vi "Main.vi"() -> ()   [LabVIEW 2015]
uses:
  Typedef/Queue1 Data.ctl
  Typedef/Data.ctl
  <vilib>/vision/Image Controls.llb/IMAQ Image.ctl
  Typedef/Last Mouse Position.ctl
  Typedef/Report Data.ctl
  Typedef/Data2.ctl
  Typedef/State.ctl
  Typedef/Inst. Data.ctl
  Typedef/Inst. Queue.ctl
  <vilib>/Utility/xml.llb/Read From XML File(string).vi
  <vilib>/Utility/xml.llb/Write to XML File(string).vi
  <vilib>/Utility/file.llb/Read From Spreadsheet File (DBL).vi
  Debug 2/Test_ARTS_1.dll
  zauxdll-2014/zauxdll.lvlib
panel:
  out "load?":bool
  out "dist":dbl[](array[numeric])
  in  "SPEED":dbl[][](array[numeric])
  in  "report dist 2":bool
  out "last time":dbl
  out "DYNAMIC 2":T1(array[cluster])
  out "time":dbl[](array[numeric])
  out "autoRs2finish?":bool
  out "autoRSfinish?":bool
  out "autoSliderfinish?":bool
  out "DYNAMIC":T1(array[cluster])
  out "big abgle":string
  out "auto step finish?":bool
  out "y angle array":i32[][](array[numeric])
  out "x angle array":i32[][](array[numeric])
  out "y angle":dbl[](array[numeric])
  out "x angle":dbl[](array[numeric])
  out "Report Data.Degree":dbl[][](array[numeric])
  out "Array":T2(array[cluster])
  out "x^y":dbl
  out "x*y":dbl
  out "Radar Settings":T3={"Car 1"=[], "Times 1"=0, "Car 2"=[], "Times 2"=0, "ORG"={"X"=0.0, "Y"=0.0}, "ORG?"=FALSE, "User1 Velocity"=[], "User2 Velocity"=[], "Lane Distance(X,Y)"={"X"=15.0, "Y"=15.0}, "Lines Para"=[], "Line to Line"=[]}
  in  "Tab Control":T4(tab)
  in  "early time(ms)":dbl
  in  "loop":bool
  in  "Open Button":bool
  in  "Save Button":bool
  in  "clearMSG":bool
  in  "B dist. comp":dbl
  in  "A dist. comp":dbl
  in  "RCS B":dbl
  in  "Path?":bool
  in  "Mode":bool
  in  "dynamic setting":T5
  in  "s/d setting":bool=TRUE
  in  "Rotate":bool
  in  "lock RCS":bool
  out "Path B":u16(slide) scale=0.0..5.0
  in  "TCP?":bool=TRUE
  out "Path A":u16(slide) scale=0.0..5.0
  in  "RUN":bool
  in  "Cluster":cluster{"tester  A":bool, " tester B":bool}={"tester  A"=TRUE, " tester B"=TRUE}
  in  "Clear All":bool
  in  "Velocity":dbl
  in  "User":enum16{"Car A", "Car B"}(ring)
  out "Image":T6(plugin-control)
  in  "Mode":T7(ring)
  in  "Lane Distance(X,Y)":cluster{"X":dbl, "Y":dbl}={"X"=4.0, "Y"=25.0}
  in  "Exit":bool
  in  "RCS A":dbl
  in  "TARGET":enum32{"CarA", "CarB", "Dy path"}(tab)
  out "Target 1":string
  out "Target 2":string
  in  "dy Path":T8(array[cluster])
  in  "set":bool
  in  "AS mode":enum16{"manual", "ratio"}(ring)
  in  "report dist":bool
  out "MSG":string
  in  "AutoExit":bool
  in  "Server":bool
  in  "gap":i32=5
  in  "Path No.":u16(ring) items=["1", "2", "3", "4", "5"]
  in  "Coordinates(X,Y)":cluster{"X":dbl, "Y":dbl}
  in  "Modify (X,Y)":bool
  out "RCS":dbl
  in  "RCSAUTO":bool
  in  "Gain":dbl=3.0
  in  "Range":dbl=3.0
  in  "Dist to RUT":dbl=3.0
  in  "GRX (dB)":dbl=10.0
  in  "GTX (dB)":dbl=10.0
  in  "Load":bool
  out "Output £m File":string
  in  "Path":path
  out "Input RCS File":string
  in  "Boolean":bool
  in  "RCS1":bool
  out "String":string
  out "Inst. Status":bool
  in  "Reset":bool
  in  "Stop":bool
  in  "RF ON/OFF":bool
  in  "T/R Converters":bool
  out "Status?":bool
  in  "Run/Stop":bool
  in  "Custom File":bool
  in  "status":bool
  in  "Trigger":bool
  in  "Dynamic1":T9={"Target 1"={"Boolean"=TRUE, "Start Speed (km/h)"=100.0, "Stop Speed (km/h)"=100.0, "Start Range(m)"=0.0, "Stop Range(m)"=100.0, "Start Gain(dB)"=0.0}, "Target 2"={"Boolean"=FALSE, "Start Speed (km/h)"=0.0, "Stop Speed (km/h)"=0.0, "Start Range(m)"=0.0, "Stop Range(m)"=0.0, "Start Gain(dB)"=0.0}, "Target 3"={"Boolean"=FALSE, "Start Speed (km/h)"=0.0, "Stop Speed (km/h)"=0.0, "Start Range(m)"=0.0, "Stop Range(m)"=0.0, "Start Gain(dB)"=0.0}, "Target 4"={"Boolean"=FALSE, "Start Speed (km/h)"=0.0, "Stop Speed (km/h)"=0.0, "Start Range(m)"=0.0, "Stop Range(m)"=0.0, "Start Gain(dB)"=0.0}}
  in  "Direct program":T10={"Target 1"={"Boolean"=TRUE, "Speed"=100.0, "Range"=50.0, "Gain"=10.0}, "Target 2"={"Boolean"=FALSE, "Speed"=0.0, "Range"=0.0, "Gain"=0.0}, "Target 3"={"Boolean"=FALSE, "Speed"=0.0, "Range"=0.0, "Gain"=0.0}, "Target 4"={"Boolean"=FALSE, "Speed"=0.0, "Range"=0.0, "Gain"=0.0}}
  in  "Mapping":cluster{"4:4":bool, "4:2":bool, "4:1":bool}
  in  "Rx Attenuation (dB)":dbl=3.0
  in  "Distance to RUT":dbl=3.0
  in  "Range Trim (m)":dbl=2.0
  in  "Gain Trim (dB)":dbl=-3.0
  in  "Freq. (GHz)":dbl=76.5
  in  "Inst. Connect":bool
  in  "Inst. Connect IP":string="192.168.0.19"
  in  "GRX (dB)":dbl=10.0
  in  "GTX (dB)":dbl=10.0
  in  "R^4 Comp":bool
  out "generateWF ok?":i32
  out "RCS":dbl=-58.2
  out "RCS def":dbl=-58.2
  in  "wait":u32=1500
  in  "Boolean 2":bool
  in  "RCS2":bool
  out "generateWF ok? 2":i32
  out "String":string
  out "Inst. Status":bool
  in  "Reset":bool
  in  "Stop":bool
  in  "RF ON/OFF":bool
  in  "T/R Converters":bool
  out "Status?":bool
  in  "Run/Stop":bool
  in  "Custom File":bool
  in  "status":bool
  in  "Trigger":bool
  in  "Dynamic2":T9
  in  "Direct program2":T10={"Target 1"={"Boolean"=TRUE, "Speed"=100.0, "Range"=50.0, "Gain"=10.0}, "Target 2"={"Boolean"=FALSE, "Speed"=0.0, "Range"=0.0, "Gain"=0.0}, "Target 3"={"Boolean"=FALSE, "Speed"=0.0, "Range"=0.0, "Gain"=0.0}, "Target 4"={"Boolean"=FALSE, "Speed"=0.0, "Range"=0.0, "Gain"=0.0}}
  in  "Mapping":cluster{"4:4":bool, "4:2":bool, "4:1":bool}
  in  "Rx Attenuation (dB)":dbl=3.0
  in  "Distance to RUT":dbl=3.0
  in  "Range Trim (m)":dbl=2.0
  in  "Gain Trim (dB)":dbl=5.0
  in  "Freq. (GHz)":dbl=76.5
  in  "Inst. Connect":bool
  in  "Inst. Connect IP":string="192.168.0.20"
  in  "GRX (dB)":dbl=10.0
  in  "GTX (dB)":dbl=10.0
  in  "R^4 Comp":bool
  out "RCS 2":dbl=-58.2
  out "RCS def 2":dbl=-58.2
  in  "wait 2":u32=1500
  in  "Y_Vert_Dist(mm)":dbl=24500.0
  in  "X_Vert_Dist(mm)":dbl=24500.0
  in  "Y_MID":dbl=72100.0
  in  "X_MID":dbl=72700.0
  in  "reset ant":bool
  out "Y Position (cm)":dbl(slide)
  out "X Position (cm)":dbl(slide) scale=0.0..150.0
  out "Run Time (sec)":dbl
  in  "Tab Control 2":enum32{"Move"}(tab)
  in  "Move Method":enum16{"Continue", "Inching"}(ring)
  in  "Distance":dbl
  in  "Move Mode":enum16{"Relative", "Absolute"}(ring)
  in  "Direct of movement":enum16{"Forward", "Backward"}(ring)
  in  "Normal Open / Close":enum16{"Open", "Close"}(ring)=enum."Close"
  in  "Move Button":bool
  in  "S ramp":dbl=30.0
  in  "Acceleration":dbl=100000.0
  in  "Initial Speed":dbl=10.0
  in  "Deceleration":dbl=100000.0
  in  "Creep":dbl=30.0
  in  "Stop Button":bool
  in  "Return to Zero Button":bool
  in  "Axis":enum16{"X", "Y", "X+Y"}[](array[ring])=[enum."X"]
  in  "Speed":dbl=10000.0
  in  "Angle":T11(ring)
  in  "Rotate Button":bool
  in  "Return to Origin Button":bool
  in  "Move & Rotate":bool
  in  "Return to Middle Button":bool
  out "Y Axis":T12
  out "X Axis":T12
  out "Connect":bool
  out "APP State":string
  in  "Connect DUT Button":bool
  in  "IP Addr":string="192.168.0.11"
  in  "Cluster 2":cluster{"reset y":bool, "reset x ":bool}
  in  "Save Button 2":bool
  in  "Speed":dbl=1.0 format="%#_13g"
  in  "Initial to Y Step":bool
  in  "Step1":bool
  in  "Step2":bool
  in  "Step3":bool
  in  "Remove Button":bool
  in  "Add Button":bool
  in  "Connect":bool
  in  "angle":T13(ring)
  out "Meter":dbl(knob) scale=-180.0..180.0
  in  "VISA GPIB Resource":refnum<visa-resource-name>="EM-2000"
  out "read buffer":string
  in  "origin":dbl=90.0 format="%#_13g"
  # "dB"
  # "dB"
  # "CarA"
  # "CarB"
  # "RCS Calc"
  # "Dynamic Target"
  # "Setting"
  # "Simulation Setup"
  # "Direct Program"
  # "Dynamic Target"
  # "Setting"
  # "Simulation Setup"
  # "Direct Program"
  # "Move"
  # "Rotate"
  # "Return to Zero"
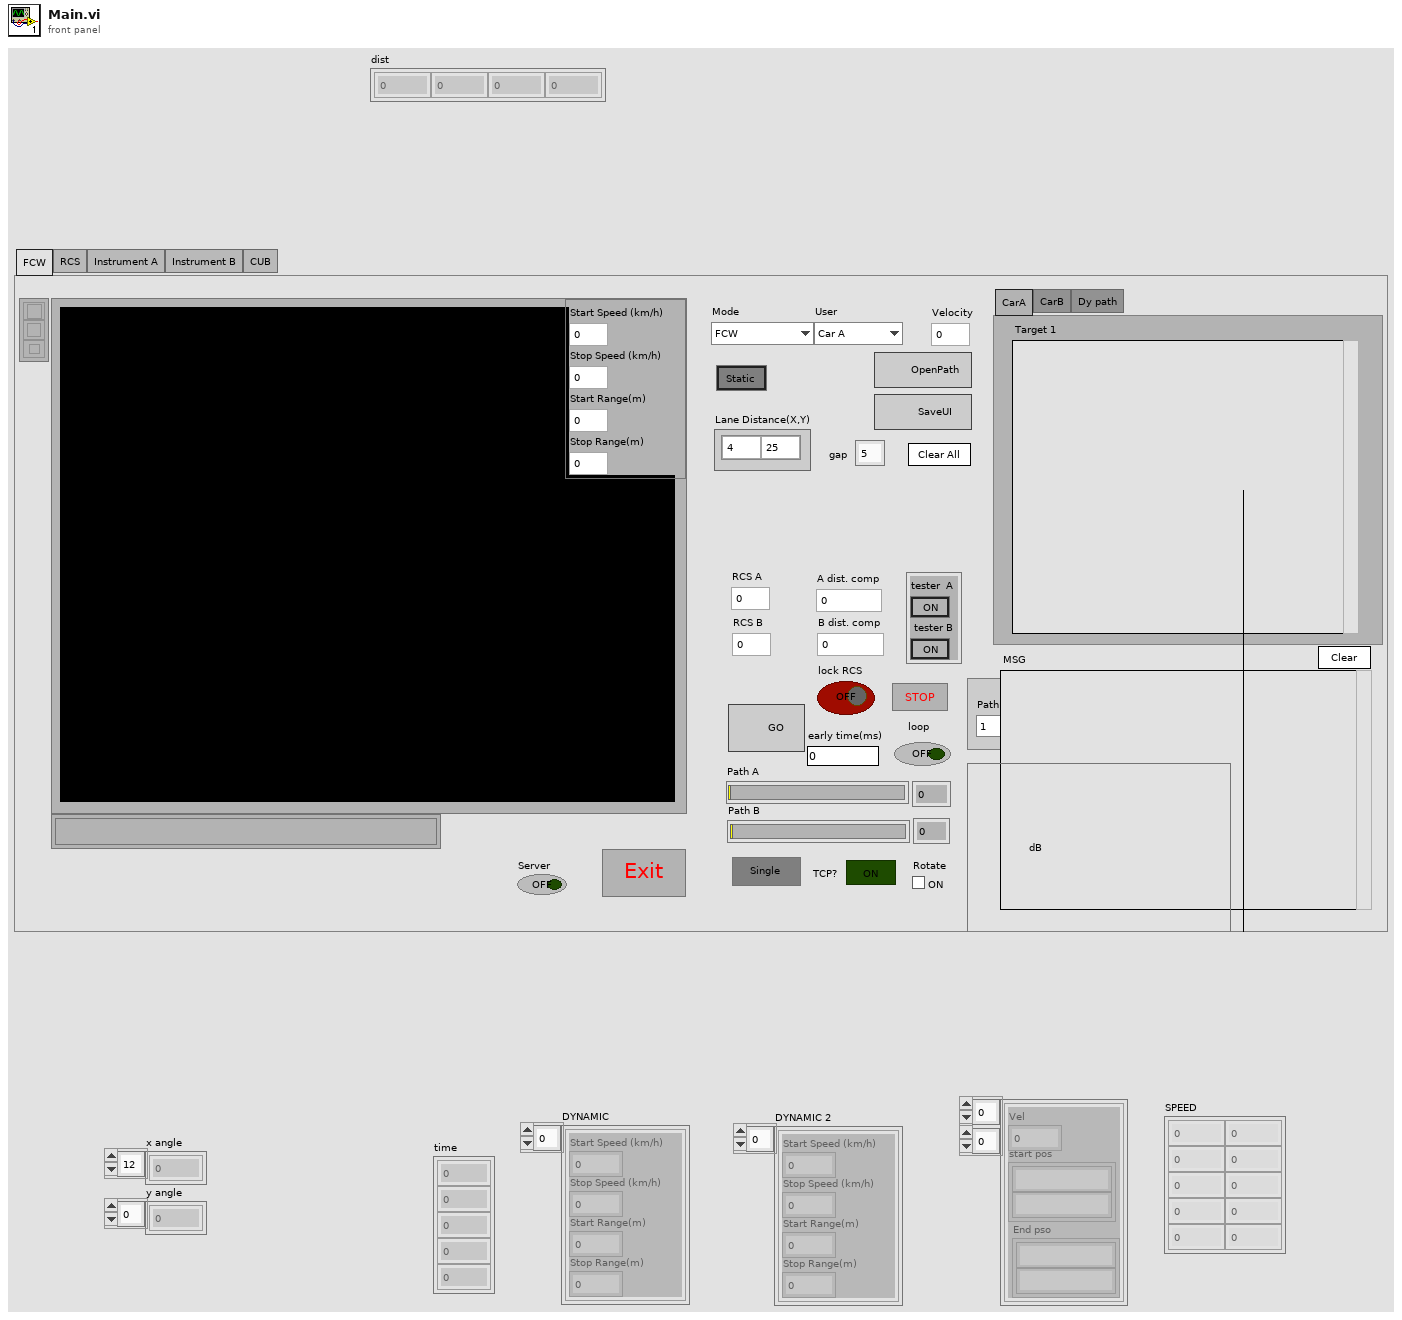
[diagram p1: front panel]
types:
  T1 = cluster{"Start Speed (km/h)":dbl, "Stop Speed (km/h) ":dbl, "Start Range(m)":dbl, "Stop Range(m)":dbl}[]
  T2 = cluster{"Vel":dbl, "start pos":cluster{string, string}, "End pso":cluster{string, string}}[][]
  T3 = cluster{"Car 1":cluster{"X":dbl, "Y":dbl}[], "Times 1":i32, "Car 2":cluster{"X":dbl, "Y":dbl}[], "Times 2":i32, "ORG":cluster{"X":dbl, "Y":dbl}, "ORG?":bool, "User1 Velocity":dbl[], "User2 Velocity":dbl[], "Lane Distance(X,Y)":cluster{"X":dbl, "Y":dbl}, "Lines Para":dbl[][], "Line to Line":dbl[]}
  T4 = enum32{"FCW", "RCS", "Instrument A", "Instrument B", "CUB", "GPIB"}
  T5 = cluster{"Start Speed (km/h)":dbl, "Stop Speed (km/h) ":dbl, "Start Range(m)":dbl, "Stop Range(m)":dbl}
  T6 = typedef "IMAQ Image.ctl" = refnum<image>
  T7 = enum16{"FCW", "BSD(Right)", "BSD(Left)", "RCTA(Right)", "RCTA(Left)", "DOW(Right)", "DOW(Left)"}
  T8 = cluster{"end":dbl, "start":dbl, "Axis Speed":dbl, "movement":dbl}[][]
  T9 = cluster{"Target 1":cluster{"Boolean":bool, "Start Speed (km/h)":dbl, "Stop Speed (km/h)":dbl, "Start Range(m)":dbl, "Stop Range(m)":dbl, "Start Gain(dB)":dbl}, "Target 2":cluster{"Boolean":bool, "Start Speed (km/h)":dbl, "Stop Speed (km/h)":dbl, "Start Range(m)":dbl, "Stop Range(m)":dbl, "Start Gain(dB)":dbl}, "Target 3":cluster{"Boolean":bool, "Start Speed (km/h)":dbl, "Stop Speed (km/h)":dbl, "Start Range(m)":dbl, "Stop Range(m)":dbl, "Start Gain(dB)":dbl}, "Target 4":cluster{"Boolean":bool, "Start Speed (km/h)":dbl, "Stop Speed (km/h)":dbl, "Start Range(m)":dbl, "Stop Range(m)":dbl, "Start Gain(dB)":dbl}}
  T10 = cluster{"Target 1":cluster{"Boolean":bool, "Speed":dbl, "Range":dbl, "Gain":dbl}, "Target 2":cluster{"Boolean":bool, "Speed":dbl, "Range":dbl, "Gain":dbl}, "Target 3":cluster{"Boolean":bool, "Speed":dbl, "Range":dbl, "Gain":dbl}, "Target 4":cluster{"Boolean":bool, "Speed":dbl, "Range":dbl, "Gain":dbl}}
  T11 = enum32{"0", "1", "10", "30", "34", "60", "90", "180", "-1", "-10"}
  T12 = cluster{"Operating State":string, "Current Position":dbl, "Current Speed":dbl, "Axis State":i32, "Angle":dbl}
  T13 = enum16{"0", "1", "5", "10", "30", "60", "90", "180"}
  T14 = cluster{"Global Rectangle":i32[], "Contours":cluster{"Contour Type":u32, "ROI Type":u32, "Points":i32[]}[]}
  T15 = typedef "Inst. Data.ctl" = cluster{"£m Data":dbl[][], "Inst. Status":bool, "GTX (dB)":dbl, "GRX (dB)":dbl, "Freq. (GHz)":dbl, "Gain Trim (dB)":dbl, "Range Trim (m)":dbl, "Distance to RUT":dbl, "Rx Attenuation (dB)":dbl, "Mapping":cluster{"4:4":bool, "4:2":bool, "4:1":bool}, "Direct program":cluster{"Target 1":cluster{"Boolean":bool, "Speed":dbl, "Range":dbl, "Gain":dbl}, "Target 2":cluster{"Boolean":bool, "Speed":dbl, "Range":dbl, "Gain":dbl}, "Target 3":cluster{"Boolean":bool, "Speed":dbl, "Range":dbl, "Gain":dbl}, "Target 4":cluster{"Boolean":bool, "Speed":dbl, "Range":dbl, "Gain":dbl}}, "Dynamic":cluster{"Target 1":cluster{"Boolean":bool, "Start Speed (km/h)":dbl, "Stop Speed (km/h)":dbl, "Start Range(m)":dbl, "Stop Range(m)":dbl, "Start Gain(dB)":dbl}, "Target 2":cluster{"Boolean":bool, "Start Speed (km/h)":dbl, "Stop Speed (km/h)":dbl, "Start Range(m)":dbl, "Stop Range(m)":dbl, "Start Gain(dB)":dbl}, "Target 3":cluster{"Boolean":bool, "Start Speed (km/h)":dbl, "Stop Speed (km/h)":dbl, "Start Range(m)":dbl, "Stop Range(m)":dbl, "Start Gain(dB)":dbl}, "Target 4":cluster{"Boolean":bool, "Start Speed (km/h)":dbl, "Stop Speed (km/h)":dbl, "Start Range(m)":dbl, "Stop Range(m)":dbl, "Start Gain(dB)":dbl}}, "String":string, "auto test":bool}
  T16 = enum16{"INIT", "READ", "WRITE", "Query", "CLOSE"}
  T17 = typedef "State.ctl" = enum16{"Idle", "Initial", "Update", "get angle", "Axis", "Connect", "Creep", "Speed", "Distance", "Move Method", "Move Mode", "Direct of Movement", "Initail Speed", "Sramp", "Normal Open", "Acceleration", "Deceleration", "Angle", "Move&Rotate", "Rotate", "Rotate_2", "Return to Origin", "Move", "Inching", "Return to Zero", "Return to Middle", "Go to Step1", "Go to Step2", "Go to Step3", "Initial to Y Step", "Select Speed", "auto mode", "Stop", "reset xy", "reset ant", "set speed", "Exit"}
  T18 = typedef "Queue1 Data.ctl" = cluster{"State":enum16{"Idle", "Initial", "Update", "User", "Mode", "Lane Distance", "ORG", "Lines Para", "Velocity", "Coordinate", "Path No.", "Modify", "Load", "Loadpath", "Clear All", "Overlay_Circle Para", "Overlay", "Report Dist", "Report", "RCS Report", "dynamic", "save", "dypath", "Exit"}, "variant":variant}
  T19 = typedef "Inst. Queue.ctl" = cluster{enum16{"auto mode", "Idle", "Inst. Connect", "£m Data", "Inst. Update", "Freq. (GHz)", "rx att", "GTX (dB)", "GRX (dB)", "Range Trim(m)", "Gain Trim (dB)", "Distance to RUT", "Mapping", "Convert", "RF ON/OFF", "Run", "Direct Program", "Stop", "Dynamic", "dyset", "Exit"}, "variant":variant}
  T20 = enum16{"0", "1", "10", "30", "34", "60", "90", "180"}
  T21 = cluster{"Enum":enum16{"INIT", "READ", "DEC", "ADD", "WRITE", "CLOSE", "IDLE"}, "Variable":variant}
  T22 = cluster{dbl, cluster{string, string}, cluster{string, string}}[]
  T23 = cluster{dbl, cluster{string, string}, cluster{string, string}}
  T24 = typedef "Data2.ctl" = cluster{"App State":string, "Connect ":bool, "phandle out":u32, "Axis":enum16{"X", "Y", "X+Y"}[], "S ramp":dbl, "Acceleration":dbl, "Initial Speed":dbl, "Normal Open / Close":enum16{"Open", "Close"}, "Deceleration":dbl, "Creep":dbl, "Speed":dbl, "X Axis":cluster{"Operating State":string, "Current Position":dbl, "Current Speed":dbl, "Axis State":i32, "Angle":dbl}, "Y Axis":cluster{"Operating State":string, "Current Position":dbl, "Current Speed":dbl, "Axis State":i32, "Angle":dbl}, "Distance":dbl, "Direct of movement":enum16{"Forward", "Backward"}, "Move Method":enum16{"Continue", "Inching"}, "Move Mode":enum16{"Relative", "Absolute"}, "Angle":enum32{"0", "1", "10", "30", "34", "60", "90", "180", "-1", "-10"}, "Times":i32, "Start Time":dbl, "Step Flag":bool, "x  dist":dbl[], "y dist":dbl[], "x angle array":i32[][], "y angle array":i32[][], "index":dbl, "big motion angle":dbl, "big angle":dbl[], "xy dy speed table":dbl[][], "x dy speed table":dbl[], "y dy speed table":dbl[], "x dy time":dbl[], "y dy time":dbl[], "xy dy time":dbl[][], "dy Path  ":cluster{"end":dbl, "start":dbl, "Axis Speed":dbl, "movement":dbl}[][]}
  T25 = typedef "Data.ctl" = cluster{"Image":T6, "User":enum16{"Car 1", "Car 2"}, "Last Mouse Position":T26, "Mode":enum16{"FCW", "BSD(Right)", "BSD(Left)", "RCTA(Right)", "RCTA(Left)", "DOW(Right)", "DOW(Left)"}, "Report Data":T27, "Target 1":string, "Target 2":string, "Velocity":dbl, "Coordinates(X,Y)":cluster{"X":dbl, "Y":dbl}, "Path No.":u16, "Input RCS File":string, "Input RCS Data":dbl[][], "Output £m File":string, "DYNAMIC":cluster{"Start Speed (km/h)":dbl, "Stop Speed (km/h) ":dbl, "Start Range(m)":dbl, "Stop Range(m)":dbl}[], "DYNAMIC 2":cluster{"Start Speed (km/h)":dbl, "Stop Speed (km/h) ":dbl, "Start Range(m)":dbl, "Stop Range(m)":dbl}[], "dy Path  ":cluster{"end":dbl, "start":dbl, "Axis Speed":dbl, "movement":dbl}[][]}
  T26 = typedef "Last Mouse Position.ctl" = cluster{"User1":cluster{"X":dbl, "Y":dbl}[], "Times 1":i32, "User2":cluster{"X":dbl, "Y":dbl}[], "Times 2":i32, "ORG":cluster{"X":dbl, "Y":dbl}, "ORG?":bool, "User1 Velocity":dbl[], "User2 Velocity":dbl[], "Lane Distance(X,Y)":cluster{"X":dbl, "Y":dbl}, "Lines Para":dbl[][], "Line to Line":dbl[]}[]
  T27 = typedef "Report Data.ctl" = cluster{"Coordinate":cluster{string, string}[][], "Distance":dbl[][], "Degree":dbl[][], "Velocity":dbl[][], "Times":i32[]}
  T28 = cluster{"Operating State":string, "Current Position":dbl, "Current Speed":dbl, "Axis State":i32, "Angle":i32}
  T29 = cluster{"end":dbl, "start":dbl, "Axis Speed":dbl, "movement":dbl}[]
  T30 = enum16{"auto mode", "Idle", "Inst. Connect", "£m Data", "Inst. Update", "Freq. (GHz)", "rx att", "GTX (dB)", "GRX (dB)", "Range Trim(m)", "Gain Trim (dB)", "Distance to RUT", "Mapping", "Convert", "RF ON/OFF", "Run", "Direct Program", "Stop", "Dynamic", "dyset", "Exit"}
  T31 = cluster{"Boolean":bool, "Speed":dbl, "Range":dbl, "Gain":dbl}
  T32 = enum16{"INIT", "READ", "DEC", "ADD", "WRITE", "CLOSE", "IDLE"}
  T33 = cluster{"Value":cluster{"Target 1":cluster{"Boolean":bool, "Start Speed (km/h)":dbl, "Stop Speed (km/h)":dbl, "Start Range(m)":dbl, "Stop Range(m)":dbl, "Start Gain(dB)":dbl}, "Target 2":cluster{"Boolean":bool, "Start Speed (km/h)":dbl, "Stop Speed (km/h)":dbl, "Start Range(m)":dbl, "Stop Range(m)":dbl, "Start Gain(dB)":dbl}, "Target 3":cluster{"Boolean":bool, "Start Speed (km/h)":dbl, "Stop Speed (km/h)":dbl, "Start Range(m)":dbl, "Stop Range(m)":dbl, "Start Gain(dB)":dbl}, "Target 4":cluster{"Boolean":bool, "Start Speed (km/h)":dbl, "Stop Speed (km/h)":dbl, "Start Range(m)":dbl, "Stop Range(m)":dbl, "Start Gain(dB)":dbl}}, "Value":cluster{"Target 1":cluster{"Boolean":bool, "Start Speed (km/h)":dbl, "Stop Speed (km/h)":dbl, "Start Range(m)":dbl, "Stop Range(m)":dbl, "Start Gain(dB)":dbl}, "Target 2":cluster{"Boolean":bool, "Start Speed (km/h)":dbl, "Stop Speed (km/h)":dbl, "Start Range(m)":dbl, "Stop Range(m)":dbl, "Start Gain(dB)":dbl}, "Target 3":cluster{"Boolean":bool, "Start Speed (km/h)":dbl, "Stop Speed (km/h)":dbl, "Start Range(m)":dbl, "Stop Range(m)":dbl, "Start Gain(dB)":dbl}, "Target 4":cluster{"Boolean":bool, "Start Speed (km/h)":dbl, "Stop Speed (km/h)":dbl, "Start Range(m)":dbl, "Stop Range(m)":dbl, "Start Gain(dB)":dbl}}}
  T34 = cluster{"Value":cluster{"Target 1":cluster{"Boolean":bool, "Speed":dbl, "Range":dbl, "Gain":dbl}, "Target 2":cluster{"Boolean":bool, "Speed":dbl, "Range":dbl, "Gain":dbl}, "Target 3":cluster{"Boolean":bool, "Speed":dbl, "Range":dbl, "Gain":dbl}, "Target 4":cluster{"Boolean":bool, "Speed":dbl, "Range":dbl, "Gain":dbl}}, "Value":cluster{"Target 1":cluster{"Boolean":bool, "Speed":dbl, "Range":dbl, "Gain":dbl}, "Target 2":cluster{"Boolean":bool, "Speed":dbl, "Range":dbl, "Gain":dbl}, "Target 3":cluster{"Boolean":bool, "Speed":dbl, "Range":dbl, "Gain":dbl}, "Target 4":cluster{"Boolean":bool, "Speed":dbl, "Range":dbl, "Gain":dbl}}}
  T35 = cluster{"Target 1":cluster{"Boolean":bool, "Start Speed (km/h)":dbl, "Stop Speed (km/h)":dbl, "Start Range(m)":dbl, "Stop Range(m)":dbl, "Start Gain(dB)":dbl}, "Target 2":cluster{"Boolean":bool, "Start Speed (km/h)":dbl, "Stop Speed (km/h)":dbl, "Start Range(m)":dbl, "Stop Range(m)":dbl, "Start Gain(dB)":dbl}, "Target 3":cluster{"Boolean":bool, "Start Speed (km/h)":dbl, "Stop Speed (km/h)":dbl, "Start Range(m)":dbl, "Stop Range(m)":dbl, "Start Gain(dB)":dbl}, "Target 4":cluster{"Boolean":bool, "Start Speed (km/h)":dbl, "Stop Speed (km/h)":dbl, "Start Range(m)":dbl, "Stop Range(m)":dbl, "Start Gain(dB)":dbl}}[][]
  T36 = cluster{cluster{"Target 1":cluster{"Boolean":bool, "Speed":dbl, "Range":dbl, "Gain":dbl}, "Target 2":cluster{"Boolean":bool, "Speed":dbl, "Range":dbl, "Gain":dbl}, "Target 3":cluster{"Boolean":bool, "Speed":dbl, "Range":dbl, "Gain":dbl}, "Target 4":cluster{"Boolean":bool, "Speed":dbl, "Range":dbl, "Gain":dbl}}[], cluster{"Target 1":cluster{"Boolean":bool, "Speed":dbl, "Range":dbl, "Gain":dbl}, "Target 2":cluster{"Boolean":bool, "Speed":dbl, "Range":dbl, "Gain":dbl}, "Target 3":cluster{"Boolean":bool, "Speed":dbl, "Range":dbl, "Gain":dbl}, "Target 4":cluster{"Boolean":bool, "Speed":dbl, "Range":dbl, "Gain":dbl}}[]}
  T37 = cluster{"Target 1":cluster{"Boolean":bool, "Start Speed (km/h)":dbl, "Stop Speed (km/h)":dbl, "Start Range(m)":dbl, "Stop Range(m)":dbl, "Start Gain(dB)":dbl}, "Target 2":cluster{"Boolean":bool, "Start Speed (km/h)":dbl, "Stop Speed (km/h)":dbl, "Start Range(m)":dbl, "Stop Range(m)":dbl, "Start Gain(dB)":dbl}, "Target 3":cluster{"Boolean":bool, "Start Speed (km/h)":dbl, "Stop Speed (km/h)":dbl, "Start Range(m)":dbl, "Stop Range(m)":dbl, "Start Gain(dB)":dbl}, "Target 4":cluster{"Boolean":bool, "Start Speed (km/h)":dbl, "Stop Speed (km/h)":dbl, "Start Range(m)":dbl, "Stop Range(m)":dbl, "Start Gain(dB)":dbl}}[]
  T38 = cluster{"queue out":refnum<queue>, "queue out":refnum<queue>, "queue out":refnum<queue>}
  T39 = cluster{"auto step finish?":refnum<vi>, "Run/Stop":refnum<vi>, "Run/Stop":refnum<vi>, "AutoExit":refnum<vi>, "RUN":refnum<vi>}
  T40 = enum16{"Idle", "Initial", "Update", "User", "Mode", "Lane Distance", "ORG", "Lines Para", "Velocity", "Coordinate", "Path No.", "Modify", "Load", "Loadpath", "Clear All", "Overlay_Circle Para", "Overlay", "Report Dist", "Report", "RCS Report", "dynamic", "save", "dypath", "Exit"}
  T41 = cluster{cluster{"X":dbl, "Y":dbl}[], i32, cluster{"X":dbl, "Y":dbl}[], i32, cluster{"X":dbl, "Y":dbl}, bool, dbl[], dbl[], "Value":cluster{"X":dbl, "Y":dbl}, "Lines Para":dbl[][], "Line to Line":dbl[]}
  T42 = cluster{cluster{"X":dbl, "Y":dbl}[], i32, cluster{"X":dbl, "Y":dbl}[], i32, cluster{"X":dbl, "Y":dbl}, bool, dbl[], dbl[], "Value":cluster{"X":dbl, "Y":dbl}, "Lines Para":dbl[][], "Line to Line":dbl[]}[]
  T43 = cluster{"Start Speed (km/h)":dbl, "Stop Speed (km/h) ":dbl, "Start Range(m)":dbl, "Stop Range(m)":dbl}[][]
  T44 = cluster{"User1":cluster{"X":dbl, "Y":dbl}[], "Times 1":i32, "User2":cluster{"X":dbl, "Y":dbl}[], "Times 2":i32, "ORG":cluster{"X":dbl, "Y":dbl}, "ORG?":bool, "User1 Velocity":dbl[], "User2 Velocity":dbl[], "Lane Distance(X,Y)":cluster{"X":dbl, "Y":dbl}, "Lines Para":dbl[][], "Line to Line":dbl[]}
  T45 = cluster{"Start Speed (km/h)":dbl, "Stop Speed (km/h) ":dbl, "Stop Range(m)":dbl, "Start Range(m)":dbl}[]
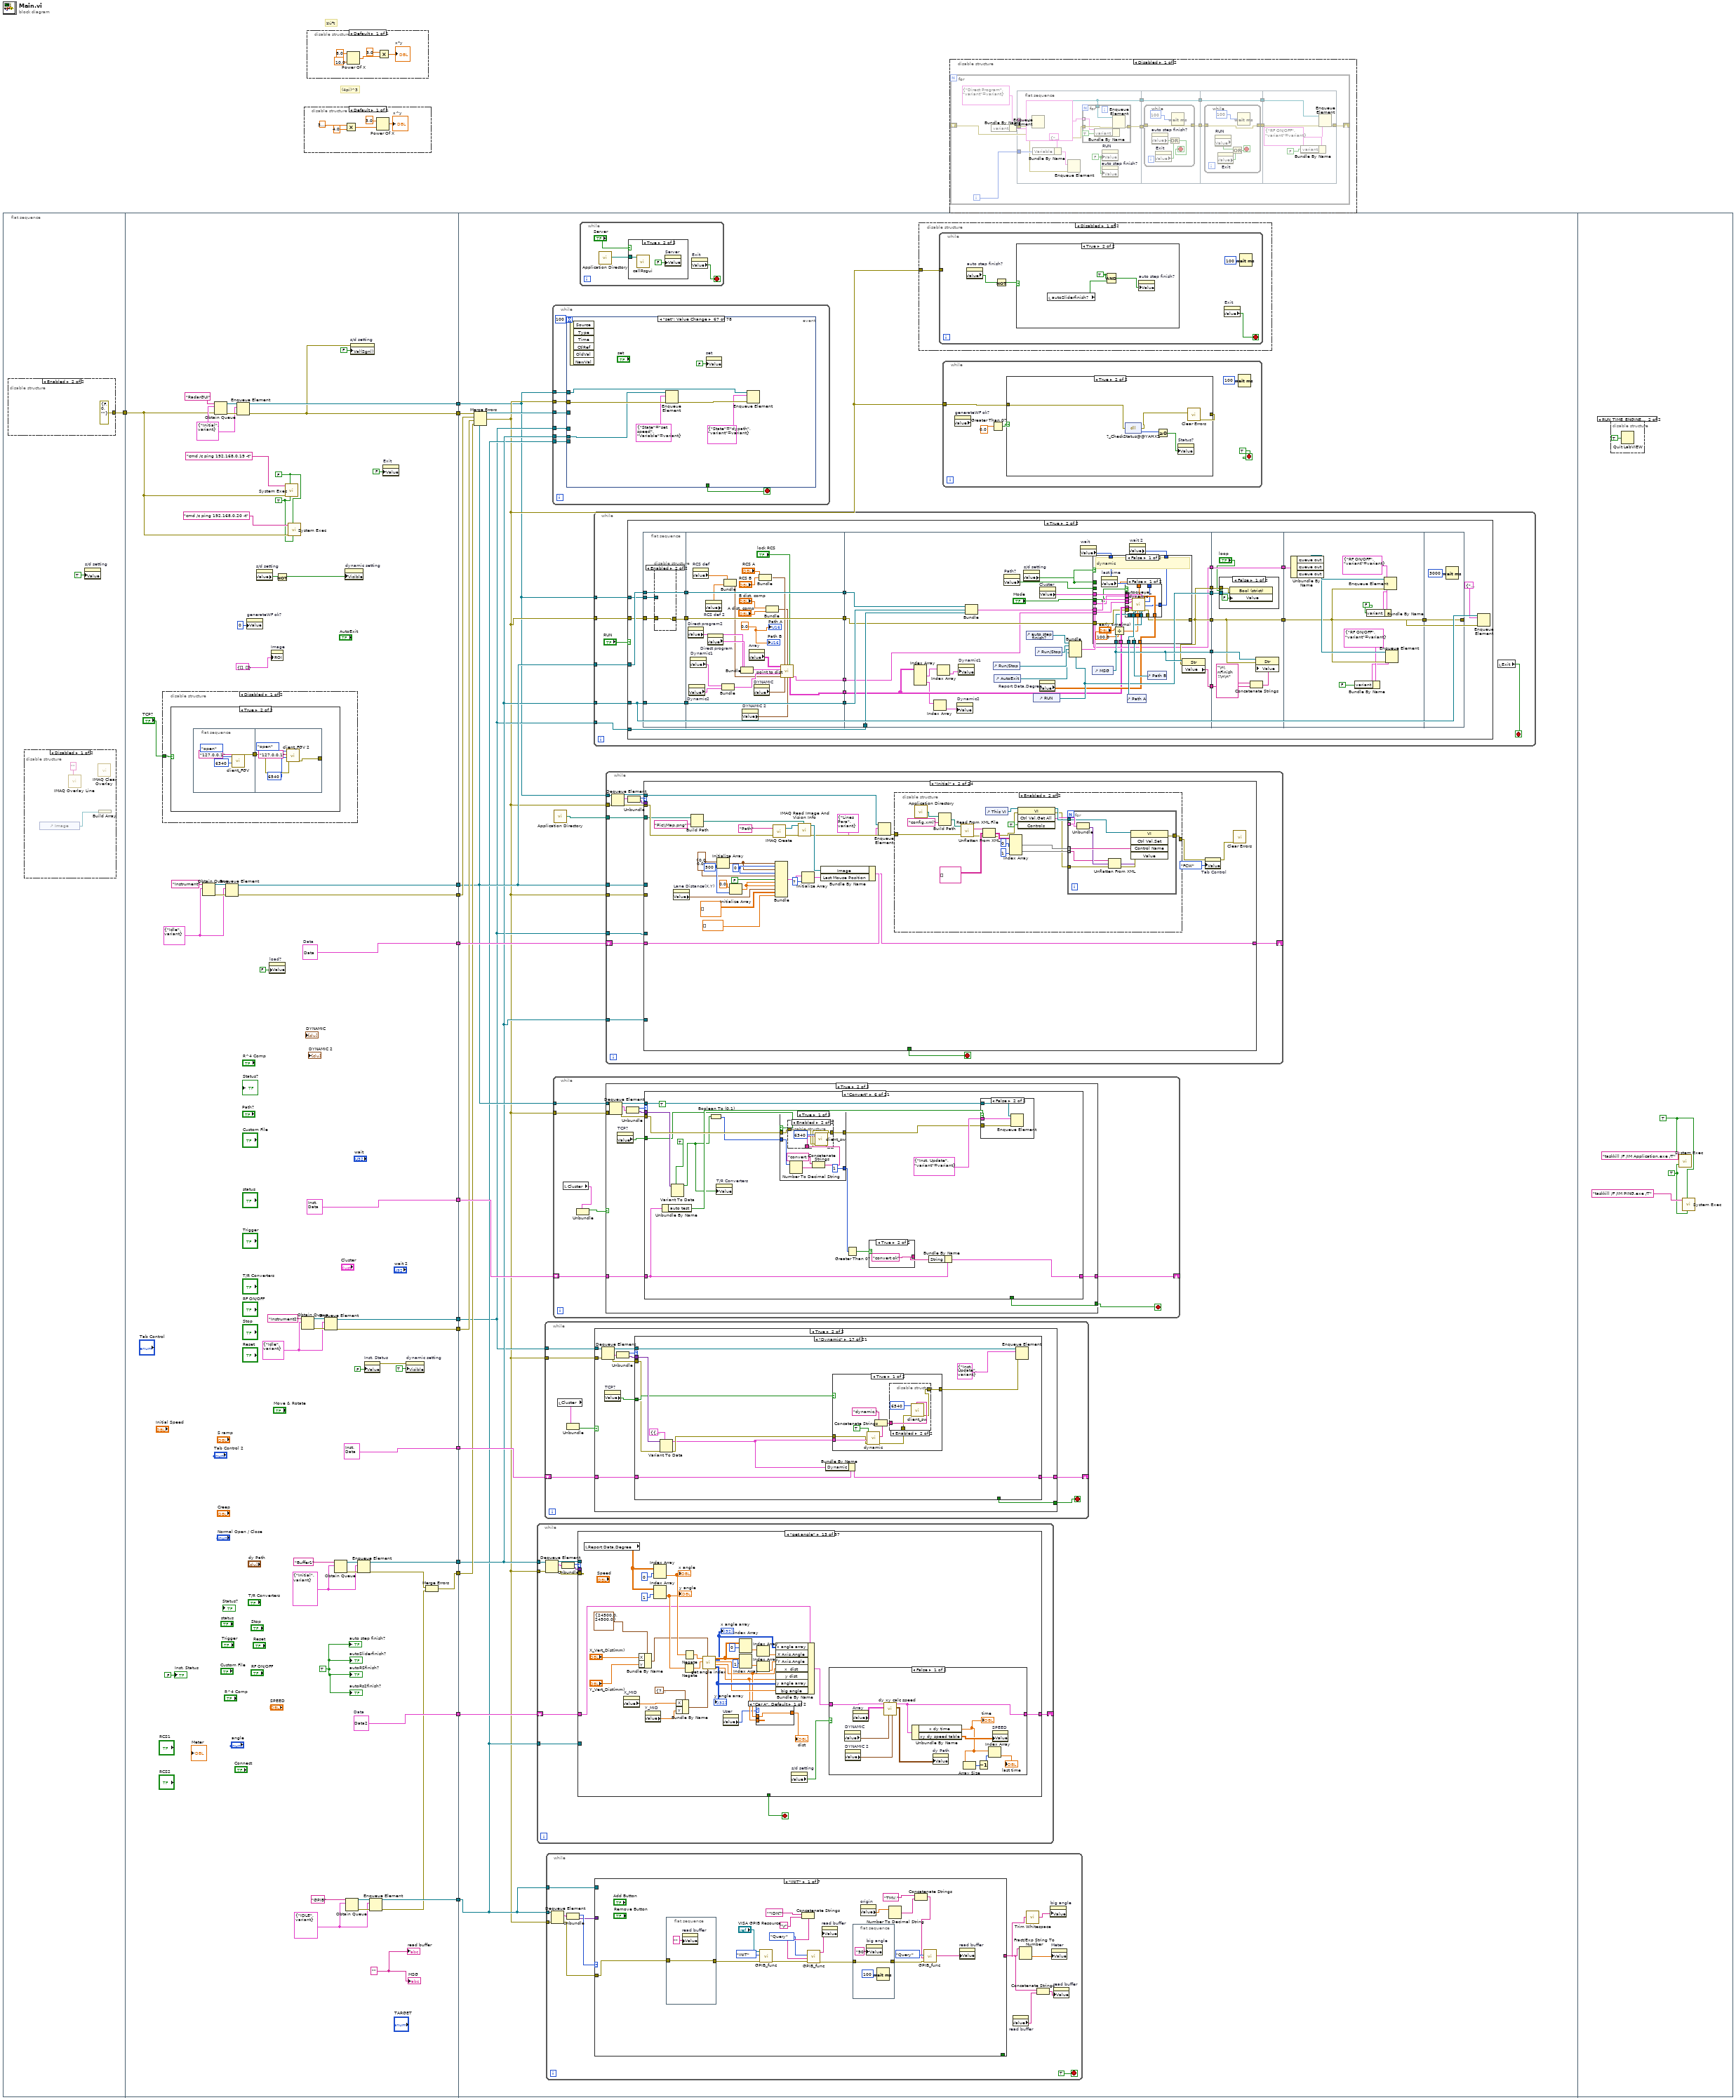
[diagram p0: block diagram]
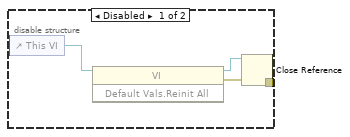
[diagram p3: hidden frame]
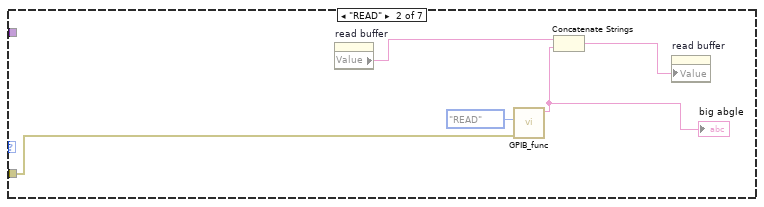
[diagram p11: hidden frame]
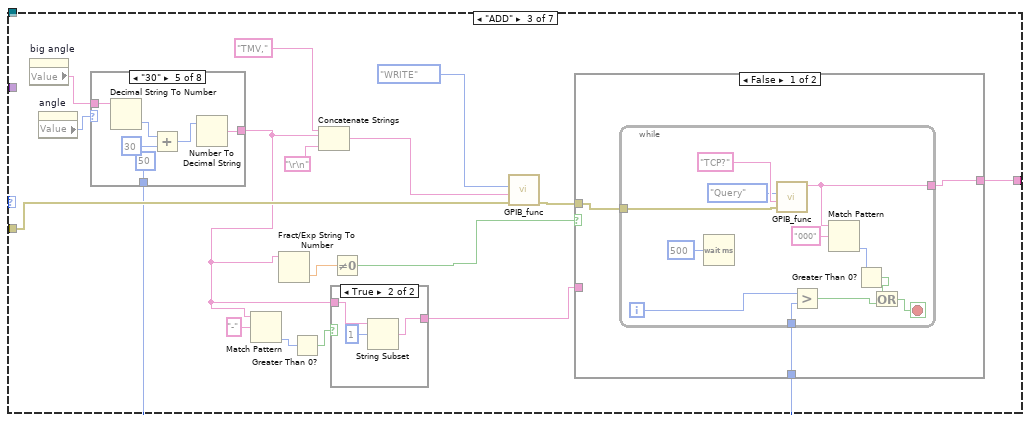
[diagram p12: hidden frame]
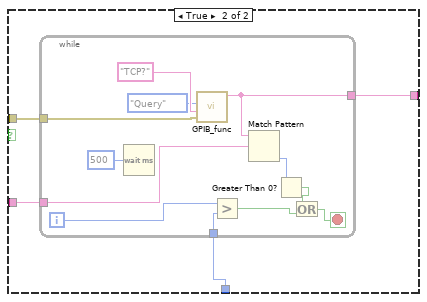
[diagram p13: hidden frame]
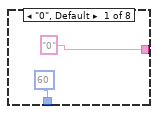
[diagram p15: hidden frame]
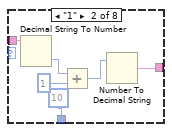
[diagram p16: hidden frame]
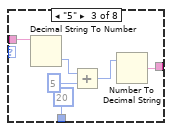
[diagram p17: hidden frame]
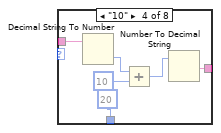
[diagram p18: hidden frame]
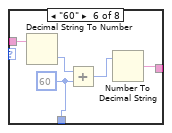
[diagram p19: hidden frame]
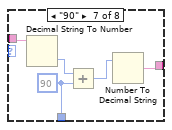
[diagram p20: hidden frame]
diagram:
  # "(4pi)^3"
  # "¥ú³t"
  n1 = flat-sequence {
    tunnel: [w16] -> w12
    tunnel: [w28] -> w14
    tunnel: [w73] -> w13
    tunnel: w12 -> [w36]
    tunnel: [w72] -> w11
    tunnel: [w68] -> w10
    tunnel: [w67] -> w9
    tunnel: [T15 {"£m Data"=[], "Inst. Status"=FALSE, "GTX (dB)"=0.0, "GRX (dB)"=0.0, "Freq. (GHz)"=76.5, "Gain Trim (dB)"=5.0, "Range Trim (m)"=2.5, "Distance to RUT"=3.0, "Rx Attenuation (dB)"=10.0, "Mapping"={"4:4"=FALSE, "4:2"=FALSE, "4:1"=FALSE}, "Direct program"={"Target 1"={"Boolean"=FALSE, "Speed"=0.0, "Range"=0.0, "Gain"=0.0}, "Target 2"={"Boolean"=FALSE, "Speed"=0.0, "Range"=0.0, "Gain"=0.0}, "Target 3"={"Boolean"=FALSE, "Speed"=0.0, "Range"=0.0, "Gain"=0.0}, "Target 4"={"Boolean"=FALSE, "Speed"=0.0, "Range"=0.0, "Gain"=0.0}}, "Dynamic"={"Target 1"={"Boolean"=FALSE, "Start Speed (km/h)"=0.0, "Stop Speed (km/h)"=0.0, "Start Range(m)"=0.0, "Stop Range(m)"=0.0, "Start Gain(dB)"=0.0}, "Target 2"={"Boolean"=FALSE, "Start Speed (km/h)"=0.0, "Stop Speed (km/h)"=0.0, "Start Range(m)"=0.0, "Stop Range(m)"=0.0, "Start Gain(dB)"=0.0}, "Target 3"={"Boolean"=FALSE, "Start Speed (km/h)"=0.0, "Stop Speed (km/h)"=0.0, "Start Range(m)"=0.0, "Stop Range(m)"=0.0, "Start Gain(dB)"=0.0}, "Target 4"={"Boolean"=FALSE, "Start Speed (km/h)"=0.0, "Stop Speed (km/h)"=0.0, "Start Range(m)"=0.0, "Stop Range(m)"=0.0, "Start Gain(dB)"=0.0}}, "String"="", "auto test"=FALSE}] -> w8
    tunnel: [w64] -> w7
    tunnel: [w46] -> w6
    tunnel: [w59] -> w5
    tunnel: [T15 {"£m Data"=[], "Inst. Status"=FALSE, "GTX (dB)"=0.0, "GRX (dB)"=0.0, "Freq. (GHz)"=76.5, "Gain Trim (dB)"=5.0, "Range Trim (m)"=2.5, "Distance to RUT"=3.0, "Rx Attenuation (dB)"=10.0, "Mapping"={"4:4"=FALSE, "4:2"=FALSE, "4:1"=FALSE}, "Direct program"={"Target 1"={"Boolean"=FALSE, "Speed"=0.0, "Range"=0.0, "Gain"=0.0}, "Target 2"={"Boolean"=FALSE, "Speed"=0.0, "Range"=0.0, "Gain"=0.0}, "Target 3"={"Boolean"=FALSE, "Speed"=0.0, "Range"=0.0, "Gain"=0.0}, "Target 4"={"Boolean"=FALSE, "Speed"=0.0, "Range"=0.0, "Gain"=0.0}}, "Dynamic"={"Target 1"={"Boolean"=FALSE, "Start Speed (km/h)"=0.0, "Stop Speed (km/h)"=0.0, "Start Range(m)"=0.0, "Stop Range(m)"=0.0, "Start Gain(dB)"=0.0}, "Target 2"={"Boolean"=FALSE, "Start Speed (km/h)"=0.0, "Stop Speed (km/h)"=0.0, "Start Range(m)"=0.0, "Stop Range(m)"=0.0, "Start Gain(dB)"=0.0}, "Target 3"={"Boolean"=FALSE, "Start Speed (km/h)"=0.0, "Stop Speed (km/h)"=0.0, "Start Range(m)"=0.0, "Stop Range(m)"=0.0, "Start Gain(dB)"=0.0}, "Target 4"={"Boolean"=FALSE, "Start Speed (km/h)"=0.0, "Stop Speed (km/h)"=0.0, "Start Range(m)"=0.0, "Stop Range(m)"=0.0, "Start Gain(dB)"=0.0}}, "String"="", "auto test"=FALSE}] -> w4
    tunnel: [w53] -> w3
    tunnel: [w52] -> w2
    tunnel: [w47] -> w1
    tunnel: w14 -> [w98]
    tunnel: w13 -> [w89]
    tunnel: w11 -> [w103]
    tunnel: w10 -> [w94]
    tunnel: w9 -> [w97]
    tunnel: w8 -> [w101]
    tunnel: w7 -> [w100]
    tunnel: w6 -> [w95]
    tunnel: w5 -> [w93]
    tunnel: w4 -> [w99]
    tunnel: w3 -> [w91]
    tunnel: w2 -> [w96]
    tunnel: w1 -> [w92]
    frame #0 {
      n2 = disable-structure shown="Enabled" {
        disable-tunnel: [w17 errorcluster {"status"=FALSE, "code"=0, "source"=""} ("error out")] -> w16
        frame Disabled {
          n3 = control-ref of="This VI"() -> (w20:refnum<vi>)
          n4 = invoke class="VI" method="Default Vals.Reinit All"(reference=w20) -> (reference out=w18:refnum<vi>, error out=w19:errorcluster)  [unwired: 2 in, 1 out]
          n5 = Close Reference(reference=w18, error in (no error)=w19) -> (error out=w17:errorcluster)
        }
        frame Enabled {
        }
      }
      n6 = disable-structure shown="Disabled" {
        frame Disabled {
          n7 = control-ref of="Image"() -> (w22:refnum<vi>)
          n8 = call "IMAQ Overlay Line"("Group"="") -> ()  [unwired: 9 in, 2 out]
          n9 = call "IMAQ Clear Overlay"() -> ()  [unwired: 10 in, 2 out]
          n10 = Build Array(w22) -> ()  [unwired: 1 out]
        }
        frame Enabled {
        }
      }
      n11 = property on="s/d setting" class="Bool (strict)"("Value"=TRUE ("s/d setting")) -> ()  [unwired: 2 in, 2 out]
    }
    frame #1 {
      w31 = TRUE ("run minimized? (F)")
      w33 = FALSE ("wait until completion? (T)")
      w37 = TRUE
      w41 = ""
      w48 = T21 {"Enum"=enum."IDLE", "Variable"=variant}
      w54 = T19 {enum."Idle", "variant"=variant}
      w60 = cluster{"State":T17, "Variable":variant} {"State"=enum."Initial", "Variable"=variant}
      w64 = T24 {"App State"="", "Connect "=FALSE, "phandle out"=0, "Axis"=[], "S ramp"=30.0, "Acceleration"=100000.0, "Initial Speed"=10.0, "Normal Open / Close"=enum."Close", "Deceleration"=100000.0, "Creep"=30.0, "Speed"=1000.0, "X Axis"={"Operating State"="", "Current Position"=0.0, "Current Speed"=0.0, "Axis State"=0, "Angle"=0.0}, "Y Axis"={"Operating State"="", "Current Position"=0.0, "Current Speed"=0.0, "Axis State"=0, "Angle"=0.0}, "Distance"=0.0, "Direct of movement"=enum."Forward", "Move Method"=enum."Continue", "Move Mode"=enum."Relative", "Angle"=enum."0", "Times"=0, "Start Time"=0.0, "Step Flag"=FALSE, "x  dist"=[], "y dist"=[], "x angle array"=[], "y angle array"=[], "index"=0.0, "big motion angle"=0.0, "big angle"=[], "xy dy speed table"=[], "x dy speed table"=[], "y dy speed table"=[], "x dy time"=[], "y dy time"=[], "xy dy time"=[], "dy Path  "=[]}  # Data
      w66 = T19 {enum."Idle", "variant"=variant}
      w72 = T25 {"Image"=refnum, "User"=enum."Car 1", "Last Mouse Position"=[], "Mode"=enum."FCW", "Report Data"={"Coordinate"=[], "Distance"=[], "Degree"=[], "Velocity"=[], "Times"=[]}, "Target 1"="", "Target 2"="", "Velocity"=0.0, "Coordinates(X,Y)"={"X"=0.0, "Y"=0.0}, "Path No."=0, "Input RCS File"="", "Input RCS Data"=[], "Output £m File"="", "DYNAMIC"=[], "DYNAMIC 2"=[], "dy Path  "=[]}  # Data
      w74 = T18 {"State"=enum."Initial", "variant"=variant}
      n12 = disable-structure shown="Disabled" {
        disable-tunnel: "TCP?" -> [w78 _]
        frame Disabled {
          n13 = case shown="True" w78 {
            frame False {
            }
            frame True {
              n14 = flat-sequence {
                tunnel: [w83] -> w79
                tunnel: w79 -> [w88]
                tunnel: [w84] -> _
                frame #0 {
                  n15 = call "client_FGV.vi"("port"=u16 6340, "address"="127.0.0.1", "Enum"=enum16{"open", "idle", "write", "read", "close"}."open") -> ("error constant 2"=w83:errorcluster)  [unwired: 7 in, 1 out]
                }
                frame #1 {
                  n16 = call "client_FGV 2.vi"("error constant"=w88, "port"=u16 6540, "address"="127.0.0.1", "Enum"=enum16{"open", "idle", "write", "read", "close"}."open") -> ("error constant 2"=w84:errorcluster)  [unwired: 6 in, 1 out]
                }
              }
            }
          }
        }
        frame Enabled {
        }
      }
      n17 = Obtain Queue(name (unnamed)="Instrument", element data type=w66) -> (queue out=w71:refnum<queue>, error out=w70:errorcluster)  [unwired: 3 in, 1 out]
      n18 = Obtain Queue(name (unnamed)="RadarGUI", element data type=w74, error in (no error)=w36) -> (queue out=w75:refnum<queue>, error out=w76:errorcluster)  [unwired: 2 in, 1 out]
      n19 = Enqueue Element(queue=w71, element=w66, error in (no error)=w70) -> (queue out=w68:refnum<queue>, error out=w67:errorcluster)  [unwired: 1 in, 1 out]
      n20 = Enqueue Element(queue=w75, element=w74, error in (no error)=w76) -> (queue out=w73:refnum<queue>, error out=w28:errorcluster)  [unwired: 1 in, 1 out]
      n21 = property on="generateWF ok?" class="DigNum (strict)"("Value"=0 ("generateWF ok?")) -> ()  [unwired: 2 in, 2 out]
      n22 = property on="s/d setting" class="Bool (strict)"() -> ("Value"=w40:bool)  [unwired: 2 in, 2 out]
      n23 = property on="load?" class="Bool (strict)"("Value"=FALSE ("load?")) -> ()  [unwired: 2 in, 2 out]
      n24 = property on="Image" class="ImageControl"("ROI"=T14 {"Global Rectangle"=[], "Contours"=[]}) -> ()  [unwired: 2 in, 2 out]
      n25 = Not(x=w40) -> (.not. x?=w39:bool)
      n26 = call <vilib>:"System Exec.vi"("run minimized? (F)"=w31, "wait until completion? (T)"=w33, "error in (no error)"=w36, "command line"="cmd /c ping 192.168.0.19 -t") -> ()  [unwired: 4 in, 4 out]
      n27 = call <vilib>:"System Exec.vi"("run minimized? (F)"=w31, "wait until completion? (T)"=w33, "error in (no error)"=w36, "command line"="cmd /c ping 192.168.0.20 -t") -> ()  [unwired: 4 in, 4 out]
      n28 = Obtain Queue(name (unnamed)="Instrument2", element data type=w54) -> (queue out=w57:refnum<queue>, error out=w56:errorcluster)  [unwired: 3 in, 1 out]
      n29 = Enqueue Element(queue=w57, element=w54, error in (no error)=w56) -> (queue out=w53:refnum<queue>, error out=w52:errorcluster)  [unwired: 1 in, 1 out]
      n30 = Obtain Queue(name (unnamed)="Buffer1", element data type=w60) -> (queue out=w61:refnum<queue>, error out=w62:errorcluster)  [unwired: 3 in, 1 out]
      n31 = property on="dynamic setting" class="Clust (strict)"("Visible"=w39) -> ()  [unwired: 2 in, 2 out]
      n32 = Obtain Queue(name (unnamed)="GPIB", element data type=w48) -> (queue out=w49:refnum<queue>, error out=w50:errorcluster)  [unwired: 3 in, 1 out]
      n33 = property on="s/d setting" class="Bool (strict)"(error in=w28, "Val(Sgnl)"=FALSE ("Value (Signaling)")) -> ()  [unwired: 1 in, 2 out]
      n34 = Enqueue Element(queue=w61, element=w60, error in (no error)=w62) -> (queue out=w59:refnum<queue>, error out=w45:errorcluster)  [unwired: 1 in, 1 out]
      n35 = property on="Inst. Status" class="Bool (strict)"("Value"=FALSE ("Inst. Status")) -> (error out=w26:errorcluster)  [unwired: 2 in, 1 out]
      n36 = Enqueue Element(queue=w49, element=w48, error in (no error)=w50) -> (queue out=w47:refnum<queue>, error out=w44:errorcluster)  [unwired: 1 in, 1 out]
      n37 = property on="Exit" class="Bool (strict)"("Value"=FALSE ("Exit")) -> ()  [unwired: 2 in, 2 out]
      n38 = property on="dynamic setting" class="Clust (strict)"(error in=w26, "Visible"=TRUE) -> ()  [unwired: 1 in, 2 out]
      n39 = Merge Errors(w45, w44) -> (w46:errorcluster)
      "Inst. Status" <- FALSE ("Inst. Status")
      "auto step finish?" <- w37
      "read buffer" <- w41
      "MSG" <- w41
      "autoSliderfinish?" <- w37
      "autoRSfinish?" <- w37
      "autoRs2finish?" <- w37
    }
    frame #2 {
      n40 = Merge Errors(w98, w97, w96, w95) -> (w90:errorcluster)
      n41 = while {
        tunnel: w93 -> [w1117]
        tunnel: w90 -> [w1118]
        shift-right: [w1109] -> _
        shift-left: w100 -> [w1110]
        tunnel: w92 -> [w1108]
        stop <- w1112 stop-if-true
        n42 = Dequeue Element(queue=w1117, error in (no error)=w1118) -> (queue out=w1114:refnum<queue>, element=w1116:cluster{"State":T17, "Variable":variant}, error out=w1113:errorcluster)  [unwired: 1 in, 1 out]
        n43 = Unbundle(w1116) -> ("State"=w1115:T17, "Variable"=w1111:variant)
        n44 = case shown="\"get angle\"" w1115 {
          tunnel: w1114 -> [w1130 w1187 _ _ _ _ _ _ _ _ _ _ _ _ _ _ _ _ _ _ w1446 w1455 _ _ _ _ w1885 w2005 w2314 w2617 w2857 _ _ _ _ w3343 w3371]
          tunnel: w1113 -> [w1119 w1188 _ w1223 w1227 w1242 w1304 w1310 w1316 w1322 w1328 w1334 _ _ w1406 w1412 w1418 w1424 w1430 w1436 w1451 w1454 w1463 w1591 w1706 w1767 w1886 w2007 w2316 w2619 w2858 w2870 w2877 w3047 w3138 w3342 w3372]
          tunnel: [_ _ w1208 _ _ _ _ _ _ _ _ _ _ _ _ _ _ _ _ _ _ _ _ _ _ _ _ _ _ _ _ _ _ _ _ _ TRUE] -> w1112
          tunnel: w1111 -> [_ _ _ w1222 w1228 _ w1303 w1309 w1315 w1321 w1327 w1333 _ _ w1405 w1411 w1417 w1423 w1429 w1435 w1450 _ _ _ _ _ _ _ _ _ _ w2869 _ w3060 _ _ _]
          tunnel: [w1128 w1189 w1196 w1219 w1225 w1244 w1301 w1307 w1313 w1319 w1325 w1331 w1335 w1383 w1403 w1409 w1415 w1421 w1427 w1433 w1444 w1453 w1461 w1589 w1704 w1764 w1896 w2003 w2311 w2614 w2854 w2865 w2878 w3050 w3139 w3339 w3378] -> w1109
          tunnel: w1110 -> [w1129 w1169 w1196 w1220 w1226 w1245 w1302 w1308 w1314 w1320 w1326 w1332 w1342 w1384 w1404 w1410 w1416 w1422 w1428 w1434 w1445 w1453 w1462 w1590 w1705 w1765 w1896 w2004 w2312 w2615 w2855 w2866 w2879 w3033 w3140 w3339 w3374]
          tunnel: w1108 -> [_ _ _ _ _ _ _ _ _ _ _ _ _ _ _ _ _ _ _ _ _ _ _ _ _ _ _ _ _ _ _ _ _ w3055 _ _ _]
          frame "Idle", Default {
            n45 = Unbundle By Name(w1129) -> ("Connect"=w1132:bool, "phandle out"=w1131:u32)
            n46 = case shown="True" w1132 {
              tunnel: w1131 -> [_ w1151]
              tunnel: w1130 -> [_ w1149]
              tunnel: [_ w1147] -> w1127
              tunnel: [_ w1146] -> w1126
              tunnel: [_ w1144] -> w1125
              tunnel: [_ w1143] -> w1124
              tunnel: [_ w1141] -> w1123
              tunnel: [_ w1140] -> w1122
              tunnel: [_ w1138] -> w1121
              tunnel: [_ w1137] -> w1120
              tunnel: w1119 -> [w1133 w1135]
              tunnel: [w1133 w1134] -> _
              frame False {
              }
              frame True {
                n47 = Enqueue Element(queue=w1149, element=cluster{"State":T17, "Variable":variant} {"State"=enum."Update", "Variable"=variant}, error in (no error)=w1135) -> (error out=w1134:errorcluster)  [unwired: 1 in, 2 out]
                n48 = for {
                  tunnel: w1151 -> [w1162]
                  tunnel: [w1161] -> w1145 mode=indexing
                  tunnel: [w1160] -> w1142 mode=indexing
                  tunnel: [w1159] -> w1139 mode=indexing
                  tunnel: i32[] [0, 1] -> [w1158] mode=indexing
                  tunnel: [w1152] -> w1148 mode=indexing
                  n49 = call "Idle.vi"("iaxis"=w1158, "handle"=w1162) -> ("Axis"=w1159:i32, "Speed"=w1160:sgl, "Dpos"=w1161:sgl, "State"=w1156:i32)  [unwired: 5 in, 1 out]
                  n50 = Equal?(x=w1156, y=0) -> (x = y?=w1155:bool)
                  n51 = Select(t="Running", s=w1155, f="Stop") -> (s? t:f=w1152:string)
                }
                n52 = Index Array(array=w1148) -> (element #1=w1147:string, element #2=w1146:string)  [unwired: 2 in]
                n53 = Index Array(array=w1145) -> (element #1=w1144:sgl, element #2=w1143:sgl)  [unwired: 2 in]
                n54 = Index Array(array=w1142) -> (element #1=w1141:sgl, element #2=w1140:sgl)  [unwired: 2 in]
                n55 = Index Array(array=w1139) -> (element #1=w1138:i32, element #2=w1137:i32)  [unwired: 2 in]
              }
            }
            n56 = Bundle By Name(cluster=w1129, "X Axis.Operating State"=w1127, "Y Axis.Operating State"=w1126, "X Axis.Current Position"=w1125, "Y Axis.Current Position"=w1124, "X Axis.Current Speed"=w1123, "Y Axis.Current Speed"=w1122, "X Axis.Axis State"=w1121, "Y Axis.Axis State"=w1120) -> (w1128:T24)
          }
          frame "Initial" {
            w1166 = T28 {"Operating State"="", "Current Position"=0.0, "Current Speed"=0.0, "Axis State"=0, "Angle"=0} ("X Axis")
            w1182 = enum16{"X", "Y", "X+Y"}[] [enum."X"] items=["X", "Y", "X+Y"] ("Axis")
            n57 = Enqueue Element(queue=w1187, element=cluster{"State":T17, "Variable":variant} {"State"=enum."Update", "Variable"=variant}, error in (no error)=w1188) -> (error out=w1163:errorcluster)  [unwired: 1 in, 2 out]
            n58 = Bundle By Name(cluster=w1169, "Step Flag"=FALSE, "X Axis.Angle"=T20."0" ("Angle"), "Distance"=0.0, "Direct of movement"=enum16{"Forward", "Backward"}."Forward", "Move Method"=enum16{"Continue", "Inching"}."Continue" ("Move Mode"), "X Axis"=w1166, "Y Axis"=w1166, "Start Time"=0.0) -> (w1168:T24)
            n59 = property on="Run Time (sec)" class="DigNum (strict)"(error in=w1163, "Value"=0.0 ("Run Time (ms)")) -> ()  [unwired: 1 in, 2 out]
            n60 = Bundle By Name(cluster=w1168, "Speed"=10000.0, "Creep"=30.0, "S ramp"=30.0, "Acceleration"=100000.0, "Deceleration"=100000.0, "Initial Speed"=10.0, "Normal Open / Close"=enum16{"Open", "Close"}."Close", "Axis"=w1182, "phandle out"=u32 0, "Connect"=FALSE, "App State"="Initial Done", "Times"=0) -> (w1189:T24)
          }
          frame "Update" {
            w1202 = "Running"
            n61 = Unbundle By Name(w1196) -> ("Axis"=w1207:enum16{"X", "Y", "X+Y"}[], "X Axis"=w1195:T12, "Y Axis"=w1194:T12, "Connect"=→"Connect":bool, "App State"=w1193:string)
            "X Axis" <- w1195
            "Y Axis" <- w1194
            "APP State" <- w1193
            n62 = Unbundle By Name(w1194) -> ("Operating State"=w1201:string, "Current Position"=w1206:dbl)
            n63 = Unbundle By Name(w1195) -> ("Current Position"=w1203:dbl, "Operating State"=w1200:string)
            n64 = property on="Axis" class="Arr (strict)"("Value"=w1207) -> ()  [unwired: 2 in, 2 out]
            n65 = Equal?(x=w1193, y="Exit") -> (x = y?=w1208:bool)
            n66 = Divide(x=w1203, y=1000.0) -> (x/y=→"X Position (cm)":dbl)
            n67 = Divide(x=w1206, y=1000.0) -> (x/y=→"Y Position (cm)":dbl)
            n68 = Equal?(x=w1200, y=w1202) -> (x = y?=w1198:bool)
            n69 = Equal?(x=w1202, y=w1201) -> (x = y?=w1199:bool)
            n70 = Or(x=w1198, y=w1199) -> (x .or. y?=w1197:bool)
            n71 = case shown="False" w1197 {
              tunnel: w1196 -> [_ w1217]
              frame False {
                n72 = property on="auto step finish?" class="Bool (strict)"() -> ("Value"=w1211:bool)  [unwired: 2 in, 2 out]
                n73 = Not(x=w1211) -> (.not. x?=w1210:bool)
                n74 = case shown="True" w1210 {
                  frame False {
                  }
                  frame True {
                    w1212 = TRUE ("auto step")
                    n75 = property on="autoSliderfinish?" class="Bool (strict)"("Value"=w1212) -> ()  [unwired: 2 in, 2 out]
                    n76 = property on="auto step finish?" class="Bool (strict)"("Value"=w1212) -> ()  [unwired: 2 in, 2 out]
                  }
                }
              }
              frame True {
                n77 = Unbundle By Name(w1217) -> ("Start Time"=w1216:dbl)
                n78 = Get Date/Time In Seconds() -> (seconds since 1Jan1904=w1215:timestamp)
                n79 = To Double Precision Float(number=w1215) -> (double precision float=w1214:dbl)
                n80 = Subtract(x=w1214, y=w1216) -> (x-y=→"Run Time (sec)":dbl)
              }
            }
          }
          frame "Axis" {
            w1221 = enum16{"X", "Y", "X+Y"}[] [] items=["X", "Y", "X+Y"] ("Axis")
            n81 = Variant To Data(error in=w1223, type=w1221, Variant=w1222) -> (data=w1218:enum16{"X", "Y", "X+Y"}[])  [unwired: 1 out]
            n82 = Bundle By Name(cluster=w1220, "Axis"=w1218) -> (w1219:T24)
          }
          frame "reset xy" {
            n83 = Unbundle By Name(w1226) -> ("phandle out"=w1239:u32)
            n84 = Variant To Data(error in=w1227, type=cluster{"reset y":bool, "reset x ":bool} {"reset y"=FALSE, "reset x "=FALSE} ("Cluster 2"), Variant=w1228) -> (data=w1231:cluster{"reset y":bool, "reset x ":bool}, error out=w1238:errorcluster)
            n85 = Unbundle By Name(w1231) -> ("reset x"=w1229:bool, "reset y"=w1230:bool)
            n86 = Build Array(w1230, w1229) -> (w1232:bool[])
            n87 = Boolean Array To Number(Boolean array=w1232) -> (number=w1237:u32)
            n88 = Build Array(w1237) -> (w1236:u32[])
            n89 = Byte Array To String(unsigned byte array=w1236) -> (string=w1235:string)
            n90 = call "Z Aux Modbus Set0x.vi"("pdata"=w1235, "error in (no error)"=w1238, "inum"=u16 2, "start"=u16 20010, "handle"=w1239) -> ("handle out"=w1224:u32)  [unwired: 3 in, 3 out]
            n91 = Bundle By Name(cluster=w1226, "phandle out"=w1224) -> (w1225:T24)
          }
          frame "reset ant" {
            w1241 = 0.0 ("X Axis.Angle")
            n92 = Unbundle By Name(w1245) -> ("phandle out"=w1246:u32)
            n93 = stacked-sequence {
              tunnel: w1246 -> [w1256 w1258 w1279 w1295]
              tunnel: [_ _ _ w1286] -> _
              tunnel: [_ _ _ w1285] -> w1243
              tunnel: w1242 -> [w1249 w1260 w1278 w1294]
              frame #0 {
                w1248 = TRUE
                n94 = Build Array(w1248, w1248) -> (w1250:bool[])
                n95 = Boolean Array To Number(Boolean array=w1250) -> (number=w1255:u32)
                n96 = Build Array(w1255) -> (w1254:u32[])
                n97 = Byte Array To String(unsigned byte array=w1254) -> (string=w1253:string)
                n98 = call "Z Aux Modbus Set0x.vi"("pdata"=w1253, "error in (no error)"=w1249, "inum"=u16 2, "start"=u16 20010, "handle"=w1256) -> ("error out"=w1247:errorcluster)  [unwired: 3 in, 3 out]
                n99 = flat-sequence {
                  tunnel: w1247 -> [_]
                  frame #0 {
                    n100 = Wait (ms)(milliseconds to wait=u32 100) -> ()  [unwired: 1 out]
                  }
                }
              }
              frame #1 {
                w1259 = FALSE
                n101 = Build Array(w1259, w1259) -> (w1261:bool[])
                n102 = Boolean Array To Number(Boolean array=w1261) -> (number=w1266:u32)
                n103 = Build Array(w1266) -> (w1265:u32[])
                n104 = Byte Array To String(unsigned byte array=w1265) -> (string=w1264:string)
                n105 = call "Z Aux Modbus Set0x.vi"("pdata"=w1264, "error in (no error)"=w1260, "inum"=u16 2, "start"=u16 20010, "handle"=w1258) -> ()  [unwired: 3 in, 4 out]
                n106 = flat-sequence {
                  frame #0 {
                    n107 = Wait (ms)(milliseconds to wait=u32 100) -> ()  [unwired: 1 out]
                  }
                }
              }
              frame #2 {
                w1273 = u16 1 ("inum")
                n108 = Build Array(TRUE) -> (w1276:bool[])
                n109 = Boolean Array To Number(Boolean array=w1276) -> (number=w1282:u32)
                n110 = Build Array(w1282) -> (w1281:u32[])
                n111 = Byte Array To String(unsigned byte array=w1281) -> (string=w1275:string)
                n112 = call "Z Aux Modbus Set0x.vi"("pdata"=w1275, "error in (no error)"=w1278, "inum"=w1273, "start"=u16 20038, "handle"=w1279) -> ("error out"=w1272:errorcluster, "handle out"=w1271:u32)  [unwired: 3 in, 2 out]
                n113 = call "Z Aux Modbus Set0x.vi"("pdata"=w1275, "error in (no error)"=w1272, "inum"=w1273, "start"=u16 20046, "handle"=w1271) -> ("error out"=w1270:errorcluster)  [unwired: 3 in, 3 out]
                n114 = flat-sequence {
                  tunnel: w1270 -> [w1283]
                  tunnel: [w1283] -> w1269
                  frame #0 {
                    n115 = Wait (ms)(milliseconds to wait=u32 5000) -> ()  [unwired: 1 out]
                  }
                }
                n116 = property on="reset ant" class="Bool (strict)"(error in=w1269, "Value"=FALSE ("reset ant")) -> ()  [unwired: 1 in, 2 out]
              }
              frame #3 {
                w1289 = u16 1 ("inum")
                n117 = Build Array(FALSE) -> (w1292:bool[])
                n118 = Boolean Array To Number(Boolean array=w1292) -> (number=w1298:u32)
                n119 = Build Array(w1298) -> (w1297:u32[])
                n120 = Byte Array To String(unsigned byte array=w1297) -> (string=w1291:string)
                n121 = call "Z Aux Modbus Set0x.vi"("pdata"=w1291, "error in (no error)"=w1294, "inum"=w1289, "start"=u16 20038, "handle"=w1295) -> ("error out"=w1288:errorcluster, "handle out"=w1287:u32)  [unwired: 3 in, 2 out]
                n122 = call "Z Aux Modbus Set0x.vi"("pdata"=w1291, "error in (no error)"=w1288, "inum"=w1289, "start"=u16 20046, "handle"=w1287) -> ("error out"=w1286:errorcluster, "handle out"=w1285:u32)  [unwired: 3 in, 2 out]
              }
            }
            n123 = Bundle By Name(cluster=w1245, "phandle out"=w1243, "X Axis.Angle"=w1241, "Y Axis.Angle"=w1241) -> (w1244:T24)
          }
          frame "Creep" {
            n124 = Variant To Data(error in=w1304, type=0.0, Variant=w1303) -> (data=w1300:dbl)  [unwired: 1 out]
            n125 = Bundle By Name(cluster=w1302, "Creep"=w1300) -> (w1301:T24)
          }
          frame "Acceleration" {
            n126 = Variant To Data(error in=w1310, type=0.0, Variant=w1309) -> (data=w1306:dbl)  [unwired: 1 out]
            n127 = Bundle By Name(cluster=w1308, "Acceleration"=w1306) -> (w1307:T24)
          }
          frame "Deceleration" {
            n128 = Variant To Data(error in=w1316, type=0.0, Variant=w1315) -> (data=w1312:dbl)  [unwired: 1 out]
            n129 = Bundle By Name(cluster=w1314, "Deceleration"=w1312) -> (w1313:T24)
          }
          frame "Sramp" {
            n130 = Variant To Data(error in=w1322, type=0.0, Variant=w1321) -> (data=w1318:dbl)  [unwired: 1 out]
            n131 = Bundle By Name(cluster=w1320, "S ramp"=w1318) -> (w1319:T24)
          }
          frame "Initail Speed" {
            n132 = Variant To Data(error in=w1328, type=0.0, Variant=w1327) -> (data=w1324:dbl)  [unwired: 1 out]
            n133 = Bundle By Name(cluster=w1326, "Initial Speed"=w1324) -> (w1325:T24)
          }
          frame "Speed" {
            n134 = Variant To Data(error in=w1334, type=0.0, Variant=w1333) -> (data=w1330:dbl)  [unwired: 1 out]
            n135 = Bundle By Name(cluster=w1332, "Speed"=w1330) -> (w1331:T24)
          }
          frame "get angle" {
            n136 = local read "Report Data.Degree"() -> (w1367:dbl[][])
            n137 = property on="X_MID" class="DigNum (strict)"() -> ("Value"=w1349:dbl)  [unwired: 2 in, 2 out]
            n138 = Bundle By Name(cluster=cluster{"X":dbl, "Y":dbl} {"X"=24500.0, "Y"=24500.0} ("Center Post Pulse"), "X"="X_Vert_Dist(mm)", "Y"="Y_Vert_Dist(mm)") -> (w1344:cluster{"X":dbl, "Y":dbl})
            n139 = property on="Y_MID" class="DigNum (strict)"() -> ("Value"=w1348:dbl)  [unwired: 2 in, 2 out]
            n140 = Index Array(array=w1367, index (row)=0 ("disabled index (col)")) -> (element=w1354:dbl[])  [unwired: 1 in]
            "x angle" <- w1354
            n141 = Index Array(array=w1367, index (row)=1 ("index (col)")) -> (element=w1352:dbl[])  [unwired: 1 in]
            "y angle" <- w1352
            n142 = Bundle By Name(cluster=cluster{"X":dbl, "Y":dbl} {"X"=72700.0, "Y"=72100.0} ("Center Post Pulse"), "X"=w1349, "Y"=w1348) -> (w1350:cluster{"X":dbl, "Y":dbl})
            n143 = Negate(x=w1352) -> (-x=w1351:dbl[])
            n144 = Negate(x=w1354) -> (-x=w1353:dbl[])
            n145 = call "get angle index.vi"("Center Post Pulse"=w1350, "Vert_Dist"=w1344, "y angle"=w1351, "x angle"=w1353) -> ("y dist"=w1339:dbl[], "x  dist"=w1341:dbl[], "angle"=w1355:dbl[], "appended array"=w1364:dbl[][], "y"=w1357:i32[][], "x"=w1356:i32[][])  [unwired: 2 in]
            "x angle array" <- w1356
            "y angle array" <- w1357
            n146 = property on="User" class="Enum (strict)"() -> ("Value"=w1338:enum16{"Car A", "Car B"})  [unwired: 2 in, 2 out]
            n147 = Index Array(array=w1364, index (row)=0) -> (element=w1363:dbl[])  [unwired: 1 in]
            n148 = Index Array(array=w1364, index (row)=1) -> (element=w1361:dbl[])  [unwired: 1 in]
            n149 = case shown="\"Car A\", Default" w1338 {
              tunnel: w1341 -> [w1380 _]
              tunnel: [w1380 w1381] -> w1340
              tunnel: w1339 -> [_ w1381]
              frame "Car A", Default {
              }
              frame "Car B" {
              }
            }
            "dist" <- w1340
            n150 = Index Array(array=w1363) -> (element=w1362:dbl)  [unwired: 1 in]
            n151 = Index Array(array=w1361) -> (element=w1360:dbl)  [unwired: 1 in]
            n152 = Bundle By Name(cluster=w1342, "x angle array"=w1356, "X Axis.Angle"=w1362, "Y Axis.Angle"=w1360, "x  dist"=w1341, "y dist"=w1339, "y angle array"=w1357, "big angle"=w1355) -> (w1337:T24)
            n153 = property on="s/d setting" class="Bool (strict)"() -> ("Value"=w1336:bool)  [unwired: 2 in, 2 out]
            n154 = case shown="False" w1336 {
              tunnel: w1337 -> [w1375 w1379]
              tunnel: [w1374 w1379] -> w1335
              frame False {
                n155 = property on="DYNAMIC" class="Arr (strict)"() -> ("Value"=w1378:T1)  [unwired: 2 in, 2 out]
                n156 = property on="DYNAMIC 2" class="Arr (strict)"() -> ("Value"=w1377:T1)  [unwired: 2 in, 2 out]
                n157 = property on="Array" class="Arr (strict)"() -> ("Value"=w1376:T2)  [unwired: 2 in, 2 out]
                n158 = call "dy xy calc speed .vi"("DYNAMIC 2"=w1377, "DYNAMIC"=w1378, "Array 2"=w1376, "Data IN"=w1375) -> ("dy Path"=w1368:T8, "Data out"=w1374:T24)  [unwired: 6 in]
                n159 = Unbundle By Name(w1374) -> ("x dy time"=w1369:dbl[], "xy dy speed table"=w1373:dbl[][])
                "time" <- w1369
                n160 = property on="dy Path" class="Arr (strict)"("Value"=w1368) -> ()  [unwired: 2 in, 2 out]
                n161 = Array Size(array=w1369) -> (size(s)=w1372:i32)
                n162 = Decrement(x=w1372) -> (x-1=w1371:i32)
                n163 = Index Array(array=w1369, index=w1371) -> (element=→"last time":dbl)
                n164 = property on="SPEED" class="Arr (strict)"("Value"=w1373) -> ()  [unwired: 2 in, 2 out]
              }
              frame True {
              }
            }
          }
          frame "set speed" {
            n165 = case shown="\"manual\", Default" "AS mode" {
              tunnel: w1384 -> [w1396]
              tunnel: [w1395] -> w1383
              frame "manual", Default {
                w1390 = 10000.0
                n166 = property on="dy Path" class="Arr (strict)"() -> ("Value"=w1394:T8)  [unwired: 2 in, 2 out]
                n167 = Index Array(array=w1394) -> (element #1=w1393:T29, element #2=w1392:T29)  [unwired: 4 in]
                n168 = for {
                  tunnel: w1393 -> [w1400] mode=indexing
                  tunnel: [w1399] -> w1391 mode=indexing
                  n169 = Unbundle(w1400) -> ("Axis Speed"=w1399:dbl)  [unwired: 3 out]
                }
                n170 = for {
                  tunnel: w1392 -> [w1398] mode=indexing
                  tunnel: [w1397] -> w1389 mode=indexing
                  n171 = Unbundle(w1398) -> ("Axis Speed"=w1397:dbl)  [unwired: 3 out]
                }
                n172 = Build Array (concatenate)(w1390, w1389) -> (w1387:dbl[])
                n173 = Build Array (concatenate)(w1390, w1391) -> (w1388:dbl[])
                n174 = Build Array(w1388, w1387) -> (w1386:dbl[][])
                n175 = Transpose 2D Array(2D array=w1386) -> (transposed array=w1385:dbl[][])
                n176 = Bundle By Name(cluster=w1396, "x dy speed table"=w1388, "y dy speed table"=w1387, "xy dy speed table"=w1385, "dy Path"=w1394) -> (w1395:T24)
              }
            }
          }
          frame "Distance" {
            n177 = Variant To Data(error in=w1406, type=0.0, Variant=w1405) -> (data=w1402:dbl)  [unwired: 1 out]
            n178 = Bundle By Name(cluster=w1404, "Distance"=w1402) -> (w1403:T24)
          }
          frame "Move Mode" {
            n179 = Variant To Data(error in=w1412, type=enum16{"Relative", "Absolute"}."Relative" ("Move Mode"), Variant=w1411) -> (data=w1408:enum16{"Relative", "Absolute"})  [unwired: 1 out]
            n180 = Bundle By Name(cluster=w1410, "Move Mode"=w1408) -> (w1409:T24)
          }
          frame "Move Method" {
            n181 = Variant To Data(error in=w1418, type=enum16{"Continue", "Inching"}."Inching" ("Move Mode"), Variant=w1417) -> (data=w1414:enum16{"Continue", "Inching"})  [unwired: 1 out]
            n182 = Bundle By Name(cluster=w1416, "Move Method"=w1414) -> (w1415:T24)
          }
          frame "Direct of Movement" {
            n183 = Variant To Data(error in=w1424, type=enum16{"Forward", "Backward"}."Forward" ("Direct of movement"), Variant=w1423) -> (data=w1420:enum16{"Forward", "Backward"})  [unwired: 1 out]
            n184 = Bundle By Name(cluster=w1422, "Direct of movement"=w1420) -> (w1421:T24)
          }
          frame "Normal Open" {
            n185 = Variant To Data(error in=w1430, type=enum16{"Open", "Close"}."Close" ("Normal Open / Close"), Variant=w1429) -> (data=w1426:enum16{"Open", "Close"})  [unwired: 1 out]
            n186 = Bundle By Name(cluster=w1428, "Normal Open / Close"=w1426) -> (w1427:T24)
          }
          frame "Angle" {
            n187 = Variant To Data(error in=w1436, type=T11."0" ("Rotate"), Variant=w1435) -> (data=w1432:T11)  [unwired: 1 out]
            n188 = Bundle By Name(cluster=w1434, "Angle"=w1432) -> (w1433:T24)
          }
          frame "Connect" {
            n189 = Variant To Data(error in=w1451, type="", Variant=w1450) -> (data=w1448:string, error out=w1447:errorcluster)
            n190 = call "Z Aux Open Eth.vi"("error in (no error)"=w1447, "ipaddr"=w1448) -> ("error out"=w1437:errorcluster, "phandle out"=w1439:u32)  [unwired: 6 in, 2 out]
            n191 = Not Equal To 0?(x=w1439) -> (x != 0?=w1438:bool)
            n192 = Select(t="Connect done.", s=w1438, f="Connect Fail" ("t")) -> (s? t:f=w1443:string)
            n193 = Bundle By Name(cluster=w1445, "phandle out"=w1439, "Connect"=w1438, "App State"=w1443) -> (w1444:T24)
            n194 = Enqueue Element(queue=w1446, element=cluster{"State":T17, "Variable":variant} {"State"=enum."Update", "Variable"=variant}, error in (no error)=w1437) -> ()  [unwired: 1 in, 3 out]
          }
          frame "Move&Rotate" {
            n195 = for {
              tunnel: w1455 -> [w1459]
              shift-right: [w1458] -> _
              shift-left: w1454 -> [w1457]
              tunnel: cluster{"State":T17, "Variable":variant}[] [{"State"=enum."Inching", "Variable"=variant}, {"State"=enum."Rotate_2", "Variable"=variant}] -> [w1456] mode=indexing
              n196 = Enqueue Element(queue=w1459, element=w1456, error in (no error)=w1457) -> (error out=w1458:errorcluster)  [unwired: 1 in, 2 out]
            }
          }
          frame "Rotate" {
            n197 = Unbundle By Name(w1462) -> ("Angle"=w1460:T11, "phandle out"=w1465:u32, "Axis"=w1464:enum16{"X", "Y", "X+Y"}[])
            n198 = for {
              tunnel: w1465 -> [w1480]
              tunnel: w1464 -> [w1479] mode=indexing
              tunnel: w1460 -> [w1466]
              shift-right: [w1471] -> _
              shift-left: w1463 -> [w1472]
              shift-right: [w1469] -> w1461
              shift-left: w1462 -> [w1470]
              n199 = To Unsigned Long Integer(number=w1466) -> (unsigned 32bit integer=w1468:u32)
              n200 = disable-structure shown="Enabled" {
                disable-tunnel: u32 128 -> [w1493 _]
                disable-tunnel: [w1492 u32 1] -> w1477
                disable-tunnel: w1468 -> [w1491 _]
                frame Disabled {
                  n201 = Add(x=w1493, y=w1491) -> (x+y=w1492:u32)
                }
                frame Enabled {
                }
              }
              n202 = case shown="\"34\"" w1466 {
                tunnel: [0.0 1.0 10.0 30.0 34.0 60.0 90.0 180.0 -1.0 -10.0] -> w1467
                frame "0", Default {
                }
                frame "1" {
                }
                frame "10" {
                }
                frame "30" {
                }
                frame "34" {
                }
                frame "60" {
                }
                frame "90" {
                }
                frame "180" {
                }
                frame "-1" {
                }
                frame "-10" {
                }
              }
              n203 = Build Array(w1477) -> (w1476:u32[])
              n204 = Build Array(w1468) -> (w1474:u32[])
              n205 = Byte Array To String(unsigned byte array=w1476) -> (string=w1475:string)
              n206 = Byte Array To String(unsigned byte array=w1474) -> (string=w1473:string)
              n207 = case shown="\"X+Y\"" w1479 {
                tunnel: w1480 -> [w1510 w1537 w1564]
                tunnel: w1475 -> [w1511 w1538 w1565]
                tunnel: w1473 -> [w1509 w1536 w1563]
                tunnel: w1472 -> [w1504 w1531 w1560]
                tunnel: [w1499 w1526 w1556] -> w1471
                tunnel: w1470 -> [w1498 w1525 w1553]
                tunnel: [w1497 w1524 w1552] -> w1469
                tunnel: w1467 -> [w1496 w1523 w1549]
                tunnel: w1466 -> [w1495 w1522 _]
                frame "Y" {
                  w1505 = u16 20047 ("start")
                  n208 = case shown="\"0\"" w1495 {
                    tunnel: w1498 -> [w1516 w1521]
                    tunnel: [w1515 w1520] -> w1497
                    tunnel: w1496 -> [w1514 w1517]
                    frame "0" {
                      n209 = Bundle By Name(cluster=w1516, "Y Axis.Angle"=w1514) -> (w1515:T24)
                    }
                    frame Default {
                      n210 = Unbundle By Name(w1521) -> ("Y Axis.Angle"=w1518:dbl)
                      n211 = Add(x=w1517, y=w1518) -> (x+y=w1519:dbl)
                      n212 = Bundle By Name(cluster=w1521, "Y Axis.Angle"=w1519) -> (w1520:T24)
                    }
                  }
                  n213 = call "Z Aux Modbus Set0x.vi"("pdata"=w1509, "error in (no error)"=w1504, "inum"=u16 8, "start"=u16 20040, "handle"=w1510) -> ("error out"=w1502:errorcluster, "handle out"=w1503:u32)  [unwired: 3 in, 2 out]
                  n214 = call "Delay Time.vi"("error in (no error)"=w1502, "Delay(ms)"=u32 30) -> ("error out"=w1500:errorcluster)  [unwired: 9 in]
                  n215 = call "Z Aux Modbus Set0x.vi"("pdata"=w1511, "error in (no error)"=w1500, "inum"=u16 1, "start"=w1505, "handle"=w1503) -> ("error out"=w1513:errorcluster, "handle out"=w1512:u32)  [unwired: 3 in, 2 out]
                  n216 = call "Check Rotate Done.vi"("error in (no error)"=w1513, "start"=w1505, "phandle in"=w1512) -> ("error out"=w1499:errorcluster)  [unwired: 8 in]
                }
                frame "X" {
                  w1532 = u16 20039 ("start")
                  n217 = case shown="\"0\"" w1522 {
                    tunnel: w1525 -> [w1543 w1548]
                    tunnel: [w1542 w1547] -> w1524
                    tunnel: w1523 -> [w1541 w1544]
                    frame "0" {
                      n218 = Bundle By Name(cluster=w1543, "X Axis.Angle"=w1541) -> (w1542:T24)
                    }
                    frame Default {
                      n219 = Unbundle By Name(w1548) -> ("X Axis.Angle"=w1546:dbl)
                      n220 = Add(x=w1544, y=w1546) -> (x+y=w1545:dbl)
                      n221 = Bundle By Name(cluster=w1548, "X Axis.Angle"=w1545) -> (w1547:T24)
                    }
                  }
                  n222 = call "Z Aux Modbus Set0x.vi"("pdata"=w1536, "error in (no error)"=w1531, "inum"=u16 8, "start"=u16 20032, "handle"=w1537) -> ("error out"=w1529:errorcluster, "handle out"=w1530:u32)  [unwired: 3 in, 2 out]
                  n223 = call "Delay Time.vi"("error in (no error)"=w1529, "Delay(ms)"=u32 30) -> ("error out"=w1527:errorcluster)  [unwired: 9 in]
                  n224 = call "Z Aux Modbus Set0x.vi"("pdata"=w1538, "error in (no error)"=w1527, "inum"=u16 1, "start"=w1532, "handle"=w1530) -> ("error out"=w1540:errorcluster, "handle out"=w1539:u32)  [unwired: 3 in, 2 out]
                  n225 = call "Check Rotate Done.vi"("error in (no error)"=w1540, "start"=w1532, "phandle in"=w1539) -> ("error out"=w1526:errorcluster)  [unwired: 8 in]
                }
                frame "X+Y" {
                  n226 = Unbundle By Name(w1553) -> ("X Axis.Angle"=w1555:dbl, "Y Axis.Angle"=w1554:dbl)
                  n227 = for {
                    tunnel: w1563 -> [w1579]
                    shift-right: [w1578] -> w1558
                    shift-left: w1564 -> [w1580]
                    tunnel: i32[] [20032, 20040] -> [w1576] mode=indexing
                    tunnel: w1560 -> [w1575]
                    tunnel: [w1574] -> w1559
                    n228 = call "Z Aux Modbus Set0x.vi"("pdata"=w1579, "error in (no error)"=w1575, "inum"=u16 8, "start"=w1576, "handle"=w1580) -> ("error out"=w1574:errorcluster, "handle out"=w1578:u32)  [unwired: 3 in, 2 out]
                  }
                  n229 = call "Delay Time.vi"("error in (no error)"=w1559) -> ("error out"=w1557:errorcluster)  [unwired: 10 in]
                  n230 = Add(x=w1549, y=w1555) -> (x+y=w1551:dbl)
                  n231 = Add(x=w1554, y=w1549) -> (x+y=w1550:dbl)
                  n232 = for {
                    tunnel: w1565 -> [w1571]
                    tunnel: w1558 -> [w1570]
                    tunnel: i32[] [20039, 20047] -> [w1568] mode=indexing
                    tunnel: w1557 -> [w1567]
                    tunnel: [w1566] -> w1556
                    n233 = call "Z Aux Modbus Set0x.vi"("pdata"=w1571, "error in (no error)"=w1567, "inum"=u16 1, "start"=w1568, "handle"=w1570) -> ("error out"=w1573:errorcluster, "handle out"=w1572:u32)  [unwired: 3 in, 2 out]
                    n234 = call "Check Rotate Done.vi"("error in (no error)"=w1573, "start"=w1568, "phandle in"=w1572) -> ("error out"=w1566:errorcluster)  [unwired: 8 in]
                  }
                  n235 = Bundle By Name(cluster=w1553, "X Axis.Angle"=w1551, "Y Axis.Angle"=w1550) -> (w1552:T24)
                }
              }
            }
          }
          frame "Rotate_2" {
            n236 = Unbundle By Name(w1590) -> ("Distance"=w1581:dbl, "phandle out"=w1593:u32, "Axis"=w1592:enum16{"X", "Y", "X+Y"}[])
            n237 = Absolute Value(x=w1581) -> (abs(x)=w1582:dbl)
            n238 = Divide(x=w1582, y=1000.0) -> (x/y=w1587:dbl)
            n239 = Build Array(u32 1) -> (w1585:u32[])
            n240 = Absolute Value(x=w1587) -> (abs(x)=w1583:dbl)
            n241 = Byte Array To String(unsigned byte array=w1585) -> (string=w1584:string)
            n242 = for {
              tunnel: w1593 -> [w1602]
              tunnel: w1592 -> [w1601] mode=indexing
              shift-right: [w1599] -> _
              shift-left: w1591 -> [w1600]
              shift-right: [w1597] -> w1589
              shift-left: w1590 -> [w1598]
              tunnel: w1584 -> [w1596]
              tunnel: w1583 -> [w1595]
              tunnel: w1581 -> [w1594]
              n243 = for {
                N: w1595 -> [_]
                tunnel: w1602 -> [w1610]
                tunnel: w1601 -> [w1609]
                tunnel: w1596 -> [w1604]
                shift-right: [w1607] -> w1599
                shift-left: w1600 -> [w1608]
                shift-right: [w1605] -> w1597
                shift-left: w1598 -> [w1606]
                tunnel: w1594 -> [w1603]
                n244 = case shown="\"X\"" w1609 {
                  tunnel: w1610 -> [w1635 w1666 w1671]
                  tunnel: w1604 -> [w1636 w1648 w1672]
                  tunnel: w1608 -> [w1630 w1665 w1670]
                  tunnel: [w1625 w1664 w1669] -> w1607
                  tunnel: w1606 -> [w1624 w1663 w1668]
                  tunnel: [w1623 w1662 w1667] -> w1605
                  tunnel: w1603 -> [w1611 w1640 _]
                  frame "Y" {
                    w1631 = u16 20047 ("start")
                    n245 = Greater Than 0?(x=w1611) -> (x > 0?=w1613:bool)
                    n246 = Select(t=u32 55 ("number"), s=w1613, f=u32 54 ("number")) -> (s? t:f=w1617:u32)
                    n247 = Build Array(w1617) -> (w1618:u32[])
                    n248 = Byte Array To String(unsigned byte array=w1618) -> (string=w1616:string)
                    n249 = call "Z Aux Modbus Set0x.vi"("pdata"=w1616, "error in (no error)"=w1630, "inum"=u16 8, "start"=u16 20040, "handle"=w1635) -> ("error out"=w1628:errorcluster, "handle out"=w1629:u32)  [unwired: 3 in, 2 out]
                    n250 = Select(t=0.21 ("x"), s=w1613, f=-0.21 ("x")) -> (s? t:f=w1612:dbl)
                    n251 = Unbundle By Name(w1624) -> ("X Axis.Angle"=w1621:dbl)
                    n252 = call "Delay Time.vi"("error in (no error)"=w1628, "Delay(ms)"=u32 30) -> ("error out"=w1626:errorcluster)  [unwired: 9 in]
                    n253 = Add(x=w1612, y=w1621) -> (x+y=w1622:dbl)
                    n254 = call "Z Aux Modbus Set0x.vi"("pdata"=w1636, "error in (no error)"=w1626, "inum"=u16 1, "start"=w1631, "handle"=w1629) -> ("error out"=w1638:errorcluster, "handle out"=w1637:u32)  [unwired: 3 in, 2 out]
                    n255 = Bundle By Name(cluster=w1624, "X Axis.Angle"=w1622) -> (w1623:T24)
                    n256 = call "Check Rotate Done.vi"("error in (no error)"=w1638, "start"=w1631, "phandle in"=w1637) -> ("error out"=w1625:errorcluster)  [unwired: 8 in]
                  }
                  frame "X" {
                    w1656 = u16 20039 ("start")
                    n257 = Greater Than 0?(x=w1640) -> (x > 0?=w1639:bool)
                    n258 = Select(t=u32 54 ("number"), s=w1639, f=u32 55 ("number")) -> (s? t:f=w1646:u32)
                    n259 = Build Array(w1646) -> (w1649:u32[])
                    n260 = Select(t=0.21 ("x"), s=w1639, f=-0.21 ("x")) -> (s? t:f=w1641:dbl)
                    n261 = Byte Array To String(unsigned byte array=w1649) -> (string=w1647:string)
                    n262 = call "Z Aux Modbus Set0x.vi"("pdata"=w1647, "error in (no error)"=w1665, "inum"=u16 8, "start"=u16 20032, "handle"=w1666) -> ("error out"=w1654:errorcluster, "handle out"=w1655:u32)  [unwired: 3 in, 2 out]
                    n263 = Unbundle By Name(w1663) -> ("X Axis.Angle"=w1651:dbl)
                    n264 = call "Delay Time.vi"("error in (no error)"=w1654, "Delay(ms)"=u32 30) -> ("error out"=w1652:errorcluster)  [unwired: 9 in]
                    n265 = Add(x=w1641, y=w1651) -> (x+y=w1650:dbl)
                    n266 = Bundle By Name(cluster=w1663, "X Axis.Angle"=w1650) -> (w1662:T24)
                    n267 = call "Z Aux Modbus Set0x.vi"("pdata"=w1648, "error in (no error)"=w1652, "inum"=u16 1, "start"=w1656, "handle"=w1655) -> ("error out"=w1661:errorcluster, "handle out"=w1660:u32)  [unwired: 3 in, 2 out]
                    n268 = call "Check Rotate Done.vi"("error in (no error)"=w1661, "start"=w1656, "phandle in"=w1660) -> ("error out"=w1664:errorcluster)  [unwired: 8 in]
                  }
                  frame "X+Y" {
                    n269 = disable-structure shown="Enabled" {
                      disable-tunnel: w1672 -> [w1688 _]
                      disable-tunnel: w1671 -> [w1687 _]
                      disable-tunnel: w1670 -> [w1684 _]
                      disable-tunnel: [w1680 _] -> w1669
                      disable-tunnel: w1668 -> [w1677 _]
                      disable-tunnel: [w1676 _] -> w1667
                      frame Disabled {
                        n270 = Unbundle By Name(w1677) -> ("X Axis.Angle"=w1679:dbl, "X Axis.Angle"=w1678:dbl)
                        n271 = for {
                          tunnel: _ -> [w1702]
                          shift-right: [w1701] -> w1682
                          shift-left: w1687 -> [w1703]
                          tunnel: i32[] [20032, 20040] -> [w1699] mode=indexing
                          tunnel: w1684 -> [w1698]
                          tunnel: [w1697] -> w1683
                          n272 = call "Z Aux Modbus Set0x.vi"("pdata"=w1702, "error in (no error)"=w1698, "inum"=u16 8, "start"=w1699, "handle"=w1703) -> ("error out"=w1697:errorcluster, "handle out"=w1701:u32)  [unwired: 3 in, 2 out]
                        }
                        n273 = call "Delay Time.vi"("error in (no error)"=w1683) -> ("error out"=w1681:errorcluster)  [unwired: 10 in]
                        n274 = Add(x=w1678) -> (y=w1673:dbl, x+y=w1674:dbl)
                        n275 = Add(x=w1673, y=w1679) -> (x+y=w1675:dbl)
                        n276 = for {
                          tunnel: w1688 -> [w1694]
                          tunnel: w1682 -> [w1693]
                          tunnel: i32[] [20039, 20047] -> [w1691] mode=indexing
                          tunnel: w1681 -> [w1690]
                          tunnel: [w1689] -> w1680
                          n277 = call "Z Aux Modbus Set0x.vi"("pdata"=w1694, "error in (no error)"=w1690, "inum"=u16 1, "start"=w1691, "handle"=w1693) -> ("error out"=w1696:errorcluster, "handle out"=w1695:u32)  [unwired: 3 in, 2 out]
                          n278 = call "Check Rotate Done.vi"("error in (no error)"=w1696, "start"=w1691, "phandle in"=w1695) -> ("error out"=w1689:errorcluster)  [unwired: 8 in]
                        }
                        n279 = Bundle By Name(cluster=w1677, "X Axis.Angle"=w1675, "X Axis.Angle"=w1674) -> (w1676:T24)
                      }
                      frame Enabled {
                      }
                    }
                  }
                }
              }
            }
          }
          frame "Return to Origin" {
            n280 = Unbundle By Name(w1705) -> ("phandle out"=w1708:u32, "Axis"=w1707:enum16{"X", "Y", "X+Y"}[])
            n281 = for {
              tunnel: w1708 -> [w1717]
              tunnel: w1707 -> [w1716] mode=indexing
              shift-right: [w1711] -> _
              shift-left: w1706 -> [w1712]
              shift-right: [w1709] -> w1704
              shift-left: w1705 -> [w1710]
              n282 = Build Array(u32 64) -> (w1714:u32[])
              n283 = Byte Array To String(unsigned byte array=w1714) -> (string=w1713:string)
              n284 = case shown="\"X+Y\"" w1716 {
                tunnel: w1717 -> [w1726 w1741 w1752]
                tunnel: w1713 -> [w1725 w1740 w1751]
                tunnel: w1712 -> [w1722 w1734 w1747]
                tunnel: [w1721 w1733 w1745] -> w1711
                tunnel: w1710 -> [w1720 w1732 w1744]
                tunnel: [w1719 w1731 w1743] -> w1709
                frame "X", Default {
                  n285 = call "Z Aux Modbus Set0x.vi"("pdata"=w1725, "error in (no error)"=w1722, "inum"=u16 8, "start"=u16 20032, "handle"=w1726) -> ("error out"=w1728:errorcluster, "handle out"=w1727:u32)  [unwired: 3 in, 2 out]
                  n286 = call "Check Rotate Done.vi"("error in (no error)"=w1728, "start"=u16 20038, "phandle in"=w1727) -> ("error out"=w1721:errorcluster)  [unwired: 8 in]
                  n287 = Bundle By Name(cluster=w1720, "X Axis.Angle"=0.0) -> (w1719:T24)
                }
                frame "Y" {
                  n288 = call "Z Aux Modbus Set0x.vi"("pdata"=w1740, "error in (no error)"=w1734, "inum"=u16 8, "start"=u16 20040, "handle"=w1741) -> ("error out"=w1738:errorcluster, "handle out"=w1737:u32)  [unwired: 3 in, 2 out]
                  n289 = call "Check Rotate Done.vi"("error in (no error)"=w1738, "start"=u16 20046, "phandle in"=w1737) -> ("error out"=w1733:errorcluster)  [unwired: 8 in]
                  n290 = Bundle By Name(cluster=w1732, "X Axis.Angle"=0.0 ("Y Axis.Angle")) -> (w1731:T24)
                }
                frame "X+Y" {
                  w1742 = 0.0 ("X Axis.Angle")
                  n291 = for {
                    tunnel: w1752 -> [w1763]
                    tunnel: i32[] [20032, 20040] -> [w1760] mode=indexing
                    tunnel: w1751 -> [w1762]
                    tunnel: [w1759] -> w1750
                    tunnel: w1747 -> [w1758]
                    tunnel: [w1757] -> w1746
                    n292 = call "Z Aux Modbus Set0x.vi"("pdata"=w1762, "error in (no error)"=w1758, "inum"=u16 8, "start"=w1760, "handle"=w1763) -> ("error out"=w1757:errorcluster, "handle out"=w1759:u32)  [unwired: 3 in, 2 out]
                  }
                  n293 = Bundle By Name(cluster=w1744, "X Axis.Angle"=w1742, "X Axis.Angle"=w1742) -> (w1743:T24)
                  n294 = for {
                    tunnel: w1750 -> [w1756]
                    tunnel: i32[] [20038, 20046] -> [w1755] mode=indexing
                    tunnel: w1746 -> [w1754]
                    tunnel: [w1753] -> w1745
                    n295 = call "Check Rotate Done.vi"("error in (no error)"=w1754, "start"=w1755, "phandle in"=w1756) -> ("error out"=w1753:errorcluster)  [unwired: 8 in]
                  }
                }
              }
            }
          }
          frame "Return to Zero" {
            n296 = Unbundle By Name(w1765) -> ("Normal Open / Close"=w1772:enum16{"Open", "Close"}, "Deceleration"=w1771:dbl, "Creep"=w1773:dbl, "phandle out"=w1777:u32, "Axis"=w1770:enum16{"X", "Y", "X+Y"}[], "S ramp"=w1776:dbl, "Acceleration"=w1775:dbl, "Initial Speed"=w1774:dbl, "Speed"=w1766:dbl, "X Axis.Operating State"=w1769:string, "X Axis.Operating State"=w1768:string)
            n297 = for {
              tunnel: w1777 -> [w1794]
              tunnel: w1776 -> [w1793]
              tunnel: w1775 -> [w1792]
              tunnel: w1774 -> [w1791]
              tunnel: w1773 -> [w1790]
              tunnel: w1772 -> [w1789]
              tunnel: w1771 -> [w1788]
              tunnel: w1770 -> [w1787] mode=indexing
              tunnel: w1769 -> [w1786]
              tunnel: w1768 -> [w1785]
              tunnel: w1766 -> [w1782]
              shift-right: [w1783] -> _
              shift-left: w1767 -> [w1784]
              tunnel: w1765 -> [w1778]
              tunnel: [w1778] -> w1764
              n298 = In Range and Coerce(upper limit=5000.0, x=w1782, lower limit=0.0) -> (coerced(x)=w1779:dbl)  [unwired: 1 out]
              n299 = case shown="\"X\", Default" w1787 {
                selector: w1787 -> [w1798 w1822 _]
                tunnel: w1794 -> [w1806 w1830 w1858]
                tunnel: w1793 -> [w1805 w1829 w1857]
                tunnel: w1792 -> [w1804 w1828 w1856]
                tunnel: w1791 -> [w1803 w1827 w1855]
                tunnel: w1779 -> [w1802 w1826 w1854]
                tunnel: w1790 -> [w1801 w1825 w1853]
                tunnel: w1789 -> [w1800 w1824 w1852]
                tunnel: w1788 -> [w1799 w1823 w1851]
                tunnel: w1786 -> [w1797 _ w1850]
                tunnel: w1785 -> [_ w1821 w1849]
                tunnel: w1784 -> [w1796 w1820 w1844]
                tunnel: [w1795 w1819 w1843] -> w1783
                frame "X", Default {
                  n300 = case shown="\"Stop\"" w1797 {
                    tunnel: w1806 -> [_ w1818]
                    tunnel: w1805 -> [_ w1817]
                    tunnel: w1804 -> [_ w1816]
                    tunnel: w1803 -> [_ w1815]
                    tunnel: w1802 -> [_ w1814]
                    tunnel: w1801 -> [_ w1813]
                    tunnel: w1800 -> [_ w1812]
                    tunnel: w1799 -> [_ w1811]
                    tunnel: w1798 -> [_ w1810]
                    tunnel: w1796 -> [w1807 w1809]
                    tunnel: [w1807 w1808] -> w1795
                    frame "False", Default {
                    }
                    frame "Stop" {
                      n301 = call "Return to Zero.vi"("handle"=w1818, "Creep"=w1813, "Decel"=w1811, "ionum"=w1812, "Axis"=w1810, "Sramp"=w1817, "Accel"=w1816, "error in (no error)"=w1809, "Lspeed"=w1815, "Speed"=w1814) -> ("error out"=w1808:errorcluster)  [unwired: 5 in]
                    }
                  }
                }
                frame "Y" {
                  n302 = case shown="\"Stop\"" w1821 {
                    tunnel: w1830 -> [_ w1842]
                    tunnel: w1829 -> [_ w1841]
                    tunnel: w1828 -> [_ w1840]
                    tunnel: w1827 -> [_ w1839]
                    tunnel: w1826 -> [_ w1838]
                    tunnel: w1825 -> [_ w1837]
                    tunnel: w1824 -> [_ w1836]
                    tunnel: w1823 -> [_ w1835]
                    tunnel: w1822 -> [_ w1834]
                    tunnel: w1820 -> [w1831 w1833]
                    tunnel: [w1831 w1832] -> w1819
                    frame "False", Default {
                    }
                    frame "Stop" {
                      n303 = call "Return to Zero.vi"("handle"=w1842, "Creep"=w1837, "Decel"=w1835, "ionum"=w1836, "Axis"=w1834, "Sramp"=w1841, "Accel"=w1840, "error in (no error)"=w1833, "Lspeed"=w1839, "Speed"=w1838) -> ("error out"=w1832:errorcluster)  [unwired: 5 in]
                    }
                  }
                }
                frame "X+Y" {
                  w1848 = "Stop" ("y")
                  n304 = Equal?(x=w1850, y=w1848) -> (x = y?=w1847:bool)
                  n305 = Equal?(x=w1848, y=w1849) -> (x = y?=w1846:bool)
                  n306 = And(x=w1847, y=w1846) -> (x .and. y?=w1845:bool)
                  n307 = case shown="True" w1845 {
                    tunnel: w1858 -> [_ w1870]
                    tunnel: w1857 -> [_ w1869]
                    tunnel: w1856 -> [_ w1868]
                    tunnel: w1855 -> [_ w1867]
                    tunnel: w1854 -> [_ w1866]
                    tunnel: w1853 -> [_ w1865]
                    tunnel: w1852 -> [_ w1864]
                    tunnel: w1851 -> [_ w1863]
                    tunnel: w1844 -> [w1859 w1861]
                    tunnel: [w1859 w1860] -> w1843
                    frame False {
                    }
                    frame True {
                      n308 = for {
                        tunnel: w1870 -> [w1881]
                        tunnel: w1869 -> [w1880]
                        tunnel: w1868 -> [w1879]
                        tunnel: w1867 -> [w1878]
                        tunnel: w1866 -> [w1877]
                        tunnel: w1865 -> [w1876]
                        tunnel: w1864 -> [w1875]
                        tunnel: w1863 -> [w1874]
                        tunnel: i32[] [0, 1] -> [w1873] mode=indexing
                        tunnel: w1861 -> [w1872]
                        tunnel: [w1871] -> w1860
                        n309 = call "Return to Zero.vi"("handle"=w1881, "Creep"=w1876, "Decel"=w1874, "ionum"=w1875, "Axis"=w1873, "Sramp"=w1880, "Accel"=w1879, "error in (no error)"=w1872, "Lspeed"=w1878, "Speed"=w1877) -> ("error out"=w1871:errorcluster)  [unwired: 5 in]
                      }
                    }
                  }
                }
              }
            }
          }
          frame "Return to Middle" {
            n310 = Unbundle By Name(w1896) -> ("Deceleration"=w1890:dbl, "phandle out"=w1895:u32, "Axis"=w1889:enum16{"X", "Y", "X+Y"}[], "S ramp"=w1894:dbl, "Acceleration"=w1893:dbl, "Initial Speed"=w1892:dbl, "Speed"=w1891:dbl, "X Axis.Operating State"=w1888:string, "X Axis.Operating State"=w1887:string)
            n311 = Build Array("X_MID", "Y_MID") -> (w1884:dbl[])
            n312 = for {
              tunnel: w1895 -> [w1911]
              tunnel: w1894 -> [w1910]
              tunnel: w1893 -> [w1909]
              tunnel: w1892 -> [w1908]
              tunnel: w1891 -> [w1907]
              tunnel: w1890 -> [w1906]
              tunnel: w1889 -> [w1905] mode=indexing
              tunnel: w1888 -> [w1904]
              tunnel: w1887 -> [w1903]
              shift-right: [w1901] -> _
              shift-left: w1886 -> [w1902]
              tunnel: w1885 -> [w1900]
              tunnel: w1884 -> [w1899]
              tunnel: "X_MID" -> [w1898]
              tunnel: "Y_MID" -> [w1897]
              n313 = case shown="\"Y\"" w1905 {
                selector: w1905 -> [w1919 w1944 _]
                tunnel: w1911 -> [w1925 w1950 w1976]
                tunnel: w1910 -> [w1924 w1949 w1975]
                tunnel: w1909 -> [w1923 w1948 w1974]
                tunnel: w1908 -> [w1922 w1947 w1973]
                tunnel: w1907 -> [w1921 w1946 w1972]
                tunnel: w1906 -> [w1920 w1945 w1971]
                tunnel: w1904 -> [w1918 _ w1970]
                tunnel: w1903 -> [_ w1943 w1969]
                tunnel: w1902 -> [w1917 w1942 w1964]
                tunnel: [w1914 w1940 w1963] -> w1901
                tunnel: w1900 -> [w1915 w1939 _]
                tunnel: w1899 -> [_ _ w1962]
                tunnel: w1898 -> [w1912 _ _]
                tunnel: w1897 -> [_ w1937 _]
                frame "X", Default {
                  (unwired) 72700.0 ("Creep")
                  n314 = case shown="\"Stop\"" w1918 {
                    tunnel: w1925 -> [_ w1936]
                    tunnel: w1924 -> [_ w1935]
                    tunnel: w1923 -> [_ w1934]
                    tunnel: w1922 -> [_ w1933]
                    tunnel: w1921 -> [_ w1932]
                    tunnel: w1912 -> [_ w1931]
                    tunnel: w1920 -> [_ w1930]
                    tunnel: w1919 -> [_ w1929]
                    tunnel: w1917 -> [w1926 w1928]
                    tunnel: [w1926 w1927] -> w1916
                    frame "False", Default {
                    }
                    frame "Stop" {
                      n315 = call "Return to Middle.vi"("handle"=w1936, "Distance"=w1931, "Decel"=w1930, "Axis"=w1929, "Sramp"=w1935, "Accel"=w1934, "error in (no error)"=w1928, "Lspeed"=w1933, "Speed"=w1932) -> ("error out"=w1927:errorcluster)  [unwired: 5 in, 1 out]
                    }
                  }
                  n316 = Enqueue Element(queue=w1915, element=cluster{"State":T17, "Variable":variant} {"State"=enum."Return to Origin", "Variable"=variant}, error in (no error)=w1916) -> (error out=w1914:errorcluster)  [unwired: 1 in, 2 out]
                }
                frame "Y" {
                  (unwired) 71700.0 ("Creep")
                  n317 = case shown="\"Stop\"" w1943 {
                    tunnel: w1950 -> [_ w1961]
                    tunnel: w1949 -> [_ w1960]
                    tunnel: w1948 -> [_ w1959]
                    tunnel: w1947 -> [_ w1958]
                    tunnel: w1946 -> [_ w1957]
                    tunnel: w1937 -> [_ w1956]
                    tunnel: w1945 -> [_ w1955]
                    tunnel: w1944 -> [_ w1954]
                    tunnel: w1942 -> [w1951 w1953]
                    tunnel: [w1951 w1952] -> w1941
                    frame "False", Default {
                    }
                    frame "Stop" {
                      n318 = call "Return to Middle.vi"("handle"=w1961, "Distance"=w1956, "Decel"=w1955, "Axis"=w1954, "Sramp"=w1960, "Accel"=w1959, "error in (no error)"=w1953, "Lspeed"=w1958, "Speed"=w1957) -> ("error out"=w1952:errorcluster)  [unwired: 5 in, 1 out]
                    }
                  }
                  n319 = Enqueue Element(queue=w1939, element=cluster{"State":T17, "Variable":variant} {"State"=enum."Return to Origin", "Variable"=variant}, error in (no error)=w1941) -> (error out=w1940:errorcluster)  [unwired: 1 in, 2 out]
                }
                frame "X+Y" {
                  w1968 = "Stop" ("y")
                  n320 = Equal?(x=w1970, y=w1968) -> (x = y?=w1967:bool)
                  n321 = Equal?(x=w1968, y=w1969) -> (x = y?=w1966:bool)
                  n322 = And(x=w1967, y=w1966) -> (x .and. y?=w1965:bool)
                  n323 = case shown="True" w1965 {
                    tunnel: w1976 -> [_ w1987]
                    tunnel: w1975 -> [_ w1986]
                    tunnel: w1974 -> [_ w1985]
                    tunnel: w1973 -> [_ w1984]
                    tunnel: w1972 -> [_ w1983]
                    tunnel: w1962 -> [_ w1982]
                    tunnel: w1971 -> [_ w1981]
                    tunnel: w1964 -> [w1977 w1979]
                    tunnel: [w1977 w1978] -> w1963
                    frame False {
                    }
                    frame True {
                      n324 = for {
                        tunnel: w1987 -> [w1997]
                        tunnel: w1986 -> [w1996]
                        tunnel: w1985 -> [w1995]
                        tunnel: w1984 -> [w1994]
                        tunnel: w1983 -> [w1993]
                        tunnel: w1982 -> [w1992] mode=indexing
                        tunnel: w1981 -> [w1991]
                        tunnel: i32[] [0, 1] -> [w1990] mode=indexing
                        tunnel: w1979 -> [w1989]
                        tunnel: [w1988] -> w1978
                        n325 = call "Return to Middle.vi"("handle"=w1997, "Distance"=w1992, "Decel"=w1991, "Axis"=w1990, "Sramp"=w1996, "Accel"=w1995, "error in (no error)"=w1989, "Lspeed"=w1994, "Speed"=w1993) -> ("error out"=w1988:errorcluster)  [unwired: 5 in, 1 out]
                      }
                    }
                  }
                }
              }
            }
          }
          frame "Go to Step1" {
            n326 = Unbundle By Name(w2004) -> ("Deceleration"=w2009:dbl, "phandle out"=w2014:u32, "Axis"=w2001:enum16{"X", "Y", "X+Y"}[], "S ramp"=w2013:dbl, "Acceleration"=w2012:dbl, "Initial Speed"=w2011:dbl, "Speed"=w2010:dbl, "X Axis.Operating State"=w2008:string, "X Axis.Operating State"=w2000:string, "X Axis.Current Position"=w2006:dbl, "X Axis.Current Position"=w1999:dbl, "X Axis.Angle"=w2002:dbl, "X Axis.Angle"=w1998:dbl)
            n327 = for {
              tunnel: w2014 -> [w2032]
              tunnel: w2013 -> [w2031]
              tunnel: w2012 -> [w2030]
              tunnel: w2011 -> [w2029]
              tunnel: w2010 -> [w2028]
              tunnel: w2009 -> [w2027]
              tunnel: w2008 -> [w2026]
              tunnel: w2006 -> [w2023]
              tunnel: w2005 -> [w2022]
              tunnel: w2002 -> [w2019]
              tunnel: w2001 -> [w2018] mode=indexing
              tunnel: w2000 -> [w2017]
              tunnel: w1999 -> [w2016]
              tunnel: w1998 -> [w2015]
              shift-right: [w2024] -> _
              shift-left: w2007 -> [w2025]
              shift-right: [w2020] -> w2003
              shift-left: w2004 -> [w2021]
              n328 = case shown="\"X\"" w2018 {
                selector: w2018 -> [w2033 w2173]
                tunnel: w2032 -> [w2047 w2184]
                tunnel: w2031 -> [w2046 w2183]
                tunnel: w2030 -> [w2045 w2182]
                tunnel: w2029 -> [w2044 w2181]
                tunnel: w2028 -> [w2043 w2180]
                tunnel: w2027 -> [w2042 w2179]
                tunnel: w2026 -> [w2041 _]
                tunnel: w2025 -> [w2040 w2178]
                tunnel: [w2039 w2177] -> w2024
                tunnel: w2023 -> [w2038 _]
                tunnel: w2022 -> [w2037 w2176]
                tunnel: w2021 -> [w2036 w2175]
                tunnel: [w2035 w2174] -> w2020
                tunnel: w2019 -> [w2034 _]
                tunnel: w2017 -> [_ w2172]
                tunnel: w2016 -> [_ w2171]
                tunnel: w2015 -> [_ w2170]
                frame "Y", Default {
                  n329 = case shown="Default" w2038 {
                    tunnel: w2047 -> [_ w2063 w2112 _]
                    tunnel: w2046 -> [_ w2062 w2111 _]
                    tunnel: w2045 -> [_ w2061 w2110 _]
                    tunnel: w2044 -> [_ w2060 w2109 _]
                    tunnel: w2043 -> [_ w2059 w2108 _]
                    tunnel: w2042 -> [_ w2058 w2107 _]
                    tunnel: w2033 -> [_ w2057 w2106 _]
                    tunnel: w2041 -> [_ w2056 w2105 w2155]
                    tunnel: w2040 -> [w2049 w2055 w2104 w2157]
                    tunnel: [w2049 w2054 w2103 w2149] -> w2039
                    tunnel: w2037 -> [_ _ _ w2156]
                    tunnel: w2036 -> [w2048 w2052 w2101 w2151]
                    tunnel: [w2048 w2051 w2100 w2151] -> w2035
                    tunnel: w2034 -> [_ w2050 w2099 _]
                    frame Default {
                    }
                    frame 0..5999 {
                      n330 = case shown="\"Stop\"" w2056 {
                        tunnel: w2063 -> [_ w2098]
                        tunnel: w2062 -> [_ w2097]
                        tunnel: w2061 -> [_ w2096]
                        tunnel: w2060 -> [_ w2095]
                        tunnel: w2059 -> [_ w2094]
                        tunnel: 6000.0 ("Creep") -> [_ w2093]
                        tunnel: w2058 -> [_ w2092]
                        tunnel: w2057 -> [_ w2091]
                        tunnel: w2055 -> [w2065 w2090]
                        tunnel: [w2065 w2074] -> w2054
                        tunnel: w2052 -> [w2064 w2070]
                        tunnel: [w2064 w2069] -> w2051
                        tunnel: w2050 -> [_ w2067]
                        frame "False", Default {
                        }
                        frame "Stop" {
                          w2071 = u16 20047 ("start")
                          n331 = call "Return to Middle.vi"("handle"=w2098, "Distance"=w2093, "Decel"=w2092, "Axis"=w2091, "Sramp"=w2097, "Accel"=w2096, "error in (no error)"=w2090, "Lspeed"=w2095, "Speed"=w2094) -> ("handle out"=w2079:u32, "error out"=w2080:errorcluster)  [unwired: 5 in]
                          n332 = Build Array(u32 61 ("element")) -> (w2077:u32[])
                          n333 = Byte Array To String(unsigned byte array=w2077) -> (string=w2078:string)
                          n334 = call "Z Aux Modbus Set0x.vi"("pdata"=w2078, "error in (no error)"=w2080, "inum"=u16 8, "start"=u16 20040, "handle"=w2079) -> ("error out"=w2083:errorcluster, "handle out"=w2084:u32)  [unwired: 3 in, 2 out]
                          n335 = Add(x=-14.43, y=w2067) -> (x+y=w2068:dbl)
                          n336 = Build Array(u32 1 ("element")) -> (w2073:u32[])
                          n337 = call "Delay Time.vi"("error in (no error)"=w2083, "Delay(ms)"=u32 30) -> ("error out"=w2081:errorcluster)  [unwired: 9 in]
                          n338 = Bundle By Name(cluster=w2070, "X Axis.Angle"=w2068) -> (w2069:T24)
                          n339 = Byte Array To String(unsigned byte array=w2073) -> (string=w2075:string)
                          n340 = call "Z Aux Modbus Set0x.vi"("pdata"=w2075, "error in (no error)"=w2081, "inum"=u16 1, "start"=w2071, "handle"=w2084) -> ("error out"=w2089:errorcluster, "handle out"=w2088:u32)  [unwired: 3 in, 2 out]
                          n341 = call "Check Rotate Done.vi"("error in (no error)"=w2089, "start"=w2071, "phandle in"=w2088) -> ("error out"=w2074:errorcluster)  [unwired: 8 in]
                        }
                      }
                    }
                    frame 6001..71700 {
                      n342 = case shown="\"Stop\"" w2105 {
                        tunnel: w2112 -> [_ w2147]
                        tunnel: w2111 -> [_ w2146]
                        tunnel: w2110 -> [_ w2145]
                        tunnel: w2109 -> [_ w2144]
                        tunnel: w2108 -> [_ w2143]
                        tunnel: 6000.0 ("Creep") -> [_ w2142]
                        tunnel: w2107 -> [_ w2141]
                        tunnel: w2106 -> [_ w2140]
                        tunnel: w2104 -> [w2114 w2139]
                        tunnel: [w2114 w2123] -> w2103
                        tunnel: w2101 -> [w2113 w2119]
                        tunnel: [w2113 w2118] -> w2100
                        tunnel: w2099 -> [_ w2117]
                        frame "False", Default {
                        }
                        frame "Stop" {
                          w2120 = u16 20047 ("start")
                          n343 = call "Return to Middle.vi"("handle"=w2147, "Distance"=w2142, "Decel"=w2141, "Axis"=w2140, "Sramp"=w2146, "Accel"=w2145, "error in (no error)"=w2139, "Lspeed"=w2144, "Speed"=w2143) -> ("handle out"=w2128:u32, "error out"=w2129:errorcluster)  [unwired: 5 in]
                          n344 = Add(x=-14.43, y=w2117) -> (x+y=w2115:dbl)
                          n345 = Build Array(u32 61 ("element")) -> (w2126:u32[])
                          n346 = Byte Array To String(unsigned byte array=w2126) -> (string=w2127:string)
                          n347 = call "Z Aux Modbus Set0x.vi"("pdata"=w2127, "error in (no error)"=w2129, "inum"=u16 8, "start"=u16 20040, "handle"=w2128) -> ("error out"=w2132:errorcluster, "handle out"=w2133:u32)  [unwired: 3 in, 2 out]
                          n348 = Build Array(u32 1 ("element")) -> (w2122:u32[])
                          n349 = call "Delay Time.vi"("error in (no error)"=w2132, "Delay(ms)"=u32 30) -> ("error out"=w2130:errorcluster)  [unwired: 9 in]
                          n350 = Bundle By Name(cluster=w2119, "X Axis.Angle"=w2115) -> (w2118:T24)
                          n351 = Byte Array To String(unsigned byte array=w2122) -> (string=w2124:string)
                          n352 = call "Z Aux Modbus Set0x.vi"("pdata"=w2124, "error in (no error)"=w2130, "inum"=u16 1, "start"=w2120, "handle"=w2133) -> ("error out"=w2138:errorcluster, "handle out"=w2137:u32)  [unwired: 3 in, 2 out]
                          n353 = call "Check Rotate Done.vi"("error in (no error)"=w2138, "start"=w2120, "phandle in"=w2137) -> ("error out"=w2123:errorcluster)  [unwired: 8 in]
                        }
                      }
                    }
                    frame 71701..135000 {
                      n354 = case shown="\"Stop\"" w2155 {
                        tunnel: w2157 -> [w2164 w2169]
                        tunnel: w2156 -> [w2163 w2168]
                        tunnel: [w2164 w2166] -> w2154
                        tunnel: [w2163 w2165] -> w2153
                        frame Default {
                        }
                        frame "Stop" {
                          n355 = Enqueue Element(queue=w2168, element=cluster{"State":T17, "Variable":variant} {"State"=enum."Go to Step2", "Variable"=variant}, error in (no error)=w2169) -> (queue out=w2165:refnum<queue>, error out=w2166:errorcluster)  [unwired: 1 in, 1 out]
                        }
                      }
                      n356 = for {
                        tunnel: w2154 -> [w2162]
                        tunnel: w2153 -> [w2161]
                        tunnel: cluster{"State":T17, "Variable":variant}[] [{"State"=enum."Idle", "Variable"=variant}, {"State"=enum."Update", "Variable"=variant}, {"State"=enum."Go to Step1", "Variable"=variant}] -> [w2160] mode=indexing
                        tunnel: [w2159] -> w2150
                        n357 = Enqueue Element(queue=w2161, element=w2160, error in (no error)=w2162) -> (error out=w2159:errorcluster)  [unwired: 1 in, 2 out]
                        n358 = call "Delay Time.vi"("Delay(ms)"=u32 30) -> ()  [unwired: 10 in, 1 out]
                      }
                      n359 = call "Delay Time.vi"("error in (no error)"=w2150, "Delay(ms)"=u32 30) -> ("error out"=w2149:errorcluster)  [unwired: 9 in]
                    }
                  }
                }
                frame "X" {
                  n360 = case shown="0..12199" w2171 {
                    tunnel: w2184 -> [_ w2200 w2249 _]
                    tunnel: w2183 -> [_ w2199 w2248 _]
                    tunnel: w2182 -> [_ w2198 w2247 _]
                    tunnel: w2181 -> [_ w2197 w2246 _]
                    tunnel: w2180 -> [_ w2196 w2245 _]
                    tunnel: w2179 -> [_ w2195 w2244 _]
                    tunnel: w2173 -> [_ w2194 w2243 _]
                    tunnel: w2178 -> [w2186 w2193 w2242 w2294]
                    tunnel: [w2186 w2192 w2241 w2287] -> w2177
                    tunnel: w2176 -> [_ _ _ w2293]
                    tunnel: w2175 -> [w2185 w2190 w2239 w2289]
                    tunnel: [w2185 w2189 w2238 w2289] -> w2174
                    tunnel: w2170 -> [_ w2188 w2237 _]
                    tunnel: w2172 -> [_ w2187 w2236 w2285]
                    frame Default {
                    }
                    frame 0..12199 {
                      n361 = case shown="\"Stop\"" w2187 {
                        tunnel: w2200 -> [_ w2235]
                        tunnel: w2199 -> [_ w2234]
                        tunnel: w2198 -> [_ w2233]
                        tunnel: w2197 -> [_ w2232]
                        tunnel: w2196 -> [_ w2231]
                        tunnel: 12200.0 ("Creep") -> [_ w2230]
                        tunnel: w2195 -> [_ w2229]
                        tunnel: w2194 -> [_ w2228]
                        tunnel: w2193 -> [w2202 w2227]
                        tunnel: [w2202 w2211] -> w2192
                        tunnel: w2190 -> [w2201 w2207]
                        tunnel: [w2201 w2206] -> w2189
                        tunnel: w2188 -> [_ w2204]
                        frame "False", Default {
                        }
                        frame "Stop" {
                          w2208 = u16 20039 ("start")
                          n362 = call "Return to Middle.vi"("handle"=w2235, "Distance"=w2230, "Decel"=w2229, "Axis"=w2228, "Sramp"=w2234, "Accel"=w2233, "error in (no error)"=w2227, "Lspeed"=w2232, "Speed"=w2231) -> ("handle out"=w2216:u32, "error out"=w2217:errorcluster)  [unwired: 5 in]
                          n363 = Build Array(u32 56 ("element")) -> (w2214:u32[])
                          n364 = Byte Array To String(unsigned byte array=w2214) -> (string=w2215:string)
                          n365 = call "Z Aux Modbus Set0x.vi"("pdata"=w2215, "error in (no error)"=w2217, "inum"=u16 8, "start"=u16 20032, "handle"=w2216) -> ("error out"=w2220:errorcluster, "handle out"=w2221:u32)  [unwired: 3 in, 2 out]
                          n366 = Add(x=13.2, y=w2204) -> (x+y=w2205:dbl)
                          n367 = Build Array(u32 1 ("element")) -> (w2210:u32[])
                          n368 = call "Delay Time.vi"("error in (no error)"=w2220, "Delay(ms)"=u32 30) -> ("error out"=w2218:errorcluster)  [unwired: 9 in]
                          n369 = Bundle By Name(cluster=w2207, "X Axis.Angle"=w2205) -> (w2206:T24)
                          n370 = Byte Array To String(unsigned byte array=w2210) -> (string=w2212:string)
                          n371 = call "Z Aux Modbus Set0x.vi"("pdata"=w2212, "error in (no error)"=w2218, "inum"=u16 1, "start"=w2208, "handle"=w2221) -> ("error out"=w2226:errorcluster, "handle out"=w2225:u32)  [unwired: 3 in, 2 out]
                          n372 = call "Check Rotate Done.vi"("error in (no error)"=w2226, "start"=w2208, "phandle in"=w2225) -> ("error out"=w2211:errorcluster)  [unwired: 8 in]
                        }
                      }
                    }
                    frame 12200..72700 {
                      n373 = case shown="\"Stop\"" w2236 {
                        tunnel: w2249 -> [_ w2284]
                        tunnel: w2248 -> [_ w2283]
                        tunnel: w2247 -> [_ w2282]
                        tunnel: w2246 -> [_ w2281]
                        tunnel: w2245 -> [_ w2280]
                        tunnel: 12200.0 ("Creep") -> [_ w2279]
                        tunnel: w2244 -> [_ w2278]
                        tunnel: w2243 -> [_ w2277]
                        tunnel: w2242 -> [w2251 w2276]
                        tunnel: [w2251 w2260] -> w2241
                        tunnel: w2239 -> [w2250 w2256]
                        tunnel: [w2250 w2255] -> w2238
                        tunnel: w2237 -> [_ w2254]
                        frame "False", Default {
                        }
                        frame "Stop" {
                          w2257 = u16 20039 ("start")
                          n374 = call "Return to Middle.vi"("handle"=w2284, "Distance"=w2279, "Decel"=w2278, "Axis"=w2277, "Sramp"=w2283, "Accel"=w2282, "error in (no error)"=w2276, "Lspeed"=w2281, "Speed"=w2280) -> ("handle out"=w2265:u32, "error out"=w2266:errorcluster)  [unwired: 5 in]
                          n375 = Add(x=13.2, y=w2254) -> (x+y=w2252:dbl)
                          n376 = Build Array(u32 56 ("element")) -> (w2263:u32[])
                          n377 = Byte Array To String(unsigned byte array=w2263) -> (string=w2264:string)
                          n378 = call "Z Aux Modbus Set0x.vi"("pdata"=w2264, "error in (no error)"=w2266, "inum"=u16 8, "start"=u16 20032, "handle"=w2265) -> ("error out"=w2269:errorcluster, "handle out"=w2270:u32)  [unwired: 3 in, 2 out]
                          n379 = Build Array(u32 1 ("element")) -> (w2259:u32[])
                          n380 = call "Delay Time.vi"("error in (no error)"=w2269, "Delay(ms)"=u32 30) -> ("error out"=w2267:errorcluster)  [unwired: 9 in]
                          n381 = Bundle By Name(cluster=w2256, "X Axis.Angle"=w2252) -> (w2255:T24)
                          n382 = Byte Array To String(unsigned byte array=w2259) -> (string=w2261:string)
                          n383 = call "Z Aux Modbus Set0x.vi"("pdata"=w2261, "error in (no error)"=w2267, "inum"=u16 1, "start"=w2257, "handle"=w2270) -> ("error out"=w2275:errorcluster, "handle out"=w2274:u32)  [unwired: 3 in, 2 out]
                          n384 = call "Check Rotate Done.vi"("error in (no error)"=w2275, "start"=w2257, "phandle in"=w2274) -> ("error out"=w2260:errorcluster)  [unwired: 8 in]
                        }
                      }
                    }
                    frame 72701..141500 {
                      n385 = case shown="Default" w2285 {
                        tunnel: w2294 -> [w2301 w2306]
                        tunnel: w2293 -> [w2300 w2305]
                        tunnel: [w2301 w2303] -> w2292
                        tunnel: [w2300 w2302] -> w2291
                        frame Default {
                        }
                        frame "Stop" {
                          n386 = Enqueue Element(queue=w2305, element=cluster{"State":T17, "Variable":variant} {"State"=enum."Go to Step2", "Variable"=variant}, error in (no error)=w2306) -> (queue out=w2302:refnum<queue>, error out=w2303:errorcluster)  [unwired: 1 in, 1 out]
                        }
                      }
                      n387 = for {
                        tunnel: w2292 -> [w2299]
                        tunnel: w2291 -> [w2298]
                        tunnel: cluster{"State":T17, "Variable":variant}[] [{"State"=enum."Idle", "Variable"=variant}, {"State"=enum."Update", "Variable"=variant}, {"State"=enum."Go to Step1", "Variable"=variant}] -> [w2297] mode=indexing
                        tunnel: [w2296] -> w2288
                        n388 = Enqueue Element(queue=w2298, element=w2297, error in (no error)=w2299) -> (error out=w2296:errorcluster)  [unwired: 1 in, 2 out]
                        n389 = call "Delay Time.vi"("Delay(ms)"=u32 30) -> ()  [unwired: 10 in, 1 out]
                      }
                      n390 = call "Delay Time.vi"("error in (no error)"=w2288, "Delay(ms)"=u32 30) -> ("error out"=w2287:errorcluster)  [unwired: 9 in]
                    }
                  }
                }
              }
            }
          }
          frame "Go to Step2" {
            n391 = Unbundle By Name(w2312) -> ("Deceleration"=w2318:dbl, "phandle out"=w2323:u32, "Axis"=w2310:enum16{"X", "Y", "X+Y"}[], "S ramp"=w2322:dbl, "Acceleration"=w2321:dbl, "Initial Speed"=w2320:dbl, "Speed"=w2319:dbl, "X Axis.Operating State"=w2317:string, "X Axis.Operating State"=w2309:string, "X Axis.Current Position"=w2315:dbl, "X Axis.Current Position"=w2308:dbl, "X Axis.Angle"=w2313:dbl, "X Axis.Angle"=w2307:dbl)
            n392 = for {
              tunnel: w2323 -> [w2341]
              tunnel: w2322 -> [w2340]
              tunnel: w2321 -> [w2339]
              tunnel: w2320 -> [w2338]
              tunnel: w2319 -> [w2337]
              tunnel: w2318 -> [w2336]
              tunnel: w2317 -> [w2335]
              tunnel: w2315 -> [w2332]
              tunnel: w2314 -> [w2331]
              tunnel: w2313 -> [w2330]
              tunnel: w2310 -> [w2327] mode=indexing
              tunnel: w2309 -> [w2326]
              tunnel: w2308 -> [w2325]
              tunnel: w2307 -> [w2324]
              shift-right: [w2333] -> _
              shift-left: w2316 -> [w2334]
              shift-right: [w2328] -> w2311
              shift-left: w2312 -> [w2329]
              n393 = case shown="\"X\"" w2327 {
                selector: w2327 -> [w2342 w2479]
                tunnel: w2341 -> [w2356 w2490]
                tunnel: w2340 -> [w2355 w2489]
                tunnel: w2339 -> [w2354 w2488]
                tunnel: w2338 -> [w2353 w2487]
                tunnel: w2337 -> [w2352 w2486]
                tunnel: w2336 -> [w2351 w2485]
                tunnel: w2335 -> [w2350 _]
                tunnel: w2334 -> [w2349 w2484]
                tunnel: [w2348 w2483] -> w2333
                tunnel: w2332 -> [w2347 _]
                tunnel: w2331 -> [w2346 w2482]
                tunnel: w2330 -> [w2345 _]
                tunnel: w2329 -> [w2344 w2481]
                tunnel: [w2343 w2480] -> w2328
                tunnel: w2326 -> [_ w2478]
                tunnel: w2325 -> [_ w2477]
                tunnel: w2324 -> [_ w2476]
                frame "Y", Default {
                  n394 = case shown="0..5999" w2347 {
                    tunnel: w2356 -> [_ _ w2391 w2440]
                    tunnel: w2355 -> [_ _ w2390 w2439]
                    tunnel: w2354 -> [_ _ w2389 w2438]
                    tunnel: w2353 -> [_ _ w2388 w2437]
                    tunnel: w2352 -> [_ _ w2387 w2436]
                    tunnel: w2351 -> [_ _ w2386 w2435]
                    tunnel: w2342 -> [_ _ w2385 w2434]
                    tunnel: w2350 -> [_ w2363 w2384 w2433]
                    tunnel: w2349 -> [w2358 w2366 w2383 w2432]
                    tunnel: [w2358 w2360 w2382 w2431] -> w2348
                    tunnel: w2346 -> [_ w2365 _ _]
                    tunnel: w2345 -> [_ _ w2378 w2429]
                    tunnel: w2344 -> [w2357 w2359 w2380 w2428]
                    tunnel: [w2357 w2359 w2379 w2427] -> w2343
                    frame Default {
                    }
                    frame 0..5999 {
                      n395 = case shown="\"Stop\"" w2363 {
                        tunnel: w2366 -> [w2367 w2373]
                        tunnel: w2365 -> [w2368 w2372]
                        tunnel: [w2367 w2370] -> w2362
                        tunnel: [w2368 w2369] -> w2361
                        frame Default {
                        }
                        frame "Stop" {
                          n396 = Enqueue Element(queue=w2372, element=cluster{"State":T17, "Variable":variant} {"State"=enum."Go to Step1", "Variable"=variant}, error in (no error)=w2373) -> (queue out=w2369:refnum<queue>, error out=w2370:errorcluster)  [unwired: 1 in, 1 out]
                        }
                      }
                      n397 = for {
                        tunnel: w2362 -> [w2377]
                        tunnel: w2361 -> [w2376]
                        tunnel: cluster{"State":T17, "Variable":variant}[] [{"State"=enum."Idle", "Variable"=variant}, {"State"=enum."Update", "Variable"=variant}, {"State"=enum."Go to Step2", "Variable"=variant}] -> [w2375] mode=indexing
                        tunnel: [w2374] -> w2360
                        n398 = Enqueue Element(queue=w2376, element=w2375, error in (no error)=w2377) -> (error out=w2374:errorcluster)  [unwired: 1 in, 2 out]
                      }
                    }
                    frame 6000..71699 {
                      n399 = case shown="\"Stop\"" w2384 {
                        tunnel: w2391 -> [_ w2426]
                        tunnel: w2390 -> [_ w2425]
                        tunnel: w2389 -> [_ w2424]
                        tunnel: w2388 -> [_ w2423]
                        tunnel: w2387 -> [_ w2422]
                        tunnel: 71700.0 ("Creep") -> [_ w2421]
                        tunnel: w2386 -> [_ w2420]
                        tunnel: w2385 -> [_ w2419]
                        tunnel: w2383 -> [w2393 w2418]
                        tunnel: [w2393 w2402] -> w2382
                        tunnel: w2380 -> [w2392 w2398]
                        tunnel: [w2392 w2397] -> w2379
                        tunnel: w2378 -> [_ w2395]
                        frame "False", Default {
                        }
                        frame "Stop" {
                          w2399 = u16 20047 ("start")
                          n400 = call "Return to Middle.vi"("handle"=w2426, "Distance"=w2421, "Decel"=w2420, "Axis"=w2419, "Sramp"=w2425, "Accel"=w2424, "error in (no error)"=w2418, "Lspeed"=w2423, "Speed"=w2422) -> ("handle out"=w2407:u32, "error out"=w2408:errorcluster)  [unwired: 5 in]
                          n401 = Build Array(u32 60 ("element")) -> (w2405:u32[])
                          n402 = Add(x=14.43, y=w2395) -> (x+y=w2396:dbl)
                          n403 = Byte Array To String(unsigned byte array=w2405) -> (string=w2406:string)
                          n404 = call "Z Aux Modbus Set0x.vi"("pdata"=w2406, "error in (no error)"=w2408, "inum"=u16 8, "start"=u16 20040, "handle"=w2407) -> ("error out"=w2411:errorcluster, "handle out"=w2412:u32)  [unwired: 3 in, 2 out]
                          n405 = Bundle By Name(cluster=w2398, "X Axis.Angle"=w2396) -> (w2397:T24)
                          n406 = Build Array(u32 1 ("element")) -> (w2401:u32[])
                          n407 = call "Delay Time.vi"("error in (no error)"=w2411, "Delay(ms)"=u32 30) -> ("error out"=w2409:errorcluster)  [unwired: 9 in]
                          n408 = Byte Array To String(unsigned byte array=w2401) -> (string=w2403:string)
                          n409 = call "Z Aux Modbus Set0x.vi"("pdata"=w2403, "error in (no error)"=w2409, "inum"=u16 1, "start"=w2399, "handle"=w2412) -> ("error out"=w2417:errorcluster, "handle out"=w2416:u32)  [unwired: 3 in, 2 out]
                          n410 = call "Check Rotate Done.vi"("error in (no error)"=w2417, "start"=w2399, "phandle in"=w2416) -> ("error out"=w2402:errorcluster)  [unwired: 8 in]
                        }
                      }
                    }
                    frame 71701..135000 {
                      n411 = case shown="\"Stop\"" w2433 {
                        tunnel: w2440 -> [_ w2475]
                        tunnel: w2439 -> [_ w2474]
                        tunnel: w2438 -> [_ w2473]
                        tunnel: w2437 -> [_ w2472]
                        tunnel: w2436 -> [_ w2471]
                        tunnel: 71700.0 ("Creep") -> [_ w2470]
                        tunnel: w2435 -> [_ w2469]
                        tunnel: w2434 -> [_ w2468]
                        tunnel: w2432 -> [w2442 w2467]
                        tunnel: [w2442 w2451] -> w2431
                        tunnel: w2429 -> [_ w2445]
                        tunnel: w2428 -> [w2441 w2447]
                        tunnel: [w2441 w2446] -> w2427
                        frame "False", Default {
                        }
                        frame "Stop" {
                          w2448 = u16 20047 ("start")
                          n412 = call "Return to Middle.vi"("handle"=w2475, "Distance"=w2470, "Decel"=w2469, "Axis"=w2468, "Sramp"=w2474, "Accel"=w2473, "error in (no error)"=w2467, "Lspeed"=w2472, "Speed"=w2471) -> ("handle out"=w2456:u32, "error out"=w2457:errorcluster)  [unwired: 5 in]
                          n413 = Build Array(u32 62 ("element")) -> (w2454:u32[])
                          n414 = Add(x=-12.92, y=w2445) -> (x+y=w2444:dbl)
                          n415 = Byte Array To String(unsigned byte array=w2454) -> (string=w2455:string)
                          n416 = call "Z Aux Modbus Set0x.vi"("pdata"=w2455, "error in (no error)"=w2457, "inum"=u16 8, "start"=u16 20040, "handle"=w2456) -> ("error out"=w2460:errorcluster, "handle out"=w2461:u32)  [unwired: 3 in, 2 out]
                          n417 = Bundle By Name(cluster=w2447, "X Axis.Angle"=w2444) -> (w2446:T24)
                          n418 = Build Array(u32 1 ("element")) -> (w2450:u32[])
                          n419 = call "Delay Time.vi"("error in (no error)"=w2460, "Delay(ms)"=u32 30) -> ("error out"=w2458:errorcluster)  [unwired: 9 in]
                          n420 = Byte Array To String(unsigned byte array=w2450) -> (string=w2452:string)
                          n421 = call "Z Aux Modbus Set0x.vi"("pdata"=w2452, "error in (no error)"=w2458, "inum"=u16 1, "start"=w2448, "handle"=w2461) -> ("error out"=w2466:errorcluster, "handle out"=w2465:u32)  [unwired: 3 in, 2 out]
                          n422 = call "Check Rotate Done.vi"("error in (no error)"=w2466, "start"=w2448, "phandle in"=w2465) -> ("error out"=w2451:errorcluster)  [unwired: 8 in]
                        }
                      }
                    }
                  }
                }
                frame "X" {
                  n423 = case shown="Default" w2477 {
                    tunnel: w2490 -> [_ _ w2525 w2574]
                    tunnel: w2489 -> [_ _ w2524 w2573]
                    tunnel: w2488 -> [_ _ w2523 w2572]
                    tunnel: w2487 -> [_ _ w2522 w2571]
                    tunnel: w2486 -> [_ _ w2521 w2570]
                    tunnel: w2485 -> [_ _ w2520 w2569]
                    tunnel: w2479 -> [_ _ w2519 w2568]
                    tunnel: w2478 -> [_ w2497 w2518 w2561]
                    tunnel: w2484 -> [w2492 w2500 w2517 w2567]
                    tunnel: [w2492 w2494 w2516 w2566] -> w2483
                    tunnel: w2482 -> [_ w2499 _ _]
                    tunnel: w2476 -> [_ _ w2512 w2564]
                    tunnel: w2481 -> [w2491 w2493 w2514 w2563]
                    tunnel: [w2491 w2493 w2513 w2562] -> w2480
                    frame Default {
                    }
                    frame 0..12199 {
                      n424 = case shown="\"Stop\"" w2497 {
                        tunnel: w2500 -> [w2501 w2507]
                        tunnel: w2499 -> [w2502 w2506]
                        tunnel: [w2501 w2504] -> w2496
                        tunnel: [w2502 w2503] -> w2495
                        frame Default {
                        }
                        frame "Stop" {
                          n425 = Enqueue Element(queue=w2506, element=cluster{"State":T17, "Variable":variant} {"State"=enum."Go to Step1", "Variable"=variant}, error in (no error)=w2507) -> (queue out=w2503:refnum<queue>, error out=w2504:errorcluster)  [unwired: 1 in, 1 out]
                        }
                      }
                      n426 = for {
                        tunnel: w2496 -> [w2511]
                        tunnel: w2495 -> [w2510]
                        tunnel: cluster{"State":T17, "Variable":variant}[] [{"State"=enum."Idle", "Variable"=variant}, {"State"=enum."Update", "Variable"=variant}, {"State"=enum."Go to Step2", "Variable"=variant}] -> [w2509] mode=indexing
                        tunnel: [w2508] -> w2494
                        n427 = Enqueue Element(queue=w2510, element=w2509, error in (no error)=w2511) -> (error out=w2508:errorcluster)  [unwired: 1 in, 2 out]
                      }
                    }
                    frame 12200..72699 {
                      n428 = case shown="\"Stop\"" w2518 {
                        tunnel: w2525 -> [_ w2560]
                        tunnel: w2524 -> [_ w2559]
                        tunnel: w2523 -> [_ w2558]
                        tunnel: w2522 -> [_ w2557]
                        tunnel: w2521 -> [_ w2556]
                        tunnel: 72700.0 ("Creep") -> [_ w2555]
                        tunnel: w2520 -> [_ w2554]
                        tunnel: w2519 -> [_ w2553]
                        tunnel: w2517 -> [w2527 w2552]
                        tunnel: [w2527 w2536] -> w2516
                        tunnel: w2514 -> [w2526 w2532]
                        tunnel: [w2526 w2531] -> w2513
                        tunnel: w2512 -> [_ w2529]
                        frame "False", Default {
                        }
                        frame "Stop" {
                          w2533 = u16 20039 ("start")
                          n429 = call "Return to Middle.vi"("handle"=w2560, "Distance"=w2555, "Decel"=w2554, "Axis"=w2553, "Sramp"=w2559, "Accel"=w2558, "error in (no error)"=w2552, "Lspeed"=w2557, "Speed"=w2556) -> ("handle out"=w2541:u32, "error out"=w2542:errorcluster)  [unwired: 5 in]
                          n430 = Build Array(u32 57 ("element")) -> (w2539:u32[])
                          n431 = Add(x=-13.2, y=w2529) -> (x+y=w2530:dbl)
                          n432 = Byte Array To String(unsigned byte array=w2539) -> (string=w2540:string)
                          n433 = call "Z Aux Modbus Set0x.vi"("pdata"=w2540, "error in (no error)"=w2542, "inum"=u16 8, "start"=u16 20032, "handle"=w2541) -> ("error out"=w2545:errorcluster, "handle out"=w2546:u32)  [unwired: 3 in, 2 out]
                          n434 = Bundle By Name(cluster=w2532, "X Axis.Angle"=w2530) -> (w2531:T24)
                          n435 = Build Array(u32 1 ("element")) -> (w2535:u32[])
                          n436 = call "Delay Time.vi"("error in (no error)"=w2545, "Delay(ms)"=u32 30) -> ("error out"=w2543:errorcluster)  [unwired: 9 in]
                          n437 = Byte Array To String(unsigned byte array=w2535) -> (string=w2537:string)
                          n438 = call "Z Aux Modbus Set0x.vi"("pdata"=w2537, "error in (no error)"=w2543, "inum"=u16 1, "start"=w2533, "handle"=w2546) -> ("error out"=w2551:errorcluster, "handle out"=w2550:u32)  [unwired: 3 in, 2 out]
                          n439 = call "Check Rotate Done.vi"("error in (no error)"=w2551, "start"=w2533, "phandle in"=w2550) -> ("error out"=w2536:errorcluster)  [unwired: 8 in]
                        }
                      }
                    }
                    frame 72701..141500 {
                      n440 = case shown="\"Stop\"" w2561 {
                        tunnel: w2574 -> [_ w2609]
                        tunnel: w2573 -> [_ w2608]
                        tunnel: w2572 -> [_ w2607]
                        tunnel: w2571 -> [_ w2606]
                        tunnel: w2570 -> [_ w2605]
                        tunnel: 72700.0 ("Creep") -> [_ w2604]
                        tunnel: w2569 -> [_ w2603]
                        tunnel: w2568 -> [_ w2602]
                        tunnel: w2567 -> [w2576 w2601]
                        tunnel: [w2576 w2585] -> w2566
                        tunnel: w2564 -> [_ w2579]
                        tunnel: w2563 -> [w2575 w2581]
                        tunnel: [w2575 w2580] -> w2562
                        frame "False", Default {
                        }
                        frame "Stop" {
                          w2582 = u16 20039 ("start")
                          n441 = call "Return to Middle.vi"("handle"=w2609, "Distance"=w2604, "Decel"=w2603, "Axis"=w2602, "Sramp"=w2608, "Accel"=w2607, "error in (no error)"=w2601, "Lspeed"=w2606, "Speed"=w2605) -> ("handle out"=w2590:u32, "error out"=w2591:errorcluster)  [unwired: 5 in]
                          n442 = Build Array(u32 59 ("element")) -> (w2588:u32[])
                          n443 = Add(x=14.7, y=w2579) -> (x+y=w2578:dbl)
                          n444 = Byte Array To String(unsigned byte array=w2588) -> (string=w2589:string)
                          n445 = call "Z Aux Modbus Set0x.vi"("pdata"=w2589, "error in (no error)"=w2591, "inum"=u16 8, "start"=u16 20032, "handle"=w2590) -> ("error out"=w2594:errorcluster, "handle out"=w2595:u32)  [unwired: 3 in, 2 out]
                          n446 = Bundle By Name(cluster=w2581, "X Axis.Angle"=w2578) -> (w2580:T24)
                          n447 = Build Array(u32 1 ("element")) -> (w2584:u32[])
                          n448 = call "Delay Time.vi"("error in (no error)"=w2594, "Delay(ms)"=u32 30) -> ("error out"=w2592:errorcluster)  [unwired: 9 in]
                          n449 = Byte Array To String(unsigned byte array=w2584) -> (string=w2586:string)
                          n450 = call "Z Aux Modbus Set0x.vi"("pdata"=w2586, "error in (no error)"=w2592, "inum"=u16 1, "start"=w2582, "handle"=w2595) -> ("error out"=w2600:errorcluster, "handle out"=w2599:u32)  [unwired: 3 in, 2 out]
                          n451 = call "Check Rotate Done.vi"("error in (no error)"=w2600, "start"=w2582, "phandle in"=w2599) -> ("error out"=w2585:errorcluster)  [unwired: 8 in]
                        }
                      }
                    }
                  }
                }
              }
            }
          }
          frame "Go to Step3" {
            n452 = Unbundle By Name(w2615) -> ("Deceleration"=w2621:dbl, "phandle out"=w2626:u32, "Axis"=w2613:enum16{"X", "Y", "X+Y"}[], "S ramp"=w2625:dbl, "Acceleration"=w2624:dbl, "Initial Speed"=w2623:dbl, "Speed"=w2622:dbl, "X Axis.Operating State"=w2620:string, "X Axis.Operating State"=w2612:string, "X Axis.Current Position"=w2618:dbl, "X Axis.Current Position"=w2611:dbl, "X Axis.Angle"=w2616:dbl, "X Axis.Angle"=w2610:dbl)
            n453 = for {
              tunnel: w2626 -> [w2644]
              tunnel: w2625 -> [w2643]
              tunnel: w2624 -> [w2642]
              tunnel: w2623 -> [w2641]
              tunnel: w2622 -> [w2640]
              tunnel: w2621 -> [w2639]
              tunnel: w2620 -> [w2638]
              tunnel: w2618 -> [w2635]
              tunnel: w2617 -> [w2634]
              tunnel: w2616 -> [w2633]
              tunnel: w2613 -> [w2630] mode=indexing
              tunnel: w2612 -> [w2629]
              tunnel: w2611 -> [w2628]
              tunnel: w2610 -> [w2627]
              shift-right: [w2636] -> _
              shift-left: w2619 -> [w2637]
              shift-right: [w2631] -> w2614
              shift-left: w2615 -> [w2632]
              n454 = case shown="\"Y\", Default" w2630 {
                selector: w2630 -> [w2645 w2752]
                tunnel: w2644 -> [w2659 w2763]
                tunnel: w2643 -> [w2658 w2762]
                tunnel: w2642 -> [w2657 w2761]
                tunnel: w2641 -> [w2656 w2760]
                tunnel: w2640 -> [w2655 w2759]
                tunnel: w2639 -> [w2654 w2758]
                tunnel: w2638 -> [w2653 _]
                tunnel: w2637 -> [w2652 w2757]
                tunnel: [w2651 w2756] -> w2636
                tunnel: w2635 -> [w2650 _]
                tunnel: w2634 -> [w2649 w2755]
                tunnel: w2633 -> [w2648 _]
                tunnel: w2632 -> [w2647 w2754]
                tunnel: [w2646 w2753] -> w2631
                tunnel: w2629 -> [_ w2751]
                tunnel: w2628 -> [_ w2750]
                tunnel: w2627 -> [_ w2749]
                frame "Y", Default {
                  n455 = case shown="71700..135000" w2650 {
                    tunnel: w2659 -> [_ _ _ w2713]
                    tunnel: w2658 -> [_ _ _ w2712]
                    tunnel: w2657 -> [_ _ _ w2711]
                    tunnel: w2656 -> [_ _ _ w2710]
                    tunnel: w2655 -> [_ _ _ w2709]
                    tunnel: w2654 -> [_ _ _ w2708]
                    tunnel: w2645 -> [_ _ _ w2707]
                    tunnel: w2653 -> [_ w2667 w2686 w2706]
                    tunnel: w2652 -> [w2661 w2669 w2688 w2705]
                    tunnel: [w2661 w2663 w2682 w2704] -> w2651
                    tunnel: w2649 -> [_ w2668 w2687 _]
                    tunnel: w2648 -> [_ _ _ w2700]
                    tunnel: w2647 -> [w2660 w2662 w2681 w2702]
                    tunnel: [w2660 w2662 w2681 w2701] -> w2646
                    frame Default {
                    }
                    frame 0..5999 {
                      n456 = case shown="\"Stop\"" w2667 {
                        tunnel: w2669 -> [w2675 w2680]
                        tunnel: w2668 -> [w2674 w2679]
                        tunnel: [w2675 w2677] -> w2665
                        tunnel: [w2674 w2676] -> w2664
                        frame Default {
                        }
                        frame "Stop" {
                          n457 = Enqueue Element(queue=w2679, element=cluster{"State":T17, "Variable":variant} {"State"=enum."Go to Step1", "Variable"=variant}, error in (no error)=w2680) -> (queue out=w2676:refnum<queue>, error out=w2677:errorcluster)  [unwired: 1 in, 1 out]
                        }
                      }
                      n458 = for {
                        tunnel: w2665 -> [w2673]
                        tunnel: w2664 -> [w2672]
                        tunnel: cluster{"State":T17, "Variable":variant}[] [{"State"=enum."Idle", "Variable"=variant}, {"State"=enum."Update", "Variable"=variant}, {"State"=enum."Go to Step3", "Variable"=variant}] -> [w2671] mode=indexing
                        tunnel: [w2670] -> w2663
                        n459 = Enqueue Element(queue=w2672, element=w2671, error in (no error)=w2673) -> (error out=w2670:errorcluster)  [unwired: 1 in, 2 out]
                      }
                    }
                    frame 6000..71699 {
                      n460 = case shown="\"Stop\"" w2686 {
                        tunnel: w2688 -> [w2694 w2699]
                        tunnel: w2687 -> [w2693 w2698]
                        tunnel: [w2694 w2696] -> w2684
                        tunnel: [w2693 w2695] -> w2683
                        frame Default {
                        }
                        frame "Stop" {
                          n461 = Enqueue Element(queue=w2698, element=cluster{"State":T17, "Variable":variant} {"State"=enum."Go to Step2", "Variable"=variant}, error in (no error)=w2699) -> (queue out=w2695:refnum<queue>, error out=w2696:errorcluster)  [unwired: 1 in, 1 out]
                        }
                      }
                      n462 = for {
                        tunnel: w2684 -> [w2692]
                        tunnel: w2683 -> [w2691]
                        tunnel: cluster{"State":T17, "Variable":variant}[] [{"State"=enum."Idle", "Variable"=variant}, {"State"=enum."Update", "Variable"=variant}, {"State"=enum."Go to Step3", "Variable"=variant}] -> [w2690] mode=indexing
                        tunnel: [w2689] -> w2682
                        n463 = Enqueue Element(queue=w2691, element=w2690, error in (no error)=w2692) -> (error out=w2689:errorcluster)  [unwired: 1 in, 2 out]
                      }
                    }
                    frame 71700..135000 {
                      n464 = case shown="\"Stop\"" w2706 {
                        tunnel: w2713 -> [_ w2748]
                        tunnel: w2712 -> [_ w2747]
                        tunnel: w2711 -> [_ w2746]
                        tunnel: w2710 -> [_ w2745]
                        tunnel: w2709 -> [_ w2744]
                        tunnel: 135000.0 ("Creep") -> [_ w2743]
                        tunnel: w2708 -> [_ w2742]
                        tunnel: w2707 -> [_ w2741]
                        tunnel: w2705 -> [w2715 w2740]
                        tunnel: [w2715 w2724] -> w2704
                        tunnel: w2702 -> [w2714 w2720]
                        tunnel: [w2714 w2719] -> w2701
                        tunnel: w2700 -> [_ w2717]
                        frame "False", Default {
                        }
                        frame "Stop" {
                          w2721 = u16 20047 ("start")
                          n465 = call "Return to Middle.vi"("handle"=w2748, "Distance"=w2743, "Decel"=w2742, "Axis"=w2741, "Sramp"=w2747, "Accel"=w2746, "error in (no error)"=w2740, "Lspeed"=w2745, "Speed"=w2744) -> ("handle out"=w2729:u32, "error out"=w2730:errorcluster)  [unwired: 5 in]
                          n466 = Build Array(u32 63 ("element")) -> (w2727:u32[])
                          n467 = Byte Array To String(unsigned byte array=w2727) -> (string=w2728:string)
                          n468 = call "Z Aux Modbus Set0x.vi"("pdata"=w2728, "error in (no error)"=w2730, "inum"=u16 8, "start"=u16 20040, "handle"=w2729) -> ("error out"=w2733:errorcluster, "handle out"=w2734:u32)  [unwired: 3 in, 2 out]
                          n469 = Add(x=12.92, y=w2717) -> (x+y=w2718:dbl)
                          n470 = Bundle By Name(cluster=w2720, "X Axis.Angle"=w2718) -> (w2719:T24)
                          n471 = Build Array(u32 1 ("element")) -> (w2723:u32[])
                          n472 = call "Delay Time.vi"("error in (no error)"=w2733, "Delay(ms)"=u32 30) -> ("error out"=w2731:errorcluster)  [unwired: 9 in]
                          n473 = Byte Array To String(unsigned byte array=w2723) -> (string=w2725:string)
                          n474 = call "Z Aux Modbus Set0x.vi"("pdata"=w2725, "error in (no error)"=w2731, "inum"=u16 1, "start"=w2721, "handle"=w2734) -> ("error out"=w2739:errorcluster, "handle out"=w2738:u32)  [unwired: 3 in, 2 out]
                          n475 = call "Check Rotate Done.vi"("error in (no error)"=w2739, "start"=w2721, "phandle in"=w2738) -> ("error out"=w2724:errorcluster)  [unwired: 8 in]
                        }
                      }
                    }
                  }
                }
                frame "X" {
                  n476 = case shown="Default" w2750 {
                    tunnel: w2763 -> [_ _ _ w2817]
                    tunnel: w2762 -> [_ _ _ w2816]
                    tunnel: w2761 -> [_ _ _ w2815]
                    tunnel: w2760 -> [_ _ _ w2814]
                    tunnel: w2759 -> [_ _ _ w2813]
                    tunnel: w2758 -> [_ _ _ w2812]
                    tunnel: w2752 -> [_ _ _ w2811]
                    tunnel: w2751 -> [_ w2771 w2790 w2810]
                    tunnel: w2757 -> [w2765 w2773 w2792 w2809]
                    tunnel: [w2765 w2767 w2786 w2808] -> w2756
                    tunnel: w2755 -> [_ w2772 w2791 _]
                    tunnel: w2749 -> [_ _ _ w2804]
                    tunnel: w2754 -> [w2764 w2766 w2785 w2806]
                    tunnel: [w2764 w2766 w2785 w2805] -> w2753
                    frame Default {
                    }
                    frame 0..12199 {
                      n477 = case shown="Default" w2771 {
                        tunnel: w2773 -> [w2779 w2784]
                        tunnel: w2772 -> [w2778 w2783]
                        tunnel: [w2779 w2781] -> w2769
                        tunnel: [w2778 w2780] -> w2768
                        frame Default {
                        }
                        frame "Stop" {
                          n478 = Enqueue Element(queue=w2783, element=cluster{"State":T17, "Variable":variant} {"State"=enum."Go to Step1", "Variable"=variant}, error in (no error)=w2784) -> (queue out=w2780:refnum<queue>, error out=w2781:errorcluster)  [unwired: 1 in, 1 out]
                        }
                      }
                      n479 = for {
                        tunnel: w2769 -> [w2777]
                        tunnel: w2768 -> [w2776]
                        tunnel: cluster{"State":T17, "Variable":variant}[] [{"State"=enum."Idle", "Variable"=variant}, {"State"=enum."Update", "Variable"=variant}, {"State"=enum."Go to Step3", "Variable"=variant}] -> [w2775] mode=indexing
                        tunnel: [w2774] -> w2767
                        n480 = Enqueue Element(queue=w2776, element=w2775, error in (no error)=w2777) -> (error out=w2774:errorcluster)  [unwired: 1 in, 2 out]
                      }
                    }
                    frame 12200..72699 {
                      n481 = case shown="\"Stop\"" w2790 {
                        tunnel: w2792 -> [w2798 w2803]
                        tunnel: w2791 -> [w2797 w2802]
                        tunnel: [w2798 w2800] -> w2788
                        tunnel: [w2797 w2799] -> w2787
                        frame Default {
                        }
                        frame "Stop" {
                          n482 = Enqueue Element(queue=w2802, element=cluster{"State":T17, "Variable":variant} {"State"=enum."Go to Step2", "Variable"=variant}, error in (no error)=w2803) -> (queue out=w2799:refnum<queue>, error out=w2800:errorcluster)  [unwired: 1 in, 1 out]
                        }
                      }
                      n483 = for {
                        tunnel: w2788 -> [w2796]
                        tunnel: w2787 -> [w2795]
                        tunnel: cluster{"State":T17, "Variable":variant}[] [{"State"=enum."Idle", "Variable"=variant}, {"State"=enum."Update", "Variable"=variant}, {"State"=enum."Go to Step3", "Variable"=variant}] -> [w2794] mode=indexing
                        tunnel: [w2793] -> w2786
                        n484 = Enqueue Element(queue=w2795, element=w2794, error in (no error)=w2796) -> (error out=w2793:errorcluster)  [unwired: 1 in, 2 out]
                      }
                    }
                    frame 72700..141500 {
                      n485 = case shown="\"Stop\"" w2810 {
                        tunnel: w2817 -> [_ w2852]
                        tunnel: w2816 -> [_ w2851]
                        tunnel: w2815 -> [_ w2850]
                        tunnel: w2814 -> [_ w2849]
                        tunnel: w2813 -> [_ w2848]
                        tunnel: 141500.0 ("Creep") -> [_ w2847]
                        tunnel: w2812 -> [_ w2846]
                        tunnel: w2811 -> [_ w2845]
                        tunnel: w2809 -> [w2819 w2844]
                        tunnel: [w2819 w2828] -> w2808
                        tunnel: w2806 -> [w2818 w2824]
                        tunnel: [w2818 w2823] -> w2805
                        tunnel: w2804 -> [_ w2821]
                        frame "False", Default {
                        }
                        frame "Stop" {
                          w2825 = u16 20039 ("start")
                          n486 = call "Return to Middle.vi"("handle"=w2852, "Distance"=w2847, "Decel"=w2846, "Axis"=w2845, "Sramp"=w2851, "Accel"=w2850, "error in (no error)"=w2844, "Lspeed"=w2849, "Speed"=w2848) -> ("handle out"=w2833:u32, "error out"=w2834:errorcluster)  [unwired: 5 in]
                          n487 = Build Array(u32 58 ("element")) -> (w2831:u32[])
                          n488 = Byte Array To String(unsigned byte array=w2831) -> (string=w2832:string)
                          n489 = call "Z Aux Modbus Set0x.vi"("pdata"=w2832, "error in (no error)"=w2834, "inum"=u16 8, "start"=u16 20032, "handle"=w2833) -> ("error out"=w2837:errorcluster, "handle out"=w2838:u32)  [unwired: 3 in, 2 out]
                          n490 = Add(x=-14.7, y=w2821) -> (x+y=w2822:dbl)
                          n491 = Bundle By Name(cluster=w2824, "X Axis.Angle"=w2822) -> (w2823:T24)
                          n492 = Build Array(u32 1 ("element")) -> (w2827:u32[])
                          n493 = call "Delay Time.vi"("error in (no error)"=w2837, "Delay(ms)"=u32 30) -> ("error out"=w2835:errorcluster)  [unwired: 9 in]
                          n494 = Byte Array To String(unsigned byte array=w2827) -> (string=w2829:string)
                          n495 = call "Z Aux Modbus Set0x.vi"("pdata"=w2829, "error in (no error)"=w2835, "inum"=u16 1, "start"=w2825, "handle"=w2838) -> ("error out"=w2843:errorcluster, "handle out"=w2842:u32)  [unwired: 3 in, 2 out]
                          n496 = call "Check Rotate Done.vi"("error in (no error)"=w2843, "start"=w2825, "phandle in"=w2842) -> ("error out"=w2828:errorcluster)  [unwired: 8 in]
                        }
                      }
                    }
                  }
                }
              }
            }
          }
          frame "Initial to Y Step" {
            w2853 = enum16{"X", "Y", "X+Y"}[] [enum."X", enum."Y"] items=["X", "Y", "X+Y"] ("Axis")
            n497 = for {
              tunnel: w2858 -> [w2862]
              tunnel: w2857 -> [w2861]
              tunnel: cluster{"State":T17, "Variable":variant}[] [{"State"=enum."Return to Zero", "Variable"=variant}, {"State"=enum."Return to Origin", "Variable"=variant}] -> [w2860] mode=indexing
              tunnel: [w2859] -> _
              n498 = Enqueue Element(queue=w2861, element=w2860, error in (no error)=w2862) -> (error out=w2859:errorcluster)  [unwired: 1 in, 2 out]
            }
            n499 = Bundle By Name(cluster=w2855, "Axis"=w2853) -> (w2854:T24)
          }
          frame "Select Speed" {
            n500 = Variant To Data(error in=w2870, type=enum32{"30", "50000"}."50000" ("Select Speed"), Variant=w2869) -> (data=w2867:enum32{"30", "50000"}, error out=w2868:errorcluster)
            n501 = case shown="\"30\"" w2867 {
              tunnel: w2868 -> [w2873 w2875]
              tunnel: [w2872 w2876] -> _
              tunnel: [w2871 w2874] -> w2864
              frame "50000", Default {
                w2871 = 50000.0 ("Speed")
                n502 = property on="Speed" class="DigNum (strict)"(error in=w2873, "Value"=w2871) -> (error out=w2872:errorcluster)  [unwired: 1 in, 1 out]
              }
              frame "30" {
                w2874 = 30.0 ("Speed")
                n503 = property on="Speed" class="DigNum (strict)"(error in=w2875, "Value"=w2874) -> (error out=w2876:errorcluster)  [unwired: 1 in, 1 out]
              }
            }
            n504 = Bundle By Name(cluster=w2866, "Speed"=w2864) -> (w2865:T24)
          }
          frame "Move" {
            n505 = Unbundle By Name(w2879) -> ("Direct of movement"=w2883:enum16{"Forward", "Backward"}, "Move Method"=w2887:enum16{"Continue", "Inching"}, "Deceleration"=w2886:dbl, "Distance"=w2884:dbl, "phandle out"=w2892:u32, "Axis"=w2885:enum16{"X", "Y", "X+Y"}[], "S ramp"=w2891:dbl, "Acceleration"=w2890:dbl, "Initial Speed"=w2889:dbl, "Speed"=w2888:dbl, "Move Mode"=w2882:enum16{"Relative", "Absolute"}, "X Axis.Operating State"=w2881:string, "X Axis.Operating State"=w2880:string)
            n506 = for {
              tunnel: w2892 -> [w2909]
              tunnel: w2891 -> [w2908]
              tunnel: w2890 -> [w2907]
              tunnel: w2889 -> [w2906]
              tunnel: w2888 -> [w2905]
              tunnel: w2887 -> [w2904]
              tunnel: w2886 -> [w2903]
              tunnel: w2885 -> [w2902] mode=indexing
              tunnel: w2884 -> [w2901]
              tunnel: w2883 -> [w2900]
              tunnel: w2882 -> [w2899]
              tunnel: w2881 -> [w2898]
              tunnel: w2880 -> [w2897]
              shift-right: [w2895] -> w2878
              shift-left: w2879 -> [w2896]
              shift-right: [w2893] -> _
              shift-left: w2877 -> [w2894]
              n507 = case shown="\"X\", Default" w2902 {
                selector: w2902 -> [w2918 w2953 _]
                tunnel: w2909 -> [w2925 w2960 w2999]
                tunnel: w2908 -> [w2924 w2959 w2998]
                tunnel: w2907 -> [w2923 w2958 w2997]
                tunnel: w2906 -> [w2922 w2957 w2996]
                tunnel: w2905 -> [w2921 w2956 w2995]
                tunnel: w2904 -> [w2920 w2955 w2994]
                tunnel: w2903 -> [w2919 w2954 w2993]
                tunnel: w2901 -> [w2916 w2951 w2992]
                tunnel: w2900 -> [w2917 w2952 w2991]
                tunnel: w2899 -> [w2915 w2950 w2990]
                tunnel: w2898 -> [w2914 _ w2989]
                tunnel: w2897 -> [_ w2949 w2987]
                tunnel: w2896 -> [w2913 w2948 w2983]
                tunnel: [w2912 w2947 w2982] -> w2895
                tunnel: w2894 -> [w2911 w2946 w2981]
                tunnel: [w2910 w2945 w2980] -> w2893
                frame "X", Default {
                  n508 = case shown="\"Stop\"" w2914 {
                    tunnel: w2925 -> [_ w2944]
                    tunnel: w2924 -> [_ w2943]
                    tunnel: w2923 -> [_ w2942]
                    tunnel: w2922 -> [_ w2941]
                    tunnel: w2921 -> [_ w2940]
                    tunnel: w2920 -> [_ w2939]
                    tunnel: w2919 -> [_ w2938]
                    tunnel: w2918 -> [_ w2937]
                    tunnel: w2917 -> [_ w2936]
                    tunnel: w2916 -> [_ w2935]
                    tunnel: w2915 -> [_ w2934]
                    tunnel: w2913 -> [w2927 w2933]
                    tunnel: [w2927 w2932] -> w2912
                    tunnel: w2911 -> [w2926 w2929]
                    tunnel: [w2926 w2928] -> w2910
                    frame "False", Default {
                    }
                    frame "Stop" {
                      n509 = Get Date/Time In Seconds() -> (seconds since 1Jan1904=w2931:timestamp)
                      n510 = call "Move.vi"("handle"=w2944, "Distance"=w2935, "Decel"=w2938, "Move Method"=w2939, "Direct of movement"=w2936, "Axis"=w2937, "Sramp"=w2943, "Accel"=w2942, "error in (no error)"=w2929, "Lspeed"=w2941, "Speed"=w2940, "Move Mode"=w2934) -> ("error out"=w2928:errorcluster)  [unwired: 3 in]
                      n511 = To Double Precision Float(number=w2931) -> (double precision float=w2930:dbl)
                      n512 = Bundle By Name(cluster=w2933, "Start Time"=w2930) -> (w2932:T24)
                    }
                  }
                }
                frame "Y" {
                  n513 = case shown="\"Stop\"" w2949 {
                    tunnel: w2960 -> [_ w2979]
                    tunnel: w2959 -> [_ w2978]
                    tunnel: w2958 -> [_ w2977]
                    tunnel: w2957 -> [_ w2976]
                    tunnel: w2956 -> [_ w2975]
                    tunnel: w2955 -> [_ w2974]
                    tunnel: w2954 -> [_ w2973]
                    tunnel: w2953 -> [_ w2972]
                    tunnel: w2952 -> [_ w2971]
                    tunnel: w2951 -> [_ w2970]
                    tunnel: w2950 -> [_ w2969]
                    tunnel: w2948 -> [w2962 w2966]
                    tunnel: [w2962 w2965] -> w2947
                    tunnel: w2946 -> [w2961 w2964]
                    tunnel: [w2961 w2963] -> w2945
                    frame "False", Default {
                    }
                    frame "Stop" {
                      n514 = Get Date/Time In Seconds() -> (seconds since 1Jan1904=w2968:timestamp)
                      n515 = To Double Precision Float(number=w2968) -> (double precision float=w2967:dbl)
                      n516 = call "Move.vi"("handle"=w2979, "Distance"=w2970, "Decel"=w2973, "Move Method"=w2974, "Direct of movement"=w2971, "Axis"=w2972, "Sramp"=w2978, "Accel"=w2977, "error in (no error)"=w2964, "Lspeed"=w2976, "Speed"=w2975, "Move Mode"=w2969) -> ("error out"=w2963:errorcluster)  [unwired: 3 in]
                      n517 = Bundle By Name(cluster=w2966, "Start Time"=w2967) -> (w2965:T24)
                    }
                  }
                }
                frame "X+Y" {
                  w2988 = "Stop" ("y")
                  n518 = Equal?(x=w2989, y=w2988) -> (x = y?=w2986:bool)
                  n519 = Equal?(x=w2988, y=w2987) -> (x = y?=w2984:bool)
                  n520 = And(x=w2986, y=w2984) -> (x .and. y?=w2985:bool)
                  n521 = case shown="False" w2985 {
                    tunnel: w2999 -> [_ w3018]
                    tunnel: w2998 -> [_ w3017]
                    tunnel: w2997 -> [_ w3016]
                    tunnel: w2996 -> [_ w3015]
                    tunnel: w2995 -> [_ w3014]
                    tunnel: w2994 -> [_ w3013]
                    tunnel: w2993 -> [_ w3012]
                    tunnel: w2992 -> [_ w3010]
                    tunnel: w2991 -> [_ w3009]
                    tunnel: w2990 -> [_ w3008]
                    tunnel: w2983 -> [w3001 w3007]
                    tunnel: [w3001 w3006] -> w2982
                    tunnel: w2981 -> [w3000 w3003]
                    tunnel: [w3000 w3002] -> w2980
                    frame False {
                    }
                    frame True {
                      n522 = Get Date/Time In Seconds() -> (seconds since 1Jan1904=w3005:timestamp)
                      n523 = To Double Precision Float(number=w3005) -> (double precision float=w3004:dbl)
                      n524 = for {
                        tunnel: w3018 -> [w3031]
                        tunnel: w3017 -> [w3030]
                        tunnel: w3016 -> [w3029]
                        tunnel: w3015 -> [w3028]
                        tunnel: w3014 -> [w3027]
                        tunnel: w3013 -> [w3026]
                        tunnel: w3012 -> [w3025]
                        tunnel: i32[] [0, 1] -> [w3024] mode=indexing
                        tunnel: w3010 -> [w3023]
                        tunnel: w3009 -> [w3022]
                        tunnel: w3008 -> [w3021]
                        tunnel: w3003 -> [w3020]
                        tunnel: [w3019] -> w3002
                        n525 = call "Move.vi"("handle"=w3031, "Distance"=w3023, "Decel"=w3025, "Move Method"=w3026, "Direct of movement"=w3022, "Axis"=w3024, "Sramp"=w3030, "Accel"=w3029, "error in (no error)"=w3020, "Lspeed"=w3028, "Speed"=w3027, "Move Mode"=w3021) -> ("error out"=w3019:errorcluster)  [unwired: 3 in]
                      }
                      n526 = Bundle By Name(cluster=w3007, "Start Time"=w3004) -> (w3006:T24)
                    }
                  }
                }
              }
            }
          }
          frame "auto mode" {
            # "move and rotate"
            n527 = Unbundle By Name(w3033) -> ("dy Path"=w3032:T8)
            n528 = Variant To Data(error in=w3047, type=i32[] [], Variant=w3060) -> (data=w3045:i32[], error out=w3035:errorcluster)
            n529 = Index Array(array=w3045) -> (element #1=w3043:i32, element #2=w3044:i32)  [unwired: 2 in]
            n530 = Bundle By Name(cluster=w3033, "index"=w3044) -> (w3052:T24)
            n531 = property on="auto step finish?" class="Bool (strict)"(error in=w3035, "Value"=FALSE ("auto step finish?")) -> ()  [unwired: 1 in, 2 out]
            n532 = property on="dy Path" class="Arr (strict)"("Value"=w3032) -> ()  [unwired: 2 in, 2 out]
            n533 = property on="autoSliderfinish?" class="Bool (strict)"(error in=w3035, "Value"=FALSE ("autoSlider")) -> (error out=w3039:errorcluster)  [unwired: 1 in, 1 out]
            n534 = case shown="0, Default" w3043 {
              tunnel: [enum16{"X", "Y", "X+Y"}."X" ("Axis") enum16{"X", "Y", "X+Y"}."Y" ("Axis") enum16{"X", "Y", "X+Y"}."X+Y" ("Axis")] -> w3042
              frame 0, Default {
              }
              frame 1 {
              }
              frame 2 {
              }
            }
            n535 = flat-sequence {
              tunnel: w3052 -> [w3067]
              tunnel: w3039 -> [w3072]
              tunnel: [w3071] -> w3059
              tunnel: [w3070] -> w3057
              tunnel: w3055 -> [w3069]
              tunnel: [w3068] -> w3053
              tunnel: "Rotate" -> [w3066]
              tunnel: w3042 -> [w3065]
              tunnel: [w3064] -> w3040
              tunnel: w3059 -> [w3097]
              tunnel: [w3097] -> w3058
              tunnel: w3057 -> [w3096]
              tunnel: [w3096] -> w3056
              tunnel: [w3094] -> w3054
              tunnel: w3053 -> [w3094]
              tunnel: [w3093] -> w3041
              tunnel: w3040 -> [w3093]
              tunnel: [w3106] -> w3051
              tunnel: [w3109] -> _
              tunnel: w3058 -> [w3108]
              tunnel: w3056 -> [w3107]
              tunnel: w3054 -> [w3112]
              tunnel: [w3111] -> w3049
              tunnel: "Rotate" -> [w3105]
              tunnel: "Rotate" -> [w3110]
              tunnel: w3042 -> [w3104]
              tunnel: w3041 -> [w3103]
              tunnel: w3037 -> [w3101]
              tunnel: w3036 -> [w3100]
              frame #0 {
                # "angle return\n to zero"
                n536 = disable-structure shown="Enabled" {
                  disable-tunnel: w3069 -> [w3091 w3092]
                  disable-tunnel: [w3090 w3092] -> w3068
                  disable-tunnel: ["origin" _] -> w3064
                  frame Disabled {
                    n537 = Bundle By Name(cluster=T21 {"Enum"=enum."WRITE", "Variable"=variant}, "Variable"="origin") -> (w3089:T21)
                    n538 = Enqueue Element(queue=w3091, element=w3089) -> (queue out=w3090:refnum<queue>)  [unwired: 2 in, 2 out]
                  }
                  frame Enabled {
                  }
                }
                n539 = case shown="False" w3066 {
                  tunnel: w3072 -> [w3073 w3078]
                  tunnel: [w3073 w3077] -> w3071
                  tunnel: [w3074 w3076] -> w3070
                  tunnel: w3067 -> [w3074 w3079]
                  tunnel: w3065 -> [_ w3075]
                  frame False {
                  }
                  frame True {
                    n540 = disable-structure shown="Enabled" {
                      disable-tunnel: w3079 -> [w3084 w3085]
                      disable-tunnel: w3078 -> [w3083 w3086]
                      disable-tunnel: [w3082 w3086] -> w3077
                      disable-tunnel: [w3081 w3085] -> w3076
                      disable-tunnel: w3075 -> [w3080 _]
                      frame Disabled {
                        n541 = call "return zero.vi"("Axis"=w3080, "error IN"=w3083, "Data IN"=w3084) -> ("error out"=w3082:errorcluster, "Data out"=w3081:T24)  [unwired: 7 in]
                      }
                      frame Enabled {
                      }
                    }
                  }
                }
              }
              frame #1 {
                n542 = Wait (ms)(milliseconds to wait=u32 0) -> ()  [unwired: 1 out]
              }
              frame #2 {
                n543 = disable-structure shown="Enabled" {
                  disable-tunnel: w3112 -> [w3119 _]
                  disable-tunnel: [w3117 0.0 ("tan(x)")] -> w3111
                  disable-tunnel: w3110 -> [w3116 _]
                  disable-tunnel: w3107 -> [w3114 _]
                  disable-tunnel: w3103 -> [w3113 _]
                  disable-tunnel: [_ w3134] -> w3098
                  disable-tunnel: [_ w3133] -> w3099
                  frame Disabled {
                    n544 = Unbundle By Name(w3114) -> ("big angle"=w3118:dbl[], "index"=w3115:dbl)
                    n545 = Index Array(array=w3118, index=w3115) -> (element=w3117:dbl)
                    n546 = case shown="False" w3116 {
                      tunnel: w3119 -> [w3123 w3132]
                      tunnel: w3117 -> [w3122 _]
                      tunnel: w3115 -> [_ w3128]
                      tunnel: w3113 -> [_ w3124]
                      frame True {
                        n547 = Bundle By Name(cluster=T21 {"Enum"=enum."WRITE", "Variable"=variant}, "Variable"=w3122) -> (w3121:T21)
                        n548 = Enqueue Element(queue=w3123, element=w3121) -> ()  [unwired: 2 in, 3 out]
                      }
                      frame False {
                        n549 = property on="x angle" class="Arr (strict)"() -> ("Value"=w3129:dbl[])  [unwired: 2 in, 2 out]
                        n550 = Index Array(array=w3129, index=w3128) -> (element=w3127:dbl)
                        n551 = Round To Nearest(number=w3127) -> (nearest integer value=w3125:dbl)
                        n552 = Add(x=w3125, y=w3124) -> (x+y=w3126:dbl)
                        n553 = Bundle By Name(cluster=T21 {"Enum"=enum."WRITE", "Variable"=variant}, "Variable"=w3126) -> (w3131:T21)
                        n554 = Enqueue Element(queue=w3132, element=w3131) -> ()  [unwired: 2 in, 3 out]
                      }
                    }
                  }
                  frame Enabled {
                    n555 = property on="Speed" class="DigNum (strict)"() -> ("Value"=w3134:dbl)  [unwired: 2 in, 2 out]
                    n556 = property on="DYNAMIC 2" class="Arr (strict)"() -> ("Value"=w3133:T1)  [unwired: 2 in, 2 out]
                  }
                }
                n557 = property on="s/d setting" class="Bool (strict)"() -> ("Value"=w3102:bool)  [unwired: 2 in, 2 out]
                n558 = call "Untitled 2.vi"("Data IN"=w3107, "Axis"=w3104, "Rotate"=w3105, "dynamic"=w3102, "Array 2"=w3101, "error IN"=w3108, "DYNAMIC"=w3100, "DYNAMIC 2"=w3099, "Speed"=w3098) -> ("Data OUT"=w3106:T24, "error out"=w3109:errorcluster)  [unwired: 5 in]
              }
            }
            n559 = property on="Array" class="Arr (strict)"() -> ("Value"=w3037:T2)  [unwired: 2 in, 2 out]
            n560 = property on="DYNAMIC" class="Arr (strict)"() -> ("Value"=w3036:T1)  [unwired: 2 in, 2 out]
            n561 = Bundle By Name(cluster=w3051, "big motion angle"=w3049) -> (w3050:T24)
          }
          frame "Inching" {
            n562 = Unbundle By Name(w3140) -> ("Direct of movement"=w3143:enum16{"Forward", "Backward"}, "Deceleration"=w3146:dbl, "Distance"=w3144:dbl, "phandle out"=w3151:u32, "Axis"=w3145:enum16{"X", "Y", "X+Y"}[], "S ramp"=w3150:dbl, "Acceleration"=w3149:dbl, "Initial Speed"=w3148:dbl, "Speed"=w3147:dbl, "X Axis.Operating State"=w3142:string, "X Axis.Operating State"=w3141:string, "X Axis.Current Position"=w3137:dbl, "X Axis.Current Position"=w3136:dbl)  [unwired: 2 out]
            n563 = for {
              tunnel: w3151 -> [w3170]
              tunnel: w3150 -> [w3169]
              tunnel: w3149 -> [w3168]
              tunnel: w3148 -> [w3167]
              tunnel: w3147 -> [w3166]
              tunnel: w3146 -> [w3165]
              tunnel: w3145 -> [w3164] mode=indexing
              tunnel: w3144 -> [w3163]
              tunnel: w3143 -> [w3162]
              tunnel: w3142 -> [w3161]
              tunnel: w3141 -> [w3160]
              shift-right: [w3158] -> w3139
              shift-left: w3140 -> [w3159]
              shift-right: [w3156] -> _
              shift-left: w3138 -> [w3157]
              tunnel: w3137 -> [w3153]
              tunnel: w3136 -> [w3152]
              n564 = case shown="\"Y\"" w3164 {
                selector: w3164 -> [w3184 w3242 _]
                tunnel: w3170 -> [w3191 w3249 w3306]
                tunnel: w3169 -> [w3190 w3248 w3305]
                tunnel: w3168 -> [w3189 w3247 w3304]
                tunnel: w3167 -> [w3188 w3246 w3303]
                tunnel: w3166 -> [w3187 w3245 w3302]
                tunnel: enum16{"Continue", "Inching"}."Inching" ("Move Method") -> [w3186 w3244 w3301]
                tunnel: w3165 -> [w3185 w3243 w3300]
                tunnel: w3163 -> [w3175 w3233 w3299]
                tunnel: w3162 -> [w3183 w3241 w3298]
                tunnel: enum16{"Relative", "Absolute"}."Relative" ("Move Mode") -> [w3182 w3240 w3297]
                tunnel: w3161 -> [w3181 _ w3296]
                tunnel: w3160 -> [_ w3239 w3294]
                tunnel: w3159 -> [w3180 w3238 w3290]
                tunnel: [w3179 w3237 w3289] -> w3158
                tunnel: w3157 -> [w3178 w3236 w3288]
                tunnel: [w3177 w3235 w3287] -> w3156
                tunnel: w3153 -> [w3176 _ _]
                tunnel: w3152 -> [_ w3234 _]
                frame "X", Default {
                  n565 = Add(x=w3175, y=w3176) -> (x+y=w3174:dbl)
                  n566 = In Range and Coerce(upper limit=141500.0, x=w3174, lower limit=12200.0) -> (In Range?=w3173:bool)  [unwired: 1 out]
                  n567 = case shown="False" w3173 {
                    tunnel: w3191 -> [_ w3209]
                    tunnel: w3190 -> [_ w3208]
                    tunnel: w3189 -> [_ w3207]
                    tunnel: w3188 -> [_ w3206]
                    tunnel: w3187 -> [_ w3205]
                    tunnel: w3186 -> [_ w3204]
                    tunnel: w3185 -> [_ w3203]
                    tunnel: w3184 -> [_ w3202]
                    tunnel: w3183 -> [_ w3201]
                    tunnel: w3175 -> [_ w3200]
                    tunnel: w3182 -> [_ w3199]
                    tunnel: w3181 -> [_ w3198]
                    tunnel: w3180 -> [w3192 w3197]
                    tunnel: [w3192 w3196] -> w3179
                    tunnel: w3178 -> [w3193 w3195]
                    tunnel: [w3193 w3194] -> w3177
                    frame False {
                    }
                    frame True {
                      n568 = case shown="\"Stop\"" w3198 {
                        tunnel: w3209 -> [_ w3228]
                        tunnel: w3208 -> [_ w3227]
                        tunnel: w3207 -> [_ w3226]
                        tunnel: w3206 -> [_ w3225]
                        tunnel: w3205 -> [_ w3224]
                        tunnel: w3204 -> [_ w3223]
                        tunnel: w3203 -> [_ w3222]
                        tunnel: w3202 -> [_ w3221]
                        tunnel: w3201 -> [_ w3220]
                        tunnel: w3200 -> [_ w3219]
                        tunnel: w3199 -> [_ w3218]
                        tunnel: w3197 -> [w3211 w3217]
                        tunnel: [w3211 w3216] -> w3196
                        tunnel: w3195 -> [w3210 w3213]
                        tunnel: [w3210 w3212] -> w3194
                        frame "False", Default {
                        }
                        frame "Stop" {
                          n569 = Get Date/Time In Seconds() -> (seconds since 1Jan1904=w3215:timestamp)
                          n570 = call "Move.vi"("handle"=w3228, "Distance"=w3219, "Decel"=w3222, "Move Method"=w3223, "Direct of movement"=w3220, "Axis"=w3221, "Sramp"=w3227, "Accel"=w3226, "error in (no error)"=w3213, "Lspeed"=w3225, "Speed"=w3224, "Move Mode"=w3218) -> ("error out"=w3212:errorcluster)  [unwired: 3 in]
                          n571 = To Double Precision Float(number=w3215) -> (double precision float=w3214:dbl)
                          n572 = Bundle By Name(cluster=w3217, "Start Time"=w3214) -> (w3216:T24)
                        }
                      }
                    }
                  }
                }
                frame "Y" {
                  n573 = Add(x=w3233, y=w3234) -> (x+y=w3232:dbl)
                  n574 = In Range and Coerce(upper limit=135000.0, x=w3232, lower limit=6000.0) -> (In Range?=w3229:bool)  [unwired: 1 out]
                  n575 = case shown="False" w3229 {
                    tunnel: w3249 -> [_ w3267]
                    tunnel: w3248 -> [_ w3266]
                    tunnel: w3247 -> [_ w3265]
                    tunnel: w3246 -> [_ w3264]
                    tunnel: w3245 -> [_ w3263]
                    tunnel: w3244 -> [_ w3262]
                    tunnel: w3243 -> [_ w3261]
                    tunnel: w3242 -> [_ w3260]
                    tunnel: w3241 -> [_ w3259]
                    tunnel: w3240 -> [_ w3258]
                    tunnel: w3239 -> [_ w3257]
                    tunnel: w3238 -> [w3250 w3256]
                    tunnel: [w3250 w3255] -> w3237
                    tunnel: w3236 -> [w3251 w3254]
                    tunnel: [w3251 w3253] -> w3235
                    tunnel: w3233 -> [_ w3252]
                    frame False {
                    }
                    frame True {
                      n576 = case shown="\"Stop\"" w3257 {
                        tunnel: w3267 -> [_ w3286]
                        tunnel: w3266 -> [_ w3285]
                        tunnel: w3265 -> [_ w3284]
                        tunnel: w3264 -> [_ w3283]
                        tunnel: w3263 -> [_ w3282]
                        tunnel: w3262 -> [_ w3281]
                        tunnel: w3261 -> [_ w3280]
                        tunnel: w3260 -> [_ w3279]
                        tunnel: w3259 -> [_ w3278]
                        tunnel: w3252 -> [_ w3277]
                        tunnel: w3258 -> [_ w3276]
                        tunnel: w3256 -> [w3269 w3273]
                        tunnel: [w3269 w3272] -> w3255
                        tunnel: w3254 -> [w3268 w3271]
                        tunnel: [w3268 w3270] -> w3253
                        frame "False", Default {
                        }
                        frame "Stop" {
                          n577 = Get Date/Time In Seconds() -> (seconds since 1Jan1904=w3275:timestamp)
                          n578 = To Double Precision Float(number=w3275) -> (double precision float=w3274:dbl)
                          n579 = call "Move.vi"("handle"=w3286, "Distance"=w3277, "Decel"=w3280, "Move Method"=w3281, "Direct of movement"=w3278, "Axis"=w3279, "Sramp"=w3285, "Accel"=w3284, "error in (no error)"=w3271, "Lspeed"=w3283, "Speed"=w3282, "Move Mode"=w3276) -> ("error out"=w3270:errorcluster)  [unwired: 3 in]
                          n580 = Bundle By Name(cluster=w3273, "Start Time"=w3274) -> (w3272:T24)
                        }
                      }
                    }
                  }
                }
                frame "X+Y" {
                  w3295 = "Stop" ("y")
                  n581 = Equal?(x=w3296, y=w3295) -> (x = y?=w3293:bool)
                  n582 = Equal?(x=w3295, y=w3294) -> (x = y?=w3291:bool)
                  n583 = And(x=w3293, y=w3291) -> (x .and. y?=w3292:bool)
                  n584 = case shown="True" w3292 {
                    tunnel: w3306 -> [_ w3325]
                    tunnel: w3305 -> [_ w3324]
                    tunnel: w3304 -> [_ w3323]
                    tunnel: w3303 -> [_ w3322]
                    tunnel: w3302 -> [_ w3321]
                    tunnel: w3301 -> [_ w3320]
                    tunnel: w3300 -> [_ w3319]
                    tunnel: w3299 -> [_ w3317]
                    tunnel: w3298 -> [_ w3316]
                    tunnel: w3297 -> [_ w3315]
                    tunnel: w3290 -> [w3308 w3314]
                    tunnel: [w3308 w3313] -> w3289
                    tunnel: w3288 -> [w3307 w3310]
                    tunnel: [w3307 w3309] -> w3287
                    frame False {
                    }
                    frame True {
                      n585 = Get Date/Time In Seconds() -> (seconds since 1Jan1904=w3312:timestamp)
                      n586 = To Double Precision Float(number=w3312) -> (double precision float=w3311:dbl)
                      n587 = for {
                        tunnel: w3325 -> [w3338]
                        tunnel: w3324 -> [w3337]
                        tunnel: w3323 -> [w3336]
                        tunnel: w3322 -> [w3335]
                        tunnel: w3321 -> [w3334]
                        tunnel: w3320 -> [w3333]
                        tunnel: w3319 -> [w3332]
                        tunnel: i32[] [0, 1] -> [w3331] mode=indexing
                        tunnel: w3317 -> [w3330]
                        tunnel: w3316 -> [w3329]
                        tunnel: w3315 -> [w3328]
                        tunnel: w3310 -> [w3327]
                        tunnel: [w3326] -> w3309
                        n588 = call "Move.vi"("handle"=w3338, "Distance"=w3330, "Decel"=w3332, "Move Method"=w3333, "Direct of movement"=w3329, "Axis"=w3331, "Sramp"=w3337, "Accel"=w3336, "error in (no error)"=w3327, "Lspeed"=w3335, "Speed"=w3334, "Move Mode"=w3328) -> ("error out"=w3326:errorcluster)  [unwired: 3 in]
                      }
                      n589 = Bundle By Name(cluster=w3314, "Start Time"=w3311) -> (w3313:T24)
                    }
                  }
                }
              }
            }
          }
          frame "Stop" {
            n590 = Flush Queue(queue=w3343, error in (no error)=w3342) -> (queue out=w3340:refnum<queue>, error out=w3341:errorcluster)  [unwired: 1 out]
            n591 = Enqueue Element At Opposite End(queue=w3340, element=cluster{"State":T17, "Variable":variant} {"State"=enum."Idle", "Variable"=variant}, error in (no error)=w3341) -> (error out=w3345:errorcluster)  [unwired: 1 in, 2 out]
            n592 = Unbundle By Name(w3339) -> ("phandle out"=w3347:u32, "Axis"=w3346:enum16{"X", "Y", "X+Y"}[])
            n593 = for {
              tunnel: w3347 -> [w3351]
              tunnel: w3346 -> [w3350] mode=indexing
              shift-right: [w3348] -> _
              shift-left: w3345 -> [w3349]
              n594 = case shown="\"X+Y\"" w3350 {
                selector: w3350 -> [_ w3363]
                tunnel: w3349 -> [w3355 w3366]
                tunnel: w3351 -> [w3354 w3365]
                tunnel: [w3352 w3362] -> w3348
                frame "X+Y" {
                  n595 = for {
                    tunnel: w3355 -> [w3359]
                    tunnel: w3354 -> [w3358]
                    tunnel: i32[] [0, 1] -> [w3357] mode=indexing
                    tunnel: [w3356] -> w3352
                    n596 = To Long Integer(number=w3357) -> (32bit integer=w3360:i32)
                    n597 = call "Z Aux Direct Singl Cancel.vi"("error in (no error)"=w3359, "imode"=2, "iaxis"=w3360, "handle"=w3358) -> ("error out"=w3356:errorcluster)  [unwired: 5 in, 2 out]
                  }
                }
                frame "X", "Y", Default {
                  n598 = To Long Integer(number=w3363) -> (32bit integer=w3364:i32)
                  n599 = call "Z Aux Direct Singl Cancel.vi"("error in (no error)"=w3366, "imode"=2, "iaxis"=w3364, "handle"=w3365) -> ("error out"=w3362:errorcluster)  [unwired: 5 in, 2 out]
                }
              }
            }
          }
          frame "Exit" {
            n600 = Flush Queue(queue=w3371, error in (no error)=w3372) -> (queue out=w3369:refnum<queue>, error out=w3370:errorcluster)  [unwired: 1 out]
            n601 = Unbundle By Name(w3374) -> ("phandle out"=w3373:u32)
            n602 = call "Z Aux Close.vi"("error in (no error)"=w3370, "handle"=w3373) -> ("error out"=w3375:errorcluster)  [unwired: 7 in, 2 out]
            n603 = Bundle By Name(cluster=w3374, "App State"="Exit") -> (w3378:T24)
            n604 = Enqueue Element(queue=w3369, element=cluster{"State":T17, "Variable":variant} {"State"=enum."Update", "Variable"=variant}, error in (no error)=w3375) -> ()  [unwired: 1 in, 3 out]
          }
        }
      }
      n605 = while {
        tunnel: w91 -> [w613]
        tunnel: w90 -> [w614]
        shift-right: [w611] -> _
        shift-left: w99 -> [w612]
        stop <- w608 stop-if-true
        n606 = local read "Cluster"() -> (w610:cluster{"tester  A":bool, " tester B":bool})
        n607 = Unbundle(w610) -> ("tester B"=w609:bool)  [unwired: 1 out]
        n608 = case shown="True" w609 {
          tunnel: w614 -> [_ w626]
          tunnel: w613 -> [_ w625]
          tunnel: w612 -> [w615 w619]
          tunnel: [w615 w618] -> w611
          tunnel: [_ w616] -> w608
          frame False {
          }
          frame True {
            n609 = Dequeue Element(queue=w625, error in (no error)=w626) -> (queue out=w622:refnum<queue>, element=w624:T19, error out=w621:errorcluster)  [unwired: 1 in, 1 out]
            n610 = property on="TCP?" class="Bool (strict)"() -> ("Value"=w617:bool)  [unwired: 2 in, 2 out]
            n611 = Unbundle(w624) -> (w623:T30, "variant"=w620:variant)
            n612 = case shown="\"Dynamic\"" w623 {
              tunnel: w622 -> [_ _ w635 _ w663 w747 w794 w834 _ w879 w888 w897 w906 w915 w924 w968 w1020 _ _ _ w1086]
              tunnel: w621 -> [_ _ w634 _ w664 w737 w783 w827 w860 w887 w896 w905 w914 w923 w932 w933 w1013 w1043 w1053 w1057 w1085]
              tunnel: w620 -> [_ _ w633 _ _ w735 w782 w825 w861 w886 w895 w904 w913 w922 w931 w971 w1023 w1048 w1054 _ _]
              tunnel: [_ _ _ _ _ _ _ _ _ _ _ _ _ _ _ _ _ _ _ TRUE _] -> w616
              tunnel: w619 -> [w627 w628 w631 w653 w660 w740 w786 w830 w865 w884 w893 w902 w911 w920 w930 w938 w1015 w1044 w1051 w1058 w1088]
              tunnel: [w627 w628 w630 w653 w662 w744 w791 w835 w865 w883 w892 w901 w910 w919 w929 w970 w1022 w1047 w1050 w1058 w1089] -> w618
              tunnel: w617 -> [_ _ _ _ w659 w738 w784 w823 w859 _ _ _ _ _ _ w935 w1014 _ _ w1056 w1083]
              frame "Idle", Default {
              }
              frame "Run" {
              }
              frame "auto mode" {
                n613 = Unbundle By Name(w631) -> ("auto test"=w632:bool)
                n614 = Not(x=w632) -> (.not. x?=w629:bool)
                n615 = case shown="True" w629 {
                  tunnel: w635 -> [_ w639]
                  tunnel: w634 -> [_ w638]
                  tunnel: w633 -> [_ w637]
                  frame False {
                  }
                  frame True {
                    n616 = Variant To Data(error in=w638, type=T10 {"Target 1"={"Boolean"=FALSE, "Speed"=0.0, "Range"=0.0, "Gain"=0.0}, "Target 2"={"Boolean"=FALSE, "Speed"=0.0, "Range"=0.0, "Gain"=0.0}, "Target 3"={"Boolean"=FALSE, "Speed"=0.0, "Range"=0.0, "Gain"=0.0}, "Target 4"={"Boolean"=FALSE, "Speed"=0.0, "Range"=0.0, "Gain"=0.0}} ("Direct program"), Variant=w637) -> (data=w643:T10, error out=w644:errorcluster)
                    n617 = Bundle By Name(cluster=T19 {enum."Direct Program", "variant"=variant}, "variant"=w643) -> (w642:T19)
                    n618 = Build Array (concatenate)(T19[] [{enum."Idle", "variant"=variant}, {enum."Freq. (GHz)", "variant"=variant}], w642, T19[] [{enum."Convert", "variant"=variant}, {enum."RF ON/OFF", "variant"=variant}]) -> (w640:T19[])
                    n619 = for {
                      tunnel: w639 -> [w649]
                      tunnel: w644 -> [w648]
                      tunnel: w640 -> [w647] mode=indexing
                      n620 = Enqueue Element(queue=w649, element=w647, error in (no error)=w648) -> ()  [unwired: 1 in, 3 out]
                    }
                  }
                }
                n621 = Bundle By Name(cluster=w631, "auto test"=w629) -> (w630:T15)
              }
              frame "Inst. Update" {
                n622 = Unbundle By Name(w653) -> ("Dynamic"=w654:T9, "Mapping"=w655:cluster{"4:4":bool, "4:2":bool, "4:1":bool}, "GRX (dB)"=w656:dbl, "GTX (dB)"=w658:dbl, "Freq. (GHz)"=w657:dbl, "Inst. Status"=w651:bool, "String"=→"String":string)
                n623 = property on="Freq. (GHz)" class="DigNum (strict)"("Value"=w657) -> ()  [unwired: 2 in, 2 out]
                n624 = property on="GTX (dB)" class="DigNum (strict)"("Value"=w658) -> ()  [unwired: 2 in, 2 out]
                n625 = property on="GRX (dB)" class="DigNum (strict)"("Value"=w656) -> ()  [unwired: 2 in, 2 out]
                n626 = property on="Mapping" class="Clust (strict)"("Value"=w655) -> ()  [unwired: 2 in, 2 out]
                n627 = property on="Dynamic2" class="Clust (strict)"("Value"=w654) -> ()  [unwired: 2 in, 2 out]
                n628 = local write "Inst. Status"(w651) -> ()
                n629 = Unbundle By Name(w653) -> ("Direct program"=w652:T10)
                n630 = property on="Direct program2" class="Clust (strict)"("Value"=w652) -> ()  [unwired: 2 in, 2 out]
              }
              frame "Inst. Connect" {
                n631 = Unbundle By Name(w660) -> ("Inst. Status"=w661:bool)
                n632 = case shown="False" w661 {
                  tunnel: w664 -> [_ w673]
                  tunnel: w663 -> [_ w666]
                  tunnel: w660 -> [w665 w670]
                  tunnel: [w665 w669] -> w662
                  tunnel: w659 -> [_ w667]
                  frame True {
                  }
                  frame False {
                    n633 = Empty String/Path?(string/path="Inst. Connect IP") -> (empty?=w674:bool)
                    n634 = case shown="False" w674 {
                      tunnel: "Inst. Connect IP" -> [w686 _]
                      tunnel: w673 -> [w677 w729]
                      tunnel: [w676 w729] -> w672
                      tunnel: w670 -> [w685 w728]
                      tunnel: [w684 w727] -> w669
                      tunnel: w667 -> [w678 _]
                      tunnel: w666 -> [w675 _]
                      frame False {
                        n635 = case shown="True" w678 {
                          tunnel: w686 -> [w691 w725]
                          tunnel: w677 -> [w692 w724]
                          tunnel: [w689 w718] -> w676
                          tunnel: [w688 w723] -> w683
                          tunnel: w675 -> [_ w720]
                          frame True {
                            n636 = Concatenate Strings("connect," ("string"), w691) -> (w690:string)
                            n637 = disable-structure shown="Enabled" {
                              disable-tunnel: w692 -> [w698 w716]
                              disable-tunnel: w690 -> [w697 w715]
                              disable-tunnel: [w695 w713] -> w689
                              disable-tunnel: [w694 w714] -> w687
                              frame Disabled {
                                (unwired) 1 ("return type")
                                n638 = call "client_FGV 2.vi"("data in"=w697, "error constant"=w698, "Enum"=enum16{"open", "idle", "write", "read", "close"}."write") -> ("error constant 2"=w696:errorcluster)  [unwired: 7 in, 1 out]
                                n639 = while {
                                tunnel: w696 -> [w703]
                                tunnel: [w701] -> w695
                                tunnel: [w700] -> w694
                                i -> [w705]
                                stop <- w707 stop-if-true
                                n640 = call "client_FGV 2.vi"("error constant"=w703, "Enum"=enum16{"open", "idle", "write", "read", "close"}."read") -> ("error constant 2"=w701:errorcluster, "data out"=w700:string)  [unwired: 8 in]
                                n641 = String Length(string=w700) -> (length=w709:i32)
                                n642 = Greater Than 0?(x=w709) -> (x > 0?=w708:bool)
                                n643 = Greater?(x=w705, y=600) -> (0:w706:bool)
                                n644 = Or(x=w706, y=w708) -> (x .or. y?=w707:bool)
                                n645 = Wait (ms)(milliseconds to wait=u32 100) -> ()  [unwired: 1 out]
                                }
                              }
                              frame Enabled {
                                n646 = call "client_sw.vi"("receive?"=TRUE, "data in"=w715, "error constant"=w716, "port"=u16 6540) -> ("error constant 2"=w713:errorcluster, "data out"=w714:string)  [unwired: 6 in]
                              }
                            }
                            n647 = Decimal String To Number(string=w687) -> (number=w688:i32)  [unwired: 2 in, 1 out]
                          }
                          frame False, Default {
                            n648 = dll-call lib="D:/0717/0717/Radar - 2015 32bit_autoqueue_angle_0319/Debug 2/Test_ARTS_1.dll" fn="?_connect@@YAHPAD@Z"(error in=w724, "serverIPaddr"=w725) -> (error out=w719:errorcluster, "return type"=w723:i32)  [unwired: 3 in, 1 out]
                            n649 = property on="Freq. (GHz)" class="DigNum (strict)"() -> ("Value"=w717:dbl)  [unwired: 2 in, 2 out]
                            n650 = Bundle By Name(cluster=T19 {enum."Freq. (GHz)", "variant"=variant}, "variant"=w717) -> (w721:T19)
                            n651 = Enqueue Element(queue=w720, element=w721, error in (no error)=w719) -> (error out=w718:errorcluster)  [unwired: 1 in, 2 out]
                          }
                        }
                        n652 = Greater Than 0?(x=w683) -> (x > 0?=w682:bool)
                        n653 = Select(t="connected" ("String"), s=w682, f="connect fail" ("String")) -> (s? t:f=w679:string)
                        n654 = Bundle By Name(cluster=w685, "Inst. Status"=w682, "String"=w679) -> (w684:T15)
                      }
                      frame True {
                        n655 = Bundle By Name(cluster=w728, "String"="connect fail") -> (w727:T15)
                      }
                    }
                    n656 = Enqueue Element(queue=w666, element=T19 {enum."Inst. Update", "variant"=variant}, error in (no error)=w672) -> ()  [unwired: 1 in, 3 out]
                  }
                }
              }
              frame "RF ON/OFF" {
                n657 = Variant To Data(error in=w737, type=TRUE, Variant=w735) -> (data=w733:bool, error out=w736:errorcluster)
                n658 = Unbundle By Name(w740) -> ("auto test"=w739:bool)
                n659 = Boolean To (0,1)(Boolean=w733) -> (0, 1=w741:i16)
                n660 = property on="RF ON/OFF" class="Bool (strict)"("Value"=w733) -> ()  [unwired: 2 in, 2 out]
                n661 = case shown="True" w738 {
                  tunnel: w736 -> [w754 w770]
                  tunnel: [w751 w769] -> w745
                  tunnel: [1 w768] -> w732
                  tunnel: w741 -> [w753 w767]
                  frame True {
                    n662 = Number To Decimal String(number=w753) -> (decimal integer string=w755:string)  [unwired: 1 in]
                    n663 = Concatenate Strings("rfon,", w755) -> (w752:string)
                    n664 = disable-structure shown="Enabled" {
                      disable-tunnel: w754 -> [w759 w765]
                      disable-tunnel: [w758 w762] -> w751
                      disable-tunnel: w752 -> [w757 w763]
                      disable-tunnel: [_ w761] -> _
                      frame Disabled {
                        n665 = call "client_FGV 2.vi"("data in"=w757, "error constant"=w759, "Enum"=enum16{"open", "idle", "write", "read", "close"}."write") -> ("error constant 2"=w758:errorcluster)  [unwired: 7 in, 1 out]
                      }
                      frame Enabled {
                        n666 = call "client_sw.vi"("receive?"=FALSE, "data in"=w763, "error constant"=w765, "port"=u16 6540) -> ("error constant 2"=w762:errorcluster, "data out"=w761:string)  [unwired: 6 in]
                      }
                    }
                  }
                  frame False, Default {
                    n667 = dll-call lib="D:/0717/0717/Radar - 2015 32bit_autoqueue_angle_0319/Debug 2/Test_ARTS_1.dll" fn="?_SetSynthRFOutput@@YAHH@Z"(error in=w770, "irfoutput"=w767) -> (error out=w769:errorcluster, "return type"=w768:i32)  [unwired: 3 in, 1 out]
                  }
                }
                n668 = Greater Than 0?(x=w732) -> (x > 0?=w743:bool)
                n669 = case shown="False" w743 {
                  tunnel: ["run fail" ("String") "run ok" ("String")] -> w742
                  frame False {
                  }
                  frame True {
                  }
                }
                n670 = property on="auto step finish?" class="Bool (strict)"() -> ("Value"=w730:bool)  [unwired: 2 in, 2 out]
                n671 = Bundle By Name(cluster=w740, "String"=w742) -> (w744:T15)
                n672 = Not(x=w730) -> (.not. x?=w731:bool)
                n673 = case shown="False" w739 {
                  tunnel: w747 -> [w773 w776]
                  tunnel: T19 {enum."Inst. Update", "variant"=variant} -> [w771 w775]
                  tunnel: w745 -> [w772 w774]
                  frame True {
                    n674 = Enqueue Element At Opposite End(queue=w773, element=w771, error in (no error)=w772) -> ()  [unwired: 1 in, 3 out]
                  }
                  frame False {
                    n675 = Enqueue Element(queue=w776, element=w775, error in (no error)=w774) -> ()  [unwired: 1 in, 3 out]
                  }
                }
                n676 = case shown="True" w731 {
                  tunnel: w732 -> [_ w748]
                  frame False {
                  }
                  frame True {
                    n677 = Greater Than 0?(x=w748) -> (x > 0?=w749:bool)
                    n678 = property on="autoRs2finish?" class="Bool (strict)"("Value"=w749) -> ()  [unwired: 2 in, 2 out]
                  }
                }
              }
              frame "Convert" {
                n679 = Variant To Data(error in=w783, type=TRUE, Variant=w782) -> (data=w779:bool, error out=w780:errorcluster)
                n680 = Unbundle By Name(w786) -> ("auto test"=w785:bool)
                n681 = Boolean To (0,1)(Boolean=w779) -> (0, 1=w787:i16)
                n682 = property on="T/R Converters" class="Bool (strict)"("Value"=w779) -> ()  [unwired: 2 in, 2 out]
                n683 = case shown="True" w784 {
                  tunnel: w780 -> [w797 w813]
                  tunnel: [w798 w812] -> w792
                  tunnel: [1 ("return type") w811] -> w789
                  tunnel: w787 -> [w796 w810]
                  frame True {
                    n684 = Number To Decimal String(number=w796) -> (decimal integer string=w801:string)  [unwired: 1 in]
                    n685 = Concatenate Strings("convert,", w801) -> (w795:string)
                    n686 = disable-structure shown="Enabled" {
                      disable-tunnel: [w804 w807] -> w798
                      disable-tunnel: w797 -> [w803 w808]
                      disable-tunnel: w795 -> [w802 w806]
                      frame Disabled {
                        n687 = call "client_FGV 2.vi"("data in"=w802, "error constant"=w803, "Enum"=enum16{"open", "idle", "write", "read", "close"}."write") -> ("error constant 2"=w804:errorcluster)  [unwired: 7 in, 1 out]
                      }
                      frame Enabled {
                        n688 = call "client_sw.vi"("data in"=w806, "error constant"=w808, "port"=u16 6540) -> ("error constant 2"=w807:errorcluster)  [unwired: 7 in, 1 out]
                      }
                    }
                  }
                  frame False, Default {
                    n689 = dll-call lib="D:/0717/0717/Radar - 2015 32bit_autoqueue_angle_0319/Debug 2/Test_ARTS_1.dll" fn="?_SetTrEn@@YAHH@Z"(error in=w813, "ienable"=w810) -> (error out=w812:errorcluster, "return type"=w811:i32)  [unwired: 3 in, 1 out]
                  }
                }
                n690 = Greater Than 0?(x=w789) -> (x > 0?=w790:bool)
                n691 = case shown="True" w790 {
                  tunnel: ["run fail" ("String") "convert ok" ("String")] -> w788
                  frame False {
                  }
                  frame True {
                  }
                }
                n692 = Bundle By Name(cluster=w786, "String"=w788) -> (w791:T15)
                n693 = case shown="False" w785 {
                  tunnel: w794 -> [w816 w819]
                  tunnel: T19 {enum."Inst. Update", "variant"=variant} -> [w814 w818]
                  tunnel: w792 -> [w815 w817]
                  frame True {
                    n694 = Enqueue Element At Opposite End(queue=w816, element=w814, error in (no error)=w815) -> ()  [unwired: 1 in, 3 out]
                  }
                  frame False {
                    n695 = Enqueue Element(queue=w819, element=w818, error in (no error)=w817) -> ()  [unwired: 1 in, 3 out]
                  }
                }
              }
              frame "Freq. (GHz)" {
                n696 = Variant To Data(error in=w827, type=0.0, Variant=w825) -> (data=w822:dbl, error out=w826:errorcluster)
                n697 = Unbundle By Name(w830) -> ("auto test"=w828:bool)
                n698 = Multiply(x=w822, y=1000.0) -> (x*y=w831:dbl)
                n699 = case shown="True" w823 {
                  tunnel: [w839 w852] -> w833
                  tunnel: w831 -> [_ w851]
                  tunnel: w826 -> [w838 w850]
                  tunnel: w822 -> [w837 _]
                  frame True {
                    n700 = Number To Fractional String(number=w837) -> (F-format string=w840:string)  [unwired: 3 in]
                    n701 = Concatenate Strings("freq," ("string"), w840) -> (w836:string)
                    n702 = disable-structure shown="Enabled" {
                      disable-tunnel: [w844 w847] -> w839
                      disable-tunnel: w838 -> [w843 w848]
                      disable-tunnel: w836 -> [w842 w846]
                      frame Disabled {
                        n703 = call "client_FGV 2.vi"("data in"=w842, "error constant"=w843, "Enum"=enum16{"open", "idle", "write", "read", "close"}."write") -> ("error constant 2"=w844:errorcluster)  [unwired: 7 in, 1 out]
                      }
                      frame Enabled {
                        n704 = call "client_sw.vi"("data in"=w846, "error constant"=w848, "port"=u16 6540) -> ("error constant 2"=w847:errorcluster)  [unwired: 7 in, 1 out]
                      }
                    }
                  }
                  frame False, Default {
                    n705 = dll-call lib="D:/0717/0717/Radar - 2015 32bit_autoqueue_angle_0319/Debug 2/Test_ARTS_1.dll" fn="?_SetRfFreq_kHz@@YAHH@Z" label="SetRfFreq"(error in=w850, "ichan"=w851) -> (error out=w852:errorcluster)  [unwired: 4 in, 1 out]
                  }
                }
                n706 = Bundle By Name(cluster=w830, "Freq. (GHz)"=w822) -> (w835:T15)
                n707 = case shown="True" w828 {
                  tunnel: w834 -> [w855 w858]
                  tunnel: w833 -> [w854 w857]
                  tunnel: T19 {enum."Inst. Update", "variant"=variant} -> [w853 w856]
                  frame True {
                    n708 = Enqueue Element At Opposite End(queue=w855, element=w853, error in (no error)=w854) -> ()  [unwired: 1 in, 3 out]
                  }
                  frame False {
                    n709 = Enqueue Element(queue=w858, element=w856, error in (no error)=w857) -> ()  [unwired: 1 in, 3 out]
                  }
                }
              }
              frame "rx att" {
                n710 = Variant To Data(error in=w860, type=0.0, Variant=w861) -> (data=w863:dbl, error out=w862:errorcluster)
                n711 = case shown="True" w859 {
                  tunnel: w863 -> [w868 w878]
                  tunnel: w862 -> [w867 w877]
                  frame True {
                    n712 = Number To Fractional String(number=w868) -> (F-format string=w869:string)  [unwired: 3 in]
                    n713 = Concatenate Strings("rxatt," ("string"), w869) -> (w866:string)
                    n714 = disable-structure shown="Enabled" {
                      disable-tunnel: w867 -> [w872 w875]
                      disable-tunnel: w866 -> [w871 w874]
                      frame Disabled {
                        n715 = call "client_FGV 2.vi"("data in"=w871, "error constant"=w872, "Enum"=enum16{"open", "idle", "write", "read", "close"}."write") -> ()  [unwired: 7 in, 2 out]
                      }
                      frame Enabled {
                        n716 = call "client_sw.vi"("data in"=w874, "error constant"=w875, "port"=u16 6540) -> ()  [unwired: 7 in, 2 out]
                      }
                    }
                  }
                  frame False, Default {
                    n717 = dll-call lib="D:/0717/0717/Radar - 2015 32bit_autoqueue_angle_0319/Debug 2/Test_ARTS_1.dll" fn="?_SetRxAttn@@YAHN@Z" label="_SetRxAttn"(error in=w877, "irxatt"=w878) -> ()  [unwired: 4 in, 2 out]
                  }
                }
              }
              frame "GTX (dB)" {
                n718 = Variant To Data(error in=w887, type=0.0, Variant=w886) -> (data=w882:dbl, error out=w880:errorcluster)
                n719 = Bundle By Name(cluster=w884, "GTX (dB)"=w882) -> (w883:T15)
                n720 = Enqueue Element(queue=w879, element=T19 {enum."Inst. Update", "variant"=variant}, error in (no error)=w880) -> ()  [unwired: 1 in, 3 out]
              }
              frame "GRX (dB)" {
                n721 = Variant To Data(error in=w896, type=0.0, Variant=w895) -> (data=w891:dbl, error out=w889:errorcluster)
                n722 = Bundle By Name(cluster=w893, "GRX (dB)"=w891) -> (w892:T15)
                n723 = Enqueue Element(queue=w888, element=T19 {enum."Inst. Update", "variant"=variant}, error in (no error)=w889) -> ()  [unwired: 1 in, 3 out]
              }
              frame "Range Trim(m)" {
                n724 = Variant To Data(error in=w905, type=0.0, Variant=w904) -> (data=w900:dbl, error out=w898:errorcluster)
                n725 = Bundle By Name(cluster=w902, "Range Trim (m)"=w900) -> (w901:T15)
                n726 = Enqueue Element(queue=w897, element=T19 {enum."Inst. Update", "variant"=variant}, error in (no error)=w898) -> ()  [unwired: 1 in, 3 out]
              }
              frame "Gain Trim (dB)" {
                n727 = Variant To Data(error in=w914, type=0.0, Variant=w913) -> (data=w909:dbl, error out=w907:errorcluster)
                n728 = Bundle By Name(cluster=w911, "Gain Trim (dB)"=w909) -> (w910:T15)
                n729 = Enqueue Element(queue=w906, element=T19 {enum."Inst. Update", "variant"=variant}, error in (no error)=w907) -> ()  [unwired: 1 in, 3 out]
              }
              frame "Distance to RUT" {
                n730 = Variant To Data(error in=w923, type=0.0, Variant=w922) -> (data=w918:dbl, error out=w916:errorcluster)
                n731 = Bundle By Name(cluster=w920, "Distance to RUT"=w918) -> (w919:T15)
                n732 = Enqueue Element(queue=w915, element=T19 {enum."Inst. Update", "variant"=variant}, error in (no error)=w916) -> ()  [unwired: 1 in, 3 out]
              }
              frame "Mapping" {
                n733 = Variant To Data(error in=w932, type=cluster{"4:4":bool, "4:2":bool, "4:1":bool} {"4:4"=FALSE, "4:2"=FALSE, "4:1"=FALSE} ("Mapping"), Variant=w931) -> (data=w928:cluster{"4:4":bool, "4:2":bool, "4:1":bool}, error out=w925:errorcluster)
                n734 = Bundle By Name(cluster=w930, "Mapping"=w928) -> (w929:T15)
                n735 = Enqueue Element(queue=w924, element=T19 {enum."Inst. Update", "variant"=variant}, error in (no error)=w925) -> ()  [unwired: 1 in, 3 out]
              }
              frame "Direct Program" {
                n736 = Unbundle By Name(w938) -> ("auto test"=w937:bool)
                n737 = Variant To Data(error in=w933, type=T10 {"Target 1"={"Boolean"=FALSE, "Speed"=0.0, "Range"=0.0, "Gain"=0.0}, "Target 2"={"Boolean"=FALSE, "Speed"=0.0, "Range"=0.0, "Gain"=0.0}, "Target 3"={"Boolean"=FALSE, "Speed"=0.0, "Range"=0.0, "Gain"=0.0}, "Target 4"={"Boolean"=FALSE, "Speed"=0.0, "Range"=0.0, "Gain"=0.0}} ("Direct program"), Variant=w971) -> (data=w936:T10, error out=w966:errorcluster)
                n738 = Unbundle(w936) -> ("Target 1"=w964:T31, "Target 2"=w963:T31, "Target 3"=w962:T31, "Target 4"=w961:T31)
                n739 = Bundle By Name(cluster=w938, "Direct program"=w936) -> (w970:T15)
                n740 = Unbundle(w964) -> ("Boolean"=w944:bool, "Speed"=w960:dbl, "Range"=w959:dbl, "Gain"=w958:dbl)
                n741 = Unbundle(w963) -> ("Boolean"=w943:bool, "Speed"=w957:dbl, "Range"=w956:dbl, "Gain"=w955:dbl)
                n742 = Unbundle(w962) -> ("Boolean"=w942:bool, "Speed"=w954:dbl, "Range"=w953:dbl, "Gain"=w952:dbl)
                n743 = Unbundle(w961) -> ("Boolean"=w941:bool, "Speed"=w951:dbl, "Range"=w950:dbl, "Gain"=w949:dbl)
                n744 = Build Array(w944, w943, w942, w941) -> (w946:bool[])
                n745 = property on="auto step finish?" class="Bool (strict)"(error in=w933) -> ("Value"=w934:bool)  [unwired: 1 in, 2 out]
                n746 = Boolean To (0,1)(Boolean=w946) -> (0, 1=w945:i16[])
                n747 = Multiply(x=w945, y=i32[] [1, 2, 4, 8]) -> (x*y=w947:i32[])
                n748 = case shown="False" w934 {
                  frame False {
                    n749 = property on="autoRs2finish?" class="Bool (strict)"("Value"=FALSE ("autoRS")) -> ()  [unwired: 2 in, 2 out]
                  }
                  frame True {
                  }
                }
                n750 = Add Array Elements(numeric array=w947) -> (sum=w940:i32)
                n751 = case shown="False" w935 {
                  tunnel: w966 -> [w1003 w1006]
                  tunnel: [w1003 w1005] -> w965
                  tunnel: w940 -> [_ w1004]
                  frame True {
                  }
                  frame False, Default {
                    n752 = dll-call lib="D:/0717/0717/Radar - 2015 32bit_autoqueue_angle_0319/Debug 2/Test_ARTS_1.dll" fn="?_TxChanEnable@@YAHH@Z" label="TxChanEnable"(error in=w1006, "ichan"=w1004) -> (error out=w1005:errorcluster)  [unwired: 4 in, 1 out]
                  }
                }
                n753 = case shown="True" w935 {
                  tunnel: w965 -> [w977 w1002]
                  tunnel: w960 -> [_ w1001]
                  tunnel: w959 -> [_ w1000]
                  tunnel: w958 -> [_ w999]
                  tunnel: w957 -> [_ w998]
                  tunnel: w956 -> [_ w997]
                  tunnel: w955 -> [_ w996]
                  tunnel: w954 -> [_ w995]
                  tunnel: w953 -> [_ w994]
                  tunnel: w952 -> [_ w993]
                  tunnel: w951 -> [_ w992]
                  tunnel: w950 -> [_ w991]
                  tunnel: w949 -> [_ w990]
                  tunnel: [w976 w989] -> w939
                  tunnel: w936 -> [w975 _]
                  frame True {
                    n754 = call "Untitled 3.vi"("Boolean"=TRUE, "Direct program"=w975) -> ("concatenated string"=w979:string)  [unwired: 8 in, 1 out]
                    n755 = Concatenate Strings("static," ("string"), w979) -> (w974:string)
                    n756 = disable-structure shown="Enabled" {
                      disable-tunnel: w977 -> [w982 w987]
                      disable-tunnel: [w981 w986] -> w976
                      disable-tunnel: w974 -> [w980 w985]
                      frame Disabled {
                        n757 = call "client_FGV 2.vi"("data in"=w980, "error constant"=w982, "Enum"=enum16{"open", "idle", "write", "read", "close"}."write") -> ("error constant 2"=w981:errorcluster)  [unwired: 7 in, 1 out]
                      }
                      frame Enabled {
                        n758 = call "client_sw.vi"("receive?"=TRUE, "data in"=w985, "error constant"=w987, "port"=u16 6540) -> ("error constant 2"=w986:errorcluster)  [unwired: 6 in, 1 out]
                      }
                    }
                  }
                  frame False, Default {
                    n759 = dll-call lib="D:/0717/0717/Radar - 2015 32bit_autoqueue_angle_0319/Debug 2/Test_ARTS_1.dll" fn="?_SetTxChanStaticCfg@@YAHHHHHHHHHHHHH@Z" label="SetTxChanStaticCfg"(error in=w1002, "speed1"=w1001, "range1"=w1000, "gain1"=w999, "speed2"=w998, "range2"=w997, "gain2"=w996, "speed3"=w995, "range3"=w994, "gain3"=w993, "speed4"=w992, "range4"=w991, "gain4"=w990) -> (error out=w989:errorcluster)  [unwired: 15 in, 1 out]
                  }
                }
                n760 = case shown="False" w937 {
                  tunnel: T19 {enum."Inst. Update", "variant"=variant} -> [w1007 w1012]
                  tunnel: w968 -> [w1009 w1011]
                  tunnel: w939 -> [w1008 w1010]
                  frame True {
                    n761 = Enqueue Element At Opposite End(queue=w1009, element=w1007, error in (no error)=w1008) -> ()  [unwired: 1 in, 3 out]
                  }
                  frame False {
                    n762 = Enqueue Element(queue=w1011, element=w1012, error in (no error)=w1010) -> ()  [unwired: 1 in, 3 out]
                  }
                }
              }
              frame "Dynamic" {
                n763 = Variant To Data(error in=w1013, type=T9 {"Target 1"={"Boolean"=FALSE, "Start Speed (km/h)"=0.0, "Stop Speed (km/h)"=0.0, "Start Range(m)"=0.0, "Stop Range(m)"=0.0, "Start Gain(dB)"=0.0}, "Target 2"={"Boolean"=FALSE, "Start Speed (km/h)"=0.0, "Stop Speed (km/h)"=0.0, "Start Range(m)"=0.0, "Stop Range(m)"=0.0, "Start Gain(dB)"=0.0}, "Target 3"={"Boolean"=FALSE, "Start Speed (km/h)"=0.0, "Stop Speed (km/h)"=0.0, "Start Range(m)"=0.0, "Stop Range(m)"=0.0, "Start Gain(dB)"=0.0}, "Target 4"={"Boolean"=FALSE, "Start Speed (km/h)"=0.0, "Stop Speed (km/h)"=0.0, "Start Range(m)"=0.0, "Stop Range(m)"=0.0, "Start Gain(dB)"=0.0}} ("Dynamic"), Variant=w1023) -> (data=w1016:T9, error out=w1017:errorcluster)
                n764 = Bundle By Name(cluster=w1015, "Dynamic"=w1016) -> (w1022:T15)
                n765 = case shown="True" w1014 {
                  tunnel: [w1029 w1040] -> w1018
                  tunnel: w1016 -> [w1026 w1042]
                  tunnel: w1017 -> [w1024 w1041]
                  frame True {
                    n766 = call "dynamic.vi"("Boolean"=TRUE, "dynamic"=w1026) -> ("concatenated string"=w1025:string)  [unwired: 8 in, 1 out]
                    n767 = Concatenate Strings("dynamic," ("string"), w1025) -> (w1028:string)
                    n768 = disable-structure shown="Enabled" {
                      disable-tunnel: [w1033 w1035] -> w1029
                      disable-tunnel: w1028 -> [w1032 w1037]
                      disable-tunnel: w1024 -> [w1031 w1036]
                      frame Disabled {
                        n769 = call "client_FGV 2.vi"("data in"=w1032, "error constant"=w1031, "Enum"=enum16{"open", "idle", "write", "read", "close"}."write") -> ("error constant 2"=w1033:errorcluster)  [unwired: 7 in, 1 out]
                      }
                      frame Enabled {
                        n770 = call "client_sw.vi"("data in"=w1037, "error constant"=w1036, "port"=u16 6540) -> ("error constant 2"=w1035:errorcluster)  [unwired: 7 in, 1 out]
                      }
                    }
                  }
                  frame False {
                    n771 = call "dynamicsub.vi"("error in (no error)"=w1041, "Dynamic"=w1042) -> ("error out"=w1040:errorcluster, "generateWF ok?"=→"generateWF ok? 2":i32)  [unwired: 8 in]
                  }
                }
                n772 = Enqueue Element(queue=w1020, element=T19 {enum."Inst. Update", "variant"=variant}, error in (no error)=w1018) -> ()  [unwired: 1 in, 3 out]
              }
              frame "dyset" {
                n773 = Variant To Data(error in=w1043, type=T9 {"Target 1"={"Boolean"=FALSE, "Start Speed (km/h)"=0.0, "Stop Speed (km/h)"=0.0, "Start Range(m)"=0.0, "Stop Range(m)"=0.0, "Start Gain(dB)"=0.0}, "Target 2"={"Boolean"=FALSE, "Start Speed (km/h)"=0.0, "Stop Speed (km/h)"=0.0, "Start Range(m)"=0.0, "Stop Range(m)"=0.0, "Start Gain(dB)"=0.0}, "Target 3"={"Boolean"=FALSE, "Start Speed (km/h)"=0.0, "Stop Speed (km/h)"=0.0, "Start Range(m)"=0.0, "Stop Range(m)"=0.0, "Start Gain(dB)"=0.0}, "Target 4"={"Boolean"=FALSE, "Start Speed (km/h)"=0.0, "Stop Speed (km/h)"=0.0, "Start Range(m)"=0.0, "Stop Range(m)"=0.0, "Start Gain(dB)"=0.0}} ("Dynamic"), Variant=w1048) -> (data=w1045:T9)  [unwired: 1 out]
                n774 = Bundle By Name(cluster=w1044, "Dynamic"=w1045) -> (w1047:T15)
              }
              frame "£m Data" {
                n775 = Variant To Data(error in=w1053, type=dbl[][] [], Variant=w1054) -> (data=w1049:dbl[][])  [unwired: 1 out]
                n776 = Bundle By Name(cluster=w1051, "£m Data"=w1049) -> (w1050:T15)
              }
              frame "Exit" {
                n777 = case shown="True" w1056 {
                  tunnel: w1057 -> [w1060 w1081]
                  tunnel: [w1067 w1079] -> w1055
                  frame True {
                    n778 = Number To Decimal String(number=0 ("return type")) -> (decimal integer string=w1066:string)  [unwired: 1 in]
                    n779 = Concatenate Strings("rfon,", w1066) -> (w1064:string)
                    n780 = call "client_sw.vi"("data in"=w1064, "error constant"=w1060, "port"=u16 6540) -> ("error constant 2"=w1061:errorcluster)  [unwired: 7 in, 1 out]
                    n781 = Concatenate Strings("close," ("string"), "ok" ("string")) -> (w1068:string)
                    n782 = disable-structure shown="Enabled" {
                      disable-tunnel: w1061 -> [w1073 w1077]
                      disable-tunnel: w1068 -> [w1072 w1075]
                      disable-tunnel: [w1071 w1076] -> w1067
                      frame Disabled {
                        n783 = call "client_FGV 2.vi"("data in"=w1072, "error constant"=w1073, "Enum"=enum16{"open", "idle", "write", "read", "close"}."write") -> ("error constant 2"=w1071:errorcluster)  [unwired: 7 in, 1 out]
                      }
                      frame Enabled {
                        n784 = call "client_sw.vi"("data in"=w1075, "error constant"=w1077, "port"=u16 6540) -> ("error constant 2"=w1076:errorcluster)  [unwired: 7 in, 1 out]
                      }
                    }
                  }
                  frame False {
                    n785 = dll-call lib="D:/0717/0717/Radar - 2015 32bit_autoqueue_angle_0319/Debug 2/Test_ARTS_1.dll" fn="?_SetSynthRFOutput@@YAHH@Z"(error in=w1081, "irfoutput"=0) -> (error out=w1082:errorcluster)  [unwired: 4 in, 1 out]
                    n786 = dll-call lib="D:/0717/0717/Radar - 2015 32bit_autoqueue_angle_0319/Debug 2/Test_ARTS_1.dll" fn="?_disconnect@@YAHXZ"(error in=w1082) -> (error out=w1079:errorcluster)  [unwired: 3 in, 1 out]
                  }
                }
                n787 = call <vilib>:"Clear Errors.vi"("error in (no error)"=w1055) -> ()  [unwired: 5 in, 2 out]
              }
              frame "Stop" {
                n788 = case shown="True" w1083 {
                  tunnel: w1085 -> [w1093 w1106]
                  tunnel: [w1092 w1104] -> w1084
                  frame True {
                    n789 = Concatenate Strings("close," ("string"), "ok" ("string")) -> (w1091:string)
                    n790 = disable-structure shown="Enabled" {
                      disable-tunnel: w1093 -> [w1098 w1102]
                      disable-tunnel: [w1097 w1101] -> w1092
                      disable-tunnel: w1091 -> [w1096 w1100]
                      frame Disabled {
                        n791 = call "client_FGV 2.vi"("data in"=w1096, "error constant"=w1098, "Enum"=enum16{"open", "idle", "write", "read", "close"}."write") -> ("error constant 2"=w1097:errorcluster)  [unwired: 7 in, 1 out]
                      }
                      frame Enabled {
                        n792 = call "client_sw.vi"("data in"=w1100, "error constant"=w1102, "port"=u16 6540) -> ("error constant 2"=w1101:errorcluster)  [unwired: 7 in, 1 out]
                      }
                    }
                  }
                  frame False {
                    n793 = dll-call lib="D:/0717/0717/Radar - 2015 32bit_autoqueue_angle_0319/Debug 2/Test_ARTS_1.dll" fn="?_SetSynthRFOutput@@YAHH@Z"(error in=w1106, "irfoutput"=0) -> (error out=w1107:errorcluster)  [unwired: 4 in, 1 out]
                    n794 = dll-call lib="D:/0717/0717/Radar - 2015 32bit_autoqueue_angle_0319/Debug 2/Test_ARTS_1.dll" fn="?_disconnect@@YAHXZ"(error in=w1107) -> (error out=w1104:errorcluster)  [unwired: 3 in, 1 out]
                  }
                }
                n795 = Bundle By Name(cluster=w1088, "Inst. Status"=FALSE) -> (w1089:T15)
                n796 = Enqueue Element(queue=w1086, element=T19 {enum."Inst. Update", "variant"=variant}, error in (no error)=w1084) -> ()  [unwired: 1 in, 3 out]
              }
            }
          }
        }
      }
      n797 = while {
        tunnel: w90 -> [w139]
        tunnel: w92 -> [w138]
        tunnel: w92 -> [w134]
        stop <- TRUE stop-if-true
        n798 = Dequeue Element(queue=w138, error in (no error)=w139) -> (element=w140:T21, error out=w135:errorcluster)  [unwired: 1 in, 2 out]
        n799 = Unbundle(w140) -> ("Enum"=w137:T32, "Variable"=w136:variant)
        n800 = case shown="\"INIT\"" w137 {
          tunnel: w136 -> [_ _ _ w274 _ _ _]
          tunnel: w135 -> [w152 w168 w182 w277 w327 w402 _]
          tunnel: [_ _ _ _ _ TRUE _] -> _
          tunnel: w134 -> [_ _ _ _ _ _ _]
          tunnel: [_ _ w177 w270 w322 _ _] -> w131
          frame "INIT" {
            n801 = flat-sequence {
              tunnel: [w163] -> w153
              tunnel: w152 -> [w163]
              frame #0 {
                n802 = property on="read buffer" class="Str"("Value"="" ("read buffer")) -> ()  [unwired: 2 in, 2 out]
              }
            }
            n803 = call "GPIB_func.vi"("error in (no error)"=w153, "Enum"=T16."INIT", "VISA resource name"="VISA GPIB Resource") -> ("error out"=w157:errorcluster)  [unwired: 7 in, 1 out]
            n804 = Concatenate Strings("*IDN?" ("write buffer"), "\r") -> (w155:string)
            n805 = call "GPIB_func.vi"("error in (no error)"=w157, "write buffer"=w155, "Enum"=T16."Query") -> ("error out"=w146:errorcluster, "read buffer"=w148:string)  [unwired: 7 in]
            n806 = property on="read buffer" class="Str"("Value"=w148) -> ()  [unwired: 2 in, 2 out]
            n807 = flat-sequence {
              tunnel: [w161] -> w145
              tunnel: w146 -> [w161]
              frame #0 {
                n808 = property on="big angle" class="Str"("Value"="90" ("big abgle")) -> ()  [unwired: 2 in, 2 out]
                n809 = Wait (ms)(milliseconds to wait=u32 100) -> ()  [unwired: 1 out]
              }
            }
            n810 = property on="origin" class="DigNum (strict)"() -> ("Value"=w144:dbl)  [unwired: 2 in, 2 out]
            n811 = Number To Decimal String(number=w144) -> (decimal integer string=w142:string)  [unwired: 1 in]
            n812 = Concatenate Strings("TMV," ("write buffer"), w142) -> (w141:string)
            n813 = call "GPIB_func.vi"("error in (no error)"=w145, "write buffer"=w141, "Enum"=T16."Query") -> ("read buffer"=w151:string)  [unwired: 7 in, 1 out]
            n814 = property on="read buffer" class="Str"("Value"=w151) -> ()  [unwired: 2 in, 2 out]
          }
          frame "READ" {
            n815 = property on="read buffer" class="Str"() -> ("Value"=w167:string)  [unwired: 2 in, 2 out]
            n816 = call "GPIB_func.vi"("error in (no error)"=w168, "Enum"=T16."READ") -> ("read buffer"=w165:string)  [unwired: 8 in, 1 out]
            "big abgle" <- w165
            n817 = Concatenate Strings(w167, w165) -> (w166:string)
            n818 = property on="read buffer" class="Str"("Value"=w166) -> ()  [unwired: 2 in, 2 out]
          }
          frame "ADD" {
            n819 = property on="big angle" class="Str"() -> ("Value"=w180:string)  [unwired: 2 in, 2 out]
            n820 = property on="angle" class="Enum (strict)"() -> ("Value"=w181:T13)  [unwired: 2 in, 2 out]
            n821 = case shown="\"30\"" w181 {
              tunnel: ["0" w225 w231 w237 w243 w249 w254 w259] -> w172
              tunnel: w180 -> [_ w224 w230 w236 w242 w248 w253 w258]
              tunnel: [60 ("y") 10 ("y") 20 ("y") 20 ("y") 50 ("y") w247 w252 30 ("y")] -> w169
              frame "0", Default {
              }
              frame "1" {
                n822 = Decimal String To Number(string=w224) -> (number=w228:i32)  [unwired: 2 in, 1 out]
                n823 = Add(x=w228, y=1) -> (x+y=w226:i32)
                n824 = Number To Decimal String(number=w226) -> (decimal integer string=w225:string)  [unwired: 1 in]
              }
              frame "5" {
                n825 = Decimal String To Number(string=w230) -> (number=w234:i32)  [unwired: 2 in, 1 out]
                n826 = Add(x=w234, y=5) -> (x+y=w232:i32)
                n827 = Number To Decimal String(number=w232) -> (decimal integer string=w231:string)  [unwired: 1 in]
              }
              frame "10" {
                n828 = Decimal String To Number(string=w236) -> (number=w240:i32)  [unwired: 2 in, 1 out]
                n829 = Add(x=w240, y=10) -> (x+y=w238:i32)
                n830 = Number To Decimal String(number=w238) -> (decimal integer string=w237:string)  [unwired: 1 in]
              }
              frame "30" {
                n831 = Decimal String To Number(string=w242) -> (number=w246:i32)  [unwired: 2 in, 1 out]
                n832 = Add(x=w246, y=30) -> (x+y=w244:i32)
                n833 = Number To Decimal String(number=w244) -> (decimal integer string=w243:string)  [unwired: 1 in]
              }
              frame "60" {
                w247 = 60 ("y")
                n834 = Decimal String To Number(string=w248) -> (number=w251:i32)  [unwired: 2 in, 1 out]
                n835 = Add(x=w251, y=w247) -> (x+y=w250:i32)
                n836 = Number To Decimal String(number=w250) -> (decimal integer string=w249:string)  [unwired: 1 in]
              }
              frame "90" {
                w252 = 90 ("y")
                n837 = Decimal String To Number(string=w253) -> (number=w256:i32)  [unwired: 2 in, 1 out]
                n838 = Add(x=w256, y=w252) -> (x+y=w255:i32)
                n839 = Number To Decimal String(number=w255) -> (decimal integer string=w254:string)  [unwired: 1 in]
              }
              frame "180" {
                n840 = Decimal String To Number(string=w258) -> (number=w262:i32)  [unwired: 2 in, 1 out]
                n841 = Add(x=w262, y=1) -> (x+y=w260:i32)
                n842 = Number To Decimal String(number=w260) -> (decimal integer string=w259:string)  [unwired: 1 in]
              }
            }
            n843 = Match Pattern(string=w172, regular expression="-") -> (offset past match=w174:i32)  [unwired: 1 in, 3 out]
            n844 = Fract/Exp String To Number(string=w172) -> (number=w176:dbl)  [unwired: 3 in, 1 out]
            n845 = Greater Than 0?(x=w174) -> (x > 0?=w175:bool)
            n846 = Concatenate Strings("TMV," ("write buffer"), w172, "\r\n") -> (w183:string)
            n847 = case shown="True" w175 {
              tunnel: w172 -> [w217 w220]
              tunnel: [w217 w218] -> w170
              frame False {
              }
              frame True {
                n848 = String Subset(string=w220, offset (0)=1) -> (substring=w218:string)  [unwired: 1 in]
              }
            }
            n849 = Not Equal To 0?(x=w176) -> (x != 0?=w171:bool)
            n850 = call "GPIB_func.vi"("error in (no error)"=w182, "write buffer"=w183, "Enum"=T16."WRITE") -> ("error out"=w178:errorcluster)  [unwired: 7 in, 1 out]
            n851 = case shown="False" w171 {
              tunnel: w178 -> [w188 w204]
              tunnel: [w187 w203] -> w177
              tunnel: w170 -> [_ w202]
              tunnel: w169 -> [w186 w201]
              frame False {
                n852 = while {
                  tunnel: w188 -> [w199]
                  tunnel: [w191] -> w187
                  tunnel: w186 -> [w189]
                  i -> [w196]
                  stop <- w195 stop-if-true
                  n853 = Wait (ms)(milliseconds to wait=u32 500) -> ()  [unwired: 1 out]
                  n854 = call "GPIB_func.vi"("error in (no error)"=w199, "write buffer"="TCP?", "Enum"=T16."Query") -> ("read buffer"=w191:string)  [unwired: 7 in, 1 out]
                  n855 = Greater?(x=w196, y=w189) -> (0:w194:bool)
                  n856 = Match Pattern(string=w191, regular expression="000") -> (offset past match=w197:i32)  [unwired: 1 in, 3 out]
                  n857 = Greater Than 0?(x=w197) -> (x > 0?=w193:bool)
                  n858 = Or(x=w193, y=w194) -> (x .or. y?=w195:bool)
                }
              }
              frame True {
                n859 = while {
                  tunnel: w204 -> [w215]
                  tunnel: w202 -> [w213]
                  tunnel: [w206] -> w203
                  tunnel: w201 -> [w205]
                  i -> [w211]
                  stop <- w210 stop-if-true
                  n860 = Wait (ms)(milliseconds to wait=u32 500) -> ()  [unwired: 1 out]
                  n861 = call "GPIB_func.vi"("error in (no error)"=w215, "write buffer"="TCP?", "Enum"=T16."Query") -> ("read buffer"=w206:string)  [unwired: 7 in, 1 out]
                  n862 = Greater?(x=w211, y=w205) -> (0:w209:bool)
                  n863 = Match Pattern(string=w206, regular expression=w213) -> (offset past match=w212:i32)  [unwired: 1 in, 3 out]
                  n864 = Greater Than 0?(x=w212) -> (x > 0?=w208:bool)
                  n865 = Or(x=w208, y=w209) -> (x .or. y?=w210:bool)
                }
              }
            }
          }
          frame "WRITE" {
            n866 = Variant To Data(type=90.0, Variant=w274) -> (data=w272:dbl)  [unwired: 1 in, 1 out]
            n867 = Round To Nearest(number=w272) -> (nearest integer value=w271:dbl)
            n868 = Number To Fractional String(number=w271) -> (F-format string=w265:string)  [unwired: 3 in]
            n869 = Match Pattern(string=w265, regular expression="-") -> (offset past match=w267:i32)  [unwired: 1 in, 3 out]
            n870 = Greater Than 0?(x=w267) -> (x > 0?=w268:bool)
            n871 = case shown="True" w268 {
              tunnel: w265 -> [w311 w314]
              tunnel: [w311 w312] -> w263
              frame False {
              }
              frame True {
                n872 = String Subset(string=w314, offset (0)=1) -> (substring=w312:string)  [unwired: 1 in]
              }
            }
            n873 = Fract/Exp String To Number(string=w265) -> (number=w269:dbl)  [unwired: 3 in, 1 out]
            n874 = Concatenate Strings("TMV," ("write buffer"), w265, "\r\n") -> (w278:string)
            n875 = Not Equal To 0?(x=w269) -> (x != 0?=w264:bool)
            n876 = call "GPIB_func.vi"("error in (no error)"=w277, "write buffer"=w278, "Enum"=T16."WRITE") -> ("error out"=w275:errorcluster)  [unwired: 7 in, 1 out]
            n877 = case shown="False" w264 {
              tunnel: w275 -> [w283 w298]
              tunnel: [w281 w297] -> w270
              tunnel: w263 -> [w282 w296]
              frame False {
                n878 = while {
                  tunnel: w283 -> [w294]
                  tunnel: w282 -> [_]
                  tunnel: [w285] -> w281
                  i -> [w291]
                  stop <- w289 stop-if-true
                  n879 = Wait (ms)(milliseconds to wait=u32 500) -> ()  [unwired: 1 out]
                  n880 = call "GPIB_func.vi"("error in (no error)"=w294, "write buffer"="TCP?", "Enum"=T16."Query") -> ("read buffer"=w285:string)  [unwired: 7 in, 1 out]
                  n881 = Greater?(x=w291, y=20) -> (0:w288:bool)
                  n882 = Match Pattern(string=w285, regular expression="000") -> (offset past match=w292:i32)  [unwired: 1 in, 3 out]
                  n883 = Greater Than 0?(x=w292) -> (x > 0?=w287:bool)
                  n884 = Or(x=w287, y=w288) -> (x .or. y?=w289:bool)
                }
              }
              frame True {
                n885 = while {
                  tunnel: w298 -> [w309]
                  tunnel: w296 -> [w307]
                  tunnel: [w299] -> w297
                  i -> [w305]
                  stop <- w303 stop-if-true
                  n886 = Wait (ms)(milliseconds to wait=u32 500) -> ()  [unwired: 1 out]
                  n887 = call "GPIB_func.vi"("error in (no error)"=w309, "write buffer"="TCP?", "Enum"=T16."Query") -> ("read buffer"=w299:string)  [unwired: 7 in, 1 out]
                  n888 = Greater?(x=w305, y=20) -> (0:w302:bool)
                  n889 = Match Pattern(string=w299, regular expression=w307) -> (offset past match=w306:i32)  [unwired: 1 in, 3 out]
                  n890 = Greater Than 0?(x=w306) -> (x > 0?=w301:bool)
                  n891 = Or(x=w301, y=w302) -> (x .or. y?=w303:bool)
                }
              }
            }
          }
          frame "DEC" {
            n892 = property on="big angle" class="Str"() -> ("Value"=w325:string)  [unwired: 2 in, 2 out]
            n893 = property on="angle" class="Enum (strict)"() -> ("Value"=w326:T13)  [unwired: 2 in, 2 out]
            n894 = case shown="\"90\"" w326 {
              tunnel: ["0" w366 w371 w376 w381 w386 w391 w396] -> w317
              tunnel: w325 -> [_ w365 w370 w375 w380 w385 w390 w395]
              frame "0", Default {
              }
              frame "1" {
                n895 = Decimal String To Number(string=w365) -> (number=w369:i32)  [unwired: 2 in, 1 out]
                n896 = Subtract(x=w369, y=1) -> (x-y=w367:i32)
                n897 = Number To Decimal String(number=w367) -> (decimal integer string=w366:string)  [unwired: 1 in]
              }
              frame "5" {
                n898 = Decimal String To Number(string=w370) -> (number=w374:i32)  [unwired: 2 in, 1 out]
                n899 = Subtract(x=w374, y=5) -> (x-y=w372:i32)
                n900 = Number To Decimal String(number=w372) -> (decimal integer string=w371:string)  [unwired: 1 in]
              }
              frame "10" {
                n901 = Decimal String To Number(string=w375) -> (number=w379:i32)  [unwired: 2 in, 1 out]
                n902 = Subtract(x=w379, y=10) -> (x-y=w377:i32)
                n903 = Number To Decimal String(number=w377) -> (decimal integer string=w376:string)  [unwired: 1 in]
              }
              frame "30" {
                n904 = Decimal String To Number(string=w380) -> (number=w384:i32)  [unwired: 2 in, 1 out]
                n905 = Subtract(x=w384, y=30) -> (x-y=w382:i32)
                n906 = Number To Decimal String(number=w382) -> (decimal integer string=w381:string)  [unwired: 1 in]
              }
              frame "60" {
                n907 = Decimal String To Number(string=w385) -> (number=w389:i32)  [unwired: 2 in, 1 out]
                n908 = Subtract(x=w389, y=60) -> (x-y=w387:i32)
                n909 = Number To Decimal String(number=w387) -> (decimal integer string=w386:string)  [unwired: 1 in]
              }
              frame "90" {
                n910 = Decimal String To Number(string=w390) -> (number=w394:i32)  [unwired: 2 in, 1 out]
                n911 = Subtract(x=w394, y=90) -> (x-y=w392:i32)
                n912 = Number To Decimal String(number=w392) -> (decimal integer string=w391:string)  [unwired: 1 in]
              }
              frame "180" {
                n913 = Decimal String To Number(string=w395) -> (number=w399:i32)  [unwired: 2 in, 1 out]
                n914 = Subtract(x=w399, y=1) -> (x-y=w397:i32)
                n915 = Number To Decimal String(number=w397) -> (decimal integer string=w396:string)  [unwired: 1 in]
              }
            }
            n916 = Match Pattern(string=w317, regular expression="-") -> (offset past match=w320:i32)  [unwired: 1 in, 3 out]
            n917 = Greater Than 0?(x=w320) -> (x > 0?=w319:bool)
            n918 = Concatenate Strings("TMV," ("write buffer"), w317, "\r\n") -> (w328:string)
            n919 = case shown="True" w319 {
              tunnel: w317 -> [w360 w363]
              tunnel: [w360 w361] -> w315
              frame False {
              }
              frame True {
                n920 = String Subset(string=w363, offset (0)=1) -> (substring=w361:string)  [unwired: 1 in]
              }
            }
            n921 = Fract/Exp String To Number(string=w317) -> (number=w318:dbl)  [unwired: 3 in, 1 out]
            n922 = Not Equal To 0?(x=w318) -> (x != 0?=w316:bool)
            n923 = call "GPIB_func.vi"("error in (no error)"=w327, "write buffer"=w328, "Enum"=T16."WRITE") -> ("error out"=w323:errorcluster)  [unwired: 7 in, 1 out]
            n924 = case shown="False" w316 {
              tunnel: w323 -> [w332 w347]
              tunnel: [w331 w346] -> w322
              tunnel: w315 -> [_ w345]
              frame False {
                n925 = while {
                  tunnel: w332 -> [w343]
                  tunnel: [w334] -> w331
                  i -> [w340]
                  stop <- w338 stop-if-true
                  n926 = Wait (ms)(milliseconds to wait=u32 500) -> ()  [unwired: 1 out]
                  n927 = call "GPIB_func.vi"("error in (no error)"=w343, "write buffer"="TCP?", "Enum"=T16."Query") -> ("read buffer"=w334:string)  [unwired: 7 in, 1 out]
                  n928 = Greater?(x=w340, y=60) -> (0:w337:bool)
                  n929 = Match Pattern(string=w334, regular expression="000") -> (offset past match=w341:i32)  [unwired: 1 in, 3 out]
                  n930 = Greater Than 0?(x=w341) -> (x > 0?=w336:bool)
                  n931 = Or(x=w336, y=w337) -> (x .or. y?=w338:bool)
                }
              }
              frame True {
                n932 = while {
                  tunnel: w347 -> [w358]
                  tunnel: w345 -> [w356]
                  tunnel: [w348] -> w346
                  i -> [w354]
                  stop <- w352 stop-if-true
                  n933 = Wait (ms)(milliseconds to wait=u32 500) -> ()  [unwired: 1 out]
                  n934 = call "GPIB_func.vi"("error in (no error)"=w358, "write buffer"="TCP?", "Enum"=T16."Query") -> ("read buffer"=w348:string)  [unwired: 7 in, 1 out]
                  n935 = Greater?(x=w354, y=60) -> (0:w351:bool)
                  n936 = Match Pattern(string=w348, regular expression=w356) -> (offset past match=w355:i32)  [unwired: 1 in, 3 out]
                  n937 = Greater Than 0?(x=w355) -> (x > 0?=w350:bool)
                  n938 = Or(x=w350, y=w351) -> (x .or. y?=w352:bool)
                }
              }
            }
          }
          frame "CLOSE" {
            n939 = call "GPIB_func.vi"("error in (no error)"=w402, "Enum"=T16."CLOSE") -> ()  [unwired: 8 in, 2 out]
          }
          frame "IDLE", Default {
          }
        }
        n940 = property on="read buffer" class="Str"() -> ("Value"=w130:string)  [unwired: 2 in, 2 out]
        n941 = Fract/Exp String To Number(string=w131) -> (number=w133:dbl)  [unwired: 3 in, 1 out]
        n942 = call <vilib>:"Trim Whitespace.vi"("string"=w131) -> ("trimmed string"=w132:string)  [unwired: 1 in]
        n943 = Concatenate Strings(w131, w130) -> (w129:string)
        n944 = property on="big angle" class="Str"("Value"=w132) -> ()  [unwired: 2 in, 2 out]
        n945 = property on="Meter" class="Knob (strict)"("Value"=w133) -> ()  [unwired: 2 in, 2 out]
        n946 = property on="read buffer" class="Str"("Value"=w129) -> ()  [unwired: 2 in, 2 out]
      }
      n947 = while {
        tunnel: w89 -> [w4685]
        tunnel: w90 -> [w4684]
        tunnel: w94 -> [w4683]
        tunnel: w91 -> [w4682]
        tunnel: w93 -> [w4681]
        tunnel: w92 -> [w4679]
        stop <- w4678 stop-if-true
        n948 = event shown="[66] \"set\": Value Change" {
          selector: _ -> [_ _ _ _ _ _ _ _ _ _ _ _ _ _ _ _ _ _ _ _ _ _ _ _ _ _ _ _ _ _ _ _ _ _ _ _ _ _ _ _ _ _ _ _ _ _ _ _ _ _ _ _ _ _ _ _ _ _ _ _ _ _ _ _ _ _ _ _ _ _ _ _ _ _ _ _ _ _]
          dyn-events: _ -> [_ _ _ _ _ _ _ _ _ _ _ _ _ _ _ _ _ _ _ _ _ _ _ _ _ _ _ _ _ _ _ _ _ _ _ _ _ _ _ _ _ _ _ _ _ _ _ _ _ _ _ _ _ _ _ _ _ _ _ _ _ _ _ _ _ _ _ _ _ _ _ _ _ _ _ _ _ _]
          timeout: 100 -> [_ _ _ _ _ _ _ _ _ _ _ _ _ _ _ _ _ _ _ _ _ _ _ _ _ _ _ _ _ _ _ _ _ _ _ _ _ _ _ _ _ _ _ _ _ _ _ _ _ _ _ _ _ _ _ _ _ _ _ _ _ _ _ _ _ _ _ _ _ _ _ _ _ _ _ _ _ _]
          tunnel: w4685 -> [_ w4695 w4719 w4725 w4729 w4734 w4737 _ w4749 w4752 _ _ _ _ _ _ _ _ _ _ w4806 w4810 w4816 _ _ _ _ _ _ _ _ _ _ _ _ _ _ _ _ _ _ _ _ _ _ _ _ w4987 _ _ w4994 w5007 w5016 _ _ _ _ _ _ _ _ _ _ _ _ _ w5082 _ _ _ _ _ _ _ _ _ _ _]
          tunnel: w4684 -> [w4690 w4696 w4720 w4724 w4730 w4735 w4738 _ w4748 w4751 w4756 w4761 w4766 w4770 w4775 w4780 w4785 w4790 w4795 w4800 w4807 w4809 w4815 w4827 _ w4837 w4840 w4845 w4850 w4855 w4860 w4865 w4870 w4886 w4902 w4907 w4912 w4917 w4922 w4927 w4932 w4937 w4943 w4948 _ _ _ w4976 w4990 _ w4995 w5006 w5015 w5035 w5036 w5041 w5044 w5047 w5050 w5053 w5056 w5059 w5062 w5068 w5072 _ w5085 w5086 w5089 w5092 w5098 w5103 w5108 w5113 w5118 w5123 w5128 w5133]
          tunnel: w4683 -> [w4691 _ _ _ _ _ _ _ _ _ w4759 w4762 _ w4771 w4779 _ w4789 _ w4799 _ _ _ _ w4829 _ _ w4844 _ w4854 w4859 _ _ w4875 _ w4905 _ w4916 _ w4924 _ w4934 w4939 w4944 _ _ _ _ w4984 _ _ _ _ _ _ _ _ _ _ _ _ _ _ _ _ _ _ _ _ _ _ _ _ _ _ _ _ _ _]
          tunnel: w4682 -> [w4689 _ _ _ _ _ _ _ _ _ _ _ w4767 _ _ w4781 _ w4791 _ w4801 _ _ _ _ _ w4838 _ w4846 _ _ w4861 w4866 _ w4887 _ w4908 _ w4918 _ w4929 _ _ _ w4949 _ _ _ w4982 _ _ _ _ _ _ _ _ _ _ _ _ _ _ _ _ _ _ _ _ _ _ _ _ _ _ _ _ _ _]
          tunnel: w4681 -> [w4692 _ _ _ _ _ _ _ _ _ _ _ _ _ _ _ _ _ _ _ _ _ _ _ _ _ _ _ _ _ _ _ _ _ _ _ _ _ _ _ _ _ _ _ _ _ _ w4980 _ _ _ _ _ _ w5040 w5042 w5045 w5048 w5051 w5054 w5057 w5060 w5063 w5069 w5071 _ w5084 w5087 w5090 w5096 w5101 w5106 w5111 w5116 w5121 w5126 w5131 w5136]
          tunnel: w4679 -> [_ _ _ _ _ _ _ _ _ _ _ _ _ _ _ _ _ _ _ _ _ _ _ _ w4831 _ _ _ _ _ _ _ _ _ _ _ _ _ _ _ _ _ _ _ _ _ _ w4979 w4989 _ _ _ _ w5034 _ _ _ _ _ _ _ _ _ _ _ _ _ _ _ _ _ _ _ _ _ _ _ _]
          tunnel: [_ _ _ _ _ _ _ _ _ _ _ _ _ _ _ _ _ _ _ _ _ _ _ _ _ _ _ _ _ _ _ _ _ _ _ _ _ _ _ _ _ _ _ _ _ _ _ "Exit" _ _ _ _ _ _ _ _ _ _ _ _ _ _ _ _ _ _ _ _ _ _ _ _ _ _ _ _ _ _] -> w4678
          event Timeout {
            n949 = event-data() -> ()  [unwired: 1 in, 1 out]
            n950 = Enqueue Element(queue=w4692, element=cluster{"State":T17, "Variable":variant} {"State"=enum."Idle", "Variable"=variant}, error in (no error)=w4690) -> ()  [unwired: 1 in, 3 out]
            n951 = Enqueue Element(queue=w4691, element=T19 {enum."Idle", "variant"=variant}, error in (no error)=w4690) -> ()  [unwired: 1 in, 3 out]
            n952 = Enqueue Element(queue=w4689, element=T19 {enum."Idle", "variant"=variant}) -> ()  [unwired: 2 in, 3 out]
          }
          event "Image": Mouse Up {
            n953 = event-data() -> ("Mods.Double Click"=w4697:bool)  [unwired: 1 in]
            n954 = property on="Image" class="ImageControl"() -> ("Last Mouse Position"=w4698:cluster{"X":i32, "Y":i32}, "ROI"=w4693:T14)  [unwired: 2 in, 2 out]
            n955 = property on="Path?" class="Bool (strict)"() -> ("Value"=w4694:bool)  [unwired: 2 in, 2 out]
            n956 = case shown="True" w4694 {
              tunnel: w4698 -> [w4702 _]
              tunnel: w4697 -> [w4701 _]
              tunnel: w4696 -> [w4700 w4715]
              tunnel: w4695 -> [w4699 w4714]
              tunnel: w4693 -> [_ w4712]
              frame False {
                n957 = case shown="True" w4701 {
                  tunnel: w4702 -> [_ w4704]
                  tunnel: w4700 -> [_ w4708]
                  tunnel: w4699 -> [_ w4707]
                  frame False {
                  }
                  frame True {
                    n958 = Build Array(w4704) -> (w4703:cluster{"X":i32, "Y":i32}[])
                    n959 = Bundle By Name(cluster=T18 {"State"=enum."Overlay_Circle Para", "variant"=variant}, "variant"=w4703) -> (w4705:T18)
                    n960 = Enqueue Element(queue=w4707, element=w4705, error in (no error)=w4708) -> ()  [unwired: 1 in, 3 out]
                  }
                }
              }
              frame True {
                n961 = call "pathVI.vi"("gap"="gap", "ROI"=w4712) -> ("Array"=w4709:cluster{i32, i32}[])  [unwired: 9 in]
                n962 = Bundle By Name(cluster=T18 {"State"=enum."Overlay_Circle Para", "variant"=variant}, "variant"=w4709) -> (w4710:T18)
                n963 = Enqueue Element(queue=w4714, element=w4710, error in (no error)=w4715) -> ()  [unwired: 1 in, 3 out]
              }
            }
          }
          event "User": Value Change {
            n964 = event-data() -> ()  [unwired: 1 in, 1 out]
            n965 = Bundle By Name(cluster=T18 {"State"=enum."User", "variant"=variant}, "variant"="User") -> (w4717:T18)
            n966 = Enqueue Element(queue=w4719, element=w4717, error in (no error)=w4720) -> ()  [unwired: 1 in, 3 out]
          }
          event "Mode": Value Change {
            n967 = event-data() -> ()  [unwired: 1 in, 1 out]
            n968 = Bundle By Name(cluster=T18 {"State"=enum."Mode", "variant"=variant}, "variant"="Mode") -> (w4722:T18)
            n969 = Enqueue Element(queue=w4725, element=w4722, error in (no error)=w4724) -> ()  [unwired: 1 in, 3 out]
          }
          event "Lane Distance(X,Y)": Value Change {
            n970 = event-data() -> ("NewVal"=w4726:cluster{"X":dbl, "Y":dbl})  [unwired: 1 in]
            n971 = Bundle By Name(cluster=T18 {"State"=enum."Lane Distance", "variant"=variant} ("element"), "variant"=w4726) -> (w4727:T18)
            n972 = Enqueue Element(queue=w4729, element=w4727, error in (no error)=w4730) -> ()  [unwired: 1 in, 3 out]
          }
          event "Velocity": Value Change {
            n973 = event-data() -> ("NewVal"=w4731:dbl)  [unwired: 1 in]
            n974 = Bundle By Name(cluster=T18 {"State"=enum."Velocity", "variant"=variant}, "variant"=w4731) -> (w4732:T18)
            n975 = Enqueue Element(queue=w4734, element=w4732, error in (no error)=w4735) -> ()  [unwired: 1 in, 3 out]
          }
          event "Clear All": Value Change {
            n976 = event-data() -> ()  [unwired: 1 in, 1 out]
            n977 = Enqueue Element(queue=w4737, element=T18 {"State"=enum."Clear All", "variant"=variant}, error in (no error)=w4738) -> ()  [unwired: 1 in, 3 out]
          }
          event "Path?": Value Change {
            w4740 = u32 11 items=["Zoom Tool"=8, "Selection Tool"=0, "Pan Tool"=9, "Point Tool"=1, "Line Tool"=2, "Rectangle Tool"=3, "Rotated Rectangle Tool"=12, "Polyline Tool"=10, "Polygon Tool"=5, "Freehand Tool"=11, "Closed Freehand Tool"=6, "Ellipse Tool"=4, "Annulus Tool"=7] ("Current ROI Tool")
            w4741 = u32 1 items=["Zoom Tool"=8, "Selection Tool"=0, "Pan Tool"=9, "Point Tool"=1, "Line Tool"=2, "Rectangle Tool"=3, "Rotated Rectangle Tool"=12, "Polyline Tool"=10, "Polygon Tool"=5, "Freehand Tool"=11, "Closed Freehand Tool"=6, "Ellipse Tool"=4, "Annulus Tool"=7] ("Current ROI Tool")
            n978 = event-data() -> ("NewVal"=w4742:bool)  [unwired: 1 in, 5 out]
            n979 = Not(x=w4742) -> (.not. x?=w4743:bool)
            n980 = Select(t=w4740, s=w4742, f=w4741) -> (s? t:f=w4739:u32)
            n981 = property on="Image" class="ImageControl"("ROI"=T14 {"Global Rectangle"=[], "Contours"=[]}, "Freehand Tool Button Visible"=w4742, "Point Tool Button Visible"=w4743, "Current ROI Tool"=w4739) -> ()  [unwired: 2 in, 2 out]
          }
          event "Coordinates(X,Y)": Value Change {
            n982 = event-data() -> ("NewVal"=w4745:cluster{"X":dbl, "Y":dbl})  [unwired: 1 in]
            n983 = Bundle By Name(cluster=T18 {"State"=enum."Coordinate", "variant"=variant}, "variant"=w4745) -> (w4746:T18)
            n984 = Enqueue Element(queue=w4749, element=w4746, error in (no error)=w4748) -> ()  [unwired: 1 in, 3 out]
          }
          event "Path No.": Value Change {
            n985 = event-data() -> ("NewVal"=w4753:u16)  [unwired: 1 in]
            n986 = Bundle By Name(cluster=T18 {"State"=enum."Path No.", "variant"=variant}, "variant"=w4753) -> (w4750:T18)
            n987 = Enqueue Element(queue=w4752, element=w4750, error in (no error)=w4751) -> ()  [unwired: 1 in, 3 out]
          }
          event "Run/Stop": Value Change {
            n988 = event-data() -> ()  [unwired: 1 in, 6 out]
            n989 = Bundle By Name(cluster=T19 {enum."Dynamic", "variant"=variant}, "variant"="Dynamic1") -> (w4757:T19)
            n990 = Enqueue Element(queue=w4759, element=w4757, error in (no error)=w4756) -> ()  [unwired: 1 in, 3 out]
          }
          event "Dynamic1": Value Change {
            n991 = event-data() -> ()  [unwired: 1 in, 6 out]
            n992 = property on="Dynamic1" class="Clust (strict)"() -> ("Value"=w4760:T9)  [unwired: 2 in, 2 out]
            n993 = Bundle By Name(cluster=T19 {enum."dyset", "variant"=variant}, "variant"=w4760) -> (w4763:T19)
            n994 = Enqueue Element(queue=w4762, element=w4763, error in (no error)=w4761) -> ()  [unwired: 1 in, 3 out]
          }
          event "Run/Stop": Value Change {
            n995 = event-data() -> ()  [unwired: 1 in, 6 out]
            n996 = Bundle By Name(cluster=T19 {enum."Dynamic", "variant"=variant}, "variant"="Dynamic2") -> (w4768:T19)
            n997 = Enqueue Element(queue=w4767, element=w4768, error in (no error)=w4766) -> ()  [unwired: 1 in, 3 out]
          }
          event "Dynamic2": Value Change {
            n998 = event-data() -> ()  [unwired: 1 in, 6 out]
            n999 = property on="Dynamic2" class="Clust (strict)"() -> ("Value"=w4772:T9)  [unwired: 2 in, 2 out]
            n1000 = Bundle By Name(cluster=T19 {enum."dyset", "variant"=variant}, "variant"=w4772) -> (w4773:T19)
            n1001 = Enqueue Element(queue=w4771, element=w4773, error in (no error)=w4770) -> ()  [unwired: 1 in, 3 out]
          }
          event "T/R Converters": Value Change {
            n1002 = event-data() -> ("NewVal"=w4776:bool)  [unwired: 1 in, 5 out]
            n1003 = Bundle By Name(cluster=T19 {enum."Convert", "variant"=variant}, "variant"=w4776) -> (w4777:T19)
            n1004 = Enqueue Element(queue=w4779, element=w4777, error in (no error)=w4775) -> ()  [unwired: 1 in, 3 out]
          }
          event "T/R Converters": Value Change {
            n1005 = event-data() -> ("NewVal"=w4782:bool)  [unwired: 1 in, 5 out]
            n1006 = Bundle By Name(cluster=T19 {enum."Convert", "variant"=variant}, "variant"=w4782) -> (w4783:T19)
            n1007 = Enqueue Element(queue=w4781, element=w4783, error in (no error)=w4780) -> ()  [unwired: 1 in, 3 out]
          }
          event "RF ON/OFF": Value Change {
            n1008 = event-data() -> ("NewVal"=w4786:bool)  [unwired: 1 in, 5 out]
            n1009 = Bundle By Name(cluster=T19 {enum."RF ON/OFF", "variant"=variant}, "variant"=w4786) -> (w4787:T19)
            n1010 = Enqueue Element(queue=w4789, element=w4787, error in (no error)=w4785) -> ()  [unwired: 1 in, 3 out]
          }
          event "RF ON/OFF": Value Change {
            n1011 = event-data() -> ("NewVal"=w4792:bool)  [unwired: 1 in, 5 out]
            n1012 = Bundle By Name(cluster=T19 {enum."RF ON/OFF", "variant"=variant}, "variant"=w4792) -> (w4793:T19)
            n1013 = Enqueue Element(queue=w4791, element=w4793, error in (no error)=w4790) -> ()  [unwired: 1 in, 3 out]
          }
          event "Stop": Value Change {
            n1014 = event-data() -> ("NewVal"=w4796:bool)  [unwired: 1 in, 5 out]
            n1015 = Bundle By Name(cluster=T19 {enum."Stop", "variant"=variant}, "variant"=w4796) -> (w4797:T19)
            n1016 = Enqueue Element(queue=w4799, element=w4797, error in (no error)=w4795) -> ()  [unwired: 1 in, 3 out]
          }
          event "Stop": Value Change {
            n1017 = event-data() -> ("NewVal"=w4802:bool)  [unwired: 1 in, 5 out]
            n1018 = Bundle By Name(cluster=T19 {enum."Stop", "variant"=variant}, "variant"=w4802) -> (w4803:T19)
            n1019 = Enqueue Element(queue=w4801, element=w4803, error in (no error)=w4800) -> ()  [unwired: 1 in, 3 out]
          }
          event "Modify (X,Y)": Value Change {
            n1020 = event-data() -> ()  [unwired: 1 in, 1 out]
            n1021 = Enqueue Element(queue=w4806, element=T18 {"State"=enum."Modify", "variant"=variant}, error in (no error)=w4807) -> ()  [unwired: 1 in, 3 out]
          }
          event "report dist 2", "report dist": Value Change {
            n1022 = event-data() -> ()  [unwired: 1 in, 1 out]
            n1023 = Enqueue Element(queue=w4810, element=T18 {"State"=enum."Report Dist", "variant"=variant}, error in (no error)=w4809) -> ()  [unwired: 1 in, 3 out]
          }
          event "Load": Value Change {
            n1024 = event-data() -> ()  [unwired: 1 in, 1 out]
            n1025 = call <vilib>:"Check if File or Folder Exists.vi"("error in (no error)"=w4815, "path"="Path") -> ("error out"=w4813:errorcluster, "file or folder exists?"=w4812:bool, "dup path"=w4811:path)  [unwired: 7 in]
            n1026 = case shown="True" w4812 {
              tunnel: w4816 -> [_ w4821]
              tunnel: w4813 -> [_ w4820]
              tunnel: w4811 -> [_ w4818]
              frame False {
              }
              frame True {
                n1027 = Bundle By Name(cluster=T18 {"State"=enum."Load", "variant"=variant}, "variant"=w4818) -> (w4817:T18)
                n1028 = Enqueue Element(queue=w4821, element=w4817, error in (no error)=w4820) -> ()  [unwired: 1 in, 3 out]
              }
            }
          }
          event "Inst. Connect": Value Change {
            n1029 = event-data() -> ()  [unwired: 1 in, 1 out]
            n1030 = Enqueue Element(queue=w4829, element=T19 {enum."Inst. Connect", "variant"=variant}, error in (no error)=w4827) -> (queue out=w4825:refnum<queue>, error out=w4826:errorcluster)  [unwired: 1 in, 1 out]
            n1031 = property on="Freq. (GHz)" class="DigNum (strict)"() -> ("Value"=w4823:dbl)  [unwired: 2 in, 2 out]
            n1032 = Bundle By Name(cluster=T19 {enum."Freq. (GHz)", "variant"=variant}, "variant"=w4823) -> (w4822:T19)
            n1033 = Enqueue Element(queue=w4825, element=w4822, error in (no error)=w4826) -> ()  [unwired: 1 in, 3 out]
          }
          event "Connect": Value Change {
            n1034 = event-data() -> ()  [unwired: 1 in, 6 out]
            n1035 = Enqueue Element(queue=w4831, element=T21 {"Enum"=enum."INIT", "Variable"=variant}) -> ()  [unwired: 2 in, 3 out]
          }
          event "Inst. Connect": Value Change {
            n1036 = event-data() -> ()  [unwired: 1 in, 6 out]
            n1037 = property on="Freq. (GHz)" class="DigNum (strict)"() -> ("Value"=w4832:dbl)  [unwired: 2 in, 2 out]
            n1038 = Enqueue Element(queue=w4838, element=T19 {enum."Inst. Connect", "variant"=variant}, error in (no error)=w4837) -> (queue out=w4834:refnum<queue>, error out=w4836:errorcluster)  [unwired: 1 in, 1 out]
            n1039 = Bundle By Name(cluster=T19 {enum."Freq. (GHz)", "variant"=variant}, "variant"=w4832) -> (w4833:T19)
            n1040 = Enqueue Element(queue=w4834, element=w4833, error in (no error)=w4836) -> ()  [unwired: 1 in, 3 out]
          }
          event "Freq. (GHz)": Value Change {
            n1041 = event-data() -> ()  [unwired: 1 in, 1 out]
            n1042 = Bundle By Name(cluster=T19 {enum."Freq. (GHz)", "variant"=variant}, "variant"="Freq. (GHz)") -> (w4842:T19)
            n1043 = Enqueue Element(queue=w4844, element=w4842, error in (no error)=w4840) -> ()  [unwired: 1 in, 3 out]
          }
          event "Freq. (GHz)": Value Change {
            n1044 = event-data() -> ()  [unwired: 1 in, 1 out]
            n1045 = Bundle By Name(cluster=T19 {enum."Freq. (GHz)", "variant"=variant}, "variant"="Freq. (GHz)") -> (w4848:T19)
            n1046 = Enqueue Element(queue=w4846, element=w4848, error in (no error)=w4845) -> ()  [unwired: 1 in, 3 out]
          }
          event "GTX (dB)": Value Change {
            n1047 = event-data() -> ()  [unwired: 1 in, 3 out]
            n1048 = Bundle By Name(cluster=T19 {enum."GTX (dB)", "variant"=variant}, "variant"="GTX (dB)") -> (w4852:T19)
            n1049 = Enqueue Element(queue=w4854, element=w4852, error in (no error)=w4850) -> ()  [unwired: 1 in, 3 out]
          }
          event "Rx Attenuation (dB)": Value Change {
            n1050 = event-data() -> ()  [unwired: 1 in, 3 out]
            n1051 = Bundle By Name(cluster=T19 {enum."rx att", "variant"=variant}, "variant"="Rx Attenuation (dB)") -> (w4857:T19)
            n1052 = Enqueue Element(queue=w4859, element=w4857, error in (no error)=w4855) -> ()  [unwired: 1 in, 3 out]
          }
          event "Rx Attenuation (dB)": Value Change {
            n1053 = event-data() -> ()  [unwired: 1 in, 3 out]
            n1054 = Bundle By Name(cluster=T19 {enum."rx att", "variant"=variant}, "variant"="Rx Attenuation (dB)") -> (w4863:T19)
            n1055 = Enqueue Element(queue=w4861, element=w4863, error in (no error)=w4860) -> ()  [unwired: 1 in, 3 out]
          }
          event "GTX (dB)": Value Change {
            n1056 = event-data() -> ()  [unwired: 1 in, 3 out]
            n1057 = Bundle By Name(cluster=T19 {enum."GTX (dB)", "variant"=variant}, "variant"="GTX (dB)") -> (w4868:T19)
            n1058 = Enqueue Element(queue=w4866, element=w4868, error in (no error)=w4865) -> ()  [unwired: 1 in, 3 out]
          }
          event "Mapping": Value Change {
            n1059 = event-data() -> ("OldVal"=w4874:cluster{"4:4":bool, "4:2":bool, "4:1":bool}, "NewVal"=w4882:cluster{"4:4":bool, "4:2":bool, "4:1":bool})  [unwired: 1 in]
            n1060 = Cluster To Array(cluster=w4882) -> (array=w4872:bool[])
            n1061 = Cluster To Array(cluster=w4874) -> (array=w4873:bool[])
            n1062 = Exclusive Or(1:w4872, 2:w4873) -> (0:w4871:bool[])
            n1063 = Search 1D Array(1D array=w4871, element=TRUE) -> (index of element=w4880:i32)  [unwired: 1 in]
            n1064 = case shown="0, Default" w4880 {
              tunnel: [bool[] [TRUE, FALSE, FALSE] bool[] [FALSE, TRUE, FALSE] bool[] [FALSE, FALSE, TRUE]] -> w4879
              frame 0, Default {
              }
              frame 1 {
              }
              frame 2 {
              }
            }
            n1065 = Array To Cluster(array=w4879) -> (cluster=w4876:cluster{"[0]":bool, "[1]":bool, "[2]":bool})
            n1066 = Bundle By Name(cluster=T19 {enum."Mapping", "variant"=variant}, "variant"=w4876) -> (w4877:T19)
            n1067 = Enqueue Element(queue=w4875, element=w4877, error in (no error)=w4870) -> ()  [unwired: 1 in, 3 out]
          }
          event "Mapping": Value Change {
            n1068 = event-data() -> ("OldVal"=w4891:cluster{"4:4":bool, "4:2":bool, "4:1":bool}, "NewVal"=w4898:cluster{"4:4":bool, "4:2":bool, "4:1":bool})  [unwired: 1 in]
            n1069 = Cluster To Array(cluster=w4898) -> (array=w4889:bool[])
            n1070 = Cluster To Array(cluster=w4891) -> (array=w4890:bool[])
            n1071 = Exclusive Or(1:w4889, 2:w4890) -> (0:w4888:bool[])
            n1072 = Search 1D Array(1D array=w4888, element=TRUE) -> (index of element=w4896:i32)  [unwired: 1 in]
            n1073 = case shown="0, Default" w4896 {
              tunnel: [bool[] [TRUE, FALSE, FALSE] bool[] [FALSE, TRUE, FALSE] bool[] [FALSE, FALSE, TRUE]] -> w4895
              frame 0, Default {
              }
              frame 1 {
              }
              frame 2 {
              }
            }
            n1074 = Array To Cluster(array=w4895) -> (cluster=w4892:cluster{"[0]":bool, "[1]":bool, "[2]":bool})
            n1075 = Bundle By Name(cluster=T19 {enum."Mapping", "variant"=variant}, "variant"=w4892) -> (w4893:T19)
            n1076 = Enqueue Element(queue=w4887, element=w4893, error in (no error)=w4886) -> ()  [unwired: 1 in, 3 out]
          }
          event "Direct program": Value Change {
            n1077 = event-data() -> ()  [unwired: 1 in, 1 out]
            n1078 = Bundle By Name(cluster=T19 {enum."Direct Program", "variant"=variant}, "variant"="Direct program") -> (w4904:T19)
            n1079 = Enqueue Element(queue=w4905, element=w4904, error in (no error)=w4902) -> ()  [unwired: 1 in, 3 out]
          }
          event "Direct program2": Value Change {
            n1080 = event-data() -> ()  [unwired: 1 in, 1 out]
            n1081 = Bundle By Name(cluster=T19 {enum."Direct Program", "variant"=variant}, "variant"="Direct program2") -> (w4910:T19)
            n1082 = Enqueue Element(queue=w4908, element=w4910, error in (no error)=w4907) -> ()  [unwired: 1 in, 3 out]
          }
          event "GRX (dB)": Value Change {
            n1083 = event-data() -> ()  [unwired: 1 in, 1 out]
            n1084 = Bundle By Name(cluster=T19 {enum."GRX (dB)", "variant"=variant}, "variant"="GRX (dB)") -> (w4914:T19)
            n1085 = Enqueue Element(queue=w4916, element=w4914, error in (no error)=w4912) -> ()  [unwired: 1 in, 3 out]
          }
          event "GRX (dB)": Value Change {
            n1086 = event-data() -> ()  [unwired: 1 in, 1 out]
            n1087 = Bundle By Name(cluster=T19 {enum."GRX (dB)", "variant"=variant}, "variant"="GRX (dB)") -> (w4920:T19)
            n1088 = Enqueue Element(queue=w4918, element=w4920, error in (no error)=w4917) -> ()  [unwired: 1 in, 3 out]
          }
          event "Range Trim (m)": Value Change {
            n1089 = event-data() -> ()  [unwired: 1 in, 2 out]
            n1090 = Bundle By Name(cluster=T19 {enum."Range Trim(m)", "variant"=variant}, "variant"="Range Trim (m)") -> (w4925:T19)
            n1091 = Enqueue Element(queue=w4924, element=w4925, error in (no error)=w4922) -> ()  [unwired: 1 in, 3 out]
          }
          event "Range Trim (m)": Value Change {
            n1092 = event-data() -> ()  [unwired: 1 in, 2 out]
            n1093 = Bundle By Name(cluster=T19 {enum."Range Trim(m)", "variant"=variant}, "variant"="Range Trim (m)") -> (w4930:T19)
            n1094 = Enqueue Element(queue=w4929, element=w4930, error in (no error)=w4927) -> ()  [unwired: 1 in, 3 out]
          }
          event "Gain Trim (dB)": Value Change {
            n1095 = event-data() -> ()  [unwired: 1 in, 1 out]
            n1096 = Bundle By Name(cluster=T19 {enum."Gain Trim (dB)", "variant"=variant}, "variant"="Gain Trim (dB)") -> (w4935:T19)
            n1097 = Enqueue Element(queue=w4934, element=w4935, error in (no error)=w4932) -> ()  [unwired: 1 in, 3 out]
          }
          event "Gain Trim (dB)": Value Change {
            n1098 = event-data() -> ()  [unwired: 1 in, 1 out]
            n1099 = Bundle By Name(cluster=T19 {enum."Gain Trim (dB)", "variant"=variant}, "variant"="Gain Trim (dB)") -> (w4940:T19)
            n1100 = Enqueue Element(queue=w4939, element=w4940, error in (no error)=w4937) -> ()  [unwired: 1 in, 3 out]
          }
          event "Distance to RUT": Value Change {
            n1101 = event-data() -> ()  [unwired: 1 in, 1 out]
            n1102 = Bundle By Name(cluster=T19 {enum."Distance to RUT", "variant"=variant}, "variant"="Distance to RUT") -> (w4945:T19)
            n1103 = Enqueue Element(queue=w4944, element=w4945, error in (no error)=w4943) -> ()  [unwired: 1 in, 3 out]
          }
          event "Distance to RUT": Value Change {
            n1104 = event-data() -> ()  [unwired: 1 in, 1 out]
            n1105 = Bundle By Name(cluster=T19 {enum."Distance to RUT", "variant"=variant}, "variant"="Distance to RUT") -> (w4950:T19)
            n1106 = Enqueue Element(queue=w4949, element=w4950, error in (no error)=w4948) -> ()  [unwired: 1 in, 3 out]
          }
          event "RCS2": Value Change {
            n1107 = event-data() -> ()  [unwired: 1 in, 6 out]
            n1108 = property on="Distance to RUT" class="DigNum (strict)"() -> ("Value"=w4956:dbl)  [unwired: 2 in, 2 out]
            n1109 = property on="Gain" class="DigNum (strict)"() -> ("Value"=w4954:dbl)  [unwired: 2 in, 2 out]
            n1110 = property on="GTX (dB)" class="DigNum (strict)"() -> ("Value"=w4958:dbl)  [unwired: 2 in, 2 out]
            n1111 = property on="GRX (dB)" class="DigNum (strict)"() -> ("Value"=w4957:dbl)  [unwired: 2 in, 2 out]
            n1112 = property on="Range" class="DigNum (strict)"() -> ("Value"=w4955:dbl)  [unwired: 2 in, 2 out]
            n1113 = call "rcs_cot.vi"("range"=w4955, "Distance to RUT"=w4956, "Gain"=w4954, "GRX (dB)"=w4957, "GTX (dB)"=w4958) -> ("x-y"=w4952:dbl)  [unwired: 6 in]
            "RCS 2" <- w4952
            n1114 = case shown="True" "Boolean 2" {
              tunnel: w4952 -> [_ w4959]
              frame False {
              }
              frame True {
                "RCS def 2" <- w4959
              }
            }
          }
          event "RCSAUTO": Value Change {
            n1115 = event-data() -> ()  [unwired: 1 in, 6 out]
            n1116 = call "rcs_cot.vi"("range"="Range", "Distance to RUT"="Dist to RUT", "Gain"="Gain", "GRX (dB)"="GRX (dB)", "GTX (dB)"="GTX (dB)") -> ("x-y"=→"RCS":dbl)  [unwired: 6 in]
          }
          event "RCS1": Value Change {
            n1117 = event-data() -> ()  [unwired: 1 in, 6 out]
            n1118 = property on="Distance to RUT" class="DigNum (strict)"() -> ("Value"=w4970:dbl)  [unwired: 2 in, 2 out]
            n1119 = property on="Gain" class="DigNum (strict)"() -> ("Value"=w4968:dbl)  [unwired: 2 in, 2 out]
            n1120 = property on="GRX (dB)" class="DigNum (strict)"() -> (error out=w4971:errorcluster, "Value"=w4972:dbl)  [unwired: 2 in, 1 out]
            n1121 = property on="GTX (dB)" class="DigNum (strict)"() -> ("Value"=w4973:dbl)  [unwired: 2 in, 2 out]
            n1122 = property on="Range" class="DigNum (strict)" props=["TipStrip", "Value"](error in=w4971) -> ("Value"=w4969:dbl)  [unwired: 1 in, 3 out]
            n1123 = call "rcs_cot.vi"("range"=w4969, "Distance to RUT"=w4970, "Gain"=w4968, "GRX (dB)"=w4972, "GTX (dB)"=w4973) -> ("x-y"=w4966:dbl)  [unwired: 6 in]
            "RCS" <- w4966
            n1124 = case shown="True" "Boolean" {
              tunnel: w4966 -> [_ w4974]
              frame False {
              }
              frame True {
                "RCS def" <- w4974
              }
            }
          }
          event "Exit": Value Change {
            n1125 = event-data() -> ()  [unwired: 1 in, 1 out]
            n1126 = property on="Cluster" class="Clust (strict)"(error in=w4976, "Value"=cluster{"tester  A":bool, " tester B":bool} {"tester  A"=TRUE, " tester B"=TRUE} ("Cluster")) -> ()  [unwired: 1 in, 2 out]
            n1127 = Enqueue Element(queue=w4987, element=T18 {"State"=enum."Exit", "variant"=variant}, error in (no error)=w4976) -> ()  [unwired: 1 in, 3 out]
            n1128 = Enqueue Element(queue=w4984, element=T19 {enum."Exit", "variant"=variant}, error in (no error)=w4976) -> ()  [unwired: 1 in, 3 out]
            n1129 = Enqueue Element(queue=w4979, element=T21 {"Enum"=enum."CLOSE", "Variable"=variant}, error in (no error)=w4976) -> ()  [unwired: 1 in, 3 out]
            n1130 = Enqueue Element(queue=w4980, element=cluster{"State":T17, "Variable":variant} {"State"=enum."Exit", "Variable"=variant}, error in (no error)=w4976) -> ()  [unwired: 1 in, 3 out]
            n1131 = Enqueue Element(queue=w4982, element=T19 {enum."Exit", "variant"=variant}, error in (no error)=w4976) -> ()  [unwired: 1 in, 3 out]
            n1132 = property on="AutoExit" class="Bool (strict)"("Value"="Exit") -> ()  [unwired: 2 in, 2 out]
          }
          event "Add Button": Value Change {
            n1133 = event-data() -> ()  [unwired: 1 in, 6 out]
            n1134 = Enqueue Element(queue=w4989, element=T21 {"Enum"=enum."ADD", "Variable"=variant}, error in (no error)=w4990) -> ()  [unwired: 1 in, 3 out]
          }
          event "clearMSG": Value Change {
            n1135 = event-data() -> ()  [unwired: 1 in, 6 out]
            n1136 = property on="MSG" class="Str"("Value"="" ("MSG")) -> ()  [unwired: 2 in, 2 out]
          }
          event "Save Button", "Save Button 2": Value Change {
            n1137 = event-data() -> ()  [unwired: 1 in, 6 out]
            n1138 = Enqueue Element(queue=w4994, element=T18 {"State"=enum."dypath", "variant"=variant}, error in (no error)=w4995) -> (queue out=w4993:refnum<queue>, error out=w4996:errorcluster)  [unwired: 1 in, 1 out]
            n1139 = Enqueue Element(queue=w4993, element=T18 {"State"=enum."save", "variant"=variant}, error in (no error)=w4996) -> ()  [unwired: 1 in, 3 out]
          }
          event "Open Button": Value Change {
            n1140 = event-data() -> ()  [unwired: 1 in, 6 out]
            n1141 = call <vilib>:"Application Directory.vi"() -> ("Application Directory"=w5002:path)
            n1142 = Build Path(base path=w5002, name or relative path="path") -> (appended path=w5000:path)
            n1143 = call "File Dialog"("start path"=w5000, "prompt"="Select an image file...", "pattern (all files)"="2*.xml") -> ("selected path"=w5003:path, "error out"=w4999:errorcluster)  [unwired: 9 in, 2 out]
            n1144 = Bundle(cluster=T18 {"State"=enum."Loadpath", "variant"=variant} ("element"), "variant"=w5003) -> (w5004:T18)  [unwired: 1 in]
            n1145 = Enqueue Element(queue=w5007, element=w5004, error in (no error)=w5006) -> ()  [unwired: 1 in, 3 out]
            n1146 = call <vilib>:"Clear Errors.vi"("error in (no error)"=w4999) -> ()  [unwired: 5 in, 2 out]
          }
          event "dynamic setting": Value Change {
            n1147 = event-data() -> ()  [unwired: 1 in, 6 out]
            n1148 = property on="DYNAMIC" class="Arr (strict)"() -> ("Value"=w5021:T1)  [unwired: 2 in, 2 out]
            n1149 = property on="DYNAMIC 2" class="Arr (strict)"() -> ("Value"=w5018:T1)  [unwired: 2 in, 2 out]
            n1150 = property on="User" class="Enum (strict)"() -> ("Value"=w5019:enum16{"Car A", "Car B"})  [unwired: 2 in, 2 out]
            n1151 = case shown="\"Car B\"" w5019 {
              tunnel: w5021 -> [w5025 w5030]
              tunnel: [w5027 w5030] -> w5020
              tunnel: w5018 -> [w5026 w5029]
              tunnel: [w5026 w5031] -> w5017
              tunnel: [w5025 w5029] -> w5011
              frame "Car A" {
                n1152 = for {
                  tunnel: w5025 -> [_] mode=indexing
                  tunnel: [w5028] -> w5027 mode=indexing
                  n1153 = property on="dynamic setting" class="Clust (strict)"() -> ("Value"=w5028:T5)  [unwired: 2 in, 2 out]
                }
              }
              frame "Car B" {
                n1154 = for {
                  tunnel: [w5032] -> w5031 mode=indexing
                  tunnel: w5029 -> [_] mode=indexing
                  n1155 = property on="dynamic setting" class="Clust (strict)"() -> ("Value"=w5032:T5)  [unwired: 2 in, 2 out]
                }
              }
            }
            n1156 = Array Size(array=w5011) -> (size(s)=w5010:i32)
            n1157 = Not Equal To 0?(x=w5010) -> (x != 0?=w5009:bool)
            n1158 = property on="DYNAMIC" class="Arr (strict)"(error in=w5015, "Value"=w5020) -> (error out=w5012:errorcluster)  [unwired: 1 in, 1 out]
            n1159 = property on="DYNAMIC 2" class="Arr (strict)"(error in=w5015, "Value"=w5017) -> (error out=w5014:errorcluster)  [unwired: 1 in, 1 out]
            n1160 = Merge Errors(w5012, w5014) -> (w5013:errorcluster)
            n1161 = case shown="True" w5009 {
              tunnel: w5016 -> [_ w5024]
              tunnel: w5013 -> [_ w5022]
              frame False {
              }
              frame True {
                n1162 = Enqueue Element(queue=w5024, element=T18 {"State"=enum."dynamic", "variant"=variant}, error in (no error)=w5022) -> ()  [unwired: 1 in, 3 out]
              }
            }
          }
          event "Remove Button": Value Change {
            n1163 = event-data() -> ()  [unwired: 1 in, 6 out]
            n1164 = Enqueue Element(queue=w5034, element=T21 {"Enum"=enum."DEC", "Variable"=variant}, error in (no error)=w5035) -> ()  [unwired: 1 in, 3 out]
          }
          event "Connect DUT Button": Value Change {
            n1165 = event-data() -> ()  [unwired: 1 in, 6 out]
            n1166 = Bundle By Name(cluster=cluster{"State":T17, "Variable":variant} {"State"=enum."Connect", "Variable"=variant}, "Variable"="IP Addr") -> (w5037:cluster{"State":T17, "Variable":variant})
            n1167 = Enqueue Element(queue=w5040, element=w5037, error in (no error)=w5036) -> ()  [unwired: 1 in, 3 out]
          }
          event "Stop Button": Value Change {
            n1168 = event-data() -> ()  [unwired: 1 in, 6 out]
            n1169 = Enqueue Element(queue=w5042, element=cluster{"State":T17, "Variable":variant} {"State"=enum."Stop", "Variable"=variant}, error in (no error)=w5041) -> ()  [unwired: 1 in, 3 out]
          }
          event "Move Button": Value Change {
            n1170 = event-data() -> ()  [unwired: 1 in, 6 out]
            n1171 = Enqueue Element(queue=w5045, element=cluster{"State":T17, "Variable":variant} {"State"=enum."Move", "Variable"=variant}, error in (no error)=w5044) -> ()  [unwired: 1 in, 3 out]
          }
          event "Rotate Button": Value Change {
            n1172 = event-data() -> ()  [unwired: 1 in, 6 out]
            n1173 = Enqueue Element(queue=w5048, element=cluster{"State":T17, "Variable":variant} {"State"=enum."Rotate", "Variable"=variant}, error in (no error)=w5047) -> ()  [unwired: 1 in, 3 out]
          }
          event "Return to Origin Button": Value Change {
            n1174 = event-data() -> ()  [unwired: 1 in, 6 out]
            n1175 = Enqueue Element(queue=w5051, element=cluster{"State":T17, "Variable":variant} {"State"=enum."Return to Origin", "Variable"=variant}, error in (no error)=w5050) -> ()  [unwired: 1 in, 3 out]
          }
          event "Return to Zero Button": Value Change {
            n1176 = event-data() -> ()  [unwired: 1 in, 6 out]
            n1177 = Enqueue Element(queue=w5054, element=cluster{"State":T17, "Variable":variant} {"State"=enum."Return to Zero", "Variable"=variant}, error in (no error)=w5053) -> ()  [unwired: 1 in, 3 out]
          }
          event "Initial to Y Step": Value Change {
            n1178 = event-data() -> ()  [unwired: 1 in, 6 out]
            n1179 = Enqueue Element(queue=w5057, element=cluster{"State":T17, "Variable":variant} {"State"=enum."Initial to Y Step", "Variable"=variant}, error in (no error)=w5056) -> ()  [unwired: 1 in, 3 out]
          }
          event "Step1": Value Change {
            n1180 = event-data() -> ()  [unwired: 1 in, 6 out]
            n1181 = Enqueue Element(queue=w5060, element=cluster{"State":T17, "Variable":variant} {"State"=enum."Go to Step1", "Variable"=variant}, error in (no error)=w5059) -> ()  [unwired: 1 in, 3 out]
          }
          event "Step2": Value Change {
            n1182 = event-data() -> ()  [unwired: 1 in, 6 out]
            n1183 = Enqueue Element(queue=w5063, element=cluster{"State":T17, "Variable":variant} {"State"=enum."Go to Step2", "Variable"=variant}, error in (no error)=w5062) -> ()  [unwired: 1 in, 3 out]
          }
          event "Cluster 2": Value Change {
            n1184 = event-data() -> ()  [unwired: 1 in, 6 out]
            n1185 = Bundle By Name(cluster=cluster{"State":T17, "Variable":variant} {"State"=enum."reset xy", "Variable"=variant}, "Variable"="Cluster 2") -> (w5066:cluster{"State":T17, "Variable":variant})
            n1186 = Enqueue Element(queue=w5069, element=w5066, error in (no error)=w5068) -> ()  [unwired: 1 in, 3 out]
          }
          event "reset ant": Value Change {
            n1187 = event-data() -> ()  [unwired: 1 in, 6 out]
            n1188 = Bundle By Name(cluster=cluster{"State":T17, "Variable":variant} {"State"=enum."reset ant", "Variable"=variant}, "Variable"="reset ant") -> (w5073:cluster{"State":T17, "Variable":variant})
            n1189 = Enqueue Element(queue=w5071, element=w5073, error in (no error)=w5072) -> ()  [unwired: 1 in, 3 out]
          }
          event "s/d setting": Value Change {
            n1190 = event-data() -> ("NewVal"=w5075:bool)  [unwired: 1 in, 5 out]
            n1191 = case shown="True" w5075 {
              frame False {
                w5077 = TRUE ("Visible")
                n1192 = property on="dynamic setting" class="Clust (strict)"("Visible"=w5077) -> ()  [unwired: 2 in, 2 out]
                n1193 = Not(x=w5077) -> (.not. x?=w5076:bool)
                n1194 = property on="Mode" class="Bool (strict)"("Value"=w5076) -> ()  [unwired: 2 in, 2 out]
                n1195 = property on="Rotate" class="Bool (strict)"("Value"=w5076) -> ()  [unwired: 2 in, 2 out]
                n1196 = property on="Path?" class="Bool (strict)"("Value"=w5076, "Visible"=w5076) -> ()  [unwired: 2 in, 2 out]
              }
              frame True {
                n1197 = property on="dynamic setting" class="Clust (strict)"("Visible"=FALSE) -> ()  [unwired: 2 in, 2 out]
              }
            }
          }
          event "set": Value Change {
            n1198 = event-data() -> ()  [unwired: 1 in, 6 out]
            n1199 = Enqueue Element(queue=w5084, element=cluster{"State":T17, "Variable":variant} {"State"=enum."set speed", "Variable"=variant}, error in (no error)=w5085) -> (error out=w5081:errorcluster)  [unwired: 1 in, 2 out]
            n1200 = property on="set" class="Bool (strict)"("Value"=FALSE ("set")) -> ()  [unwired: 2 in, 2 out]
            n1201 = Enqueue Element(queue=w5082, element=T18 {"State"=enum."dypath", "variant"=variant}, error in (no error)=w5081) -> ()  [unwired: 1 in, 3 out]
          }
          event "Step3": Value Change {
            n1202 = event-data() -> ()  [unwired: 1 in, 6 out]
            n1203 = Enqueue Element(queue=w5087, element=cluster{"State":T17, "Variable":variant} {"State"=enum."Go to Step3", "Variable"=variant}, error in (no error)=w5086) -> ()  [unwired: 1 in, 3 out]
          }
          event "Return to Middle Button": Value Change {
            n1204 = event-data() -> ()  [unwired: 1 in, 6 out]
            n1205 = Enqueue Element(queue=w5090, element=cluster{"State":T17, "Variable":variant} {"State"=enum."Return to Middle", "Variable"=variant}, error in (no error)=w5089) -> ()  [unwired: 1 in, 3 out]
          }
          event "Axis": Value Change {
            n1206 = event-data() -> ()  [unwired: 1 in, 6 out]
            n1207 = Bundle By Name(cluster=cluster{"State":T17, "Variable":variant} {"State"=enum."Axis", "Variable"=variant}, "Variable"="Axis") -> (w5093:cluster{"State":T17, "Variable":variant})
            n1208 = Enqueue Element(queue=w5096, element=w5093, error in (no error)=w5092) -> ()  [unwired: 1 in, 3 out]
          }
          event "Acceleration": Value Change {
            n1209 = event-data() -> ()  [unwired: 1 in, 6 out]
            n1210 = Bundle By Name(cluster=cluster{"State":T17, "Variable":variant} {"State"=enum."Acceleration", "Variable"=variant}, "Variable"="Acceleration") -> (w5099:cluster{"State":T17, "Variable":variant})
            n1211 = Enqueue Element(queue=w5101, element=w5099, error in (no error)=w5098) -> ()  [unwired: 1 in, 3 out]
          }
          event "Deceleration": Value Change {
            n1212 = event-data() -> ()  [unwired: 1 in, 6 out]
            n1213 = Bundle By Name(cluster=cluster{"State":T17, "Variable":variant} {"State"=enum."Deceleration", "Variable"=variant}, "Variable"="Deceleration") -> (w5104:cluster{"State":T17, "Variable":variant})
            n1214 = Enqueue Element(queue=w5106, element=w5104, error in (no error)=w5103) -> ()  [unwired: 1 in, 3 out]
          }
          event "Speed": Value Change {
            n1215 = event-data() -> ()  [unwired: 1 in, 6 out]
            n1216 = Bundle By Name(cluster=cluster{"State":T17, "Variable":variant} {"State"=enum."Speed", "Variable"=variant}, "Variable"="Speed") -> (w5109:cluster{"State":T17, "Variable":variant})
            n1217 = Enqueue Element(queue=w5111, element=w5109, error in (no error)=w5108) -> ()  [unwired: 1 in, 3 out]
          }
          event "Distance": Value Change {
            n1218 = event-data() -> ()  [unwired: 1 in, 6 out]
            n1219 = Bundle By Name(cluster=cluster{"State":T17, "Variable":variant} {"State"=enum."Distance", "Variable"=variant}, "Variable"="Distance") -> (w5114:cluster{"State":T17, "Variable":variant})
            n1220 = Enqueue Element(queue=w5116, element=w5114, error in (no error)=w5113) -> ()  [unwired: 1 in, 3 out]
          }
          event "Move Mode": Value Change {
            n1221 = event-data() -> ()  [unwired: 1 in, 6 out]
            n1222 = Bundle By Name(cluster=cluster{"State":T17, "Variable":variant} {"State"=enum."Move Mode", "Variable"=variant}, "Variable"="Move Mode") -> (w5119:cluster{"State":T17, "Variable":variant})
            n1223 = Enqueue Element(queue=w5121, element=w5119, error in (no error)=w5118) -> ()  [unwired: 1 in, 3 out]
          }
          event "Move Method": Value Change {
            n1224 = event-data() -> ()  [unwired: 1 in, 6 out]
            n1225 = Bundle By Name(cluster=cluster{"State":T17, "Variable":variant} {"State"=enum."Move Method", "Variable"=variant}, "Variable"="Move Method") -> (w5124:cluster{"State":T17, "Variable":variant})
            n1226 = Enqueue Element(queue=w5126, element=w5124, error in (no error)=w5123) -> ()  [unwired: 1 in, 3 out]
          }
          event "Direct of movement": Value Change {
            n1227 = event-data() -> ()  [unwired: 1 in, 6 out]
            n1228 = Bundle By Name(cluster=cluster{"State":T17, "Variable":variant} {"State"=enum."Direct of Movement", "Variable"=variant}, "Variable"="Direct of movement") -> (w5129:cluster{"State":T17, "Variable":variant})
            n1229 = Enqueue Element(queue=w5131, element=w5129, error in (no error)=w5128) -> ()  [unwired: 1 in, 3 out]
          }
          event "Angle": Value Change {
            n1230 = event-data() -> ()  [unwired: 1 in, 6 out]
            n1231 = Bundle By Name(cluster=cluster{"State":T17, "Variable":variant} {"State"=enum."Angle", "Variable"=variant}, "Variable"="Angle") -> (w5134:cluster{"State":T17, "Variable":variant})
            n1232 = Enqueue Element(queue=w5136, element=w5134, error in (no error)=w5133) -> ()  [unwired: 1 in, 3 out]
          }
        }
      }
      n1233 = while {
        tunnel: w94 -> [w3384]
        tunnel: w90 -> [w3385]
        shift-right: [w3382] -> _
        shift-left: w101 -> [w3383]
        stop <- w3379 stop-if-true
        n1234 = local read "Cluster"() -> (w3381:cluster{"tester  A":bool, " tester B":bool})
        n1235 = Unbundle(w3381) -> ("tester  A"=w3380:bool)  [unwired: 1 out]
        n1236 = case shown="True" w3380 {
          tunnel: w3385 -> [_ w3397]
          tunnel: w3384 -> [_ w3396]
          tunnel: w3383 -> [w3386 w3390]
          tunnel: [w3386 w3389] -> w3382
          tunnel: [_ w3387] -> w3379
          frame False {
          }
          frame True {
            n1237 = Dequeue Element(queue=w3396, error in (no error)=w3397) -> (queue out=w3393:refnum<queue>, element=w3395:T19, error out=w3392:errorcluster)  [unwired: 1 in, 1 out]
            n1238 = property on="TCP?" class="Bool (strict)"() -> ("Value"=w3388:bool)  [unwired: 2 in, 2 out]
            n1239 = Unbundle(w3395) -> (w3394:T30, "variant"=w3391:variant)
            n1240 = case shown="\"Convert\"" w3394 {
              tunnel: w3393 -> [_ w3405 _ w3433 w3516 w3560 w3598 w3624 w3633 w3642 w3651 w3660 w3669 _ w3737 w3788 _ _ _ _ w3856]
              tunnel: w3392 -> [_ w3403 _ w3434 w3514 w3558 w3594 w3632 w3641 w3650 w3659 w3668 w3677 w3680 w3702 w3781 w3813 _ w3824 w3829 w3861]
              tunnel: w3391 -> [_ w3404 _ _ w3506 w3548 w3591 w3631 w3640 w3649 w3658 w3667 w3676 w3683 w3740 w3791 w3818 _ w3825 _ _]
              tunnel: w3390 -> [w3398 w3402 w3422 w3430 w3507 w3551 w3593 w3629 w3638 w3647 w3656 w3665 w3675 w3684 w3707 w3786 w3815 w3819 w3822 w3830 w3860]
              tunnel: [w3398 w3401 w3422 w3432 w3512 w3556 w3600 w3628 w3637 w3646 w3655 w3664 w3674 w3684 w3739 w3790 w3817 w3819 w3821 w3830 w3859] -> w3389
              tunnel: w3388 -> [_ _ _ w3429 w3504 w3546 w3589 _ _ _ _ _ _ w3678 w3705 w3782 _ _ _ w3828 w3854]
              tunnel: [_ _ _ _ _ _ _ _ _ _ _ _ _ _ _ _ _ _ _ TRUE _] -> w3387
              frame "Idle", Default {
              }
              frame "auto mode" {
                n1241 = Unbundle By Name(w3402) -> ("auto test"=w3400:bool)
                n1242 = Not(x=w3400) -> (.not. x?=w3399:bool)
                n1243 = case shown="True" w3399 {
                  tunnel: w3405 -> [_ w3416]
                  tunnel: w3404 -> [_ w3413]
                  tunnel: w3403 -> [_ w3412]
                  frame False {
                  }
                  frame True {
                    n1244 = Variant To Data(error in=w3412, type=T10 {"Target 1"={"Boolean"=FALSE, "Speed"=0.0, "Range"=0.0, "Gain"=0.0}, "Target 2"={"Boolean"=FALSE, "Speed"=0.0, "Range"=0.0, "Gain"=0.0}, "Target 3"={"Boolean"=FALSE, "Speed"=0.0, "Range"=0.0, "Gain"=0.0}, "Target 4"={"Boolean"=FALSE, "Speed"=0.0, "Range"=0.0, "Gain"=0.0}} ("Direct program"), Variant=w3413) -> (data=w3410:T10, error out=w3411:errorcluster)
                    n1245 = Bundle By Name(cluster=T19 {enum."Direct Program", "variant"=variant}, "variant"=w3410) -> (w3409:T19)
                    n1246 = Build Array (concatenate)(T19[] [{enum."Inst. Connect", "variant"=variant}, {enum."Freq. (GHz)", "variant"=variant}], w3409, T19[] [{enum."Convert", "variant"=variant}, {enum."RF ON/OFF", "variant"=variant}]) -> (w3407:T19[])
                    n1247 = for {
                      tunnel: w3416 -> [w3419]
                      tunnel: w3411 -> [w3418]
                      tunnel: w3407 -> [w3417] mode=indexing
                      n1248 = Enqueue Element(queue=w3419, element=w3417, error in (no error)=w3418) -> ()  [unwired: 1 in, 3 out]
                    }
                  }
                }
                n1249 = Bundle By Name(cluster=w3402, "auto test"=w3399) -> (w3401:T15)
              }
              frame "Inst. Update" {
                n1250 = Unbundle By Name(w3422) -> ("Dynamic"=w3423:T9, "Mapping"=w3424:cluster{"4:4":bool, "4:2":bool, "4:1":bool}, "GRX (dB)"=w3425:dbl, "GTX (dB)"=w3427:dbl, "Freq. (GHz)"=w3426:dbl, "Inst. Status"=→"Inst. Status":bool, "String"=→"String":string)
                n1251 = property on="Freq. (GHz)" class="DigNum (strict)"("Value"=w3426) -> ()  [unwired: 2 in, 2 out]
                n1252 = property on="GTX (dB)" class="DigNum (strict)"("Value"=w3427) -> ()  [unwired: 2 in, 2 out]
                n1253 = property on="GRX (dB)" class="DigNum (strict)"("Value"=w3425) -> ()  [unwired: 2 in, 2 out]
                n1254 = property on="Mapping" class="Clust (strict)"("Value"=w3424) -> ()  [unwired: 2 in, 2 out]
                n1255 = property on="Dynamic1" class="Clust (strict)"("Value"=w3423) -> ()  [unwired: 2 in, 2 out]
                n1256 = Unbundle By Name(w3422) -> ("Direct program"=w3421:T10)
                n1257 = property on="Direct program" class="Clust (strict)"("Value"=w3421) -> ()  [unwired: 2 in, 2 out]
              }
              frame "Inst. Connect" {
                n1258 = Unbundle By Name(w3430) -> ("Inst. Status"=w3431:bool)
                n1259 = case shown="False" w3431 {
                  tunnel: w3434 -> [_ w3442]
                  tunnel: w3433 -> [_ w3436]
                  tunnel: [w3435 w3439] -> w3432
                  tunnel: w3430 -> [w3435 w3438]
                  tunnel: w3429 -> [_ w3437]
                  frame True {
                  }
                  frame False {
                    n1260 = Empty String/Path?(string/path="Inst. Connect IP") -> (empty?=w3444:bool)
                    n1261 = case shown="False" w3444 {
                      tunnel: "Inst. Connect IP" -> [w3456 _]
                      tunnel: w3442 -> [w3455 w3499]
                      tunnel: [w3454 w3499] -> w3441
                      tunnel: w3438 -> [w3453 w3498]
                      tunnel: [w3452 w3497] -> w3439
                      tunnel: w3437 -> [w3446 _]
                      tunnel: w3436 -> [w3445 _]
                      frame False {
                        n1262 = case shown="True" w3446 {
                          tunnel: w3456 -> [w3461 w3495]
                          tunnel: w3455 -> [w3463 w3494]
                          tunnel: [w3459 w3490] -> w3454
                          tunnel: [w3458 w3493] -> w3451
                          tunnel: w3445 -> [_ w3491]
                          frame True {
                            n1263 = Concatenate Strings("connect," ("string"), w3461) -> (w3460:string)
                            n1264 = disable-structure shown="Enabled" {
                              disable-tunnel: w3463 -> [w3469 w3485]
                              disable-tunnel: w3460 -> [w3467 w3484]
                              disable-tunnel: [w3465 w3483] -> w3459
                              disable-tunnel: [w3464 w3482] -> w3457
                              frame Disabled {
                                n1265 = call "client_FGV.vi"("data in"=w3467, "error constant"=w3469, "Enum"=enum16{"open", "idle", "write", "read", "close"}."write") -> ("error constant 2"=w3466:errorcluster)  [unwired: 7 in, 1 out]
                                n1266 = while {
                                tunnel: w3466 -> [w3480]
                                tunnel: [w3471] -> w3465
                                tunnel: [w3470] -> w3464
                                i -> [w3473]
                                stop <- w3475 stop-if-true
                                n1267 = call "client_FGV.vi"("error constant"=w3480, "Enum"=enum16{"open", "idle", "write", "read", "close"}."read") -> ("error constant 2"=w3471:errorcluster, "data out"=w3470:string)  [unwired: 8 in]
                                n1268 = String Length(string=w3470) -> (length=w3477:i32)
                                n1269 = Greater Than 0?(x=w3477) -> (x > 0?=w3476:bool)
                                n1270 = Greater?(x=w3473, y=600) -> (0:w3474:bool)
                                n1271 = Or(x=w3474, y=w3476) -> (x .or. y?=w3475:bool)
                                n1272 = Wait (ms)(milliseconds to wait=u32 100) -> ()  [unwired: 1 out]
                                }
                              }
                              frame Enabled {
                                n1273 = call "client_sw.vi"("receive?"=TRUE, "data in"=w3484, "error constant"=w3485, "port"=u16 6340) -> ("error constant 2"=w3483:errorcluster, "data out"=w3482:string)  [unwired: 6 in]
                              }
                            }
                            n1274 = Decimal String To Number(string=w3457) -> (number=w3458:i32)  [unwired: 2 in, 1 out]
                          }
                          frame False, Default {
                            n1275 = property on="Freq. (GHz)" class="DigNum (strict)"() -> ("Value"=w3487:dbl)  [unwired: 2 in, 2 out]
                            n1276 = dll-call lib="D:/0717/0717/Radar - 2015 32bit_autoqueue_angle_0319/Debug 2/Test_ARTS_1.dll" fn="?_connect@@YAHPAD@Z"(error in=w3494, "serverIPaddr"=w3495) -> (error out=w3492:errorcluster, "return type"=w3493:i32)  [unwired: 3 in, 1 out]
                            n1277 = Bundle By Name(cluster=T19 {enum."Freq. (GHz)", "variant"=variant}, "variant"=w3487) -> (w3488:T19)
                            n1278 = Enqueue Element(queue=w3491, element=w3488, error in (no error)=w3492) -> (error out=w3490:errorcluster)  [unwired: 1 in, 2 out]
                          }
                        }
                        n1279 = Greater Than 0?(x=w3451) -> (x > 0?=w3448:bool)
                        n1280 = Select(t="connected" ("String"), s=w3448, f="connect fail" ("String")) -> (s? t:f=w3447:string)
                        n1281 = Bundle By Name(cluster=w3453, "Inst. Status"=w3448, "String"=w3447) -> (w3452:T15)
                      }
                      frame True {
                        n1282 = Bundle By Name(cluster=w3498, "String"="connect fail") -> (w3497:T15)
                      }
                    }
                    n1283 = Enqueue Element(queue=w3436, element=T19 {enum."Inst. Update", "variant"=variant}, error in (no error)=w3441) -> ()  [unwired: 1 in, 3 out]
                  }
                }
              }
              frame "RF ON/OFF" {
                n1284 = Unbundle By Name(w3507) -> ("auto test"=w3508:bool)
                n1285 = Variant To Data(type=TRUE, Variant=w3506) -> (data=w3503:bool)  [unwired: 1 in, 1 out]
                n1286 = Boolean To (0,1)(Boolean=w3503) -> (0, 1=w3509:i16)
                n1287 = property on="RF ON/OFF" class="Bool (strict)"("Value"=w3503) -> ()  [unwired: 2 in, 2 out]
                n1288 = case shown="True" w3504 {
                  tunnel: w3514 -> [w3525 w3537]
                  tunnel: [w3520 w3536] -> w3513
                  tunnel: [1 w3535] -> w3502
                  tunnel: w3509 -> [w3524 w3534]
                  frame True {
                    n1289 = Number To Decimal String(number=w3524) -> (decimal integer string=w3523:string)  [unwired: 1 in]
                    n1290 = Concatenate Strings("rfon,", w3523) -> (w3521:string)
                    n1291 = disable-structure shown="Enabled" {
                      disable-tunnel: w3525 -> [w3529 w3531]
                      disable-tunnel: [w3528 w3530] -> w3520
                      disable-tunnel: w3521 -> [w3526 w3532]
                      frame Disabled {
                        n1292 = call "client_FGV.vi"("data in"=w3526, "error constant"=w3529, "Enum"=enum16{"open", "idle", "write", "read", "close"}."write") -> ("error constant 2"=w3528:errorcluster)  [unwired: 7 in, 1 out]
                      }
                      frame Enabled {
                        n1293 = call "client_sw.vi"("data in"=w3532, "error constant"=w3531, "port"=u16 6340) -> ("error constant 2"=w3530:errorcluster)  [unwired: 7 in, 1 out]
                      }
                    }
                  }
                  frame False, Default {
                    n1294 = dll-call lib="D:/0717/0717/Radar - 2015 32bit_autoqueue_angle_0319/Debug 2/Test_ARTS_1.dll" fn="?_SetSynthRFOutput@@YAHH@Z"(error in=w3537, "irfoutput"=w3534) -> (error out=w3536:errorcluster, "return type"=w3535:i32)  [unwired: 3 in, 1 out]
                  }
                }
                n1295 = property on="auto step finish?" class="Bool (strict)"() -> ("Value"=w3500:bool)  [unwired: 2 in, 2 out]
                n1296 = Greater Than 0?(x=w3502) -> (x > 0?=w3511:bool)
                n1297 = Not(x=w3500) -> (.not. x?=w3501:bool)
                n1298 = case shown="True" w3511 {
                  tunnel: ["run fail" ("String") "run ok" ("String")] -> w3510
                  frame False {
                  }
                  frame True {
                  }
                }
                n1299 = case shown="True" w3501 {
                  tunnel: w3502 -> [_ w3518]
                  frame False {
                  }
                  frame True {
                    n1300 = Greater Than 0?(x=w3518) -> (x > 0?=w3517:bool)
                    n1301 = property on="autoRSfinish?" class="Bool (strict)"("Value"=w3517) -> ()  [unwired: 2 in, 2 out]
                  }
                }
                n1302 = Bundle By Name(cluster=w3507, "String"=w3510) -> (w3512:T15)
                n1303 = case shown="False" w3508 {
                  tunnel: w3516 -> [w3540 w3543]
                  tunnel: T19 {enum."Inst. Update", "variant"=variant} -> [w3538 w3542]
                  tunnel: w3513 -> [w3539 w3541]
                  frame True {
                    n1304 = Enqueue Element At Opposite End(queue=w3540, element=w3538, error in (no error)=w3539) -> ()  [unwired: 1 in, 3 out]
                  }
                  frame False {
                    n1305 = Enqueue Element(queue=w3543, element=w3542, error in (no error)=w3541) -> ()  [unwired: 1 in, 3 out]
                  }
                }
              }
              frame "Convert" {
                (unwired) TRUE
                n1306 = Unbundle By Name(w3551) -> ("auto test"=w3550:bool)
                n1307 = Variant To Data(type=TRUE, Variant=w3548) -> (data=w3547:bool)  [unwired: 1 in, 1 out]
                n1308 = Boolean To (0,1)(Boolean=w3547) -> (0, 1=w3552:i16)
                n1309 = property on="T/R Converters" class="Bool (strict)"("Value"=w3547) -> ()  [unwired: 2 in, 2 out]
                n1310 = case shown="True" w3546 {
                  tunnel: w3558 -> [w3565 w3579]
                  tunnel: [w3563 w3578] -> w3557
                  tunnel: [1 ("return type") w3577] -> w3554
                  tunnel: w3552 -> [w3562 w3576]
                  frame True {
                    n1311 = Number To Decimal String(number=w3562) -> (decimal integer string=w3567:string)  [unwired: 1 in]
                    n1312 = Concatenate Strings("convert,", w3567) -> (w3561:string)
                    n1313 = disable-structure shown="Enabled" {
                      disable-tunnel: w3565 -> [w3570 w3574]
                      disable-tunnel: [w3569 w3573] -> w3563
                      disable-tunnel: w3561 -> [w3568 w3572]
                      frame Disabled {
                        n1314 = call "client_FGV.vi"("data in"=w3568, "error constant"=w3570, "Enum"=enum16{"open", "idle", "write", "read", "close"}."write") -> ("error constant 2"=w3569:errorcluster)  [unwired: 7 in, 1 out]
                      }
                      frame Enabled {
                        n1315 = call "client_sw.vi"("data in"=w3572, "error constant"=w3574, "port"=u16 6340) -> ("error constant 2"=w3573:errorcluster)  [unwired: 7 in, 1 out]
                      }
                    }
                  }
                  frame False, Default {
                    n1316 = dll-call lib="D:/0717/0717/Radar - 2015 32bit_autoqueue_angle_0319/Debug 2/Test_ARTS_1.dll" fn="?_SetTrEn@@YAHH@Z"(error in=w3579, "ienable"=w3576) -> (error out=w3578:errorcluster, "return type"=w3577:i32)  [unwired: 3 in, 1 out]
                  }
                }
                n1317 = Greater Than 0?(x=w3554) -> (x > 0?=w3555:bool)
                n1318 = case shown="True" w3555 {
                  tunnel: ["run fail" ("String") "convert ok" ("String")] -> w3553
                  frame False {
                  }
                  frame True {
                  }
                }
                n1319 = Bundle By Name(cluster=w3551, "String"=w3553) -> (w3556:T15)
                n1320 = case shown="False" w3550 {
                  tunnel: w3560 -> [w3581 w3585]
                  tunnel: T19 {enum."Inst. Update", "variant"=variant} -> [w3580 w3584]
                  tunnel: w3557 -> [w3582 w3583]
                  frame True {
                    n1321 = Enqueue Element At Opposite End(queue=w3581, element=w3580, error in (no error)=w3582) -> ()  [unwired: 1 in, 3 out]
                  }
                  frame False {
                    n1322 = Enqueue Element(queue=w3585, element=w3584, error in (no error)=w3583) -> ()  [unwired: 1 in, 3 out]
                  }
                }
              }
              frame "Freq. (GHz)" {
                n1323 = Unbundle By Name(w3593) -> ("auto test"=w3592:bool)
                n1324 = Variant To Data(type=0.0, Variant=w3591) -> (data=w3588:dbl)  [unwired: 1 in, 1 out]
                n1325 = Multiply(x=w3588, y=1000.0) -> (x*y=w3595:dbl)
                n1326 = case shown="True" w3589 {
                  tunnel: [w3606 w3617] -> w3597
                  tunnel: w3595 -> [_ w3616]
                  tunnel: w3594 -> [w3605 w3615]
                  tunnel: w3588 -> [w3602 _]
                  frame True {
                    n1327 = Number To Fractional String(number=w3602) -> (F-format string=w3604:string)  [unwired: 3 in]
                    n1328 = Concatenate Strings("freq," ("string"), w3604) -> (w3601:string)
                    n1329 = disable-structure shown="Enabled" {
                      disable-tunnel: [w3610 w3612] -> w3606
                      disable-tunnel: w3605 -> [w3609 w3613]
                      disable-tunnel: w3601 -> [w3607 w3611]
                      frame Disabled {
                        n1330 = call "client_FGV.vi"("data in"=w3607, "error constant"=w3609, "Enum"=enum16{"open", "idle", "write", "read", "close"}."write") -> ("error constant 2"=w3610:errorcluster)  [unwired: 7 in, 1 out]
                      }
                      frame Enabled {
                        n1331 = call "client_sw.vi"("data in"=w3611, "error constant"=w3613, "port"=u16 6340) -> ("error constant 2"=w3612:errorcluster)  [unwired: 7 in, 1 out]
                      }
                    }
                  }
                  frame False, Default {
                    n1332 = dll-call lib="D:/0717/0717/Radar - 2015 32bit_autoqueue_angle_0319/Debug 2/Test_ARTS_1.dll" fn="?_SetRfFreq_kHz@@YAHH@Z" label="SetRfFreq"(error in=w3615, "ichan"=w3616) -> (error out=w3617:errorcluster)  [unwired: 4 in, 1 out]
                  }
                }
                n1333 = Bundle By Name(cluster=w3593, "Freq. (GHz)"=w3588) -> (w3600:T15)
                n1334 = case shown="True" w3592 {
                  tunnel: T19 {enum."Inst. Update", "variant"=variant} -> [w3618 w3623]
                  tunnel: w3598 -> [w3620 w3622]
                  tunnel: w3597 -> [w3619 w3621]
                  frame True {
                    n1335 = Enqueue Element At Opposite End(queue=w3620, element=w3618, error in (no error)=w3619) -> ()  [unwired: 1 in, 3 out]
                  }
                  frame False {
                    n1336 = Enqueue Element(queue=w3622, element=w3623, error in (no error)=w3621) -> ()  [unwired: 1 in, 3 out]
                  }
                }
              }
              frame "GTX (dB)" {
                n1337 = Variant To Data(error in=w3632, type=0.0, Variant=w3631) -> (data=w3627:dbl, error out=w3625:errorcluster)
                n1338 = Bundle By Name(cluster=w3629, "GTX (dB)"=w3627) -> (w3628:T15)
                n1339 = Enqueue Element(queue=w3624, element=T19 {enum."Inst. Update", "variant"=variant}, error in (no error)=w3625) -> ()  [unwired: 1 in, 3 out]
              }
              frame "GRX (dB)" {
                n1340 = Variant To Data(error in=w3641, type=0.0, Variant=w3640) -> (data=w3636:dbl, error out=w3634:errorcluster)
                n1341 = Bundle By Name(cluster=w3638, "GRX (dB)"=w3636) -> (w3637:T15)
                n1342 = Enqueue Element(queue=w3633, element=T19 {enum."Inst. Update", "variant"=variant}, error in (no error)=w3634) -> ()  [unwired: 1 in, 3 out]
              }
              frame "Range Trim(m)" {
                n1343 = Variant To Data(error in=w3650, type=0.0, Variant=w3649) -> (data=w3645:dbl, error out=w3643:errorcluster)
                n1344 = Bundle By Name(cluster=w3647, "Range Trim (m)"=w3645) -> (w3646:T15)
                n1345 = Enqueue Element(queue=w3642, element=T19 {enum."Inst. Update", "variant"=variant}, error in (no error)=w3643) -> ()  [unwired: 1 in, 3 out]
              }
              frame "Gain Trim (dB)" {
                n1346 = Variant To Data(error in=w3659, type=0.0, Variant=w3658) -> (data=w3654:dbl, error out=w3652:errorcluster)
                n1347 = Bundle By Name(cluster=w3656, "Gain Trim (dB)"=w3654) -> (w3655:T15)
                n1348 = Enqueue Element(queue=w3651, element=T19 {enum."Inst. Update", "variant"=variant}, error in (no error)=w3652) -> ()  [unwired: 1 in, 3 out]
              }
              frame "Distance to RUT" {
                n1349 = Variant To Data(error in=w3668, type=0.0, Variant=w3667) -> (data=w3663:dbl, error out=w3661:errorcluster)
                n1350 = Bundle By Name(cluster=w3665, "Distance to RUT"=w3663) -> (w3664:T15)
                n1351 = Enqueue Element(queue=w3660, element=T19 {enum."Inst. Update", "variant"=variant}, error in (no error)=w3661) -> ()  [unwired: 1 in, 3 out]
              }
              frame "Mapping" {
                n1352 = Variant To Data(error in=w3677, type=cluster{"4:4":bool, "4:2":bool, "4:1":bool} {"4:4"=FALSE, "4:2"=FALSE, "4:1"=FALSE} ("Mapping"), Variant=w3676) -> (data=w3673:cluster{"4:4":bool, "4:2":bool, "4:1":bool}, error out=w3670:errorcluster)
                n1353 = Bundle By Name(cluster=w3675, "Mapping"=w3673) -> (w3674:T15)
                n1354 = Enqueue Element(queue=w3669, element=T19 {enum."Inst. Update", "variant"=variant}, error in (no error)=w3670) -> ()  [unwired: 1 in, 3 out]
              }
              frame "rx att" {
                n1355 = Variant To Data(error in=w3680, type=0.0, Variant=w3683) -> (data=w3681:dbl, error out=w3679:errorcluster)
                n1356 = case shown="True" w3678 {
                  tunnel: w3681 -> [w3688 w3701]
                  tunnel: w3679 -> [w3687 w3700]
                  tunnel: [w3686 w3699] -> _
                  frame True {
                    n1357 = Number To Fractional String(number=w3688) -> (F-format string=w3690:string)  [unwired: 3 in]
                    n1358 = Concatenate Strings("rxatt," ("string"), w3690) -> (w3685:string)
                    n1359 = disable-structure shown="Enabled" {
                      disable-tunnel: w3687 -> [w3693 w3696]
                      disable-tunnel: [w3692 w3695] -> w3686
                      disable-tunnel: w3685 -> [w3691 w3697]
                      frame Disabled {
                        n1360 = call "client_FGV.vi"("data in"=w3691, "error constant"=w3693, "Enum"=enum16{"open", "idle", "write", "read", "close"}."write") -> ("error constant 2"=w3692:errorcluster)  [unwired: 7 in, 1 out]
                      }
                      frame Enabled {
                        n1361 = call "client_sw.vi"("data in"=w3697, "error constant"=w3696, "port"=u16 6340) -> ("error constant 2"=w3695:errorcluster)  [unwired: 7 in, 1 out]
                      }
                    }
                  }
                  frame False, Default {
                    n1362 = dll-call lib="D:/0717/0717/Radar - 2015 32bit_autoqueue_angle_0319/Debug 2/Test_ARTS_1.dll" fn="?_SetRxAttn@@YAHN@Z" label="_SetRxAttn"(error in=w3700, "irxatt"=w3701) -> (error out=w3699:errorcluster)  [unwired: 4 in, 1 out]
                  }
                }
              }
              frame "Direct Program" {
                n1363 = Unbundle By Name(w3707) -> ("auto test"=w3706:bool)
                n1364 = Variant To Data(error in=w3702, type=T10 {"Target 1"={"Boolean"=FALSE, "Speed"=0.0, "Range"=0.0, "Gain"=0.0}, "Target 2"={"Boolean"=FALSE, "Speed"=0.0, "Range"=0.0, "Gain"=0.0}, "Target 3"={"Boolean"=FALSE, "Speed"=0.0, "Range"=0.0, "Gain"=0.0}, "Target 4"={"Boolean"=FALSE, "Speed"=0.0, "Range"=0.0, "Gain"=0.0}} ("Direct program"), Variant=w3740) -> (data=w3704:T10, error out=w3735:errorcluster)
                n1365 = Unbundle(w3704) -> ("Target 1"=w3733:T31, "Target 2"=w3732:T31, "Target 3"=w3731:T31, "Target 4"=w3730:T31)
                n1366 = Bundle By Name(cluster=w3707, "Direct program"=w3704) -> (w3739:T15)
                n1367 = Unbundle(w3733) -> ("Boolean"=w3713:bool, "Speed"=w3729:dbl, "Range"=w3728:dbl, "Gain"=w3727:dbl)
                n1368 = Unbundle(w3732) -> ("Boolean"=w3712:bool, "Speed"=w3726:dbl, "Range"=w3725:dbl, "Gain"=w3724:dbl)
                n1369 = Unbundle(w3731) -> ("Boolean"=w3711:bool, "Speed"=w3723:dbl, "Range"=w3722:dbl, "Gain"=w3721:dbl)
                n1370 = Unbundle(w3730) -> ("Boolean"=w3710:bool, "Speed"=w3720:dbl, "Range"=w3719:dbl, "Gain"=w3718:dbl)
                n1371 = Build Array(w3713, w3712, w3711, w3710) -> (w3715:bool[])
                n1372 = property on="auto step finish?" class="Bool (strict)"(error in=w3702) -> ("Value"=w3703:bool)  [unwired: 1 in, 2 out]
                n1373 = Boolean To (0,1)(Boolean=w3715) -> (0, 1=w3714:i16[])
                n1374 = case shown="False" w3703 {
                  frame False {
                    n1375 = property on="autoRSfinish?" class="Bool (strict)"("Value"=FALSE ("autoRS")) -> ()  [unwired: 2 in, 2 out]
                  }
                  frame True {
                  }
                }
                n1376 = Multiply(x=w3714, y=i32[] [1, 2, 4, 8]) -> (x*y=w3716:i32[])
                n1377 = Add Array Elements(numeric array=w3716) -> (sum=w3709:i32)
                n1378 = case shown="True" w3705 {
                  tunnel: w3735 -> [w3771 w3774]
                  tunnel: [w3771 w3773] -> w3734
                  tunnel: w3709 -> [_ w3772]
                  frame True {
                  }
                  frame False, Default {
                    n1379 = dll-call lib="D:/0717/0717/Radar - 2015 32bit_autoqueue_angle_0319/Debug 2/Test_ARTS_1.dll" fn="?_TxChanEnable@@YAHH@Z" label="TxChanEnable"(error in=w3774, "ichan"=w3772) -> (error out=w3773:errorcluster)  [unwired: 4 in, 1 out]
                  }
                }
                n1380 = case shown="True" w3705 {
                  tunnel: w3734 -> [w3744 w3770]
                  tunnel: w3729 -> [_ w3769]
                  tunnel: w3728 -> [_ w3768]
                  tunnel: w3727 -> [_ w3767]
                  tunnel: w3726 -> [_ w3766]
                  tunnel: w3725 -> [_ w3765]
                  tunnel: w3724 -> [_ w3764]
                  tunnel: w3723 -> [_ w3763]
                  tunnel: w3722 -> [_ w3762]
                  tunnel: w3721 -> [_ w3761]
                  tunnel: w3720 -> [_ w3760]
                  tunnel: w3719 -> [_ w3759]
                  tunnel: w3718 -> [_ w3758]
                  tunnel: [w3745 w3757] -> w3708
                  tunnel: w3704 -> [w3746 _]
                  frame True {
                    n1381 = call "Untitled 3.vi"("Boolean"=TRUE, "Direct program"=w3746) -> ("concatenated string"=w3747:string)  [unwired: 8 in, 1 out]
                    n1382 = Concatenate Strings("static," ("string"), w3747) -> (w3743:string)
                    n1383 = disable-structure shown="Enabled" {
                      disable-tunnel: [w3751 w3754] -> w3745
                      disable-tunnel: w3744 -> [w3750 w3755]
                      disable-tunnel: w3743 -> [w3749 w3753]
                      frame Disabled {
                        n1384 = call "client_FGV.vi"("data in"=w3749, "error constant"=w3750, "Enum"=enum16{"open", "idle", "write", "read", "close"}."write") -> ("error constant 2"=w3751:errorcluster)  [unwired: 7 in, 1 out]
                      }
                      frame Enabled {
                        n1385 = call "client_sw.vi"("data in"=w3753, "error constant"=w3755, "port"=u16 6340) -> ("error constant 2"=w3754:errorcluster)  [unwired: 7 in, 1 out]
                      }
                    }
                  }
                  frame False {
                    n1386 = dll-call lib="D:/0717/0717/Radar - 2015 32bit_autoqueue_angle_0319/Debug 2/Test_ARTS_1.dll" fn="?_SetTxChanStaticCfg@@YAHHHHHHHHHHHHH@Z" label="SetTxChanStaticCfg"(error in=w3770, "speed1"=w3769, "range1"=w3768, "gain1"=w3767, "speed2"=w3766, "range2"=w3765, "gain2"=w3764, "speed3"=w3763, "range3"=w3762, "gain3"=w3761, "speed4"=w3760, "range4"=w3759, "gain4"=w3758) -> (error out=w3757:errorcluster)  [unwired: 15 in, 1 out]
                  }
                }
                n1387 = case shown="False" w3706 {
                  tunnel: T19 {enum."Inst. Update", "variant"=variant} -> [w3775 w3780]
                  tunnel: w3737 -> [w3776 w3779]
                  tunnel: w3708 -> [w3777 w3778]
                  frame True {
                    n1388 = Enqueue Element At Opposite End(queue=w3776, element=w3775, error in (no error)=w3777) -> ()  [unwired: 1 in, 3 out]
                  }
                  frame False {
                    n1389 = Enqueue Element(queue=w3779, element=w3780, error in (no error)=w3778) -> ()  [unwired: 1 in, 3 out]
                  }
                }
              }
              frame "Dynamic" {
                n1390 = Variant To Data(error in=w3781, type=T9 {"Target 1"={"Boolean"=FALSE, "Start Speed (km/h)"=0.0, "Stop Speed (km/h)"=0.0, "Start Range(m)"=0.0, "Stop Range(m)"=0.0, "Start Gain(dB)"=0.0}, "Target 2"={"Boolean"=FALSE, "Start Speed (km/h)"=0.0, "Stop Speed (km/h)"=0.0, "Start Range(m)"=0.0, "Stop Range(m)"=0.0, "Start Gain(dB)"=0.0}, "Target 3"={"Boolean"=FALSE, "Start Speed (km/h)"=0.0, "Stop Speed (km/h)"=0.0, "Start Range(m)"=0.0, "Stop Range(m)"=0.0, "Start Gain(dB)"=0.0}, "Target 4"={"Boolean"=FALSE, "Start Speed (km/h)"=0.0, "Stop Speed (km/h)"=0.0, "Start Range(m)"=0.0, "Stop Range(m)"=0.0, "Start Gain(dB)"=0.0}} ("Dynamic"), Variant=w3791) -> (data=w3785:T9, error out=w3783:errorcluster)
                n1391 = case shown="True" w3782 {
                  tunnel: [w3797 w3811] -> w3784
                  tunnel: w3785 -> [w3794 w3809]
                  tunnel: w3783 -> [w3792 w3810]
                  frame True {
                    n1392 = call "dynamic.vi"("Boolean"=TRUE, "dynamic"=w3794) -> ("concatenated string"=w3793:string)  [unwired: 8 in, 1 out]
                    n1393 = Concatenate Strings("dynamic," ("string"), w3793) -> (w3796:string)
                    n1394 = disable-structure shown="Enabled" {
                      disable-tunnel: [w3801 w3804] -> w3797
                      disable-tunnel: w3796 -> [w3800 w3803]
                      disable-tunnel: w3792 -> [w3799 w3805]
                      frame Disabled {
                        n1395 = call "client_FGV.vi"("data in"=w3800, "error constant"=w3799, "Enum"=enum16{"open", "idle", "write", "read", "close"}."write") -> ("error constant 2"=w3801:errorcluster)  [unwired: 7 in, 1 out]
                      }
                      frame Enabled {
                        n1396 = call "client_sw.vi"("data in"=w3803, "error constant"=w3805, "port"=u16 6340) -> ("error constant 2"=w3804:errorcluster)  [unwired: 7 in, 1 out]
                      }
                    }
                  }
                  frame False {
                    n1397 = call "dynamicsub.vi"("error in (no error)"=w3810, "Dynamic"=w3809) -> ("error out"=w3811:errorcluster, "generateWF ok?"=w3808:i32)  [unwired: 8 in]
                    "generateWF ok?" <- w3808
                    n1398 = Greater Than 0?(x=w3808) -> (x > 0?=w3807:bool)
                    n1399 = case shown="True" w3807 {
                      frame False {
                      }
                      frame True {
                        w3812 = TRUE
                        n1400 = property on="Run/Stop" class="Bool (strict)"("Value"=w3812) -> ()  [unwired: 2 in, 2 out]
                        n1401 = property on="Status?" class="Bool (strict)"("Value"=w3812) -> ()  [unwired: 2 in, 2 out]
                      }
                    }
                  }
                }
                n1402 = Bundle By Name(cluster=w3786, "Dynamic"=w3785) -> (w3790:T15)
                n1403 = Enqueue Element(queue=w3788, element=T19 {enum."Inst. Update", "variant"=variant}, error in (no error)=w3784) -> ()  [unwired: 1 in, 3 out]
              }
              frame "dyset" {
                n1404 = Variant To Data(error in=w3813, type=T9 {"Target 1"={"Boolean"=FALSE, "Start Speed (km/h)"=0.0, "Stop Speed (km/h)"=0.0, "Start Range(m)"=0.0, "Stop Range(m)"=0.0, "Start Gain(dB)"=0.0}, "Target 2"={"Boolean"=FALSE, "Start Speed (km/h)"=0.0, "Stop Speed (km/h)"=0.0, "Start Range(m)"=0.0, "Stop Range(m)"=0.0, "Start Gain(dB)"=0.0}, "Target 3"={"Boolean"=FALSE, "Start Speed (km/h)"=0.0, "Stop Speed (km/h)"=0.0, "Start Range(m)"=0.0, "Stop Range(m)"=0.0, "Start Gain(dB)"=0.0}, "Target 4"={"Boolean"=FALSE, "Start Speed (km/h)"=0.0, "Stop Speed (km/h)"=0.0, "Start Range(m)"=0.0, "Stop Range(m)"=0.0, "Start Gain(dB)"=0.0}} ("Dynamic"), Variant=w3818) -> (data=w3814:T9)  [unwired: 1 out]
                n1405 = Bundle By Name(cluster=w3815, "Dynamic"=w3814) -> (w3817:T15)
              }
              frame "Run" {
              }
              frame "£m Data" {
                n1406 = Variant To Data(error in=w3824, type=dbl[][] [], Variant=w3825) -> (data=w3820:dbl[][])  [unwired: 1 out]
                n1407 = Bundle By Name(cluster=w3822, "£m Data"=w3820) -> (w3821:T15)
              }
              frame "Exit" {
                n1408 = case shown="True" w3828 {
                  tunnel: w3829 -> [w3833 w3852]
                  tunnel: [w3838 w3850] -> w3827
                  frame True {
                    n1409 = Number To Decimal String(number=0 ("return type")) -> (decimal integer string=w3837:string)  [unwired: 1 in]
                    n1410 = Concatenate Strings("rfon,", w3837) -> (w3835:string)
                    n1411 = call "client_sw.vi"("data in"=w3835, "error constant"=w3833, "port"=u16 6340) -> ("error constant 2"=w3832:errorcluster)  [unwired: 7 in, 1 out]
                    n1412 = Concatenate Strings("close," ("string"), "ok" ("string")) -> (w3839:string)
                    n1413 = disable-structure shown="Enabled" {
                      disable-tunnel: w3832 -> [w3845 w3848]
                      disable-tunnel: w3839 -> [w3843 w3846]
                      disable-tunnel: [w3842 w3847] -> w3838
                      frame Disabled {
                        n1414 = call "client_FGV.vi"("data in"=w3843, "error constant"=w3845, "Enum"=enum16{"open", "idle", "write", "read", "close"}."write") -> ("error constant 2"=w3842:errorcluster)  [unwired: 7 in, 1 out]
                      }
                      frame Enabled {
                        n1415 = call "client_sw.vi"("data in"=w3846, "error constant"=w3848, "port"=u16 6340) -> ("error constant 2"=w3847:errorcluster)  [unwired: 7 in, 1 out]
                      }
                    }
                  }
                  frame False {
                    n1416 = dll-call lib="D:/0717/0717/Radar - 2015 32bit_autoqueue_angle_0319/Debug 2/Test_ARTS_1.dll" fn="?_SetSynthRFOutput@@YAHH@Z"(error in=w3852, "irfoutput"=0) -> (error out=w3853:errorcluster)  [unwired: 4 in, 1 out]
                    n1417 = dll-call lib="D:/0717/0717/Radar - 2015 32bit_autoqueue_angle_0319/Debug 2/Test_ARTS_1.dll" fn="?_disconnect@@YAHXZ"(error in=w3853) -> (error out=w3850:errorcluster)  [unwired: 3 in, 1 out]
                  }
                }
                n1418 = call <vilib>:"Clear Errors.vi"("error in (no error)"=w3827) -> ()  [unwired: 5 in, 2 out]
              }
              frame "Stop" {
                n1419 = case shown="True" w3854 {
                  tunnel: w3861 -> [w3864 w3877]
                  tunnel: [w3863 w3875] -> w3855
                  frame True {
                    n1420 = Concatenate Strings("close," ("string"), "ok" ("string")) -> (w3862:string)
                    n1421 = disable-structure shown="Enabled" {
                      disable-tunnel: w3864 -> [w3869 w3873]
                      disable-tunnel: [w3868 w3872] -> w3863
                      disable-tunnel: w3862 -> [w3867 w3871]
                      frame Disabled {
                        n1422 = call "client_FGV.vi"("data in"=w3867, "error constant"=w3869, "Enum"=enum16{"open", "idle", "write", "read", "close"}."write") -> ("error constant 2"=w3868:errorcluster)  [unwired: 7 in, 1 out]
                      }
                      frame Enabled {
                        n1423 = call "client_sw.vi"("data in"=w3871, "error constant"=w3873, "port"=u16 6340) -> ("error constant 2"=w3872:errorcluster)  [unwired: 7 in, 1 out]
                      }
                    }
                  }
                  frame False {
                    n1424 = dll-call lib="D:/0717/0717/Radar - 2015 32bit_autoqueue_angle_0319/Debug 2/Test_ARTS_1.dll" fn="?_SetSynthRFOutput@@YAHH@Z"(error in=w3877, "irfoutput"=0) -> (error out=w3878:errorcluster)  [unwired: 4 in, 1 out]
                    n1425 = dll-call lib="D:/0717/0717/Radar - 2015 32bit_autoqueue_angle_0319/Debug 2/Test_ARTS_1.dll" fn="?_disconnect@@YAHXZ"(error in=w3878) -> (error out=w3875:errorcluster)  [unwired: 3 in, 1 out]
                  }
                }
                n1426 = Bundle By Name(cluster=w3860, "Inst. Status"=FALSE) -> (w3859:T15)
                n1427 = Enqueue Element(queue=w3856, element=T19 {enum."Inst. Update", "variant"=variant}, error in (no error)=w3855) -> ()  [unwired: 1 in, 3 out]
              }
            }
          }
        }
      }
      n1428 = call <vilib>:"Application Directory.vi"() -> ("Application Directory"=w102:path)
      n1429 = while {
        stop <- w112 stop-if-true
        n1430 = call <vilib>:"Application Directory.vi"() -> ("Application Directory"=w113:path)
        n1431 = case shown="True" "Server" {
          tunnel: w113 -> [_ w116]
          frame False {
          }
          frame True {
            n1432 = call "callRsgui.vi"("path"=w116) -> ()  [unwired: 11 in]
            n1433 = property on="Server" class="Bool (strict)"("Value"=FALSE ("Server")) -> ()  [unwired: 2 in, 2 out]
          }
        }
        n1434 = property on="Exit" class="Bool (strict)"() -> ("Value"=w112:bool)  [unwired: 2 in, 2 out]
      }
      n1435 = while {
        tunnel: w94 -> [w409]
        tunnel: w93 -> [w408]
        tunnel: w90 -> [w405]
        tunnel: w91 -> [w404]
        tunnel: w89 -> [w403]
        stop <- w406 stop-if-true
        n1436 = case shown="True" "RUN" {
          tunnel: w409 -> [_ w432]
          tunnel: w408 -> [_ w421]
          tunnel: w405 -> [_ w428]
          tunnel: w404 -> [_ w427]
          tunnel: w403 -> [_ w422]
          frame False {
          }
          frame True {
            n1437 = flat-sequence {
              tunnel: w428 -> [w436]
              tunnel: w421 -> [w437]
              tunnel: w432 -> [w438]
              tunnel: [w438] -> w425
              tunnel: [w437] -> w424
              tunnel: [w435] -> w423
              tunnel: w422 -> [w434]
              tunnel: [w464] -> w433
              tunnel: [w463] -> w431
              tunnel: [w462] -> w430
              tunnel: [w461] -> w429
              tunnel: [w458] -> w426
              tunnel: w425 -> [w464]
              tunnel: w424 -> [w463]
              tunnel: w423 -> [w461]
              tunnel: w433 -> [w487]
              tunnel: w431 -> [w497]
              tunnel: w430 -> [w474]
              tunnel: w429 -> [w486]
              tunnel: w427 -> [w490]
              tunnel: w426 -> [w473]
              tunnel: [w480] -> w419
              tunnel: [w482] -> w418
              tunnel: [w483] -> w417
              tunnel: [w481] -> w416
              tunnel: [w480] -> w415
              tunnel: [w478] -> w412
              tunnel: w419 -> [w591]
              tunnel: w418 -> [w592]
              tunnel: w417 -> [w589]
              tunnel: w416 -> [w587]
              tunnel: w415 -> [w586]
              tunnel: [w591] -> w414
              tunnel: [w585] -> w413
              tunnel: w412 -> [w585]
              tunnel: w414 -> [w602]
              tunnel: w413 -> [w605]
              tunnel: [w602] -> w410
              tunnel: [w607] -> w420
              tunnel: w410 -> [w607]
              frame #0 {
                n1438 = disable-structure shown="Enabled" {
                  disable-tunnel: w436 -> [w441 w443]
                  disable-tunnel: [w440 w443] -> w435
                  disable-tunnel: w434 -> [w439 _]
                  frame Disabled {
                    n1439 = Enqueue Element(queue=w439, element=T18 {"State"=enum."Report Dist", "variant"=variant}, error in (no error)=w441) -> (error out=w440:errorcluster)  [unwired: 1 in, 2 out]
                  }
                  frame Enabled {
                  }
                }
              }
              frame #1 {
                w459 = 0.0 ("num")
                n1440 = property on="Direct program2" class="Clust (strict)"() -> ("Value"=w466:T10)  [unwired: 2 in, 2 out]
                n1441 = property on="Dynamic2" class="Clust (strict)"() -> ("Value"=w456:T9)  [unwired: 2 in, 2 out]
                n1442 = property on="Dynamic1" class="Clust (strict)"() -> ("Value"=w457:T9)  [unwired: 2 in, 2 out]
                n1443 = property on="RCS def" class="DigNum (strict)"() -> ("Value"=w453:dbl)  [unwired: 2 in, 2 out]
                n1444 = property on="RCS def 2" class="DigNum (strict)"() -> ("Value"=w452:dbl)  [unwired: 2 in, 2 out]
                n1445 = property on="Direct program" class="Clust (strict)"() -> ("Value"=w467:T10)  [unwired: 2 in, 2 out]
                n1446 = Bundle("Value"=w457, "Value"=w456) -> (w455:T33)  [unwired: 1 in]
                n1447 = Bundle("Value"=w453, "Value"=w452) -> (w451:cluster{"Value":dbl, "Value":dbl})  [unwired: 1 in]
                n1448 = Bundle("Value"=w467, "Value"=w466) -> (w468:T34)  [unwired: 1 in]
                n1449 = property on="DYNAMIC 2" class="Arr (strict)"() -> ("Value"=w444:T1)  [unwired: 2 in, 2 out]
                n1450 = property on="Array" class="Arr (strict)"() -> ("Value"=w465:T2)  [unwired: 2 in, 2 out]
                n1451 = property on="DYNAMIC" class="Arr (strict)"() -> ("Value"=w454:T1)  [unwired: 2 in, 2 out]
                n1452 = Bundle("RCS A"="RCS A", "RCS B"="RCS B") -> (w448:cluster{"RCS A":dbl, "RCS B":dbl})  [unwired: 1 in]
                n1453 = Bundle("B dist. comp"="B dist. comp", "A dist. comp"="A dist. comp") -> (w445:cluster{"B dist. comp":dbl, "A dist. comp":dbl})  [unwired: 1 in]
                n1454 = call "point to dist.vi"("Array 2"=w465, "lock rcs value"=w448, "dist compensate"=w445, "lock RCS"="lock RCS", "Cluster in"=w468, "output cluster"=w455, "RCS"=w451, "DYNAMIC"=w454, "DYNAMIC 2"=w444) -> ("xy dynamic array"=w458:T35, "1to4"=w462:T36)  [unwired: 2 in, 3 out]
                "Path B" <- w459
                "Path A" <- w459
              }
              frame #2 {
                n1455 = Index Array(array=w473) -> (element #1=w472:T37, element #2=w470:T37)  [unwired: 4 in]
                n1456 = Index Array(array=w470) -> (element=w469:T9)  [unwired: 1 in]
                n1457 = Index Array(array=w472) -> (element=w471:T9)  [unwired: 1 in]
                n1458 = property on="Dynamic2" class="Clust (strict)"("Value"=w469) -> ()  [unwired: 2 in, 2 out]
                n1459 = property on="Dynamic1" class="Clust (strict)"("Value"=w471) -> ()  [unwired: 2 in, 2 out]
                n1460 = Bundle("queue out"=w487, "queue out"=w497, "queue out"=w490) -> (w478:T38)  [unwired: 1 in]
                n1461 = control-ref of="Run/Stop"() -> (w494:refnum<vi>)
                n1462 = control-ref of="AutoExit"() -> (w485:refnum<vi>)
                n1463 = property on="Path?" class="Bool (strict)"() -> ("Value"=w484:bool)  [unwired: 2 in, 2 out]
                n1464 = property on="s/d setting" class="Bool (strict)"() -> ("Value"=w477:bool)  [unwired: 2 in, 2 out]
                n1465 = control-ref of="auto step finish?"() -> (w496:refnum<vi>)
                n1466 = control-ref of="RUN"() -> (w481:refnum<vi>)
                n1467 = control-ref of="Run/Stop"() -> (w495:refnum<vi>)
                n1468 = property on="Report Data.Degree" class="Arr (strict)"() -> ("Value"=w479:dbl[][])  [unwired: 2 in, 2 out]
                n1469 = property on="Cluster" class="Clust (strict)"() -> ("Value"=w489:cluster{"tester  A":bool, " tester B":bool})  [unwired: 2 in, 2 out]
                n1470 = Bundle("auto step finish?"=w496, "Run/Stop"=w495, "Run/Stop"=w494, "AutoExit"=w485, "RUN"=w481) -> (w491:T39)  [unwired: 1 in]
                n1471 = property on="wait" class="DigNum (strict)"() -> ("Value"=w476:u32)  [unwired: 2 in, 2 out]
                n1472 = control-ref of="MSG"() -> (w482:refnum<vi>)
                n1473 = control-ref of="Path A"() -> (w493:refnum<vi>)
                n1474 = property on="wait 2" class="DigNum (strict)"() -> ("Value"=w475:u32)  [unwired: 2 in, 2 out]
                n1475 = control-ref of="Path B"() -> (w492:refnum<vi>)
                n1476 = case shown="False" w477 {
                  tunnel: w493 -> [w512 w559]
                  tunnel: w474 -> [w514 w558]
                  tunnel: w492 -> [w510 w557]
                  tunnel: w491 -> [w505 w556]
                  tunnel: w489 -> [w506 w555]
                  tunnel: w477 -> [_ w554]
                  tunnel: "Mode" -> [w502 w553]
                  tunnel: w486 -> [w507 w552]
                  tunnel: w473 -> [w513 w551]
                  tunnel: w484 -> [_ w550]
                  tunnel: w482 -> [w511 w549]
                  tunnel: [w508 w548] -> w480
                  tunnel: w479 -> [w509 w547]
                  tunnel: w478 -> [w515 w546]
                  tunnel: w476 -> [w504 w545]
                  tunnel: w475 -> [w503 w544]
                  frame False {
                    # "dynamic"
                    n1477 = property on="last time" class="DigNum (strict)"() -> ("Value"=w501:dbl)  [unwired: 2 in, 2 out]
                    n1478 = Divide(x="early time(ms)", y=100.0) -> (x/y=w498:dbl)
                    n1479 = case shown="False" w502 {
                      tunnel: w515 -> [w530 w539]
                      tunnel: w514 -> [w529 w538]
                      tunnel: w513 -> [w518 w533]
                      tunnel: w512 -> [w528 w536]
                      tunnel: w511 -> [w527 w535]
                      tunnel: w510 -> [w526 w537]
                      tunnel: w509 -> [w525 w542]
                      tunnel: [w524 w534] -> w508
                      tunnel: w507 -> [w523 w543]
                      tunnel: w506 -> [w522 w541]
                      tunnel: w505 -> [w521 w540]
                      tunnel: w504 -> [w520 _]
                      tunnel: w503 -> [w519 _]
                      tunnel: w501 -> [w517 w532]
                      tunnel: w498 -> [w516 w531]
                      frame False {
                        n1480 = call "autoqueue_dynamic.vi"("cluster"=w530, "1to4"=w529, "xy dynamic array"=w518, "error out"=w523, "output cluster"=w521, "reference"=w528, "index"=w516, "last time"=w517, "Str Refnum"=w527, "Cluster"=w522, "reference 2"=w526, "Report Data.Degree"=w525, "milliseconds to wait"=w520, "milliseconds to wait 2"=w519) -> ("error out 2"=w524:errorcluster)  [unwired: 5 in]
                      }
                      frame True {
                        n1481 = call "autoqueue_dynamic_DUAL.vi"("cluster"=w539, "1to4"=w538, "xy dynamic array"=w533, "error out"=w543, "output cluster"=w540, "reference"=w536, "index"=w531, "last tme"=w532, "Str Refnum"=w535, "Cluster"=w541, "reference 2"=w537, "Report Data.Degree"=w542) -> ("error out 2"=w534:errorcluster)  [unwired: 7 in]
                      }
                    }
                  }
                  frame True {
                    # "stastic"
                    n1482 = case shown="True" w553 {
                      tunnel: w546 -> [w567 w575]
                      tunnel: w559 -> [w566 w578]
                      tunnel: w558 -> [w572 w581]
                      tunnel: w557 -> [w565 w577]
                      tunnel: w556 -> [w571 w579]
                      tunnel: w552 -> [w570 w582]
                      tunnel: [w569 w583] -> w548
                      tunnel: w555 -> [w568 w580]
                      tunnel: w554 -> [_ _]
                      tunnel: w551 -> [_ _]
                      tunnel: w549 -> [w564 w576]
                      tunnel: w550 -> [w563 w574]
                      tunnel: w547 -> [w562 w573]
                      tunnel: w545 -> [w561 _]
                      tunnel: w544 -> [w560 _]
                      frame False {
                        n1483 = call "autoqueue.vi"("cluster"=w567, "output cluster"=w571, "Cluster"=w568, "Report Data.Degree"=w562, "1to4"=w572, "milliseconds to wait"=w561, "path?"=w563, "milliseconds to wait 2"=w560, "error out"=w570, "reference"=w566, "Str Refnum"=w564, "reference 2"=w565) -> ("error out 2"=w569:errorcluster)  [unwired: 3 in]
                      }
                      frame True {
                        n1484 = call "autoqueue_dual.vi"("cluster"=w575, "output cluster"=w579, "Cluster"=w580, "1to4"=w581, "path"=w574, "Str Refnum"=w576, "error out"=w582, "Slide Refnum"=w578, "Report Data.Degree"=w573, "Slide Refnum 2"=w577) -> ("error out 2"=w583:errorcluster)  [unwired: 5 in]
                      }
                    }
                  }
                }
                n1485 = property class="Str"(reference=w482, error in=w480) -> ("Value"=w483:string)  [unwired: 2 out]
              }
              frame #3 {
                n1486 = case shown="False" "loop" {
                  tunnel: w587 -> [w595 _]
                  tunnel: w586 -> [w594 _]
                  frame False {
                    n1487 = property class="Bool (strict)"(reference=w595, error in=w594, "Value"=FALSE) -> ()  [unwired: 2 out]
                  }
                  frame True {
                  }
                }
                n1488 = Concatenate Strings("\n\nFinish  !!\n\n" ("Value"), w589) -> (w588:string)
                n1489 = property class="Str"(reference=w592, error in=w591, "Value"=w588) -> ()  [unwired: 2 out]
              }
              frame #4 {
                n1490 = Unbundle By Name(w605) -> ("queue out"=w604:refnum<queue>, "queue out"=w603:refnum<queue>)  [unwired: 1 out]
                n1491 = Bundle By Name(cluster=T19 {enum."RF ON/OFF", "variant"=variant}, "variant"=FALSE) -> (w597:T19)
                n1492 = Bundle By Name(cluster=T19 {enum."RF ON/OFF", "variant"=variant}, "variant"=FALSE) -> (w600:T19)
                n1493 = Enqueue Element(queue=w604, element=w600, error in (no error)=w602) -> ()  [unwired: 1 in, 3 out]
                n1494 = Enqueue Element(queue=w603, element=w597, error in (no error)=w602) -> ()  [unwired: 1 in, 3 out]
              }
              frame #5 {
                n1495 = Wait (ms)(milliseconds to wait=u32 3000) -> ()  [unwired: 1 out]
              }
            }
            n1496 = Enqueue Element(queue=w421, element=cluster{"State":T17, "Variable":variant} {"State"=enum."reset ant", "Variable"=variant}, error in (no error)=w420) -> ()  [unwired: 1 in, 3 out]
          }
        }
        n1497 = local read "Exit"() -> (w406:bool)
      }
      n1498 = while {
        tunnel: w89 -> [w3893]
        tunnel: w90 -> [w3892]
        shift-right: [w3884] -> _
        shift-left: w103 -> [w3885]
        tunnel: w102 -> [w3883]
        tunnel: w94 -> [w3882]
        tunnel: w90 -> [w3881]
        tunnel: w91 -> [w3880]
        tunnel: w93 -> [w3879]
        stop <- w3886 stop-if-true
        n1499 = Dequeue Element(queue=w3893, error in (no error)=w3892) -> (queue out=w3888:refnum<queue>, element=w3890:T18, error out=w3891:errorcluster)  [unwired: 1 in, 1 out]
        n1500 = Unbundle(w3890) -> ("State"=w3889:T40, "variant"=w3887:variant)
        n1501 = case shown="\"Initial\"" w3889 {
          tunnel: w3891 -> [_ w3921 w4004 _ w4120 w4204 w4220 w4292 _ w4347 w4369 w4391 w4397 w4406 w4418 w4427 w4444 w4458 w4478 w4499 w4557 w4573 w4650 w4674]
          tunnel: w3888 -> [_ w3913 _ _ w4117 w4199 w4225 w4294 _ w4351 w4368 w4385 _ w4404 w4409 w4428 w4445 w4454 w4475 w4498 w4550 w4572 w4658 _]
          tunnel: w3887 -> [_ _ _ _ w4121 _ _ _ _ _ _ w4392 w4398 w4407 w4419 _ _ w4459 w4479 _ w4558 w4574 _ _]
          tunnel: [_ _ _ _ _ _ _ _ _ _ _ _ _ _ _ _ _ _ _ _ _ _ _ TRUE] -> w3886
          tunnel: w3885 -> [w3894 w3920 w4001 w4071 w4119 w4203 w4227 w4285 w4329 w4349 w4372 w4390 w4396 w4400 w4416 w4430 w4447 w4461 w4480 w4502 w4556 w4569 w4660 w4676]
          tunnel: [w3894 w3919 w4001 w4071 w4118 w4202 w4226 w4282 w4328 w4348 w4371 w4389 w4395 w4405 w4417 w4431 w4448 w4460 w4472 w4501 w4555 w4567 w4661 w4676] -> w3884
          tunnel: w3883 -> [_ w3917 _ _ _ _ _ _ _ _ _ _ _ _ _ _ _ _ _ _ _ _ _ _]
          tunnel: w3882 -> [_ _ _ _ _ _ _ _ _ _ w4364 _ _ _ _ _ _ _ _ _ _ _ _ _]
          tunnel: w3881 -> [_ _ _ _ _ _ _ _ _ _ _ _ _ _ _ _ _ _ _ _ _ _ _ _]
          tunnel: w3880 -> [_ _ _ _ _ _ _ _ _ _ _ _ _ _ _ _ _ _ _ _ _ _ _ _]
          tunnel: w3879 -> [_ _ _ _ _ _ _ w4286 _ _ _ _ _ _ _ _ _ _ _ _ _ _ _ _]
          frame "Idle", Default {
          }
          frame "Initial" {
            w3909 = 0
            w3904 = 500 ("dimension size")
            w3902 = cluster{"X":dbl, "Y":dbl} {"X"=0.0, "Y"=0.0}
            n1502 = property on="Lane Distance(X,Y)" class="Clust (strict)"() -> ("Value"=w3901:cluster{"X":dbl, "Y":dbl})  [unwired: 2 in, 2 out]
            n1503 = Build Path(base path=w3917, name or relative path="Pic\\Map.png") -> (appended path=w3915:path)
            n1504 = Initialize Array(w3902, w3904) -> (w3908:cluster{"X":dbl, "Y":dbl}[])
            n1505 = Initialize Array(0.0 ("Breadth"), w3904) -> (w3903:dbl[])
            n1506 = call "IMAQ Create"("Image Name"="Path", "error in (no error)"=w3921) -> ("New Image"=w3923:T6, "error out"=w3924:errorcluster)  [unwired: 3 in]
            n1507 = Bundle(w3908, w3909, w3908, w3909, w3902, FALSE, w3903, w3903, "Value"=w3901, "Lines Para"=dbl[][] [], "Line to Line"=dbl[] []) -> (w3910:T41)  [unwired: 1 in]
            n1508 = call "IMAQ Read Image And Vision Info"("File Path"=w3915, "error in (no error)"=w3924, "Image"=w3923) -> ("error out"=w3914:errorcluster, "Image Out"=w3918:T6)  [unwired: 6 in, 1 out]
            n1509 = Initialize Array(w3910, 7 ("dimension size")) -> (w3907:T42)
            n1510 = Bundle By Name(cluster=w3920, "Image"=w3918, "Last Mouse Position"=w3907) -> (w3919:T25)
            n1511 = Enqueue Element(queue=w3913, element=T18 {"State"=enum."Lines Para", "variant"=variant}, error in (no error)=w3914) -> (error out=w3898:errorcluster)  [unwired: 1 in, 2 out]
            n1512 = disable-structure shown="Enabled" {
              disable-tunnel: w3898 -> [w3929 w3963]
              disable-tunnel: [_ w3959] -> w3897
              frame Disabled {
                w3926 = string[] []
                n1513 = call <vilib>:"Application Directory.vi"() -> ("Application Directory"=w3925:path)
                n1514 = Build Path(base path=w3925, name or relative path="config1.xml") -> (appended path=w3948:path)
                n1515 = Build Path(base path=w3925, name or relative path="config2.xml") -> (appended path=w3943:path)
                n1516 = Build Path(base path=w3925, name or relative path="config3.xml") -> (appended path=w3942:path)
                n1517 = call-poly <vilib>:"Read From XML File.vi"("error in (no error)"=w3929, "XML File Path"=w3948) -> ("error out"=w3947:errorcluster, "XML Elements"=w3946:string)  [unwired: 7 in, 1 out]
                n1518 = call-poly <vilib>:"Read From XML File.vi"("error in (no error)"=w3929, "XML File Path"=w3943) -> ("error out"=w3939:errorcluster, "XML Elements"=w3941:string)  [unwired: 7 in, 1 out]
                n1519 = call-poly <vilib>:"Read From XML File.vi"("error in (no error)"=w3929, "XML File Path"=w3942) -> ("error out"=w3938:errorcluster, "XML Elements"=w3937:string)  [unwired: 7 in, 1 out]
                n1520 = Unflatten From XML(xml string=w3946, type=w3926, error in (no error)=w3947) -> (value=w3928:string[], error out=w3933:errorcluster)
                n1521 = Unflatten From XML(xml string=w3941, type=i16[][] [] ("type string"), error in (no error)=w3939) -> (value=w3936:i16[][], error out=w3932:errorcluster)
                n1522 = Unflatten From XML(xml string=w3937, type=w3926, error in (no error)=w3938) -> (value=w3935:string[], error out=w3931:errorcluster)
                n1523 = control-ref of="This VI"() -> (w3927:refnum<vi>)
                n1524 = Merge Errors(w3933, w3932, w3931) -> (w3934:errorcluster)
                n1525 = for {
                  tunnel: w3927 -> [w3956]
                  tunnel: w3928 -> [w3955] mode=indexing
                  tunnel: w3936 -> [w3953] mode=indexing
                  tunnel: w3935 -> [w3952] mode=indexing
                  shift-right: [w3950] -> w3930
                  shift-left: w3934 -> [w3954]
                  n1526 = Flattened String To Variant(6:w3952, 7:w3953) -> (3:w3951:variant)  [unwired: 1 in, 1 out]
                  n1527 = invoke class="VI" method="Ctrl Val.Set"(reference=w3956, error in=w3954, "Control Name"=w3955, "Value"=w3951) -> (error out=w3950:errorcluster)  [unwired: 1 in, 4 out]
                }
                n1528 = call <vilib>:"Clear Errors.vi"("error in (no error)"=w3930) -> ()  [unwired: 5 in, 2 out]
              }
              frame Enabled {
                n1529 = call <vilib>:"Application Directory.vi"() -> ("Application Directory"=w3975:path)
                n1530 = Build Path(base path=w3975, name or relative path="config.xml") -> (appended path=w3973:path)
                n1531 = call-poly <vilib>:"Read From XML File.vi"("error in (no error)"=w3963, "XML File Path"=w3973) -> ("error out"=w3962:errorcluster, "XML Elements"=w3972:string)  [unwired: 7 in, 1 out]
                n1532 = Unflatten From XML(xml string=w3972, type=string[][] [], error in (no error)=w3962) -> (value=w3970:string[][], error out=w3961:errorcluster)
                n1533 = control-ref of="This VI"() -> (w3966:refnum<vi>)
                n1534 = Index Array(array=w3970, index (col) #1=0 ("index (row)"), index (col) #2=1 ("disabled index (col)")) -> (element #1=w3968:string[], element #2=w3967:string[])  [unwired: 2 in]
                n1535 = invoke class="VI" method="Ctrl Val.Get All"(reference=w3966, error in=w3961, "Controls"=TRUE) -> (reference out=w3965:refnum<vi>, error out=w3960:errorcluster, "Get All Control Values Variant"=w3964:cluster{"Name":string, "Variant Data":variant}[])  [unwired: 1 in, 1 out]
                n1536 = for {
                  tunnel: w3965 -> [w3984]
                  tunnel: w3968 -> [w3983] mode=indexing
                  tunnel: w3967 -> [w3978] mode=indexing
                  tunnel: w3964 -> [w3980] mode=indexing
                  tunnel: w3960 -> [w3977]
                  tunnel: [w3976] -> w3959
                  n1537 = Unbundle(w3980) -> ("Variant Data"=w3979:variant)  [unwired: 1 out]
                  n1538 = Unflatten From XML(xml string=w3978, type=w3979, error in (no error)=w3977) -> (value=w3981:variant, error out=w3982:errorcluster)
                  n1539 = invoke class="VI" method="Ctrl Val.Set"(reference=w3984, error in=w3982, "Control Name"=w3983, "Value"=w3981) -> (error out=w3976:errorcluster)  [unwired: 1 in, 4 out]
                }
              }
            }
            n1540 = property on="Tab Control" class="TabCtl (strict)"(error in=w3897, "Value"=T4."FCW" ("Tab Control")) -> (error out=w3896:errorcluster)  [unwired: 1 in, 1 out]
            n1541 = call <vilib>:"Clear Errors.vi"("error in (no error)"=w3896) -> ()  [unwired: 5 in, 2 out]
          }
          frame "save" {
            n1542 = Unbundle(w4001) -> ("Last Mouse Position"=w4000:T26, "DYNAMIC"=w3988:T1, "DYNAMIC 2"=w3987:T1, "dy Path"=w3985:T8)  [unwired: 12 out]
            n1543 = control-ref of="This VI"() -> (w3997:refnum<vi>)
            n1544 = Get Date/Time In Seconds() -> (seconds since 1Jan1904=w4003:timestamp)
            n1545 = Build Array(w3988, w3987) -> (w3986:T43)
            n1546 = invoke class="VI" method="Ctrl Val.Get All"(reference=w3997, error in=w4004, "Controls"=TRUE) -> ("Get All Control Values Variant"=w3995:cluster{"Name":string, "Variant Data":variant}[])  [unwired: 1 in, 3 out]
            n1547 = Format Date/Time String(time format string (%c)="%Y_%m_%d_%H_%M_%S", seconds (now)=w4003) -> (date/time string=w3998:string)  [unwired: 1 in]
            n1548 = property on="s/d setting" class="Bool (strict)"() -> ("Value"=w3999:bool)  [unwired: 2 in, 2 out]
            n1549 = for {
              shift-right: [w4009] -> w3992
              shift-left: string[][] [] -> [w4010]
              tunnel: w3995 -> [w4011] mode=indexing
              n1550 = Unbundle By Name(w4011) -> ("Name"=w4008:string, "Variant Data"=w4007:variant)
              n1551 = Flatten To XML(anything=w4007) -> (xml string=w4006:string)
              n1552 = Build Array(w4008, w4006) -> (w4005:string[])
              n1553 = Build Array (concatenate)(w4010, w4005) -> (w4009:string[][])
            }
            n1554 = call <vilib>:"Application Directory.vi"() -> ("Application Directory"=w3989:path)
            n1555 = case shown="False" w3999 {
              tunnel: w4000 -> [w4039 w4055]
              tunnel: w3986 -> [w4024 _]
              tunnel: w3998 -> [w4014 w4053]
              tunnel: w3989 -> [w4018 w4049]
              tunnel: w3985 -> [w4021 _]
              frame False {
                w4025 = i16 0 ("precision (6)")
                w4032 = "_" ("string")
                w4016 = ".xml" ("string")
                n1556 = Index Array(array=w4024) -> (element=w4023:T1)  [unwired: 2 in]
                n1557 = Array Size(array=w4024) -> (size(s)=w4038:i32[])
                n1558 = Index Array(array=w4023) -> (element=w4022:T5)  [unwired: 1 in]
                n1559 = Number To Decimal String(number=w4038) -> (decimal integer string=w4037:string[])  [unwired: 1 in]
                n1560 = Unbundle By Name(w4022) -> ("Start Speed (km/h)"=w4035:dbl, "Start Range(m)"=w4034:dbl, "Stop Range(m)"=w4033:dbl)
                n1561 = Flatten To XML(anything=w4021) -> (xml string=w4019:string)
                n1562 = Concatenate Strings(w4032, "point" ("string"), w4037, w4032) -> (w4013:string)
                n1563 = Flatten To XML(anything=w4024) -> (xml string=w4043:string)
                n1564 = Flatten To XML(anything=w4039) -> (xml string=w4046:string)
                n1565 = Number To Fractional String(number=w4035, precision (6)=w4025) -> (F-format string=w4031:string)  [unwired: 2 in]
                n1566 = Number To Fractional String(number=w4033, precision (6)=w4025) -> (F-format string=w4026:string)  [unwired: 2 in]
                n1567 = Number To Fractional String(number=w4034, precision (6)=w4025) -> (F-format string=w4029:string)  [unwired: 2 in]
                n1568 = Concatenate Strings("speed" ("string"), w4031, "_start" ("string"), w4029, "_stop" ("string"), w4026) -> (w4012:string)
                n1569 = Concatenate Strings("path\\dynamic\\" ("string"), w4014, w4013, w4012, w4016) -> (w4045:string)
                n1570 = Concatenate Strings("path\\dynamic\\setting" ("string"), w4014, w4013, w4012, w4016) -> (w4042:string)
                n1571 = Concatenate Strings("path\\dynamic\\dy_path" ("string"), w4014, w4013, w4012, w4016) -> (w4017:string)
                n1572 = Build Path(base path=w4018, name or relative path=w4045) -> (appended path=w4047:path)
                n1573 = Build Path(base path=w4018, name or relative path=w4017) -> (appended path=w4020:path)
                n1574 = Build Path(base path=w4018, name or relative path=w4042) -> (appended path=w4044:path)
                n1575 = call-poly <vilib>:"Write to XML File.vi"("XML Input"=w4019, "XML File Path"=w4020) -> ()  [unwired: 7 in, 3 out]
                n1576 = call-poly <vilib>:"Write to XML File.vi"("XML Input"=w4046, "XML File Path"=w4047) -> ()  [unwired: 7 in, 3 out]
                n1577 = call-poly <vilib>:"Write to XML File.vi"("XML Input"=w4043, "XML File Path"=w4044) -> ()  [unwired: 7 in, 3 out]
              }
              frame True {
                n1578 = Flatten To XML(anything=w4055) -> (xml string=w4050:string)
                n1579 = Concatenate Strings("path\\" ("string"), w4053, ".xml" ("string")) -> (w4048:string)
                n1580 = Build Path(base path=w4049, name or relative path=w4048) -> (appended path=w4051:path)
                n1581 = call-poly <vilib>:"Write to XML File.vi"("XML Input"=w4050, "XML File Path"=w4051) -> ()  [unwired: 7 in, 3 out]
              }
            }
            n1582 = Build Path(base path=w3989, name or relative path="config.xml") -> (appended path=w3993:path)
            n1583 = Flatten To XML(anything=w3992) -> (xml string=w3991:string)
            n1584 = call-poly <vilib>:"Write to XML File.vi"("XML Input"=w3991, "XML File Path"=w3993) -> ()  [unwired: 7 in, 3 out]
          }
          frame "Update" {
            n1585 = Unbundle By Name(w4071) -> ("Velocity"=w4072:dbl, "Image"=→"Image":T6, "Last Mouse Position"=w4077:T26, "Mode"=w4076:T7, "Path No."=w4067:u16, "User"=w4061:enum16{"Car 1", "Car 2"})
            n1586 = Unbundle By Name(w4071) -> ("Output £m File"=→"Output £m File":string, "Input RCS File"=→"Input RCS File":string, "Target 1"=w4070:string, "Target 2"=w4069:string, "DYNAMIC"=w4060:T1, "DYNAMIC 2"=w4059:T1)
            "Target 1" <- w4070
            "Target 2" <- w4069
            n1587 = Index Array(array=w4077, index=w4076) -> (element=w4062:T44)
            "Radar Settings" <- w4062
            n1588 = case shown="\"Car 1\", Default" w4061 {
              tunnel: w4062 -> [w4109 w4111]
              tunnel: [w4110 w4112] -> w4068
              tunnel: [w4109 w4111] -> w4066
              frame "Car 1", Default {
                n1589 = Unbundle By Name(w4109) -> ("Times 1"=w4110:i32)
              }
              frame "Car 2" {
                n1590 = Unbundle By Name(w4111) -> ("Times 2"=w4112:i32)
              }
            }
            n1591 = case shown="\"Car 1\", Default" w4061 {
              tunnel: w4060 -> [w4081 w4083]
              tunnel: w4059 -> [w4079 w4082]
              tunnel: [w4081 w4083] -> w4058
              tunnel: [w4080 w4084] -> w4057
              tunnel: [w4079 w4082] -> w4056
              frame "Car 1", Default {
                n1592 = Index Array(array=w4081) -> (element=w4080:T5)  [unwired: 1 in]
              }
              frame "Car 2" {
                n1593 = Index Array(array=w4082) -> (element=w4084:T5)  [unwired: 1 in]
              }
            }
            n1594 = property on="Velocity" class="DigNum (strict)"("Value"=w4072) -> ()  [unwired: 2 in, 2 out]
            n1595 = Unbundle By Name(w4066) -> ("Lane Distance(X,Y)"=w4065:cluster{"X":dbl, "Y":dbl})
            n1596 = String Length(string=w4070) -> (length=w4075:i32)
            n1597 = String Length(string=w4069) -> (length=w4074:i32)
            n1598 = property on="Target 1" class="Str"("Text.Scroll Position"=w4075) -> (error out=w4073:errorcluster)  [unwired: 2 in, 1 out]
            n1599 = property on="Lane Distance(X,Y)" class="Clust (strict)"("Value"=w4065) -> ()  [unwired: 2 in, 2 out]
            n1600 = property on="DYNAMIC" class="Arr (strict)"("Value"=w4058) -> ()  [unwired: 2 in, 2 out]
            n1601 = property on="DYNAMIC 2" class="Arr (strict)"("Value"=w4056) -> ()  [unwired: 2 in, 2 out]
            n1602 = property on="dynamic setting" class="Clust (strict)"("Value"=w4057) -> ()  [unwired: 2 in, 2 out]
            n1603 = property on="Target 2" class="Str"(error in=w4073, "Text.Scroll Position"=w4074) -> ()  [unwired: 1 in, 2 out]
            n1604 = property on="Path No." class="Ring (strict)"("Value"=w4067) -> ()  [unwired: 2 in, 2 out]
            n1605 = case shown="\"Car 1\", Default" w4061 {
              tunnel: w4062 -> [w4087 w4096]
              frame "Car 1", Default {
                n1606 = Unbundle By Name(w4087) -> ("Times 1"=w4085:i32)
                n1607 = Not Equal To 0?(x=w4085) -> (x != 0?=w4086:bool)
                n1608 = case shown="True" w4086 {
                  tunnel: w4085 -> [_ w4091]
                  frame False {
                    n1609 = property on="Path No." class="Ring (strict)"("Strings []"=string[] []) -> ()  [unwired: 2 in, 2 out]
                  }
                  frame True {
                    n1610 = for {
                      N: w4091 -> [_]
                      tunnel: [w4092] -> w4090 mode=indexing
                      i -> [w4093]
                      n1611 = Increment(x=w4093) -> (x+1=w4092:i32)
                    }
                    n1612 = Number To Decimal String(number=w4090) -> (decimal integer string=w4089:string[])  [unwired: 1 in]
                    n1613 = property on="Path No." class="Ring (strict)"("Strings []"=w4089) -> ()  [unwired: 2 in, 2 out]
                  }
                }
              }
              frame "Car 2" {
                n1614 = Unbundle By Name(w4096) -> ("Times 2"=w4094:i32)
                n1615 = Not Equal To 0?(x=w4094) -> (x != 0?=w4095:bool)
                n1616 = case shown="True" w4095 {
                  tunnel: w4094 -> [_ w4100]
                  frame False {
                    n1617 = property on="Path No." class="Ring (strict)"("Strings []"=string[] []) -> ()  [unwired: 2 in, 2 out]
                  }
                  frame True {
                    n1618 = for {
                      N: w4100 -> [_]
                      tunnel: [w4101] -> w4099 mode=indexing
                      i -> [w4102]
                      n1619 = Increment(x=w4102) -> (x+1=w4101:i32)
                    }
                    n1620 = Number To Decimal String(number=w4099) -> (decimal integer string=w4098:string[])  [unwired: 1 in]
                    n1621 = property on="Path No." class="Ring (strict)"("Strings []"=w4098) -> ()  [unwired: 2 in, 2 out]
                  }
                }
              }
            }
            n1622 = disable-structure shown="Disabled" {
              disable-tunnel: w4068 -> [w4103 _]
              frame Disabled {
                n1623 = case shown="1, Default" w4103 {
                  selector: w4103 -> [_ w4105]
                  tunnel: [_ w4104] -> _
                  frame 0 {
                  }
                  frame 1, Default {
                    n1624 = for {
                      N: w4105 -> [_]
                      tunnel: [w4106] -> w4104 mode=indexing
                      i -> [w4108]
                      n1625 = Increment(x=w4108) -> (x+1=w4107:i32)
                      n1626 = Number To Decimal String(number=w4107) -> (decimal integer string=w4106:string)  [unwired: 1 in]
                    }
                  }
                }
              }
              frame Enabled {
              }
            }
          }
          frame "Overlay_Circle Para" {
            n1627 = Variant To Data(error in=w4120, type=cluster{"X":i32, "Y":i32}[] [], Variant=w4121) -> (data=w4115:cluster{"X":i32, "Y":i32}[], error out=w4113:errorcluster)
            n1628 = for {
              tunnel: w4115 -> [w4131] mode=indexing
              shift-right: [w4133] -> w4118
              shift-left: w4119 -> [w4134]
              n1629 = Unbundle By Name(w4134) -> ("Last Mouse Position"=w4129:T26, "Mode"=w4132:T7, "User"=w4122:enum16{"Car 1", "Car 2"}, "Velocity"=w4128:dbl, "DYNAMIC"=w4127:T1, "DYNAMIC 2"=w4123:T1)
              n1630 = in-place {
                in-place-border: w4131 -> [w4149]
                in-place-border: w4122 -> [w4152]
                in-place-border: w4128 -> [w4148]
                in-place-border: w4127 -> [w4147]
                in-place-border: [w4146] -> w4125
                in-place-border: w4123 -> [w4145]
                n1631 = in-place-array #1(w4129, w4132) -> (w4150:T44)
                n1632 = case shown="\"Car 1\"" w4152 {
                  tunnel: w4150 -> [w4173 w4194]
                  tunnel: [w4171 w4193] -> w4151
                  tunnel: w4149 -> [w4167 w4188]
                  tunnel: w4148 -> [w4159 w4182]
                  tunnel: w4147 -> [_ w4174]
                  tunnel: [w4155 w4175] -> w4146
                  tunnel: w4145 -> [w4153 _]
                  frame "Car 2" {
                    n1633 = Unbundle(w4173) -> ("User1"=w4172:cluster{"X":dbl, "Y":dbl}[], "Times 1"=w4170:i32, "User2"=w4169:cluster{"X":dbl, "Y":dbl}[], "Times 2"=w4158:i32, "ORG"=w4165:cluster{"X":dbl, "Y":dbl}, "ORG?"=w4164:bool, "User1 Velocity"=w4163:dbl[], "User2 Velocity"=w4161:dbl[], "Lane Distance(X,Y)"=w4162:cluster{"X":dbl, "Y":dbl}, "Lines Para"=w4157:dbl[][], "Line to Line"=w4156:dbl[])
                    n1634 = Increment(x=w4158) -> (x+1=w4166:i32)
                    n1635 = Replace Array Subset(array=w4169, new element=w4167, index=w4158) -> (w4168:cluster{"X":dbl, "Y":dbl}[])
                    n1636 = Replace Array Subset(array=w4161, new element=w4159, index=w4158) -> (w4160:dbl[])
                    n1637 = property on="dynamic setting" class="Clust (strict)"() -> ("Value"=w4154:T5)  [unwired: 2 in, 2 out]
                    n1638 = Bundle(cluster=w4173, "User1"=w4172, "Times 1"=w4170, "User2"=w4168, "Times 2"=w4166, "ORG"=w4165, "ORG?"=w4164, "User1 Velocity"=w4163, "User2 Velocity"=w4160, "Lane Distance(X,Y)"=w4162, "Lines Para"=w4157, "Line to Line"=w4156) -> (w4171:T44)
                    n1639 = Build Array (concatenate)(w4153, w4154) -> (w4155:T1)
                  }
                  frame "Car 1" {
                    n1640 = Unbundle(w4194) -> ("User1"=w4190:cluster{"X":dbl, "Y":dbl}[], "Times 1"=w4183:i32, "User2"=w4192:cluster{"X":dbl, "Y":dbl}[], "Times 2"=w4191:i32, "ORG"=w4186:cluster{"X":dbl, "Y":dbl}, "ORG?"=w4185:bool, "User1 Velocity"=w4180:dbl[], "User2 Velocity"=w4184:dbl[], "Lane Distance(X,Y)"=w4181:cluster{"X":dbl, "Y":dbl}, "Lines Para"=w4178:dbl[][], "Line to Line"=w4177:dbl[])
                    n1641 = Replace Array Subset(array=w4190, new element=w4188, index=w4183) -> (w4189:cluster{"X":dbl, "Y":dbl}[])
                    n1642 = Increment(x=w4183) -> (x+1=w4187:i32)
                    n1643 = Replace Array Subset(array=w4180, new element=w4182, index=w4183) -> (w4179:dbl[])
                    n1644 = property on="dynamic setting" class="Clust (strict)"() -> ("Value"=w4176:T5)  [unwired: 2 in, 2 out]
                    n1645 = Bundle(cluster=w4194, "User1"=w4189, "Times 1"=w4187, "User2"=w4192, "Times 2"=w4191, "ORG"=w4186, "ORG?"=w4185, "User1 Velocity"=w4179, "User2 Velocity"=w4184, "Lane Distance(X,Y)"=w4181, "Lines Para"=w4178, "Line to Line"=w4177) -> (w4193:T44)
                    n1646 = Build Array (concatenate)(w4174, w4176) -> (w4175:T1)
                  }
                }
                n1647 = in-place-array #1(w4151) -> (w4130:T26)  [unwired: 1 out]
              }
              n1648 = property on="s/d setting" class="Bool (strict)"() -> ("Value"=w4126:bool)  [unwired: 2 in, 2 out]
              n1649 = case shown="False" w4126 {
                tunnel: w4125 -> [w4143 _]
                tunnel: [w4143 T1 []] -> w4124
                frame False {
                }
                frame True {
                }
              }
              n1650 = case shown="\"Car 1\", Default" w4122 {
                tunnel: w4134 -> [w4137 w4142]
                tunnel: [w4138 w4141] -> w4133
                tunnel: w4130 -> [w4136 w4140]
                tunnel: w4124 -> [w4135 w4139]
                frame "Car 1", Default {
                  n1651 = Bundle By Name(cluster=w4137, "Last Mouse Position"=w4136, "DYNAMIC"=w4135) -> (w4138:T25)
                }
                frame "Car 2" {
                  n1652 = Bundle By Name(cluster=w4142, "Last Mouse Position"=w4140, "DYNAMIC 2"=w4139) -> (w4141:T25)
                }
              }
            }
            n1653 = Enqueue Element(queue=w4117, element=T18 {"State"=enum."Overlay", "variant"=variant}, error in (no error)=w4113) -> ()  [unwired: 1 in, 3 out]
          }
          frame "Overlay" {
            n1654 = Unbundle By Name(w4203) -> ("Image"=w4207:T6, "Last Mouse Position"=w4197:T26, "Mode"=w4196:T7)
            n1655 = call "IMAQ Clear Overlay"("error in (no error)"=w4204, "Image"=w4207) -> ("error out"=w4205:errorcluster, "Image Out"=w4206:T6)  [unwired: 8 in]
            n1656 = call "Check Overlay Settings.vi"("error in (no error)"=w4205, "Mode"=w4196, "Overlay Settings"=w4197, "Refnum in"=w4206) -> ("error out"=w4200:errorcluster, "Report Data"=w4195:T27, "Refnum out"=w4201:T6)  [unwired: 5 in]
            n1657 = Bundle By Name(cluster=w4203, "Image"=w4201, "Report Data"=w4195) -> (w4202:T25)
            n1658 = Enqueue Element(queue=w4199, element=T18 {"State"=enum."Report", "variant"=variant}, error in (no error)=w4200) -> ()  [unwired: 1 in, 3 out]
          }
          frame "Report" {
            w4211 = 0
            n1659 = Unbundle By Name(w4227) -> ("Report Data.Degree"=w4217:dbl[][], "Report Data.Coordinate"=w4219:cluster{string, string}[][], "Report Data.Times"=w4218:i32[], "Report Data.Velocity"=w4216:dbl[][])
            n1660 = for {
              tunnel: w4219 -> [w4235] mode=indexing
              tunnel: [w4236] -> w4223 mode=indexing
              tunnel: w4218 -> [w4229] mode=indexing
              tunnel: w4216 -> [w4232] mode=indexing
              tunnel: w4217 -> [w4230] mode=indexing
              n1661 = Array Subset(array=w4235, length=w4229) -> (w4233:cluster{string, string}[])  [unwired: 1 in]
              n1662 = Array Subset(array=w4232, length=w4229) -> (w4231:dbl[])  [unwired: 1 in]
              n1663 = Array Subset(array=w4230, length=w4229) -> (w4228:dbl[])  [unwired: 1 in]
              n1664 = Empty Array?(array=w4233) -> (empty?=w4234:bool)
              n1665 = case shown="False" w4234 {
                tunnel: [w4239 _] -> w4236
                tunnel: w4233 -> [w4241 _]
                tunnel: w4231 -> [w4238 _]
                tunnel: w4228 -> [w4237 _]
                frame False {
                  n1666 = while {
                    shift-right: [w4255] -> w4239
                    shift-left: "" -> [w4254]
                    tunnel: w4241 -> [w4253]
                    tunnel: w4238 -> [w4246]
                    tunnel: w4237 -> [w4244]
                    i -> [w4243]
                    stop <- w4247 stop-if-true
                    n1667 = Index Array(array=w4246, index=w4243) -> (element=w4245:dbl)
                    n1668 = Index Array(array=w4244, index=w4243) -> (element=w4242:dbl)
                    n1669 = Array Subset(array=w4253, index=w4243, length=2) -> (w4248:cluster{string, string}[])
                    n1670 = Array Size(array=w4248) -> (size(s)=w4252:i32)
                    n1671 = Index Array(array=w4248) -> (element #1=w4258:cluster{string, string}, element #2=w4257:cluster{string, string})  [unwired: 2 in]
                    n1672 = Less?(x=w4252, y=2) -> (x < y?=w4247:bool)
                    n1673 = Increment(x=w4243) -> (x+1=w4249:i32)
                    n1674 = case shown="True" w4247 {
                      tunnel: w4258 -> [w4266 w4278]
                      tunnel: w4257 -> [_ w4274]
                      tunnel: w4249 -> [w4262 w4271]
                      tunnel: [w4261 w4269] -> w4256
                      tunnel: w4245 -> [w4260 w4268]
                      tunnel: w4242 -> [w4259 w4267]
                      frame True {
                        n1675 = Unbundle(w4266) -> (w4264:string, w4263:string)
                        n1676 = Format Into String(format string="¸ô®| %u (³t«× %.2f)\n%u(%s,%s)\n¨¤«× %.2f\n", w4262, w4260, w4262, w4264, w4263, w4259) -> (resulting string=w4261:string)  [unwired: 2 in, 1 out]
                      }
                      frame False {
                        n1677 = Increment(x=w4271) -> (x+1=w4270:i32)
                        n1678 = Unbundle(w4274) -> (w4273:string, w4272:string)
                        n1679 = Unbundle(w4278) -> (w4276:string, w4275:string)
                        n1680 = Format Into String(format string="¸ô®| %u (³t«× %.2f)\n%u(%s,%s)==>%u(%s,%s)\n¨¤«× %.2f\n\n", w4271, w4268, w4271, w4276, w4275, w4270, w4273, w4272, w4267) -> (resulting string=w4269:string)  [unwired: 2 in, 1 out]
                      }
                    }
                    n1681 = Concatenate Strings(w4254, w4256) -> (w4255:string)
                  }
                }
                frame True {
                }
              }
            }
            n1682 = Index Array(array=w4216) -> (element #1=w4215:dbl[], element #2=w4214:dbl[])  [unwired: 4 in]
            n1683 = Array Size(array=w4214) -> (size(s)=w4212:i32)
            n1684 = Array Size(array=w4215) -> (size(s)=w4213:i32)
            n1685 = property on="Path A" class="Slide (strict)"("Scale.Maximum"=w4213, "Scale.Minimum"=w4211) -> ()  [unwired: 2 in, 2 out]
            n1686 = property on="Path B" class="Slide (strict)"("Scale.Maximum"=w4212, "Scale.Minimum"=w4211) -> ()  [unwired: 2 in, 2 out]
            n1687 = Index Array(array=w4223) -> (element #1=w4222:string, element #2=w4221:string)  [unwired: 2 in]
            n1688 = Bundle By Name(cluster=w4227, "Target 1"=w4222, "Target 2"=w4221) -> (w4226:T25)
            n1689 = Enqueue Element(queue=w4225, element=T18 {"State"=enum."Update", "variant"=variant}, error in (no error)=w4220) -> (queue out=w4210:refnum<queue>, error out=w4209:errorcluster)  [unwired: 1 in, 1 out]
            n1690 = Enqueue Element(queue=w4210, element=T18 {"State"=enum."Report Dist", "variant"=variant}, error in (no error)=w4209) -> ()  [unwired: 1 in, 3 out]
          }
          frame "Report Dist" {
            n1691 = Unbundle By Name(w4285) -> ("Report Data.Coordinate"=w4291:cluster{string, string}[][], "Report Data.Times"=w4290:i32[], "Report Data.Velocity"=w4289:dbl[][], "Report Data.Degree"=→"Report Data.Degree":dbl[][])
            n1692 = for {
              tunnel: w4291 -> [w4307] mode=indexing
              tunnel: w4290 -> [w4303] mode=indexing
              tunnel: w4289 -> [w4304] mode=indexing
              tunnel: [w4301] -> w4288 mode=indexing
              n1693 = Array Subset(array=w4307, length=w4303) -> (w4305:cluster{string, string}[])  [unwired: 1 in]
              n1694 = Array Subset(array=w4304, length=w4303) -> (w4302:dbl[])  [unwired: 1 in]
              n1695 = Empty Array?(array=w4305) -> (empty?=w4306:bool)
              n1696 = case shown="False" w4306 {
                tunnel: w4305 -> [w4311 _]
                tunnel: w4302 -> [w4310 _]
                tunnel: [w4308 _] -> w4301
                frame False {
                  n1697 = while {
                    tunnel: w4311 -> [w4326]
                    tunnel: w4310 -> [w4320]
                    shift-right: [w4317] -> w4308
                    shift-left: T22 [] -> [w4316]
                    i -> [w4319]
                    stop <- w4321 stop-if-true
                    n1698 = Index Array(array=w4320, index=w4319) -> (element=w4318:dbl)
                    n1699 = Array Subset(array=w4326, index=w4319, length=2) -> (w4322:cluster{string, string}[])
                    n1700 = Array Size(array=w4322) -> (size(s)=w4325:i32)
                    n1701 = Index Array(array=w4322) -> (element #1=w4315:cluster{string, string}, element #2=w4314:cluster{string, string})  [unwired: 2 in]
                    n1702 = Less?(x=w4325, y=2) -> (x < y?=w4321:bool)
                    n1703 = Bundle(cluster=T23 {0.0, {"", ""}, {"", ""}}, w4318, w4315, w4314) -> (w4313:T23)
                    n1704 = Build Array (concatenate)(w4316, w4313) -> (w4317:T22)
                  }
                }
                frame True {
                }
              }
            }
            "Array" <- w4288
            n1705 = disable-structure shown="Enabled" {
              disable-tunnel: w4285 -> [w4299 w4300]
              disable-tunnel: [w4298 w4300] -> w4282
              frame Disabled {
                n1706 = Bundle By Name(cluster=w4299) -> (w4298:T25)  [unwired: 2 in]
              }
              frame Enabled {
              }
            }
            n1707 = Enqueue Element(queue=w4294, element=T18 {"State"=enum."Update", "variant"=variant}, error in (no error)=w4292) -> (queue out=w4280:refnum<queue>, error out=w4284:errorcluster)  [unwired: 1 in, 1 out]
            n1708 = Enqueue Element(queue=w4286, element=cluster{"State":T17, "Variable":variant} {"State"=enum."get angle", "Variable"=variant}, error in (no error)=w4284) -> (error out=w4279:errorcluster)  [unwired: 1 in, 2 out]
            n1709 = property on="load?" class="Bool (strict)"() -> ("Value"=w4281:bool)  [unwired: 2 in, 2 out]
            n1710 = case shown="True" w4281 {
              tunnel: w4280 -> [_ w4296]
              tunnel: w4279 -> [_ w4297]
              frame False {
              }
              frame True {
                n1711 = Enqueue Element(queue=w4296, element=T18 {"State"=enum."dypath", "variant"=variant}, error in (no error)=w4297) -> ()  [unwired: 1 in, 3 out]
              }
            }
          }
          frame "dypath" {
            n1712 = property on="load?" class="Bool (strict)"() -> ("Value"=w4327:bool)  [unwired: 2 in, 2 out]
            n1713 = case shown="True" w4327 {
              tunnel: w4329 -> [w4331 w4339]
              tunnel: [w4330 w4339] -> w4328
              frame False {
                n1714 = flat-sequence {
                  tunnel: w4331 -> [w4334]
                  tunnel: [w4334] -> w4332
                  tunnel: w4332 -> [w4337]
                  tunnel: [w4336] -> w4330
                  frame #0 {
                    n1715 = Wait (ms)(milliseconds to wait=u32 200) -> ()  [unwired: 1 out]
                  }
                  frame #1 {
                    n1716 = property on="dy Path" class="Arr (strict)"() -> ("Value"=w4335:T8)  [unwired: 2 in, 2 out]
                    n1717 = Bundle By Name(cluster=w4337, "dy Path"=w4335) -> (w4336:T25)
                  }
                }
              }
              frame True {
                n1718 = flat-sequence {
                  tunnel: w4339 -> [w4341]
                  tunnel: [w4341] -> w4338
                  tunnel: w4338 -> [w4343]
                  frame #0 {
                    n1719 = Wait (ms)(milliseconds to wait=u32 500) -> ()  [unwired: 1 out]
                  }
                  frame #1 {
                    n1720 = property on="load?" class="Bool (strict)"("Value"=FALSE ("load?")) -> ()  [unwired: 2 in, 2 out]
                    n1721 = Unbundle By Name(w4343) -> ("dy Path"=w4342:T8)
                    n1722 = property on="dy Path" class="Arr (strict)"("Value"=w4342) -> ()  [unwired: 2 in, 2 out]
                  }
                  frame #2 {
                    n1723 = property on="set" class="Bool (strict)"("Val(Sgnl)"=TRUE ("Value (Signaling)")) -> ()  [unwired: 2 in, 2 out]
                  }
                }
              }
            }
          }
          frame "dynamic" {
            n1724 = Unbundle By Name(w4349) -> ("User"=w4350:enum16{"Car 1", "Car 2"})
            n1725 = case shown="\"Car 2\"" w4350 {
              tunnel: w4349 -> [w4356 w4360]
              tunnel: [w4355 w4359] -> w4348
              tunnel: w4347 -> [w4353 w4357]
              tunnel: [w4353 w4357] -> w4346
              frame "Car 1", Default {
                n1726 = property on="DYNAMIC" class="Arr (strict)"() -> ("Value"=w4354:T1)  [unwired: 2 in, 2 out]
                n1727 = Bundle By Name(cluster=w4356, "DYNAMIC"=w4354) -> (w4355:T25)
              }
              frame "Car 2" {
                n1728 = property on="DYNAMIC 2" class="Arr (strict)"() -> ("Value"=w4358:T1)  [unwired: 2 in, 2 out]
                n1729 = Bundle By Name(cluster=w4360, "DYNAMIC 2"=w4358) -> (w4359:T25)
              }
            }
            n1730 = Enqueue Element(queue=w4351, element=T18 {"State"=enum."Update", "variant"=variant}, error in (no error)=w4346) -> ()  [unwired: 1 in, 3 out]
          }
          frame "RCS Report" {
            n1731 = Unbundle By Name(w4372) -> ("Input RCS Data"=w4374:dbl[][])
            n1732 = for {
              tunnel: w4374 -> [w4383] mode=indexing
              tunnel: [w4382] -> w4373 mode=indexing
              tunnel: [w4379] -> w4361 mode=indexing
              tunnel: [w4375] -> w4366 mode=indexing
              w4376 = "%u«× = (%.2f) dBsm\n"
              n1733 = Index Array(array=w4383) -> (element #1=w4378:dbl, element #2=w4380:dbl)  [unwired: 2 in]
              n1734 = Decrement(x=w4380) -> (x-1=w4381:dbl)
              n1735 = Power Of 10(x=w4381) -> (10^x=w4377:dbl)
              n1736 = Build Array(w4378, w4377) -> (w4379:dbl[])
              n1737 = Format Into String(format string=w4376, w4378, w4380) -> (resulting string=w4382:string)  [unwired: 2 in, 1 out]
              n1738 = Format Into String(format string=w4376, w4378, w4377) -> (resulting string=w4375:string)  [unwired: 2 in, 1 out]
            }
            n1739 = Enqueue Element(queue=w4368, element=T18 {"State"=enum."Update", "variant"=variant}, error in (no error)=w4369) -> ()  [unwired: 1 in, 3 out]
            n1740 = Concatenate Strings(w4373) -> (w4370:string)
            n1741 = Concatenate Strings(w4366) -> (w4365:string)
            n1742 = Bundle By Name(cluster=T19 {enum."£m Data", "variant"=variant}, "variant"=w4361) -> (w4362:T19)
            n1743 = Bundle By Name(cluster=w4372, "Output £m File"=w4365, "Input RCS File"=w4370) -> (w4371:T25)
            n1744 = Enqueue Element(queue=w4364, element=w4362) -> ()  [unwired: 2 in, 3 out]
          }
          frame "User" {
            n1745 = Variant To Data(error in=w4391, type=enum16{"Car 1", "Car 2"}."Car 1" ("User 2"), Variant=w4392) -> (data=w4388:enum16{"Car 1", "Car 2"}, error out=w4386:errorcluster)
            n1746 = Bundle By Name(cluster=w4390, "User"=w4388) -> (w4389:T25)
            n1747 = Enqueue Element(queue=w4385, element=T18 {"State"=enum."Update", "variant"=variant}, error in (no error)=w4386) -> ()  [unwired: 1 in, 3 out]
          }
          frame "Velocity" {
            n1748 = Variant To Data(error in=w4397, type=0.0, Variant=w4398) -> (data=w4394:dbl)  [unwired: 1 out]
            n1749 = Bundle By Name(cluster=w4396, "Velocity"=w4394) -> (w4395:T25)
          }
          frame "Mode" {
            n1750 = Variant To Data(error in=w4406, type=T7."FCW" ("Mode 2"), Variant=w4407) -> (data=w4399:T7, error out=w4402:errorcluster)
            n1751 = Bundle By Name(cluster=w4400, "Mode"=w4399) -> (w4405:T25)
            n1752 = Enqueue Element(queue=w4404, element=T18 {"State"=enum."Lines Para", "variant"=variant}, error in (no error)=w4402) -> ()  [unwired: 1 in, 3 out]
          }
          frame "Lane Distance" {
            n1753 = Variant To Data(error in=w4418, type=cluster{"X":dbl, "Y":dbl} {"X"=30.0, "Y"=30.0} ("Length(X,Y)"), Variant=w4419) -> (data=w4413:cluster{"X":dbl, "Y":dbl}, error out=w4410:errorcluster)
            n1754 = Unbundle By Name(w4416) -> ("Last Mouse Position"=w4415:T26, "Mode"=w4414:T7)
            n1755 = in-place {
              in-place-border: w4413 -> [w4420]
              n1756 = in-place-array #2(w4415, w4414) -> (w4422:T44)
              n1757 = Bundle By Name(cluster=w4422, "Lane Distance(X,Y)"=w4420) -> (w4421:T44)
              n1758 = in-place-array #2(w4421) -> (w4412:T26)  [unwired: 1 out]
            }
            n1759 = Bundle By Name(cluster=w4416, "Last Mouse Position"=w4412) -> (w4417:T25)
            n1760 = Enqueue Element(queue=w4409, element=T18 {"State"=enum."Overlay", "variant"=variant}, error in (no error)=w4410) -> ()  [unwired: 1 in, 3 out]
          }
          frame "ORG" {
            n1761 = Unbundle By Name(w4430) -> ("Last Mouse Position"=w4425:T26, "Mode"=w4424:T7)
            n1762 = case shown="\"FCW\", Default" w4424 {
              tunnel: [cluster{"X":dbl, "Y":dbl} {"X"=320.0, "Y"=460.0} ("ORG") cluster{"X":dbl, "Y":dbl} {"X"=113.0, "Y"=60.0} ("ORG") cluster{"X":dbl, "Y":dbl} {"X"=526.0, "Y"=60.0} ("ORG")] -> w4426
              frame "FCW", Default {
              }
              frame "BSD(Right)", "RCTA(Right)", "DOW(Right)" {
              }
              frame "BSD(Left)", "RCTA(Left)", "DOW(Left)" {
              }
            }
            n1763 = in-place {
              in-place-border: w4426 -> [w4435]
              n1764 = in-place-array #3(w4425, w4424) -> (w4437:T44)
              n1765 = Bundle By Name(cluster=w4437, "ORG"=w4435) -> (w4436:T44)
              n1766 = in-place-array #3(w4436) -> (w4423:T26)  [unwired: 1 out]
            }
            n1767 = Bundle By Name(cluster=w4430, "Last Mouse Position"=w4423) -> (w4431:T25)
            n1768 = Enqueue Element(queue=w4428, element=T18 {"State"=enum."Overlay", "variant"=variant}, error in (no error)=w4427) -> ()  [unwired: 1 in, 3 out]
          }
          frame "Lines Para" {
            w4440 = cluster{"X":dbl, "Y":dbl} {"X"=10.0, "Y"=10.0}  # Lines(X,Y)
            n1769 = Unbundle By Name(w4447) -> ("Last Mouse Position"=w4443:T26, "Mode"=w4441:T7)
            n1770 = call "Lines Convert.vi"("Mode"=w4441, "Lines(X,Y)"=w4440) -> ("Line to Line"=w4438:dbl[], "Lines Para"=w4439:dbl[][])  [unwired: 8 in]
            n1771 = in-place {
              in-place-border: w4439 -> [w4450]
              in-place-border: w4438 -> [w4449]
              n1772 = in-place-array #4(w4443, w4441) -> (w4452:T44)
              n1773 = Bundle By Name(cluster=w4452, "Lines Para"=w4450, "Line to Line"=w4449) -> (w4451:T44)
              n1774 = in-place-array #4(w4451) -> (w4442:T26)  [unwired: 1 out]
            }
            n1775 = Bundle By Name(cluster=w4447, "Last Mouse Position"=w4442) -> (w4448:T25)
            n1776 = Enqueue Element(queue=w4445, element=T18 {"State"=enum."ORG", "variant"=variant}, error in (no error)=w4444) -> ()  [unwired: 1 in, 3 out]
          }
          frame "Coordinate" {
            n1777 = Variant To Data(error in=w4458, type=cluster{"X":dbl, "Y":dbl} {"X"=0.0, "Y"=0.0} ("Coordinates(X,Y)"), Variant=w4459) -> (data=w4456:cluster{"X":dbl, "Y":dbl}, error out=w4455:errorcluster)
            n1778 = Bundle By Name(cluster=w4461, "Coordinates(X,Y)"=w4456) -> (w4460:T25)
            n1779 = Enqueue Element(queue=w4454, element=T18 {"State"=enum."Update", "variant"=variant}, error in (no error)=w4455) -> ()  [unwired: 1 in, 3 out]
          }
          frame "Path No." {
            (unwired) u16 0 items=["1", "2", "3", "4", "5", "6", "7", "8", "9", "10", "11", "12", "13", "14", "15", "16", "17", "18", "19", "20"] ("Path No.")
            # "2018.10.31 ­Y¦³¶W¹L20­ÓÂI¦ì¡A»Ý­n­×§ï¦¹Constant»PData¸ÌªºPath No."
            n1780 = Variant To Data(error in=w4478, type=0, Variant=w4479) -> (data=w4477:i32, error out=w4476:errorcluster)
            n1781 = Bundle By Name(cluster=w4480, "Path No."=w4477) -> (w4472:T25)
            n1782 = Unbundle By Name(w4472) -> ("Report Data.Coordinate"=w4462:cluster{string, string}[][], "User"=w4471:enum16{"Car 1", "Car 2"}, "Path No."=w4470:u16)  [unwired: 1 out]
            n1783 = Enqueue Element(queue=w4475, element=T18 {"State"=enum."Update", "variant"=variant}, error in (no error)=w4476) -> ()  [unwired: 1 in, 3 out]
            n1784 = case shown="\"Car 2\"" w4471 {
              tunnel: w4470 -> [w4485 w4486]
              tunnel: [w4484 w4488] -> w4467
              tunnel: w4462 -> [w4483 w4490]
              frame "Car 1", Default {
                n1785 = Index Array(array=w4483, index (row)=0) -> (element=w4482:cluster{string, string}[])  [unwired: 1 in]
                n1786 = Index Array(array=w4482, index=w4485) -> (element=w4484:cluster{string, string})
              }
              frame "Car 2" {
                n1787 = Index Array(array=w4490, index (row)=1) -> (element=w4489:cluster{string, string}[])  [unwired: 1 in]
                n1788 = Index Array(array=w4489, index=w4486) -> (element=w4488:cluster{string, string})
              }
            }
            n1789 = Unbundle(w4467) -> (w4466:string, w4464:string)
            n1790 = Fract/Exp String To Number(string=w4466) -> (number=w4465:dbl)  [unwired: 3 in, 1 out]
            n1791 = Fract/Exp String To Number(string=w4464) -> (number=w4463:dbl)  [unwired: 3 in, 1 out]
            n1792 = Bundle By Name(cluster=cluster{"X":dbl, "Y":dbl} {"X"=0.0, "Y"=0.0} ("Coordinates(X,Y)"), "X"=w4465, "Y"=w4463) -> (w4468:cluster{"X":dbl, "Y":dbl})
            n1793 = property on="Coordinates(X,Y)" class="Clust (strict)"("Value"=w4468) -> ()  [unwired: 2 in, 2 out]
          }
          frame "Modify" {
            n1794 = Unbundle By Name(w4502) -> ("Last Mouse Position"=w4505:T26, "Mode"=w4496:T7, "Path No."=w4504:u16, "Coordinates(X,Y)"=w4503:cluster{"X":dbl, "Y":dbl}, "User"=w4495:enum16{"Car 1", "Car 2"}, "DYNAMIC"=w4494:T1, "DYNAMIC 2"=w4492:T1)
            n1795 = in-place {
              in-place-border: w4504 -> [w4513]
              in-place-border: w4503 -> [w4516]
              in-place-border: w4496 -> [w4517]
              in-place-border: w4495 -> [w4512]
              in-place-border: w4494 -> [w4509]
              in-place-border: [w4508] -> w4493
              in-place-border: w4492 -> [w4507]
              in-place-border: [w4506] -> w4491
              n1796 = in-place-array #5(w4505, w4496) -> (w4515:T44)
              n1797 = call "Real Coordinates convert.vi"("Mode"=w4517, "Coordinates(X,Y)"=w4516, "Overlay Setting"=w4515) -> ("Real Coordinates(X,Y)"=w4514:cluster{dbl, dbl})  [unwired: 8 in]
              n1798 = To Long Integer(number=w4513) -> (32bit integer=w4511:i32)
              n1799 = property on="s/d setting" class="Bool (strict)"() -> ("Value"=w4510:bool)  [unwired: 2 in, 2 out]
              n1800 = case shown="\"Car 2\"" w4512 {
                tunnel: w4515 -> [w4527 w4542]
                tunnel: [w4526 w4541] -> w4518
                tunnel: w4514 -> [w4524 w4539]
                tunnel: w4511 -> [w4521 w4537]
                tunnel: w4510 -> [w4523 w4538]
                tunnel: w4509 -> [w4522 w4534]
                tunnel: [w4520 w4534] -> w4508
                tunnel: w4507 -> [w4519 w4536]
                tunnel: [w4519 w4535] -> w4506
                frame "Car 1", Default {
                  n1801 = case shown="False" w4523 {
                    tunnel: w4522 -> [w4532 w4533]
                    tunnel: w4521 -> [w4531 _]
                    tunnel: [w4530 w4533] -> w4520
                    frame False {
                      n1802 = property on="dynamic setting" class="Clust (strict)"() -> ("Value"=w4529:T5)  [unwired: 2 in, 2 out]
                      n1803 = Replace Array Subset(array=w4532, new element=w4529, index=w4531) -> (w4530:T1)
                    }
                    frame True {
                    }
                  }
                  n1804 = Unbundle By Name(w4527) -> ("User1"=w4528:cluster{"X":dbl, "Y":dbl}[])
                  n1805 = Replace Array Subset(array=w4528, new element=w4524, index=w4521) -> (w4525:cluster{"X":dbl, "Y":dbl}[])
                  n1806 = Bundle By Name(cluster=w4527, "User1"=w4525) -> (w4526:T44)
                }
                frame "Car 2" {
                  n1807 = case shown="False" w4538 {
                    tunnel: w4536 -> [w4547 w4548]
                    tunnel: w4537 -> [w4546 _]
                    tunnel: [w4545 w4548] -> w4535
                    frame False {
                      n1808 = property on="dynamic setting" class="Clust (strict)"() -> ("Value"=w4544:T5)  [unwired: 2 in, 2 out]
                      n1809 = Replace Array Subset(array=w4547, new element=w4544, index=w4546) -> (w4545:T1)
                    }
                    frame True {
                    }
                  }
                  n1810 = Unbundle By Name(w4542) -> ("User2"=w4543:cluster{"X":dbl, "Y":dbl}[])
                  n1811 = Replace Array Subset(array=w4543, new element=w4539, index=w4537) -> (w4540:cluster{"X":dbl, "Y":dbl}[])
                  n1812 = Bundle By Name(cluster=w4542, "User2"=w4540) -> (w4541:T44)
                }
              }
              n1813 = in-place-array #5(w4518) -> (w4500:T26)  [unwired: 1 out]
            }
            n1814 = Enqueue Element(queue=w4498, element=T18 {"State"=enum."Overlay", "variant"=variant}, error in (no error)=w4499) -> ()  [unwired: 1 in, 3 out]
            n1815 = Bundle By Name(cluster=w4502, "Last Mouse Position"=w4500, "DYNAMIC"=w4493, "DYNAMIC 2"=w4491) -> (w4501:T25)
          }
          frame "Load" {
            n1816 = Variant To Data(error in=w4557, type=path "" ("dup path"), Variant=w4558) -> (data=w4554:path, error out=w4551:errorcluster)
            n1817 = call-poly <vilib>:"Read From Spreadsheet File.vi"("delimiter (\\t)"="," ("delimiter (\\t)"), "file path (dialog if empty)"=w4554) -> ("all rows"=w4552:dbl[][])  [unwired: 5 in, 4 out]
            n1818 = Enqueue Element(queue=w4550, element=T18 {"State"=enum."RCS Report", "variant"=variant}, error in (no error)=w4551) -> ()  [unwired: 1 in, 3 out]
            n1819 = Bundle By Name(cluster=w4556, "Input RCS Data"=w4552) -> (w4555:T25)
          }
          frame "Loadpath" {
            n1820 = Variant To Data(error in=w4573, type=path "" ("dup path"), Variant=w4574) -> (data=w4560:path, error out=w4570:errorcluster)
            n1821 = Path To String(path=w4560) -> (string=w4564:string)
            n1822 = Match Pattern(string=w4564, regular expression="dynamic") -> (offset past match=w4561:i32)  [unwired: 1 in, 3 out]
            n1823 = Greater Than 0?(x=w4561) -> (x > 0?=w4562:bool)
            n1824 = call-poly <vilib>:"Read From XML File.vi"("error in (no error)"=w4570, "XML File Path"=w4560) -> ("error out"=w4566:errorcluster, "XML Elements"=w4568:string)  [unwired: 7 in, 1 out]
            n1825 = case shown="True" w4562 {
              selector: w4562 -> [_ w4599]
              tunnel: w4569 -> [w4580 w4620]
              tunnel: w4568 -> [w4579 w4619]
              tunnel: [w4578 w4618] -> w4567
              tunnel: w4566 -> [w4577 w4617]
              tunnel: [w4576 w4616] -> w4565
              tunnel: w4560 -> [_ w4606]
              frame False {
                n1826 = in-place {
                  in-place-border: w4579 -> [w4598]
                  in-place-border: w4577 -> [w4582]
                  in-place-border: [w4581] -> w4576
                  n1827 = in-place-cluster #6(w4580) -> ("Image"=w4595:T6, "User"=w4594:enum16{"Car 1", "Car 2"}, "Last Mouse Position"=w4597:T26, "Mode"=w4593:T7, "Report Data"=w4592:T27, "Target 1"=w4591:string, "Target 2"=w4590:string, "Velocity"=w4589:dbl, "Coordinates(X,Y)"=w4588:cluster{"X":dbl, "Y":dbl}, "Path No."=w4587:u16, "Input RCS File"=w4586:string, "Input RCS Data"=w4585:dbl[][], "Output £m File"=w4584:string, "DYNAMIC"=w4583:T1)
                  n1828 = Unflatten From XML(xml string=w4598, type=w4597, error in (no error)=w4582) -> (value=w4596:T26, error out=w4581:errorcluster)
                  n1829 = in-place-cluster #6("Image"=w4595, "User"=w4594, "Last Mouse Position"=w4596, "Mode"=w4593, "Report Data"=w4592, "Target 1"=w4591, "Target 2"=w4590, "Velocity"=w4589, "Coordinates(X,Y)"=w4588, "Path No."=w4587, "Input RCS File"=w4586, "Input RCS Data"=w4585, "Output £m File"=w4584, "DYNAMIC"=w4583) -> (w4578:T25)
                }
              }
              frame True {
                n1830 = Strip Path(path=w4606) -> (stripped path=w4612:path, name=w4615:string)
                n1831 = Strip Path(path=w4606) -> (stripped path=w4605:path, name=w4603:string)
                n1832 = Concatenate Strings("dy_path" ("string"), w4603) -> (w4604:string)
                n1833 = Build Path(base path=w4605, name or relative path=w4604) -> (appended path=w4602:path)
                n1834 = Concatenate Strings("setting" ("string"), w4615) -> (w4613:string)
                n1835 = call-poly <vilib>:"Read From XML File.vi"("XML File Path"=w4602) -> ("XML Elements"=w4601:string)  [unwired: 8 in, 2 out]
                n1836 = Build Path(base path=w4612, name or relative path=w4613) -> (appended path=w4611:path)
                n1837 = call-poly <vilib>:"Read From XML File.vi"("XML File Path"=w4611) -> ("XML Elements"=w4610:string)  [unwired: 8 in, 2 out]
                n1838 = in-place {
                  in-place-border: w4619 -> [w4647]
                  in-place-border: w4617 -> [w4630]
                  in-place-border: [w4634] -> w4616
                  in-place-border: w4610 -> [w4631]
                  in-place-border: [w4625] -> w4608
                  in-place-border: [w4624] -> w4607
                  in-place-border: w4601 -> [w4621]
                  n1839 = in-place-cluster #7(w4620) -> ("Image"=w4646:T6, "User"=w4645:enum16{"Car 1", "Car 2"}, "Last Mouse Position"=w4633:T26, "Mode"=w4644:T7, "Report Data"=w4643:T27, "Target 1"=w4642:string, "Target 2"=w4641:string, "Velocity"=w4640:dbl, "Coordinates(X,Y)"=w4639:cluster{"X":dbl, "Y":dbl}, "Path No."=w4638:u16, "Input RCS File"=w4637:string, "Input RCS Data"=w4636:dbl[][], "Output £m File"=w4635:string, "DYNAMIC"=w4629:T1, "DYNAMIC 2"=w4628:T1, "dy Path"=w4623:T8)
                  n1840 = Build Array(w4629, w4628) -> (w4627:T43)
                  n1841 = Unflatten From XML(xml string=w4621, type=w4623) -> (value=w4622:T8)  [unwired: 1 in, 1 out]
                  n1842 = Unflatten From XML(xml string=w4631, type=w4627, error in (no error)=w4630) -> (value=w4626:T43)  [unwired: 1 out]
                  n1843 = Unflatten From XML(xml string=w4647, type=w4633, error in (no error)=w4630) -> (value=w4632:T26, error out=w4634:errorcluster)
                  n1844 = Index Array(array=w4626) -> (element #1=w4625:T1, element #2=w4624:T1)  [unwired: 4 in]
                  n1845 = in-place-cluster #7("Image"=w4646, "User"=w4645, "Last Mouse Position"=w4632, "Mode"=w4644, "Report Data"=w4643, "Target 1"=w4642, "Target 2"=w4641, "Velocity"=w4640, "Coordinates(X,Y)"=w4639, "Path No."=w4638, "Input RCS File"=w4637, "Input RCS Data"=w4636, "Output £m File"=w4635, "DYNAMIC"=w4625, "DYNAMIC 2"=w4624, "dy Path"=w4622) -> (w4618:T25)
                }
                n1846 = Index Array(array=w4608) -> (element=w4609:T5)  [unwired: 1 in]
                n1847 = property on="DYNAMIC" class="Arr (strict)"("Value"=w4608) -> ()  [unwired: 2 in, 2 out]
                n1848 = property on="dynamic setting" class="Clust (strict)"("Value"=w4609) -> ()  [unwired: 2 in, 2 out]
                n1849 = property on="DYNAMIC 2" class="Arr (strict)"("Value"=w4607) -> ()  [unwired: 2 in, 2 out]
                "load?" <- w4599
              }
            }
            n1850 = Enqueue Element(queue=w4572, element=T18 {"State"=enum."Overlay", "variant"=variant}, error in (no error)=w4565) -> ()  [unwired: 1 in, 3 out]
          }
          frame "Clear All" {
            w4648 = T45 [] ("DYNAMIC")
            w4654 = u16 0 items=["1", "2", "3", "4", "5", "6", "7", "8", "9", "10", "11", "12", "13", "14", "15", "16", "17", "18", "19", "20"] ("Path No.")
            n1851 = Unbundle By Name(w4660) -> ("Last Mouse Position"=w4657:T26, "Mode"=w4656:T7)
            n1852 = in-place {
              w4673 = 0
              w4668 = 1000 ("dimension size")
              w4671 = cluster{"X":i32, "Y":i32} {"X"=0, "Y"=0}
              n1853 = in-place-array #8(w4657, w4656) -> (w4667:T44)
              n1854 = property on="Lane Distance(X,Y)" class="Clust (strict)"() -> ("Value"=w4664:cluster{"X":dbl, "Y":dbl})  [unwired: 2 in, 2 out]
              n1855 = Initialize Array(w4671, w4668) -> (w4672:cluster{"X":i32, "Y":i32}[])
              n1856 = Initialize Array(0.0 ("Breadth"), w4668) -> (w4665:dbl[])
              n1857 = Bundle(cluster=w4667, "User1"=w4672, "Times 1"=w4673, "User2"=w4672, "Times 2"=w4673, "ORG"=w4671, "ORG?"=FALSE, "User1 Velocity"=w4665, "User2 Velocity"=w4665, "Lane Distance(X,Y)"=w4664, "Lines Para"=dbl[][] [], "Line to Line"=dbl[] []) -> (w4666:T44)
              n1858 = in-place-array #8(w4666) -> (w4655:T26)  [unwired: 1 out]
            }
            n1859 = property on="Image" class="ImageControl"(error in=w4650, "ROI"=T14 {"Global Rectangle"=[], "Contours"=[]}) -> ()  [unwired: 1 in, 2 out]
            n1860 = Enqueue Element(queue=w4658, element=T18 {"State"=enum."Lines Para", "variant"=variant}, error in (no error)=w4650) -> ()  [unwired: 1 in, 3 out]
            n1861 = Bundle By Name(cluster=w4660, "Last Mouse Position"=w4655, "Path No."=w4654, "DYNAMIC 2"=w4648, "DYNAMIC"=w4648) -> (w4661:T25)
            n1862 = property on="Report Data.Degree" class="Arr (strict)"("Value"=dbl[][] [] ("Report Data.Degree")) -> ()  [unwired: 2 in, 2 out]
            n1863 = property on="DYNAMIC" class="Arr (strict)"("Value"=w4648) -> ()  [unwired: 2 in, 2 out]
            n1864 = property on="MSG" class="Str"("Value"="" ("MSG")) -> ()  [unwired: 2 in, 2 out]
            n1865 = property on="Array" class="Arr (strict)"("Value"=T2 [] ("Array")) -> ()  [unwired: 2 in, 2 out]
          }
          frame "Exit" {
            n1866 = Unbundle By Name(w4676) -> ("Image"=w4675:T6)
            n1867 = call "IMAQ Dispose"("Image"=w4675, "error in (no error)"=w4674) -> ()  [unwired: 4 in, 1 out]
          }
        }
      }
      n1868 = disable-structure shown="Disabled" {
        disable-tunnel: w90 -> [w104 _]
        frame Disabled {
          n1869 = while {
            tunnel: w104 -> [_]
            stop <- w108 stop-if-true
            n1870 = property on="auto step finish?" class="Bool (strict)"() -> ("Value"=w106:bool)  [unwired: 2 in, 2 out]
            n1871 = Not(x=w106) -> (.not. x?=w105:bool)
            n1872 = case shown="True" w105 {
              frame False {
              }
              frame True {
                w109 = TRUE ("value")
                n1873 = local read "autoSliderfinish?"() -> (w110:bool)
                n1874 = Compound Arithmetic op=AND(w109, w109, w110) -> (w111:bool)
                n1875 = property on="auto step finish?" class="Bool (strict)"("Value"=w111) -> ()  [unwired: 2 in, 2 out]
              }
            }
            n1876 = property on="Exit" class="Bool (strict)"() -> ("Value"=w108:bool)  [unwired: 2 in, 2 out]
            n1877 = Wait (ms)(milliseconds to wait=u32 100) -> ()  [unwired: 1 out]
          }
        }
        frame Enabled {
        }
      }
      n1878 = while {
        tunnel: w90 -> [w120]
        stop <- TRUE stop-if-true
        n1879 = property on="generateWF ok?" class="DigNum (strict)" props=["Value"]() -> ()  [unwired: 2 in, 3 out]
        n1880 = Greater Than 0?(x=0.0) -> (x > 0?=w119:bool)
        n1881 = case shown="True" w119 {
          tunnel: [w122 w126] -> _
          tunnel: w120 -> [w122 w124]
          frame False {
          }
          frame True {
            n1882 = dll-call lib="D:/0717/0717/Radar - 2015 32bit_autoqueue_angle_0319/Debug 2/Test_ARTS_1.dll" fn="?_CheckStatus@@YAHXZ" label="_GetSystemStatus"(error in=w124) -> (error out=w125:errorcluster, "return type"=w127:i32)  [unwired: 2 in, 1 out]
            n1883 = Greater Or Equal To 0?(x=w127) -> (x >= 0?=w123:bool)
            n1884 = property on="Status?" class="Bool (strict)"("Value"=w123) -> ()  [unwired: 2 in, 2 out]
            n1885 = call <vilib>:"Clear Errors.vi"("error in (no error)"=w125) -> ("error out"=w126:errorcluster)  [unwired: 5 in, 1 out]
          }
        }
        n1886 = Wait (ms)(milliseconds to wait=u32 100) -> ()  [unwired: 1 out]
      }
    }
    frame #3 {
      w5138 = TRUE ("run minimized? (F)")
      w5137 = TRUE ("wait until completion? (T)")
      n1887 = disable-structure shown="RUN_TIME_ENGINE==True" {
        frame condition #0 (active) {
        }
        frame condition #1 {
          n1888 = Quit LabVIEW(quit? (T)=TRUE) -> ()
        }
      }
      n1889 = call <vilib>:"System Exec.vi"("run minimized? (F)"=w5138, "wait until completion? (T)"=w5137, "command line"="taskkill /F /IM Application.exe /T") -> ()  [unwired: 5 in, 4 out]
      n1890 = call <vilib>:"System Exec.vi"("run minimized? (F)"=w5138, "wait until completion? (T)"=w5137, "command line"="taskkill /F /IM PING.exe /T") -> ()  [unwired: 5 in, 4 out]
    }
  }
  n1891 = disable-structure shown="Default" {
    frame Enabled {
      n1892 = Multiply(x=3.141592653589793, y=4.0) -> (x*y=w5144:dbl)
      n1893 = Power Of X(1:w5144, 2:3.0 ("y")) -> (0:→"x^y":dbl)
    }
  }
  n1894 = disable-structure shown="Default" {
    frame Enabled {
      n1895 = Power Of X(1:10.0 ("x"), 2:8.0 ("y")) -> (0:w5150:dbl)
      n1896 = Multiply(x=3.0, y=w5150) -> (x*y=→"x*y":dbl)
    }
  }
  n1897 = disable-structure shown="Disabled" {
    frame Disabled {
      n1898 = for {
        shift-right: [w5159] -> _
        shift-left: _ -> [w5158]
        i -> [w5152]
        n1899 = Bundle By Name(cluster=T19 {enum."Direct Program", "variant"=variant}) -> (w5161:T19)  [unwired: 1 in]
        n1900 = flat-sequence {
          tunnel: [w5169] -> w5160
          tunnel: w5161 -> [w5172]
          tunnel: w5158 -> [w5165]
          tunnel: w5152 -> [w5167]
          tunnel: [w5163] -> w5153
          tunnel: w5160 -> [w5181]
          tunnel: [w5180] -> w5157
          tunnel: [w5179] -> w5154
          tunnel: w5153 -> [w5179]
          tunnel: w5157 -> [w5189]
          tunnel: [w5188] -> w5156
          tunnel: [w5187] -> w5155
          tunnel: w5154 -> [w5187]
          tunnel: [w5200] -> w5159
          tunnel: w5156 -> [w5199]
          tunnel: w5155 -> [w5198]
          frame #0 {
            w5164 = FALSE ("RUN")
            n1901 = Enqueue Element(element=w5172, error in (no error)=w5165) -> (queue out=w5163:refnum<queue>, error out=w5170:errorcluster)  [unwired: 2 in, 1 out]
            n1902 = Bundle By Name(cluster=cluster{"State":T17, "Variable":variant} {"State"=enum."auto mode", "Variable"=variant}, "Variable"=w5167) -> (w5166:cluster{"State":T17, "Variable":variant})
            n1903 = Enqueue Element(element=w5166, error in (no error)=w5165) -> ()  [unwired: 2 in, 3 out]
            n1904 = for {
              tunnel: T19[] [{enum."Convert", "variant"=variant}, {enum."RF ON/OFF", "variant"=variant}] -> [w5175] mode=indexing
              tunnel: w5163 -> [w5178]
              tunnel: w5170 -> [w5177]
              tunnel: [w5176] -> w5169
              n1905 = Bundle By Name(cluster=w5175, "variant"=TRUE) -> (w5174:T19)
              n1906 = Enqueue Element(queue=w5178, element=w5174, error in (no error)=w5177) -> (error out=w5176:errorcluster)  [unwired: 1 in, 2 out]
            }
            n1907 = property on="RUN" class="Bool (strict)"("Value"=w5164) -> ()  [unwired: 2 in, 2 out]
            n1908 = property on="auto step finish?" class="Bool (strict)"("Value"=w5164) -> ()  [unwired: 2 in, 2 out]
          }
          frame #1 {
            n1909 = while {
              tunnel: w5181 -> [w5186]
              tunnel: [w5186] -> w5180
              stop <- w5182 stop-if-true
              n1910 = property on="auto step finish?" class="Bool (strict)"() -> ("Value"=w5184:bool)  [unwired: 2 in, 2 out]
              n1911 = property on="Exit" class="Bool (strict)"() -> ("Value"=w5183:bool)  [unwired: 2 in, 2 out]
              n1912 = Or(x=w5184, y=w5183) -> (x .or. y?=w5182:bool)
              n1913 = Wait (ms)(milliseconds to wait=u32 100) -> ()  [unwired: 1 out]
            }
          }
          frame #2 {
            n1914 = while {
              tunnel: w5189 -> [w5193]
              tunnel: [w5193] -> w5188
              stop <- w5190 stop-if-true
              n1915 = property on="RUN" class="Bool (strict)"() -> ("Value"=w5192:bool)  [unwired: 2 in, 2 out]
              n1916 = property on="Exit" class="Bool (strict)"() -> ("Value"=w5191:bool)  [unwired: 2 in, 2 out]
              n1917 = Or(x=w5192, y=w5191) -> (x .or. y?=w5190:bool)
              n1918 = Wait (ms)(milliseconds to wait=u32 100) -> ()  [unwired: 1 out]
            }
          }
          frame #3 {
            n1919 = Bundle By Name(cluster=T19 {enum."RF ON/OFF", "variant"=variant}, "variant"=FALSE) -> (w5196:T19)
            n1920 = Enqueue Element(queue=w5198, element=w5196, error in (no error)=w5199) -> (error out=w5200:errorcluster)  [unwired: 1 in, 2 out]
          }
        }
      }
    }
    frame Enabled {
    }
  }
